vi "DéfiGentecEO.vi"() -> ()   [LabVIEW 2017]
uses:
  PC-Beamage Labview Distribution/BeamageNP.dll
panel:
  in  "File Type 2":enum16{"JPG", "PNG", "BMP"}(ring)=enum."BMP"
  in  "File Type":enum16{"JPG", "PNG", "BMP"}(ring)=enum."BMP"
  in  "Panneau de Fin":string caption="Tous les vaisseaux\n  ont été détruits!"
  out "Loop":dbl
  out "Saturation Power":dbl
  out "Yposition":dbl
  out "Xposition":dbl
  in  "Boolean":bool
  in  "error in  2":errorcluster
  out "DLL is Present":bool
  out "path":path
  out "error out 3":errorcluster
  in  "error in":errorcluster
  out "Connected":bool
  out "error out":errorcluster
  out "Pause En Cours 1":bool
  out "Temps Pause 1":timestamp
  out "Barre Bleue 1":dbl(slide) scale=0.0..100.0
  out "Pointage 1":dbl
  out "Barre Verte 1":dbl(slide) max=50.0 scale=0.0..100.0
  out "Chrono 1":dbl format="%.2g"
  in  "Cancel Button":bool
  out "Nombre total de vaisseaux":dbl
  out "Barre Rouge 1":dbl(slide) scale=0.0..100.0
  out "XY Graph 1":cluster{dbl[], dbl[]}[](graph)
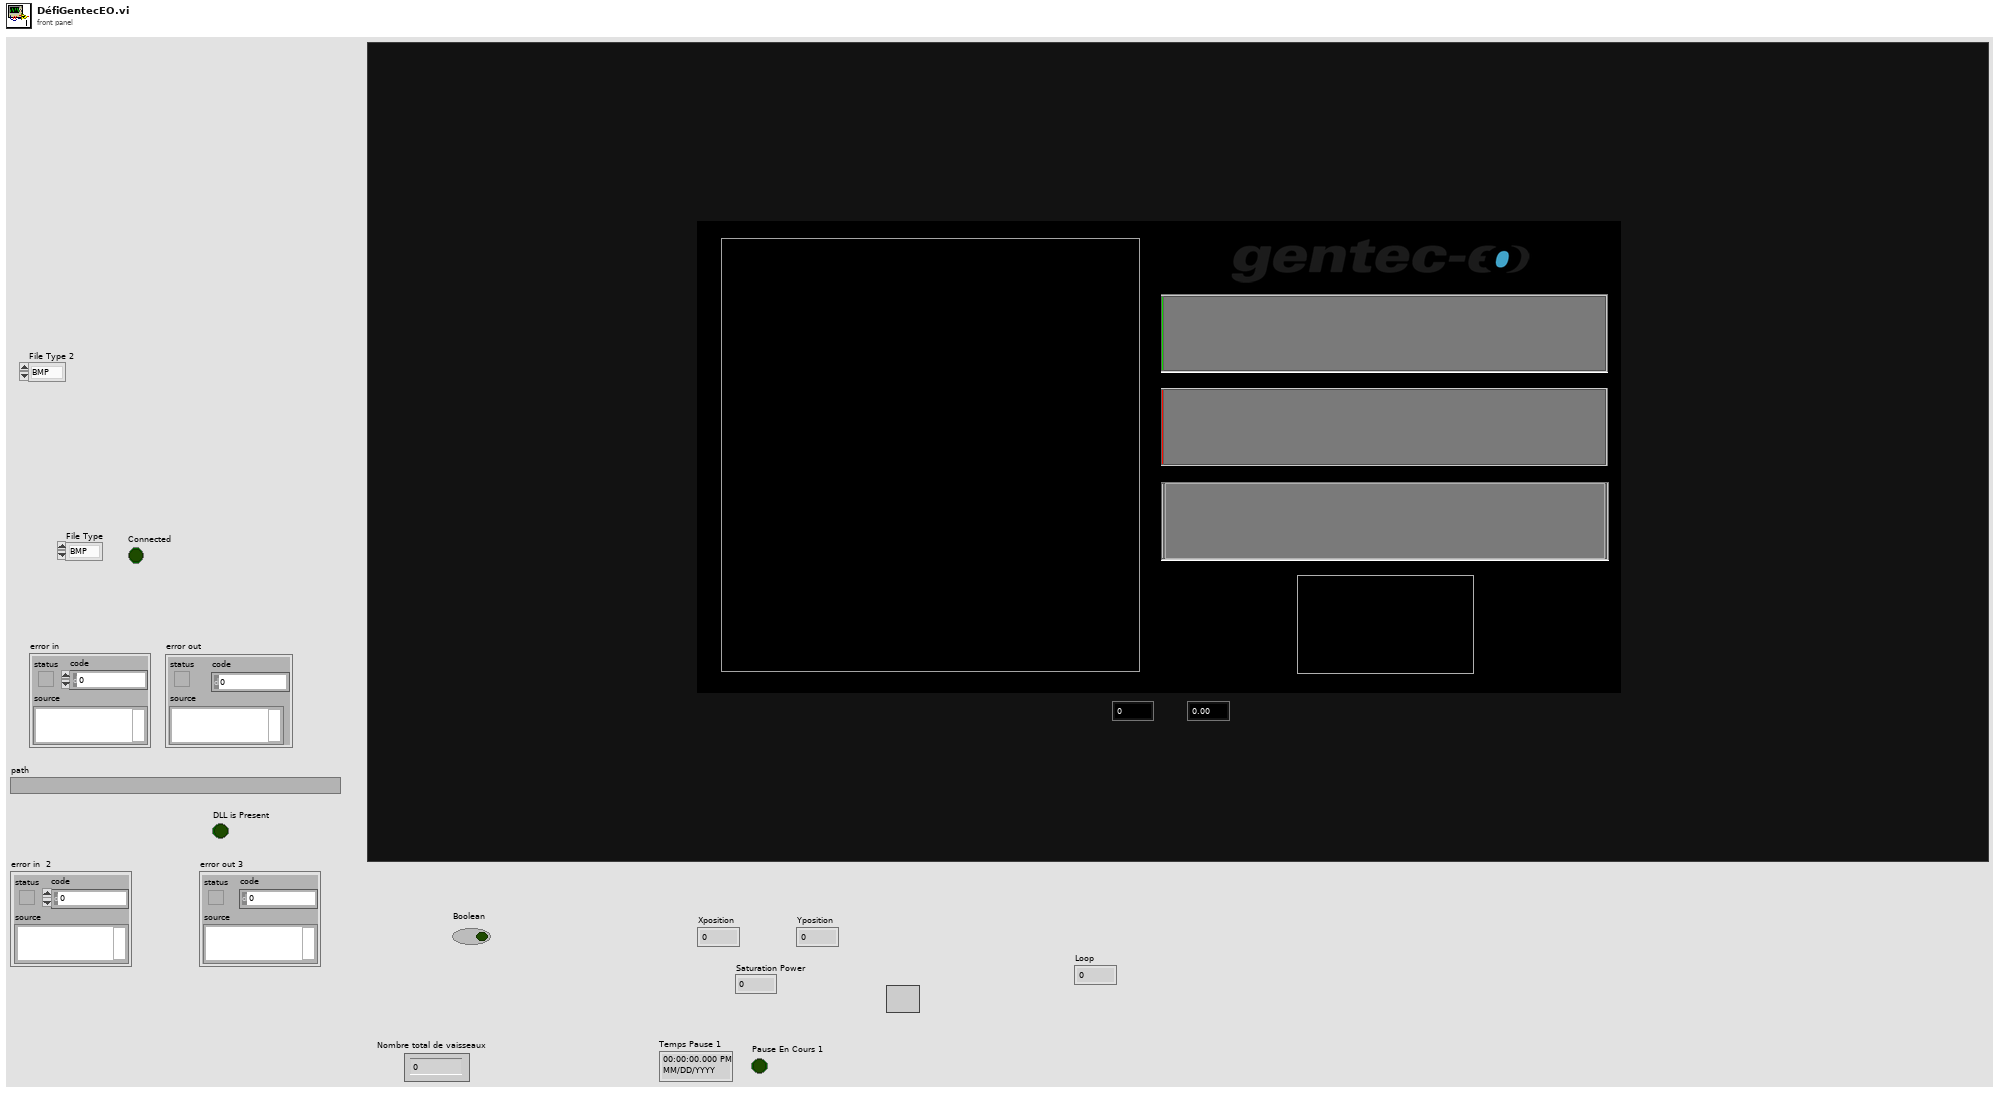
[diagram p1: front panel]
types:
  T1 = typedef "imagedata.ctl" = cluster{"image type":i32, "image depth":i32, "image":u8[], "mask":u8[], "colors":u32[], "Rectangle":cluster{"left":i16, "top":i16, "right":i16, "bottom":i16}}
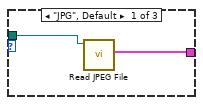
[diagram p2: hidden frame]
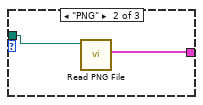
[diagram p3: hidden frame]
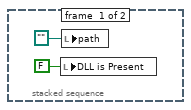
[diagram p4: hidden frame]
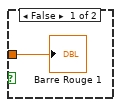
[diagram p11: hidden frame]
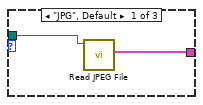
[diagram p13: hidden frame]
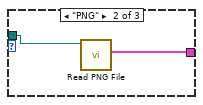
[diagram p14: hidden frame]
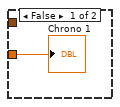
[diagram p15: hidden frame]
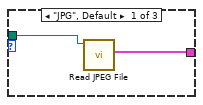
[diagram p17: hidden frame]
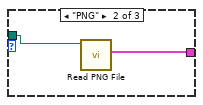
[diagram p18: hidden frame]
diagram:
  n1 = flat-sequence {
    tunnel: [w25] -> w2
    tunnel: [w13] -> w1
    tunnel: w2 -> [w56]
    tunnel: w1 -> [w55]
    frame #0 {
      w10 = u32 16777215
      w22 = 0
      # "Code LabVIEW écrit par Charles Matte-Breton dans le cadre de la 10e édition des Jeux Photoniques (23 octobre 2017)"
      n2 = Current VI's Path() -> (path=w5:path)
      n3 = case shown="No Error" "error in" {
        selector: "error in" -> [w50 w54]
        tunnel: [w49 w54] -> w17
        frame No Error {
          # "Verify that PC Beamage is running and the Labview data  pipe is open."
          n4 = dll-call lib="PTH2Šabs CUsersCharles\tDocumentsÃ‰coleImplicationJeux PhotoniquesDÃ©fi Gentec-EOPC-Beamage Labview Distribution\nBeamageNP.dll" fn="OpenNP"(error in=w50) -> (error out=w49:errorcluster, "return type"=w53:i32)  [unwired: 2 in, 1 out]
          n5 = Equal?(x=w53, y=1) -> (x = y?=→"Connected":bool)
        }
        frame Error {
        }
      }
      "error out" <- w17
      n6 = local write "Barre Rouge 1"(w22) -> ()
      n7 = local write "Barre Bleue 1"(w22) -> ()
      n8 = property on="XY Graph 1" class="XYGraph (strict)"("BG Color"=u32 0) -> ()  [unwired: 2 in, 2 out]
      n9 = case shown="No Error" "error in  2" {
        selector: "error in  2" -> [w33 w48]
        tunnel: [w32 w48] -> w15
        frame No Error {
          # "Verify the DLL Labview needs to communicate with PC-Beamage is present on the PC.\n\nFile should be in the same directory as this VI."
          n10 = stacked-sequence {
            tunnel: w33 -> [_ w43]
            tunnel: [_ w41] -> w32
            frame #0 {
              n11 = local write "DLL is Present"(FALSE ("file exists?")) -> ()
              n12 = local write "path"(path "") -> ()
            }
            frame #1 {
              n13 = property class="VI"(error in=w43) -> (error out=w42:errorcluster, "Path"=w47:path, "Name"=w37:string)  [unwired: 1 in, 1 out]
              n14 = Path To String(path=w47) -> (string=w38:string)
              n15 = Match Pattern(string=w38, regular expression=w37) -> (before substring=w36:string)  [unwired: 1 in, 3 out]
              n16 = Concatenate Strings(w36, "BeamageNP.dll" ("string")) -> (w45:string)
              n17 = String To Path(string=w45) -> (path=w44:path)
              n18 = call <vilib>:"Check if File or Folder Exists.vi"("error in (no error)"=w42, "path"=w44) -> ("error out"=w41:errorcluster, "file or folder exists?"=→"DLL is Present":bool, "dup path"=→"path":path)  [unwired: 7 in]
            }
          }
        }
        frame Error {
        }
      }
      "error out 3" <- w15
      n19 = property on="Chrono 1" class="DigNum (strict)"("NumText.BGColor"=u32 0) -> ()  [unwired: 2 in, 2 out]
      n20 = Build Path(base path=w5, name or relative path=path "../Espace.bmp") -> (appended path=w3:path)
      n21 = case shown="\"BMP\"" "File Type" {
        tunnel: [w27 w29 w31] -> w8
        tunnel: w3 -> [w26 w28 w30]
        frame "JPG", Default {
          n22 = call <vilib>:"Read JPEG File.vi"("path to JPEG file"=w26) -> ("image data"=w27:T1)  [unwired: 8 in, 2 out]
        }
        frame "PNG" {
          n23 = call <vilib>:"Read PNG File.vi"("path to PNG file"=w28) -> ("image data"=w29:T1)  [unwired: 8 in, 2 out]
        }
        frame "BMP" {
          n24 = call <vilib>:"Read BMP File.vi"("path to BMP file"=w30) -> ("image data"=w31:T1)  [unwired: 8 in, 2 out]
        }
      }
      n25 = Wait (ms)(milliseconds to wait=5) -> ()  [unwired: 1 out]
      n26 = local write "Pause En Cours 1"(FALSE) -> ()
      n27 = property on="Chrono 1" class="DigNum (strict)"("NumText.TextColor"=w10) -> ()  [unwired: 2 in, 2 out]
      n28 = property on="Panneau de Fin" class="Str"("Visible"=FALSE) -> ()  [unwired: 2 in, 2 out]
      n29 = call <vilib>:"Draw Flattened Pixmap.vi"("image data"=w8) -> ("new picture"=w6:picture)  [unwired: 8 in]
      n30 = local write "Pointage 1"(0) -> ()
      n31 = property on="Pointage 1" class="DigNum (strict)"("NumText.TextColor"=w10) -> ()  [unwired: 2 in, 2 out]
      n32 = property on="XY Graph 1" class="XYGraph (strict)"("PlotImages.Back"=w6) -> ()  [unwired: 2 in, 2 out]
      n33 = Spreadsheet String To Array(format string="%f", spreadsheet string="0\t0\n0\t0\n0\t0\n0\t0\n0\t0\n0\t0\n0\t0\n0\t0\n0\t0\n0\t0\n0\t0\n0\t0\n0\t0\n0\t0\n0\t0\n0\t0\n0\t0\n0\t0\n0\t0\n0\t0\n0\t0\n0\t0\n0\t0\n0\t0\n0\t0\n0\t0\n0\t0\n0\t0\n0\t0\n0\t0\n0\t0\n0\t0\n0\t0\n0\t0\n0\t0\n0\t0\n0\t0\n0\t0\n0\t0\n0\t0\n0\t0\n0\t0\n0\t0\n0\t0\n0\t0\n0\t0\n0\t0\n0\t0\n0\t0\n0\t0\n0\t0\n0\t0\n0\t0\n0\t0\n0\t0\n0\t0\n0\t0\n0\t0\n0\t0\n0\t0\n0\t0\n0\t0\n0\t0\n0\t0\n0\t0\n0\t0\n0\t0\n0\t0\n0\t0\n0\t0\n0\t0\n0\t0\n0\t0\n0\t0\n0\t0\n0\t0\n0\t0\n0\t0\n0\t0\n0\t0\n0\t0\n0\t0\n0\t0\n0\t0\n0\t0\n0\t0\n0\t0\n0\t0\n0\t0\n0\t0\n0\t0\n0\t0\n0\t0\n0\t0\n0\t0\n0\t0\n0\t0\n0\t0\n0\t0\n0\t0\n0\t0\n0\t0\n0\t0\n0\t0\n0\t0\n0\t0\n0\t0\n0\t0\n0\t0\n0\t0\n0\t0\n0\t0\n0\t0\n0\t0\n0\t0\n0\t0\n0\t0\n0\t0\n0\t0\n0\t0\n0\t0\n0\t0\n0\t0\n0\t0\n0\t0\n0\t0\n0\t0\n0\t0\n0\t0\n0\t0\n0\t0\n0\t0\n0\t0\n0\t0\n0\t0\n0\t0\n0\t0\n0\t0\n0\t0\n0\t0\n0\t0\n0\t0\n0\t0\n0\t0\n0\t0\n0\t0\n0\t0\n0\t0\n0\t0\n0\t0\n0.1\t0\n0.2\t0\n0.3\t0\n0.4\t0\n0.5\t0\n0.6\t0\n0.7\t0\n0.8\t0\n0.9\t0\n1\t0\n1.1\t0\n1.2\t0\n1.3\t0\n1.4\t0\n1.5\t0\n1.6\t0\n1.7\t0\n1.8\t0\n1.9\t0\n2\t0\n2.1\t0\n2.2\t0\n2.3\t0\n2.4\t0\n2.5\t0\n2.6\t0\n2.7\t0\n2.8\t0\n2.9\t0\n3\t0\n3.1\t0\n3.2\t0\n3.3\t0\n3.4\t0\n3.5\t0\n3.6\t0\n3.7\t0\n3.8\t0\n3.9\t0\n4\t0\n4.1\t0\n4.2\t0\n4.3\t0\n4.4\t0\n4.5\t0\n4.6\t0\n4.7\t0\n4.8\t0\n4.9\t0\n5\t0\n5.1\t0\n5.2\t0\n5.3\t0\n5.4\t0\n5.5\t0\n5.6\t0\n5.7\t0\n5.8\t0\n5.9\t0\n6\t0\n6.1\t0\n6.2\t0\n6.3\t0\n6.4\t0\n6.5\t0\n6.6\t0\n6.7\t0\n6.8\t0\n6.9\t0\n7\t0\n7.1\t0\n7.2\t0\n7.3\t0\n7.4\t0\n7.5\t0\n7.6\t0\n7.7\t0\n7.8\t0\n7.9\t0\n8\t0\n8.1\t0\n8.2\t0\n8.3\t0\n8.4\t0\n8.5\t0\n8.6\t0\n8.7\t0\n8.8\t0\n8.9\t0\n9\t0\n9.1\t0\n9.2\t0\n9.3\t0\n9.4\t0\n9.5\t0\n9.6\t0\n9.7\t0\n9.8\t0\n9.9\t0\n10\t0\n10.1\t0\n10.2\t0\n10.3\t0\n10.4\t0\n10.5\t0\n10.6\t0\n10.7\t0\n10.8\t0\n10.9\t0\n11\t0\n11.1\t0\n11.2\t0\n11.3\t0\n11.4\t0\n11.5\t0\n11.6\t0\n11.7\t0\n11.8\t0\n11.9\t0\n12\t0\n12.1\t0\n12.2\t0\n12.3\t0\n12.4\t0\n12.5\t0\n12.6\t0\n12.7\t0\n12.8\t0\n12.9\t0\n13\t0\n13.1\t0\n13.2\t0\n13.3\t0\n13.4\t0\n13.5\t0\n13.6\t0\n13.7\t0\n13.8\t0\n13.9\t0\n14\t0\n14.1\t0\n14.2\t0\n14.3\t0\n14.4\t0\n14.5\t0\n14.6\t0\n14.7\t0\n14.8\t0\n14.9\t0\n15\t0\n15.1\t0\n15.2\t0\n15.3\t0\n15.4\t0\n15.5\t0\n15.6\t0\n15.7\t0\n15.8\t0\n15.9\t0\n16\t0\n16.1\t0\n16.2\t0\n16.3\t0\n16.4\t0\n16.5\t0\n16.6\t0\n16.7\t0\n16.8\t0\n16.9\t0\n17\t0\n17.1\t0\n17.2\t0\n17.3\t0\n17.4\t0\n17.5\t0\n17.6\t0\n17.7\t0\n17.8\t0\n17.9\t0\n18\t0\n18.1\t0\n18.2\t0\n18.3\t0\n18.4\t0\n18.5\t0\n18.6\t0\n18.7\t0\n18.8\t0\n18.9\t0\n19\t0\n19.1\t0\n19.2\t0\n19.3\t0\n19.4\t0\n19.5\t0\n19.6\t0\n19.7\t0\n19.8\t0\n19.9\t0\n20\t0\n20.1\t0\n20.2\t0\n20.3\t0\n20.4\t0\n20.5\t0\n20.6\t0\n20.7\t0\n20.8\t0\n20.9\t0\n21\t0\n21.1\t0\n21.2\t0\n21.3\t0\n21.4\t0\n21.5\t0\n21.6\t0\n21.7\t0\n21.8\t0\n21.9\t0\n22\t0\n22.1\t0\n22.2\t0\n22.3\t0\n22.4\t0\n22.5\t0\n22.6\t0\n22.7\t0\n22.8\t0\n22.9\t0\n23\t0\n23.1\t0\n23.2\t0\n23.3\t0\n23.4\t0\n23.5\t0\n23.6\t0\n23.7\t0\n23.8\t0\n23.9\t0\n24\t0\n24.1\t0\n24.2\t0\n24.3\t0\n24.4\t0\n24.5\t0\n24.6\t0\n24.7\t0\n24.8\t0\n24.9\t0\n25\t0\n25.1\t0\n25.2\t0\n25.3\t0\n25.4\t0\n25.5\t0\n25.6\t0\n25.7\t0\n25.8\t0\n25.9\t0\n26\t0\n26.1\t0\n26.2\t0\n26.3\t0\n26.4\t0\n26.5\t0\n26.6\t0\n26.7\t0\n26.8\t0\n26.9\t0\n27\t0\n27.1\t0\n27.2\t0\n27.3\t0\n27.4\t0\n27.5\t0\n27.6\t0\n27.7\t0\n27.8\t0\n27.9\t0\n28\t0\n28.1\t0\n28.2\t0\n28.3\t0\n28.4\t0\n28.5\t0\n28.6\t0\n28.7\t0\n28.8\t0\n28.9\t0\n29\t0\n29.1\t0\n29.2\t0\n29.3\t0\n29.4\t0\n29.5\t0\n29.6\t0\n29.7\t0\n29.8\t0\n29.9\t0\n30\t0\n30.1\t0\n30.2\t0\n30.3\t0\n30.4\t0\n30.5\t0\n30.6\t0\n30.7\t0\n30.8\t0\n30.9\t0\n31\t0\n31.1\t0\n31.2\t0\n31.3\t0\n31.4\t0\n31.5\t0\n31.6\t0\n31.7\t0\n31.8\t0\n31.9\t0\n32\t0\n32.1\t0\n32.2\t0\n32.3\t0\n32.4\t0\n32.5\t0\n32.6\t0\n32.7\t0\n32.8\t0\n32.9\t0\n33\t0\n33.1\t0\n33.2\t0\n33.3\t0\n33.4\t0\n33.5\t0\n33.6\t0\n33.7\t0\n33.8\t0\n33.9\t0\n34\t0\n34.1\t0\n34.2\t0\n34.3\t0\n34.4\t0\n34.5\t0\n34.6\t0\n34.7\t0\n34.8\t0\n34.9\t0\n35\t0\n35.1\t0\n35.2\t0\n35.3\t0\n35.4\t0\n35.5\t0\n35.6\t0\n35.7\t0\n35.8\t0\n35.9\t0\n36\t0\n36.1\t0\n36.2\t0\n36.3\t0\n36.4\t0\n36.5\t0\n36.6\t0\n36.7\t0\n36.8\t0\n36.9\t0\n37\t0\n37.1\t0\n37.2\t0\n37.3\t0\n37.4\t0\n37.5\t0\n37.6\t0\n37.7\t0\n37.8\t0\n37.9\t0\n38\t0\n38.1\t0\n38.2\t0\n38.3\t0\n38.4\t0\n38.5\t0\n38.6\t0\n38.7\t0\n38.8\t0\n38.9\t0\n39\t0\n39.1\t0\n39.2\t0\n39.3\t0\n39.4\t0\n39.5\t0\n39.6\t0\n39.7\t0\n39.8\t0\n39.9\t0\n40\t0\n40.1\t0\n40.2\t0\n40.3\t0\n40.4\t0\n40.5\t0\n40.6\t0\n40.7\t0\n40.8\t0\n40.9\t0\n41\t0\n41.1\t0\n41.2\t0\n41.3\t0\n41.4\t0\n41.5\t0\n41.6\t0\n41.7\t0\n41.8\t0\n41.9\t0\n42\t0\n42.1\t0\n42.2\t0\n42.3\t0\n42.4\t0\n42.5\t0\n42.6\t0\n42.7\t0\n42.8\t0\n42.9\t0\n43\t0\n43.1\t0\n43.2\t0\n43.3\t0\n43.4\t0\n43.5\t0\n43.6\t0\n43.7\t0\n43.8\t0\n43.9\t0\n44\t0\n44.1\t0\n44.2\t0\n44.3\t0\n44.4\t0\n44.5\t0\n44.6\t0\n44.7\t0\n44.8\t0\n44.9\t0\n45\t0\n45.1\t0\n45.2\t0\n45.3\t0\n45.4\t0\n45.5\t0\n45.6\t0\n45.7\t0\n45.8\t0\n45.9\t0\n46\t0\n46.1\t0\n46.2\t0\n46.3\t0\n46.4\t0\n46.5\t0\n46.6\t0\n46.7\t0\n46.8\t0\n46.9\t0\n47\t0\n47.1\t0\n47.2\t0\n47.3\t0\n47.4\t0\n47.5\t0\n47.6\t0\n47.7\t0\n47.8\t0\n47.9\t0\n48\t0.3\n48.1\t0.6\n48.2\t0.9\n48.3\t1.2\n48.4\t1.5\n48.5\t1.8\n48.6\t2.1\n48.7\t2.4\n48.8\t2.7\n48.9\t3\n49\t3.3\n49.1\t3.6\n49.2\t3.9\n49.3\t4.2\n49.4\t4.5\n49.5\t4.8\n49.6\t5.1\n49.7\t5.4\n49.8\t5.7\n49.9\t6\n50\t6.3\n50.1\t6.6\n50.2\t6.9\n50.3\t7.2\n50.4\t7.5\n50.5\t7.8\n50.6\t8.1\n50.7\t8.4\n50.8\t8.7\n50.9\t9\n51\t9.3\n51.1\t9.6\n51.2\t9.9\n51.3\t10.2\n51.4\t10.5\n51.5\t10.8\n51.6\t11.1\n51.7\t11.4\n51.8\t11.7\n51.9\t12\n52\t12.3\n52.1\t12.6\n52.2\t12.9\n52.3\t13.2\n52.4\t13.5\n52.5\t13.8\n52.6\t14.1\n52.7\t14.4\n52.8\t14.7\n52.9\t15\n53\t15.3\n53.1\t15.6\n53.2\t15.9\n53.3\t16.2\n53.4\t16.5\n53.5\t16.8\n53.6\t17.1\n53.7\t17.4\n53.8\t17.7\n53.9\t18\n54\t18.3\n54.1\t18.6\n54.2\t18.9\n54.3\t19.2\n54.4\t19.5\n54.5\t19.8\n54.6\t20.1\n54.7\t20.4\n54.8\t20.7\n54.9\t21\n55\t21.3\n55.1\t21.6\n55.2\t21.9\n55.3\t22.2\n55.4\t22.5\n55.5\t22.8\n55.6\t23.1\n55.7\t23.4\n55.8\t23.7\n55.9\t24\n56\t24.3\n56.1\t24.6\n56.2\t24.9\n56.3\t25.2\n56.4\t25.5\n56.5\t25.8\n56.6\t26.1\n56.7\t26.4\n56.8\t26.7\n56.9\t27\n57\t27.3\n57.1\t27.6\n57.2\t27.9\n57.3\t28.2\n57.4\t28.5\n57.5\t28.8\n57.6\t29.1\n57.7\t29.4\n57.8\t29.7\n57.9\t30\n58\t30.3\n58.1\t30.6\n58.2\t30.9\n58.3\t31.2\n58.4\t31.5\n58.5\t31.8\n58.6\t32.1\n58.7\t32.4\n58.8\t32.7\n58.9\t33\n59\t33.3\n59.1\t33.6\n59.2\t33.9\n59.3\t34.2\n59.4\t34.5\n59.5\t34.8\n59.6\t35.1\n59.7\t35.4\n59.8\t35.7\n59.9\t36\n60\t36.3\n60.1\t36.6\n60.2\t36.9\n60.3\t37.2\n60.4\t37.5\n60.5\t37.8\n60.6\t38.1\n60.7\t38.4\n60.8\t38.7\n60.9\t39\n61\t39.3\n61.1\t39.6\n61.2\t39.9\n61.3\t40.2\n61.4\t40.5\n61.5\t40.8\n61.6\t41.1\n61.7\t41.4\n61.8\t41.7\n61.9\t42\n62\t42.3\n62.1\t42.6\n62.2\t42.9\n62.3\t43.2\n62.4\t43.5\n62.5\t43.8\n62.6\t44.1\n62.7\t44.4\n62.8\t44.7\n62.9\t45\n63\t45.3\n63.1\t45.6\n63.2\t45.9\n63.3\t46.2\n63.4\t46.5\n63.5\t46.8\n63.6\t47.1\n63.7\t47.4\n63.8\t47.7\n63.9\t48\n64\t48.3\n64.1\t48.6\n64.2\t48.9\n64.3\t49.2\n64.4\t49.5\n64.5\t49.8\n64.6\t50.1\n64.7\t50.4\n64.8\t50.7\n64.9\t51\n65\t51.3\n65.1\t51.6\n65.2\t51.9\n65.3\t52.2\n65.4\t52.5\n65.5\t52.8\n65.6\t53.1\n65.7\t53.4\n65.8\t53.7\n65.9\t54\n66\t54.3\n66.1\t54.6\n66.2\t54.9\n66.3\t55.2\n66.4\t55.5\n66.5\t55.8\n66.6\t56.1\n66.7\t56.4\n66.8\t56.7\n66.9\t57\n67\t57.3\n67.1\t57.6\n67.2\t57.9\n67.3\t58.2\n67.4\t58.5\n67.5\t58.8\n67.6\t59.1\n67.7\t59.4\n67.8\t59.7\n67.9\t60\n68\t60.3\n68.1\t60.6\n68.2\t60.9\n68.3\t61.2\n68.4\t61.5\n68.5\t61.8\n68.6\t62.1\n68.7\t62.4\n68.8\t62.7\n68.9\t63\n69\t63.3\n69.1\t63.6\n69.2\t63.9\n69.3\t64.2\n69.4\t64.5\n69.5\t64.8\n69.6\t65.1\n69.7\t65.4\n69.8\t65.7\n69.9\t66\n70\t66.3\n70.1\t66.6\n70.2\t66.9\n70.3\t67.2\n70.4\t67.5\n70.5\t67.8\n70.6\t68.1\n70.7\t68.4\n70.8\t68.7\n70.9\t69\n71\t69.3\n71.1\t69.6\n71.2\t69.9\n71.3\t70.2\n71.4\t70.5\n71.5\t70.8\n71.6\t71.1\n71.7\t71.4\n71.8\t71.7\n71.9\t72\n72\t72.3\n72.1\t72.6\n72.2\t72.9\n72.3\t73.2\n72.4\t73.5\n72.5\t73.8\n72.6\t74.1\n72.7\t74.4\n72.8\t74.7\n72.9\t75\n73\t75.3\n73.1\t75.6\n73.2\t75.9\n73.3\t76.2\n73.4\t76.5\n73.5\t76.8\n73.6\t77.1\n73.7\t77.4\n73.8\t77.7\n73.9\t78\n74\t78.3\n74.1\t78.6\n74.2\t78.9\n74.3\t79.2\n74.4\t79.5\n74.5\t79.8\n74.6\t80.1\n74.7\t80.4\n74.8\t80.7\n74.9\t81\n74.7\t81.3\n74.5\t81.6\n74.3\t81.9\n74.1\t82.2\n73.9\t82.5\n73.7\t82.8\n73.5\t83.1\n73.3\t83.4\n73.1\t83.7\n72.9\t84\n72.7\t84.3\n72.5\t84.6\n72.3\t84.9\n72.1\t85.2\n71.9\t85.5\n71.7\t85.8\n71.5\t86.1\n71.3\t86.4\n71.1\t86.7\n70.9\t87\n70.7\t87.3\n70.5\t87.6\n70.3\t87.9\n70.1\t88.2\n69.9\t88.5\n69.7\t88.8\n69.5\t89.1\n69.3\t89.4\n69.1\t89.7\n68.9\t90\n68.7\t90.3\n68.5\t90.6\n68.3\t90.9\n68.1\t91.2\n67.9\t91.5\n67.7\t91.8\n67.5\t92.1\n67.3\t92.4\n67.1\t92.7\n66.9\t93\n66.7\t93.3\n66.5\t93.6\n66.3\t93.9\n66.1\t94.2\n65.9\t94.5\n65.7\t94.8\n65.5\t95.1\n65.3\t95.4\n65.1\t95.7\n64.9\t96\n64.7\t96.3\n64.5\t96.6\n64.3\t96.9\n64.1\t97.2\n63.9\t97.5\n63.7\t97.3\n63.5\t97.1\n63.3\t96.9\n63.1\t96.7\n62.9\t96.5\n62.7\t96.3\n62.5\t96.1\n62.3\t95.9\n62.1\t95.7\n61.9\t95.5\n61.7\t95.3\n61.5\t95.1\n61.3\t94.9\n61.1\t94.7\n60.9\t94.5\n60.7\t94.3\n60.5\t94.1\n60.3\t93.9\n60.1\t93.7\n59.9\t93.5\n59.7\t93.3\n59.5\t93.1\n59.3\t92.9\n59.1\t92.7\n58.9\t92.5\n58.7\t92.3\n58.5\t92.1\n58.3\t91.9\n58.1\t91.7\n57.9\t91.5\n57.7\t91.3\n57.5\t91.1\n57.3\t90.9\n57.1\t90.7\n56.9\t90.5\n56.7\t90.3\n56.5\t90.1\n56.3\t89.9\n56.1\t89.7\n55.9\t89.5\n55.7\t89.3\n55.5\t89.1\n55.3\t88.9\n55.1\t88.7\n54.9\t88.5\n54.7\t88.3\n54.5\t88.1\n54.3\t87.9\n54.1\t87.7\n53.9\t87.5\n53.7\t87.3\n53.5\t87.1\n53.3\t86.9\n53.1\t86.7\n52.9\t86.5\n52.7\t86.3\n52.5\t86.1\n52.3\t85.9\n52.1\t85.7\n51.9\t85.5\n51.7\t85.3\n51.5\t85.1\n51.3\t84.9\n51.1\t84.7\n50.9\t84.5\n50.7\t84.3\n50.5\t84.1\n50.3\t83.9\n50.1\t83.7\n49.9\t83.5\n49.7\t83.3\n49.5\t83.1\n49.3\t82.9\n49.1\t82.7\n48.9\t82.5\n48.7\t82.3\n48.5\t82.1\n48.3\t81.9\n48.1\t81.7\n47.9\t81.5\n47.7\t81.3\n47.5\t81.1\n47.3\t80.9\n47.1\t80.7\n46.9\t80.5\n46.7\t80.3\n46.5\t80.1\n46.3\t79.9\n46.1\t79.7\n45.9\t79.5\n45.7\t79.3\n45.5\t79.1\n45.3\t78.9\n45.1\t78.7\n44.9\t78.5\n44.7\t78.3\n44.5\t78.1\n44.3\t77.9\n44.1\t77.7\n43.9\t77.5\n43.7\t77.3\n43.5\t77.1\n43.3\t76.9\n43.1\t76.7\n42.9\t76.5\n42.7\t76.3\n42.5\t76.1\n42.3\t75.9\n42.1\t75.7\n41.9\t75.5\n41.7\t75.3\n41.5\t75.1\n41.3\t74.9\n41.1\t74.7\n40.9\t74.5\n40.7\t74.3\n40.5\t74.1\n40.3\t73.9\n40.1\t73.7\n39.9\t73.5\n39.7\t73.3\n39.5\t73.1\n39.3\t72.9\n39.1\t72.7\n38.9\t72.5\n38.7\t72.3\n38.5\t72.1\n38.3\t71.9\n38.1\t71.7\n37.9\t71.5\n37.7\t71.3\n37.5\t71.1\n37.3\t70.9\n37.1\t70.7\n36.9\t70.5\n36.7\t70.3\n36.5\t70.1\n36.3\t69.9\n36.1\t69.7\n35.9\t69.5\n35.7\t69.3\n35.5\t69.1\n35.3\t68.9\n35.1\t68.7\n34.9\t68.5\n34.7\t68.3\n34.5\t68.1\n34.3\t67.9\n34.1\t67.7\n33.9\t67.5\n33.7\t67.3\n33.5\t67.1\n33.3\t66.9\n33.1\t66.7\n32.9\t66.5\n32.7\t66.3\n32.5\t66.1\n32.3\t65.9\n32.1\t65.7\n31.9\t65.5\n31.7\t65.3\n31.5\t65.1\n31.3\t64.9\n31.1\t64.7\n30.9\t64.5\n30.7\t64.3\n30.5\t64.1\n30.3\t63.9\n30.1\t63.7\n29.9\t63.5\n29.7\t63.3\n29.5\t63.1\n29.3\t62.9\n29.1\t62.7\n28.9\t62.5\n28.7\t62.3\n28.5\t62.1\n28.3\t61.9\n28.1\t61.7\n27.9\t61.5\n27.7\t61.3\n27.5\t61.1\n27.3\t60.9\n27.1\t60.7\n26.9\t60.5\n26.7\t60.3\n26.5\t60.1\n26.3\t59.9\n26.1\t59.7\n25.9\t59.5\n25.7\t59.3\n25.5\t59.1\n25.3\t58.9\n25.1\t58.7\n24.9\t58.5\n24.7\t58.3\n24.5\t58.1\n24.3\t57.9\n24.1\t57.7\n23.9\t57.5\n23.7\t57.3\n23.5\t57.1\n23.3\t56.9\n23.1\t56.7\n22.9\t56.5\n22.7\t56.3\n22.5\t56.1\n22.3\t55.9\n22.1\t55.7\n21.9\t55.5\n21.7\t55.3\n21.5\t55.1\n21.3\t54.9\n21.1\t54.7\n20.9\t54.5\n20.7\t54.3\n20.5\t54.1\n20.3\t53.9\n20.1\t53.7\n19.9\t53.5\n19.7\t53.3\n19.5\t53.1\n19.3\t52.9\n19.1\t52.7\n18.9\t52.5\n18.7\t52.3\n18.5\t52.1\n18.3\t51.9\n18.1\t51.7\n17.9\t51.5\n17.7\t51.3\n17.5\t51.1\n17.3\t50.9\n17.1\t50.7\n16.9\t50.5\n16.7\t50.3\n16.5\t50.1\n16.3\t49.9\n16.1\t49.7\n15.9\t49.5\n15.7\t49.3\n15.5\t49.1\n15.3\t48.9\n15.1\t48.7\n14.9\t48.5\n14.7\t48.3\n14.5\t48.1\n14.3\t47.9\n14.1\t47.7\n13.9\t47.5\n13.7\t47.3\n13.5\t47.1\n13.3\t46.9\n13.1\t46.7\n12.9\t46.5\n12.7\t46.3\n12.5\t46.1\n12.3\t45.9\n12.1\t45.7\n11.9\t45.5\n11.7\t45.3\n11.5\t45.1\n11.3\t44.9\n11.1\t44.7\n10.9\t44.5\n10.7\t44.3\n10.5\t44.1\n10.3\t43.9\n10.1\t43.7\n9.9\t43.5\n9.7\t43.3\n9.5\t43.1\n9.3\t42.9\n9.1\t42.7\n8.9\t42.5\n8.7\t42.3\n8.5\t42.1\n8.3\t41.9\n8.1\t41.7\n7.9\t41.5\n7.7\t41.3\n7.5\t41.1\n7.3\t40.9\n7.1\t40.7\n6.9\t40.5\n6.7\t40.3\n6.5\t40.1\n6.3\t39.9\n6.1\t39.7\n5.9\t39.5\n5.7\t39.3\n5.5\t39.1\n5.3\t38.9\n5.1\t38.7\n4.9\t38.5\n4.7\t38.3\n4.5\t38.1\n4.3\t37.9\n4.1\t37.7\n3.9\t37.5\n3.7\t37.3\n3.5\t37.1\n3.3\t36.9\n3.1\t36.7\n2.9\t36.5\n2.7\t36.3\n2.5\t36.1\n2.3\t35.9\n2.1\t35.7\n1.9\t35.5\n1.7\t35.3\n1.5\t35.1\n1.3\t34.9\n1.1\t34.7\n0.9\t34.5\n0.7\t34.3\n0.5\t34.1\n0.3\t33.9\n0.1\t33.7\n-0.1\t33.5\n-0.3\t33.3\n-0.5\t33.1\n-0.7\t32.9\n-0.9\t32.7\n-1.1\t32.5\n-1.3\t32.3\n-1.5\t32.1\n-1.7\t31.9\n-1.9\t31.7\n-2.1\t31.5\n-2.3\t31.3\n-2.5\t31.1\n-2.7\t30.9\n-2.9\t30.7\n-3.1\t30.5\n-3.3\t30.3\n-3.5\t30.1\n-3.7\t29.9\n-3.9\t29.7\n-4.1\t29.5\n-4.3\t29.3\n-4.5\t29.1\n-4.7\t28.9\n-4.9\t28.7\n-5.1\t28.5\n-5.3\t28.3\n-5.5\t28.1\n-5.7\t27.9\n-5.9\t27.7\n-6.1\t27.5\n-6.3\t27.3\n-6.5\t27.1\n-6.7\t26.9\n-6.9\t26.7\n-7.1\t26.5\n-7.3\t26.3\n-7.5\t26.1\n-7.7\t25.9\n-7.9\t25.7\n-8.1\t25.5\n-8.3\t25.3\n-8.5\t25.1\n-8.7\t24.9\n-8.9\t24.7\n-9.1\t24.5\n-9.3\t24.3\n-9.5\t24.1\n-9.7\t23.9\n-9.9\t23.7\n-10.1\t23.5\n-10.3\t23.3\n-10.5\t23.1\n-10.7\t22.9\n-10.9\t22.7\n-11.1\t22.5\n-11.3\t22.3\n-11.5\t22.1\n-11.7\t21.9\n-11.9\t21.7\n-12.1\t21.5\n-12.3\t21.3\n-12.5\t21.1\n-12.7\t20.9\n-12.9\t20.7\n-13.1\t20.5\n-13.3\t20.3\n-13.5\t20.1\n-13.7\t19.9\n-13.9\t19.7\n-14.1\t19.5\n-14.3\t19.3\n-14.5\t19.1\n-14.7\t18.9\n-14.9\t18.7\n-15.1\t18.5\n-15.3\t18.3\n-15.5\t18.1\n-15.7\t17.9\n-15.9\t17.7\n-16.1\t17.5\n-16.3\t17.3\n-16.5\t17.1\n-16.7\t16.9\n-16.9\t16.7\n-17.1\t16.5\n-17.3\t16.3\n-17.5\t16.1\n-17.7\t15.9\n-17.9\t15.7\n-18.1\t15.5\n-18.3\t15.3\n-18.5\t15.1\n-18.7\t14.9\n-18.9\t14.7\n-19.1\t14.5\n-19.3\t14.3\n-19.5\t14.1\n-19.7\t13.9\n-19.9\t13.7\n-20.1\t13.5\n-20.3\t13.3\n-20.5\t13.1\n-20.7\t12.9\n-20.9\t12.7\n-21.1\t12.5\n-21.3\t12.3\n-21.5\t12.1\n-21.7\t11.9\n-21.9\t11.7\n-22.1\t11.5\n-22.3\t11.3\n-22.5\t11.1\n-22.7\t10.9\n-22.9\t10.7\n-23.1\t11.3\n-23.3\t11.9\n-23.5\t12.5\n-23.7\t13.1\n-23.9\t13.7\n-24.1\t14.3\n-24.3\t14.9\n-24.5\t15.5\n-24.7\t16.1\n-24.9\t16.7\n-25.1\t17.3\n-25.3\t17.9\n-25.5\t18.5\n-25.7\t19.1\n-25.9\t19.7\n-26.1\t20.3\n-26.3\t20.9\n-26.5\t21.5\n-26.7\t22.1\n-26.9\t22.7\n-27.1\t23.3\n-27.3\t23.9\n-27.5\t24.5\n-27.7\t25.1\n-27.9\t25.7\n-28.1\t26.3\n-28.3\t26.9\n-28.5\t27.5\n-28.7\t28.1\n-28.9\t28.7\n-29.1\t29.3\n-29.3\t29.9\n-29.5\t30.5\n-29.7\t31.1\n-29.9\t31.7\n-30.1\t32.3\n-30.3\t32.9\n-30.5\t33.5\n-30.7\t34.1\n-30.9\t34.7\n-31.1\t35.3\n-31.3\t35.9\n-31.5\t36.5\n-31.7\t37.1\n-31.9\t37.7\n-32.1\t38.3\n-32.3\t38.9\n-32.5\t39.5\n-32.7\t40.1\n-32.9\t40.7\n-33.1\t41.3\n-33.3\t41.9\n-33.5\t42.5\n-33.7\t43.1\n-33.9\t43.7\n-34.1\t44.3\n-34.3\t44.9\n-34.5\t45.5\n-34.7\t46.1\n-34.9\t46.7\n-35.1\t47.3\n-35.3\t47.9\n-35.5\t48.5\n-35.7\t49.1\n-35.9\t49.7\n-36.1\t50.3\n-36.3\t50.9\n-36.5\t51.5\n-36.7\t52.1\n-36.9\t52.7\n-37.1\t53.3\n-37.3\t53.9\n-37.5\t54.5\n-37.7\t55.1\n-37.9\t55.7\n-38.1\t56.3\n-38.3\t56.9\n-38.5\t57.5\n-38.7\t58.1\n-38.9\t58.7\n-39.1\t59.3\n-39.3\t59.9\n-39.5\t60.5\n-39.7\t61.1\n-39.9\t61.7\n-40.1\t62.3\n-40.3\t62.9\n-40.5\t63.5\n-40.7\t64.1\n-40.9\t64.7\n-41.1\t65.3\n-41.3\t65.9\n-41.5\t66.5\n-41.7\t67.1\n-41.9\t67.7\n-42.1\t68.3\n-42.3\t68.9\n-42.5\t69.5\n-42.7\t70.1\n-42.9\t70.7\n-43.1\t71.3\n-43.3\t71.9\n-43.5\t72.5\n-43.7\t73.1\n-43.9\t73.7\n-44.1\t74.3\n-44.3\t74.9\n-44.5\t75.5\n-44.7\t76.1\n-44.9\t76.7\n-45.1\t77.3\n-45.3\t77.9\n-45.5\t78.5\n-45.7\t79.1\n-45.9\t79.7\n-46.1\t80.3\n-46.3\t80.9\n-46.5\t81.5\n-46.7\t82.1\n-46.9\t82.7\n-47.1\t83.3\n-47.3\t83.9\n-47.5\t84.5\n-47.7\t85.1\n-47.9\t85.7\n-48.1\t86.3\n-48.3\t86.9\n-48.5\t87.5\n-48.7\t88.1\n-48.9\t88.7\n-49.1\t89.3\n-49.3\t89.9\n-49.5\t90.5\n-49.7\t91.1\n-49.9\t91.7\n-50.1\t92.3\n-50.3\t92.9\n-50.5\t93.5\n-50.7\t94.1\n-50.9\t93.8\n-51.1\t93.5\n-51.3\t93.2\n-51.5\t92.9\n-51.7\t92.6\n-51.9\t92.3\n-52.1\t92\n-52.3\t91.7\n-52.5\t91.4\n-52.7\t91.1\n-52.9\t90.8\n-53.1\t90.5\n-53.3\t90.2\n-53.5\t89.9\n-53.7\t89.6\n-53.9\t89.3\n-54.1\t89\n-54.3\t88.7\n-54.5\t88.4\n-54.7\t88.1\n-54.9\t87.8\n-55.1\t87.5\n-55.3\t87.2\n-55.5\t86.9\n-55.7\t86.6\n-55.9\t86.3\n-56.1\t86\n-56.3\t85.7\n-56.5\t85.4\n-56.7\t85.1\n-56.9\t84.8\n-57.1\t84.5\n-57.3\t84.2\n-57.5\t83.9\n-57.7\t83.6\n-57.9\t83.3\n-58.1\t83\n-58.3\t82.7\n-58.5\t82.4\n-58.7\t82.1\n-58.9\t81.8\n-59.1\t81.5\n-59.3\t81.2\n-59.5\t80.9\n-59.7\t80.6\n-59.9\t80.3\n-60.1\t80\n-60.3\t79.7\n-60.5\t79.4\n-60.7\t79.1\n-60.9\t78.8\n-61.1\t78.5\n-61.3\t78.2\n-61.5\t77.9\n-61.7\t77.6\n-61.9\t77.3\n-62.1\t77\n-62.3\t76.7\n-62.5\t76.4\n-62.7\t76.1\n-62.9\t75.8\n-63.1\t75.5\n-63.3\t75.2\n-63.5\t74.9\n-63.7\t74.6\n-63.9\t74.3\n-64.1\t74\n-64.3\t73.7\n-64.5\t73.4\n-64.7\t73.1\n-64.9\t72.8\n-65.1\t72.5\n-65.3\t72.2\n-65.5\t71.9\n-65.7\t71.6\n-65.9\t71.3\n-66.1\t71\n-66.3\t70.7\n-66.5\t70.4\n-66.7\t70.1\n-66.9\t69.8\n-67.1\t69.5\n-67.3\t69.2\n-67.5\t68.9\n-67.2\t68.6\n-66.9\t68.3\n-66.6\t68\n-66.3\t67.7\n-66\t67.4\n-65.7\t67.1\n-65.4\t66.8\n-65.1\t66.5\n-64.8\t66.2\n-64.5\t65.9\n-64.2\t65.6\n-63.9\t65.3\n-63.6\t65\n-63.3\t64.7\n-63\t64.4\n-62.7\t64.1\n-62.4\t63.8\n-62.1\t63.5\n-61.8\t63.2\n-61.5\t62.9\n-61.2\t62.6\n-60.9\t62.3\n-60.6\t62\n-60.3\t61.7\n-60\t61.4\n-59.7\t61.1\n-59.4\t60.8\n-59.1\t60.5\n-58.8\t60.2\n-58.5\t59.9\n-58.2\t59.6\n-57.9\t59.3\n-57.6\t59\n-57.3\t58.7\n-57\t58.4\n-56.7\t58.1\n-56.4\t57.8\n-56.1\t57.5\n-55.8\t57.2\n-55.5\t56.9\n-55.2\t56.6\n-54.9\t56.3\n-54.6\t56\n-54.3\t55.7\n-54\t55.4\n-53.7\t55.1\n-53.4\t54.8\n-53.1\t54.5\n-52.8\t54.2\n-52.5\t53.9\n-52.2\t53.6\n-51.9\t53.3\n-51.6\t53\n-51.3\t52.7\n-51\t52.4\n-50.7\t52.1\n-50.4\t51.8\n-50.1\t51.5\n-49.8\t51.2\n-49.5\t50.9\n-49.2\t50.6\n-48.9\t50.3\n-48.6\t50\n-48.3\t49.7\n-48\t49.4\n-47.7\t49.1\n-47.4\t48.8\n-47.1\t48.5\n-46.8\t48.2\n-46.5\t47.9\n-46.2\t47.6\n-45.9\t47.3\n-45.6\t47\n-45.3\t46.7\n-45\t46.4\n-44.7\t46.1\n-44.4\t45.8\n-44.1\t45.5\n-43.8\t45.2\n-43.5\t44.9\n-43.2\t44.6\n-42.9\t44.3\n-42.6\t44\n-42.3\t43.7\n-42\t43.4\n-41.7\t43.1\n-41.4\t42.8\n-41.1\t42.5\n-40.8\t42.2\n-40.5\t41.9\n-40.2\t41.6\n-39.9\t41.3\n-39.6\t41\n-39.3\t40.7\n-39\t40.4\n-38.7\t40.1\n-38.4\t39.8\n-38.1\t39.5\n-37.8\t39.2\n-37.5\t38.9\n-37.2\t38.6\n-36.9\t38.3\n-36.6\t38\n-36.3\t37.7\n-36\t37.4\n-35.7\t37.1\n-35.4\t36.8\n-35.1\t36.5\n-34.8\t36.2\n-34.5\t35.9\n-34.2\t35.6\n-33.9\t35.3\n-33.6\t35\n-33.3\t34.7\n-33\t34.4\n-32.7\t34.1\n-32.4\t33.8\n-32.1\t33.5\n-31.8\t33.2\n-31.5\t32.9\n-31.2\t32.6\n-30.9\t32.3\n-30.6\t32\n-30.3\t31.7\n-30\t31.4\n-29.7\t31.1\n-29.4\t30.8\n-29.1\t30.5\n-28.8\t30.2\n-28.5\t29.9\n-28.2\t29.6\n-27.9\t29.3\n-27.6\t29\n-27.3\t28.7\n-27\t28.4\n-26.7\t28.1\n-26.4\t27.8\n-26.1\t27.5\n-25.8\t27.2\n-25.5\t26.9\n-25.2\t26.6\n-24.9\t26.3\n-24.6\t26\n-24.3\t25.7\n-24\t25.4\n-23.7\t25.1\n-23.4\t24.8\n-23.1\t24.5\n-22.8\t24.2\n-22.5\t23.9\n-22.2\t23.6\n-21.9\t23.3\n-21.6\t23\n-21.3\t22.7\n-21\t22.4\n-20.7\t22.1\n-20.4\t21.8\n-20.1\t21.5\n-19.8\t21.2\n-19.5\t20.9\n-19.2\t20.6\n-18.9\t20.3\n-18.6\t20\n-18.3\t19.7\n-18\t19.4\n-17.7\t19.1\n-17.4\t18.8\n-17.1\t18.5\n-16.8\t18.2\n-16.5\t17.9\n-16.2\t17.6\n-15.9\t17.3\n-15.6\t17\n-15.3\t16.7\n-15\t16.4\n-14.7\t16.1\n-14.4\t15.8\n-14.1\t15.5\n-13.8\t15.2\n-13.5\t14.9\n-13.2\t14.6\n-12.9\t14.3\n-12.6\t14\n-12.3\t13.7\n-12\t13.4\n-11.7\t13.1\n-11.4\t12.8\n-11.1\t12.5\n-10.8\t12.2\n-10.5\t11.9\n-10.2\t11.6\n-9.9\t11.3\n-9.6\t11\n-9.3\t10.7\n-9\t10.4\n-8.7\t10.1\n-8.4\t9.8\n-8.1\t9.5\n-7.8\t9.2\n-7.5\t8.9\n-7.2\t8.6\n-6.9\t8.3\n-6.6\t8\n-6.3\t7.7\n-6\t7.4\n-5.7\t7.1\n-5.4\t6.8\n-5.1\t6.5\n-4.8\t6.2\n-4.5\t5.9\n-4.2\t5.6\n-3.9\t5.3\n-3.6\t5\n-3.3\t4.7\n-3\t4.4\n-2.7\t4.1\n-2.4\t3.8\n-2.1\t3.5\n-1.8\t3.2\n-1.5\t2.9\n-1.2\t2.6\n-0.9\t2.3\n-0.6\t2\n-0.3\t1.7\n-1.20559E-12\t1.4\n0.3\t1.1\n0.6\t0.8\n0.9\t0.5\n1.2\t0.2\n1.5\t-0.1\n1.8\t-0.4\n2.1\t-0.7\n2.4\t-1\n2.7\t-1.3\n3\t-1.6\n3.3\t-1.9\n3.6\t-2.2\n3.9\t-2.5\n4.2\t-2.8\n4.5\t-3.1\n4.8\t-3.4\n5.1\t-3.7\n5.4\t-4\n5.7\t-4.3\n6\t-4.6\n6.3\t-4.9\n6.6\t-5.2\n6.9\t-5.5\n7.2\t-5.8\n7.5\t-6.1\n7.8\t-6.4\n8.1\t-6.7\n8.4\t-7\n8.7\t-7.3\n9\t-7.6\n9.3\t-7.9\n9.6\t-8.2\n9.9\t-8.5\n10.2\t-8.8\n10.5\t-9.1\n10.8\t-9.4\n11.1\t-9.7\n11.4\t-10\n11.7\t-10.3\n12\t-10.6\n12.3\t-10.9\n12.6\t-11.2\n12.9\t-11.5\n13.2\t-11.8\n13.5\t-12.1\n13.8\t-12.4\n14.1\t-12.7\n14.4\t-13\n14.7\t-13.3\n15\t-13.6\n15.3\t-13.9\n15.6\t-14.2\n15.9\t-14.5\n16.2\t-14.8\n16.5\t-15.1\n16.8\t-15.4\n17.1\t-15.7\n17.4\t-16\n17.7\t-16.3\n18\t-16.6\n18.3\t-16.9\n18.6\t-17.2\n18.9\t-17.5\n19.2\t-17.8\n19.5\t-18.1\n19.8\t-18.4\n20.1\t-18.7\n20.4\t-19\n20.7\t-19.3\n21\t-19.6\n21.3\t-19.9\n21.6\t-20.2\n21.9\t-20.5\n22.2\t-20.8\n22.1\t-21.1\n22\t-21.4\n21.9\t-21.7\n21.8\t-22\n21.7\t-22.3\n21.6\t-22.6\n21.5\t-22.9\n21.4\t-23.2\n21.3\t-23.5\n21.2\t-23.8\n21.1\t-24.1\n21\t-24.4\n20.9\t-24.7\n20.8\t-25\n20.7\t-25.3\n20.6\t-25.6\n20.5\t-25.9\n20.4\t-26.2\n20.3\t-26.5\n20.2\t-26.8\n20.1\t-27.1\n20\t-27.4\n19.9\t-27.7\n19.8\t-28\n19.7\t-28.3\n19.6\t-28.6\n19.5\t-28.9\n19.4\t-29.2\n19.3\t-29.5\n19.2\t-29.8\n19.1\t-30.1\n19\t-30.4\n18.9\t-30.7\n18.8\t-31\n18.7\t-31.3\n18.6\t-31.6\n18.5\t-31.9\n18.4\t-32.2\n18.3\t-32.5\n18.2\t-32.8\n18.1\t-33.1\n18\t-33.4\n17.9\t-33.7\n17.8\t-34\n17.7\t-34.3\n17.6\t-34.6\n17.5\t-34.9\n17.4\t-35.2\n17.3\t-35.5\n17.2\t-35.8\n17.1\t-36.1\n17\t-36.4\n16.9\t-36.7\n16.8\t-37\n16.7\t-37.3\n16.6\t-37.6\n16.5\t-37.9\n16.4\t-38.2\n16.3\t-38.5\n16.2\t-38.8\n16.1\t-39.1\n16\t-39.4\n15.9\t-39.7\n15.8\t-40\n15.7\t-40.3\n15.6\t-40.6\n15.5\t-40.9\n15.4\t-41.2\n15.3\t-41.5\n15.2\t-41.8\n15.1\t-42.1\n15\t-42.4\n14.9\t-42.7\n14.8\t-43\n14.7\t-43.3\n14.6\t-43.6\n14.5\t-43.9\n14.4\t-44.2\n14.3\t-44.5\n14.2\t-44.8\n14.1\t-45.1\n14\t-45.4\n13.9\t-45.7\n13.8\t-46\n13.7\t-46.3\n13.6\t-46.6\n13.5\t-46.9\n13.4\t-47.2\n13.3\t-47.5\n13.2\t-47.8\n13.1\t-48.1\n13\t-48.4\n12.9\t-48.7\n12.8\t-49\n12.7\t-49.3\n12.6\t-49.6\n12.5\t-49.9\n12.4\t-50.2\n12.3\t-50.5\n12.2\t-50.8\n12.1\t-51.1\n12\t-51.4\n11.9\t-51.7\n11.8\t-52\n11.7\t-52.3\n11.6\t-52.6\n11.5\t-52.9\n11.4\t-53.2\n11.3\t-53.5\n11.2\t-53.8\n11.1\t-54.1\n11\t-54.4\n10.9\t-54.7\n10.8\t-55\n10.7\t-55.3\n10.6\t-55.6\n10.5\t-55.9\n10.4\t-56.2\n10.3\t-56.5\n10.2\t-56.8\n10.1\t-57.1\n10\t-57.4\n9.9\t-57.7\n9.8\t-58\n9.7\t-58.3\n9.6\t-58.6\n9.5\t-58.9\n9.4\t-59.2\n9.3\t-59.5\n9.2\t-59.8\n9.1\t-60.1\n9\t-60.4\n8.9\t-60.7\n8.8\t-61\n8.7\t-61.3\n8.6\t-61.6\n8.5\t-61.9\n8.4\t-62.2\n8.3\t-62.5\n8.2\t-62.8\n8.1\t-63.1\n8\t-63.4\n7.9\t-63.7\n7.8\t-64\n7.7\t-64.3\n7.6\t-64.6\n7.5\t-64.9\n7.4\t-65.2\n7.3\t-65.5\n7.2\t-65.8\n7.1\t-66.1\n7\t-66.4\n6.9\t-65.8\n6.8\t-65.2\n6.7\t-64.6\n6.6\t-64\n6.5\t-63.4\n6.4\t-62.8\n6.3\t-62.2\n6.2\t-61.6\n6.1\t-61\n6\t-60.4\n5.9\t-59.8\n5.8\t-59.2\n5.7\t-58.6\n5.6\t-58\n5.5\t-57.4\n5.4\t-56.8\n5.3\t-56.2\n5.2\t-55.6\n5.1\t-55\n5\t-54.4\n4.9\t-53.8\n4.8\t-53.2\n4.7\t-52.6\n4.6\t-52\n4.5\t-51.4\n4.4\t-50.8\n4.3\t-50.2\n4.2\t-49.6\n4.1\t-49\n4\t-48.4\n3.9\t-47.8\n3.8\t-47.2\n3.7\t-46.6\n3.6\t-46\n3.5\t-45.4\n3.4\t-44.8\n3.3\t-44.2\n3.2\t-43.6\n3.1\t-43\n3\t-42.4\n2.9\t-41.8\n2.8\t-41.2\n2.7\t-40.6\n2.6\t-40\n2.5\t-39.4\n2.4\t-38.8\n2.3\t-38.2\n2.2\t-37.6\n2.1\t-37\n2\t-36.4\n1.9\t-35.8\n1.8\t-35.2\n1.7\t-34.6\n1.6\t-34\n1.5\t-33.4\n1.4\t-32.8\n1.3\t-32.2\n1.2\t-31.6\n1.1\t-31\n1\t-30.4\n0.9\t-29.8\n0.8\t-29.2\n0.7\t-28.6\n0.6\t-28\n0.5\t-27.4\n0.4\t-26.8\n0.3\t-26.2\n0.2\t-25.6\n0.1\t-25\n0\t-24.4\n-0.1\t-23.8\n-0.2\t-23.2\n-0.3\t-22.6\n-0.4\t-22\n-0.5\t-21.4\n-0.6\t-20.8\n-0.7\t-20.2\n-0.8\t-19.6\n-0.9\t-19\n-1\t-18.4\n-1.1\t-17.8\n-1.2\t-17.2\n-1.3\t-16.6\n-1.4\t-16\n-1.5\t-15.4\n-1.6\t-14.8\n-1.7\t-14.2\n-1.8\t-13.6\n-1.9\t-13\n-2\t-12.4\n-2.1\t-11.8\n-2.2\t-11.2\n-2.3\t-10.6\n-2.4\t-10\n-2.5\t-9.4\n-2.6\t-8.8\n-2.7\t-8.2\n-2.8\t-7.6\n-2.9\t-7\n-3\t-6.4\n-3.1\t-5.8\n-3.2\t-5.2\n-3.3\t-4.6\n-3.4\t-4\n-3.5\t-3.4\n-3.6\t-2.8\n-3.7\t-2.2\n-3.8\t-1.6\n-3.9\t-1\n-4\t-0.4\n-4.1\t0.2\n-4.2\t0.8\n-4.3\t1.4\n-4.4\t2\n-4.5\t2.6\n-4.6\t3.2\n-4.7\t3.8\n-4.8\t4.4\n-4.9\t5\n-5\t5.6\n-5.1\t6.2\n-5.2\t6.8\n-5.3\t7.4\n-5.4\t8\n-5.5\t8.6\n-5.6\t9.2\n-5.7\t9.8\n-5.8\t10.4\n-5.9\t11\n-6\t11.6\n-6.1\t12.2\n-6.2\t12.8\n-6.3\t13.4\n-6.4\t14\n-6.5\t14.6\n-6.6\t15.2\n-6.7\t15.8\n-6.8\t16.4\n-6.9\t17\n-7\t17.6\n-7.1\t18.2\n-7.2\t18.8\n-7.3\t19.4\n-7.4\t20\n-7.5\t20.6\n-7.6\t21.2\n-7.7\t21.8\n-7.8\t22.4\n-7.9\t23\n-8\t23.6\n-8.1\t24.2\n-8.2\t24.8\n-8.3\t25.4\n-8.4\t26\n-8.5\t26.6\n-8.6\t27.2\n-8.7\t27.8\n-8.8\t28.4\n-8.9\t29\n-9\t29.6\n-9.1\t30.2\n-9.2\t30.8\n-9.3\t31.4\n-9.4\t32\n-9.5\t32.6\n-9.6\t33.2\n-9.7\t33.8\n-9.8\t34.4\n-9.9\t35\n-10\t35.6\n-10.1\t36.2\n-10.2\t36.8\n-10.3\t37.4\n-10.4\t38\n-10.5\t38.6\n-10.6\t39.2\n-10.7\t39.8\n-10.8\t40.4\n-10.9\t40.1\n-11\t39.8\n-11.1\t39.5\n-11.2\t39.2\n-11.3\t38.9\n-11.4\t38.6\n-11.5\t38.3\n-11.6\t38\n-11.7\t37.7\n-11.8\t37.4\n-11.9\t37.1\n-12\t36.8\n-12.1\t36.5\n-12.2\t36.2\n-12.3\t35.9\n-12.4\t35.6\n-12.5\t35.3\n-12.8\t35\n-13.1\t34.7\n-13.4\t34.4\n-13.7\t34.1\n-14\t33.8\n-14.3\t33.5\n-14.6\t33.2\n-14.9\t32.9\n-15.2\t32.6\n-15.5\t32.3\n-15.8\t32\n-16.1\t31.7\n-16.4\t31.4\n-16.7\t31.1\n-17\t30.8\n-17.3\t30.5\n-17.6\t30.2\n-17.9\t29.9\n-18.2\t29.6\n-18.5\t29.3\n-18.8\t29\n-19.1\t28.7\n-19.4\t28.4\n-19.7\t28.1\n-20\t27.8\n-20.3\t27.5\n-20.6\t27.2\n-20.9\t26.9\n-21.2\t26.6\n-21.5\t26.3\n-21.8\t26\n-22.1\t25.7\n-22.4\t25.4\n-22.7\t25.1\n-23\t24.8\n-23.3\t24.5\n-23.6\t24.2\n-23.9\t23.9\n-24.2\t23.6\n-24.5\t23.3\n-24.8\t23\n-25.1\t22.7\n-25.4\t22.4\n-25.7\t22.1\n-26\t21.8\n-26.3\t21.5\n-26.6\t21.2\n-26.9\t20.9\n-27.2\t20.6\n-27.5\t20.3\n-27.8\t20\n-28.1\t19.7\n-28.4\t19.4\n-28.7\t19.1\n-29\t18.8\n-29.3\t18.5\n-29.6\t18.2\n-29.9\t17.9\n-30.2\t17.6\n-30.5\t17.3\n-30.8\t17\n-31.1\t16.7\n-31.4\t16.4\n-31.7\t16.1\n-32\t15.8\n-32.3\t15.5\n-32.6\t15.2\n-32.9\t14.9\n-33.2\t14.6\n-33.5\t14.3\n-33.8\t14\n-34.1\t13.7\n-34.4\t13.4\n-34.7\t13.1\n-35\t12.8\n-35.3\t12.5\n-35.6\t12.2\n-35.9\t11.9\n-36.2\t11.6\n-36.5\t11.3\n-36.8\t11\n-37.1\t10.7\n-37.4\t10.4\n-37.7\t10.1\n-38\t9.8\n-38.3\t9.5\n-38.6\t9.2\n-38.9\t8.9\n-39.2\t8.6\n-39.5\t8.3\n-39.8\t8\n-40.1\t7.7\n-40.4\t7.4\n-40.7\t7.1\n-41\t6.8\n-41.3\t6.5\n-41.6\t6.2\n-41.9\t5.9\n-42.2\t5.6\n-42.5\t5.3\n-42.8\t5\n-43.1\t4.7\n-43.4\t4.4\n-43.7\t4.1\n-44\t3.8\n-44.3\t3.5\n-44.6\t3.2\n-44.9\t2.9\n-45.2\t2.6\n-45.5\t2.3\n-45.8\t2\n-46.1\t1.7\n-46.4\t1.4\n-46.7\t1.1\n-47\t0.8\n-47.3\t0.5\n-47.6\t0.2\n-47.9\t-0.1\n-48.2\t-0.4\n-48.5\t-0.7\n-48.8\t-1\n-49.1\t-1.3\n-49.4\t-1.6\n-49.7\t-1.9\n-50\t-2.2\n-50.3\t-2.5\n-50.6\t-2.8\n-50.9\t-3.1\n-51.2\t-3.4\n-51.5\t-3.7\n-51.8\t-4\n-52.1\t-4.3\n-52.4\t-4.6\n-52.7\t-4.9\n-53\t-5.2\n-53.3\t-5.5\n-53.6\t-5.8\n-53.9\t-6.1\n-54.2\t-6.4\n-54.5\t-6.7\n-54.8\t-7\n-55.1\t-7.3\n-55.4\t-7.6\n-55.7\t-7.9\n-56\t-8.2\n-56.3\t-8.5\n-56.6\t-8.8\n-56.9\t-9.1\n-57.2\t-9.4\n-57.5\t-9.7\n-57.8\t-10\n-58.1\t-10.3\n-58.4\t-10.6\n-58.7\t-10.9\n-59\t-11.2\n-59.3\t-11.5\n-59.6\t-11.8\n-59.9\t-12.1\n-60.2\t-12.4\n-60.5\t-12.7\n-60.8\t-13\n-61.1\t-13.3\n-61.4\t-13.6\n-61.7\t-13.9\n-62\t-14.2\n-62.3\t-14.5\n-62.6\t-14.8\n-62.9\t-15.1\n-63.2\t-15.4\n-63.5\t-15.7\n-63.8\t-16\n-64.1\t-16.3\n-64.4\t-16.6\n-64.7\t-16.9\n-65\t-17.2\n-65.3\t-17.5\n-65.6\t-17.8\n-65.9\t-18.1\n-66.2\t-18.4\n-66.5\t-18.7\n-66.8\t-19\n-67.1\t-19.3\n-67.4\t-19.6\n-67.7\t-19.9\n-68\t-20.2\n-68.3\t-20.5\n-68.6\t-20.8\n-68.9\t-21.1\n-69.2\t-21.4\n-69.5\t-21.7\n-69.8\t-22\n-70.1\t-22.3\n-70.4\t-22.6\n-70.7\t-22.9\n-71\t-23.2\n-71.3\t-23.5\n-71.6\t-23.8\n-71.9\t-24.1\n-72.2\t-24.4\n-72.5\t-24.7\n-72.8\t-25\n-73.1\t-25.3\n-73.4\t-25.6\n-73.7\t-25.9\n-74\t-26.2\n-74.3\t-26.5\n-74.6\t-26.8\n-74.9\t-27.1\n-75.2\t-27.4\n-75.5\t-27.7\n-75.8\t-28\n-76.1\t-28.3\n-76.4\t-28.6\n-76.7\t-28.9\n-77\t-29.2\n-77.3\t-29.5\n-77.6\t-29.8\n-77.9\t-30.1\n-78.2\t-30.4\n-78.5\t-30.7\n-78.8\t-31\n-79.1\t-31.3\n-79.4\t-31.6\n-79.7\t-31.9\n-80\t-32.2\n-80.3\t-32.5\n-80.6\t-32.8\n-80.9\t-33.1\n-81.2\t-33.4\n-81.5\t-33.7\n-81.8\t-34\n-82.1\t-34.3\n-82.4\t-34.6\n-82.7\t-34.9\n-83\t-35.2\n-83.3\t-35.5\n-83.6\t-35.8\n-83.9\t-36.1\n-84.2\t-36.4\n-84.5\t-36.7\n-84.8\t-37\n-85.1\t-37.3\n-85.4\t-37.6\n-85.7\t-37.9\n-86\t-38.2\n-86.3\t-38.5\n-86.6\t-38.8\n-86.9\t-39.1\n-87.2\t-39.4\n-87.5\t-39.7\n-87.8\t-40\n-88.1\t-40.3\n-88.4\t-40.6\n-88.7\t-40.9\n-89\t-41.2\n-88.4\t-41.5\n-87.8\t-41.8\n-87.2\t-42.1\n-86.6\t-42.4\n-86\t-42.7\n-85.4\t-43\n-84.8\t-43.3\n-84.2\t-43.6\n-83.6\t-43.9\n-83\t-44.2\n-82.4\t-44.5\n-81.8\t-44.8\n-81.2\t-45.1\n-80.6\t-45.4\n-80\t-45.7\n-79.4\t-46\n-78.8\t-46.3\n-78.2\t-46.6\n-77.6\t-46.9\n-77\t-47.2\n-76.4\t-47.5\n-75.8\t-47.8\n-75.2\t-48.1\n-74.6\t-48.4\n-74\t-48.7\n-73.4\t-49\n-72.8\t-49.3\n-72.2\t-49.6\n-71.6\t-49.9\n-71\t-50.2\n-70.4\t-50.5\n-69.8\t-50.8\n-69.2\t-51.1\n-68.6\t-51.4\n-68\t-51.7\n-67.4\t-52\n-66.8\t-52.3\n-66.2\t-52.6\n-65.6\t-52.9\n-65\t-53.2\n-64.4\t-53.5\n-63.8\t-53.8\n-63.2\t-54.1\n-62.6\t-54.4\n-62\t-54.7\n-61.4\t-55\n-60.8\t-55.3\n-60.2\t-55.6\n-59.6\t-55.9\n-59\t-56.2\n-58.4\t-56.5\n-57.8\t-56.8\n-57.2\t-57.1\n-56.6\t-57.4\n-56\t-57.7\n-55.4\t-58\n-54.8\t-58.3\n-54.2\t-58.6\n-53.6\t-58.9\n-53\t-59.2\n-52.4\t-59.5\n-51.8\t-59.8\n-51.2\t-60.1\n-50.6\t-60.4\n-50\t-60.7\n-49.4\t-61\n-48.8\t-61.3\n-48.2\t-61.6\n-47.6\t-61.9\n-47\t-62.2\n-46.4\t-62.5\n-45.8\t-62.8\n-45.2\t-63.1\n-44.6\t-63.4\n-44\t-63.7\n-43.4\t-64\n-42.8\t-64.3\n-42.2\t-64.6\n-41.6\t-64.9\n-41\t-65.2\n-40.4\t-65.5\n-39.8\t-65.8\n-39.2\t-66.1\n-38.6\t-66.4\n-38\t-66.7\n-37.4\t-67\n-36.8\t-67.3\n-36.2\t-67.6\n-35.6\t-67.9\n-35\t-68.2\n-34.4\t-68.5\n-33.8\t-68.8\n-33.2\t-69.1\n-32.6\t-69.4\n-32\t-69.7\n-31.4\t-70\n-30.8\t-70.3\n-30.2\t-70.6\n-29.6\t-70.9\n-29\t-71.2\n-28.4\t-71.5\n-27.8\t-71.8\n-27.2\t-72.1\n-26.6\t-72.4\n-26\t-72.7\n-25.4\t-73\n-24.8\t-73.3\n-24.2\t-73.6\n-23.6\t-73.9\n-23\t-74.2\n-22.4\t-74.5\n-21.8\t-74.8\n-21.2\t-75.1\n-20.6\t-75.4\n-20\t-75.7\n-19.4\t-76\n-18.8\t-76.3\n-18.2\t-76.6\n-17.6\t-76.9\n-17\t-77.2\n-16.4\t-77.5\n-15.8\t-77.8\n-15.2\t-78.1\n-14.6\t-78.4\n-14\t-78.7\n-13.4\t-79\n-12.8\t-79.3\n-12.2\t-79.6\n-11.6\t-79.9\n-11\t-80.2\n-10.4\t-80.5\n-9.8\t-80.8\n-9.2\t-81.1\n-8.6\t-81.4\n-8\t-81.7\n-7.4\t-82\n-6.8\t-82.3\n-6.2\t-82.6\n-5.6\t-82.9\n-5\t-83.2\n-4.4\t-83.5\n-3.8\t-83.8\n-3.2\t-84.1\n-2.6\t-84.4\n-2\t-84.7\n-1.4\t-85\n-0.8\t-85.3\n-0.2\t-85.6\n0.4\t-85.9\n1\t-86.2\n1.6\t-86.5\n2.2\t-86.8\n2.8\t-87.1\n3.4\t-87.4\n4\t-87.7\n4.6\t-88\n5.2\t-88.3\n5.8\t-88.6\n6.4\t-88.9\n7\t-89.2\n7.6\t-89.5\n8.2\t-89.8\n8.8\t-90.1\n9.4\t-90.4\n10\t-90.3\n10.6\t-90.2\n11.2\t-90.1\n11.8\t-90\n12.4\t-89.9\n13\t-89.8\n13.6\t-89.7\n14.2\t-89.6\n14.8\t-89.5\n15.4\t-89.4\n16\t-89.3\n16.6\t-89.2\n17.2\t-89.1\n17.8\t-89\n18.4\t-88.9\n19\t-88.8\n19.6\t-88.7\n20.2\t-88.6\n20.8\t-88.5\n21.4\t-88.4\n22\t-88.3\n22.6\t-88.2\n23.2\t-88.1\n23.8\t-88\n24.4\t-87.9\n25\t-87.8\n25.6\t-87.7\n26.2\t-87.6\n26.8\t-87.5\n27.4\t-87.4\n28\t-87.3\n28.6\t-87.2\n29.2\t-87.1\n29.8\t-87\n30.4\t-86.9\n31\t-86.8\n31.6\t-86.7\n32.2\t-86.6\n32.8\t-86.5\n33.4\t-86.4\n34\t-86.3\n34.6\t-86.2\n35.2\t-86.1\n35.8\t-86\n36.4\t-85.9\n37\t-85.8\n37.6\t-85.7\n38.2\t-85.6\n38.8\t-85.5\n39.4\t-85.4\n40\t-85.3\n40.6\t-85.2\n41.2\t-85.1\n41.8\t-85\n42.4\t-84.9\n43\t-84.8\n43.6\t-84.7\n44.2\t-84.6\n44.8\t-84.5\n45.4\t-84.4\n46\t-84.3\n46.6\t-84.2\n47.2\t-84.1\n47.8\t-84\n48.4\t-83.9\n49\t-83.8\n49.6\t-83.7\n50.2\t-83.6\n50.8\t-83.5\n51.4\t-83.4\n52\t-83.3\n52.6\t-83.2\n53.2\t-83.1\n53.8\t-83\n54.4\t-82.9\n55\t-82.8\n55.6\t-82.7\n56.2\t-82.6\n56.8\t-82.5\n57.4\t-82.4\n58\t-82.3\n58.6\t-82.2\n59.2\t-82.1\n59.8\t-82\n60.4\t-81.9\n61\t-81.8\n61.6\t-81.7\n62.2\t-81.6\n62.8\t-81.5\n63.4\t-81.4\n64\t-81.3\n64.6\t-81.2\n65.2\t-81.1\n65.8\t-81\n66.4\t-80.9\n67\t-80.8\n67.6\t-80.7\n68.2\t-80.6\n68.8\t-80.5\n69.4\t-80.4\n70\t-80.3\n70.6\t-80.2\n71.2\t-80.1\n71.8\t-80\n72.4\t-79.9\n73\t-79.8\n73.6\t-79.7\n74.2\t-79.6\n74.8\t-79.5\n75.4\t-79.4\n76\t-79.3\n76.6\t-79.2\n77.2\t-79.1\n77.8\t-79\n78.4\t-78.9\n79\t-78.8\n79.6\t-78.7\n80.2\t-78.6\n80.8\t-78.5\n81.4\t-78.4\n82\t-78.3\n82.6\t-78.2\n83.2\t-78.1\n83.8\t-78\n84.4\t-77.9\n84\t-77.8\n83.6\t-77.7\n83.2\t-77.6\n82.8\t-77.5\n82.4\t-77.4\n82\t-77.3\n81.6\t-77.2\n81.2\t-77.1\n80.8\t-77\n80.4\t-76.9\n80\t-76.8\n79.6\t-76.7\n79.2\t-76.6\n78.8\t-76.5\n78.4\t-76.4\n78\t-76.3\n77.6\t-76.2\n77.2\t-76.1\n76.8\t-76\n76.4\t-75.9\n76\t-75.8\n75.6\t-75.7\n75.2\t-75.6\n74.8\t-75.5\n74.4\t-75.4\n74\t-75.3\n73.6\t-75.2\n73.2\t-75.1\n72.8\t-75\n72.4\t-74.9\n72\t-74.8\n71.6\t-74.7\n71.2\t-74.6\n70.8\t-74.5\n70.4\t-74.4\n70\t-74.3\n69.6\t-74.2\n69.2\t-74.1\n68.8\t-74\n68.4\t-73.9\n68\t-73.8\n67.6\t-73.7\n67.2\t-73.6\n66.8\t-73.5\n66.4\t-73.4\n66\t-73.3\n65.6\t-73.2\n65.2\t-73.1\n64.8\t-73\n64.4\t-72.9\n64\t-72.8\n63.6\t-72.7\n63.2\t-72.6\n62.8\t-72.5\n62.4\t-72.4\n62\t-72.3\n61.6\t-72.2\n61.2\t-72.1\n60.8\t-72\n60.4\t-71.9\n60\t-71.8\n59.6\t-71.7\n59.2\t-71.6\n58.8\t-71.5\n58.4\t-71.4\n58\t-71.3\n57.6\t-71.2\n57.2\t-71.1\n56.8\t-71\n56.4\t-70.9\n56\t-70.8\n55.6\t-70.7\n55.2\t-70.6\n54.8\t-70.5\n54.4\t-70.4\n54\t-70.3\n53.6\t-70.2\n53.2\t-70.1\n52.8\t-70\n52.4\t-69.9\n52\t-69.8\n51.6\t-69.7\n51.2\t-69.6\n50.8\t-69.5\n50.4\t-69.4\n50\t-69.3\n49.6\t-69.2\n49.2\t-69.1\n48.8\t-69\n48.4\t-68.9\n48\t-68.8\n47.6\t-68.7\n47.2\t-68.6\n46.8\t-68.5\n46.4\t-68.4\n46\t-68.3\n45.6\t-68.2\n45.2\t-68.1\n44.8\t-68\n44.4\t-67.9\n44\t-67.8\n43.6\t-67.7\n43.2\t-67.6\n42.8\t-67.5\n42.4\t-67.4\n42\t-67.3\n41.6\t-67.2\n41.2\t-67.1\n40.8\t-67\n40.4\t-66.9\n40\t-66.8\n39.6\t-66.7\n39.2\t-66.6\n38.8\t-66.5\n38.4\t-66.4\n38\t-66.3\n37.6\t-66.2\n37.2\t-66.1\n36.8\t-66\n36.4\t-65.9\n36\t-65.8\n35.6\t-65.7\n35.2\t-65.6\n34.8\t-65.5\n34.4\t-65.4\n34\t-65.1\n33.6\t-64.8\n33.2\t-64.5\n32.8\t-64.2\n32.4\t-63.9\n32\t-63.6\n31.6\t-63.3\n31.2\t-63\n30.8\t-62.7\n30.4\t-62.4\n30\t-62.1\n29.6\t-61.8\n29.2\t-61.5\n28.8\t-61.2\n28.4\t-60.9\n28\t-60.6\n27.6\t-60.3\n27.2\t-60\n26.8\t-59.7\n26.4\t-59.4\n26\t-59.1\n25.6\t-58.8\n25.2\t-58.5\n24.8\t-58.2\n24.4\t-57.9\n24\t-57.6\n23.6\t-57.3\n23.2\t-57\n22.8\t-56.7\n22.4\t-56.4\n22\t-56.1\n21.6\t-55.8\n21.2\t-55.5\n20.8\t-55.2\n20.4\t-54.9\n20\t-54.6\n19.6\t-54.3\n19.2\t-54\n18.8\t-53.7\n18.4\t-53.4\n18\t-53.1\n17.6\t-52.8\n17.2\t-52.5\n16.8\t-52.2\n16.4\t-51.9\n16\t-51.6\n15.6\t-51.3\n15.2\t-51\n14.8\t-50.7\n14.4\t-50.4\n14\t-50.1\n13.6\t-49.8\n13.2\t-49.5\n12.8\t-49.2\n12.4\t-48.9\n12\t-48.6\n11.6\t-48.3\n11.2\t-48\n10.8\t-47.7\n10.4\t-47.4\n10\t-47.1\n9.6\t-46.8\n9.2\t-46.5\n8.8\t-46.2\n8.4\t-45.9\n8\t-45.6\n7.6\t-45.3\n7.2\t-45\n6.8\t-44.7\n6.4\t-44.4\n6\t-44.1\n5.6\t-43.8\n5.2\t-43.5\n4.8\t-43.2\n4.4\t-42.9\n4\t-42.6\n3.6\t-42.3\n3.2\t-42\n2.8\t-41.7\n2.4\t-41.4\n2\t-41.1\n1.6\t-40.8\n1.2\t-40.5\n0.8\t-40.2\n0.4\t-39.9\n1.74638E-13\t-39.6\n-0.4\t-39.3\n-0.8\t-39\n-1.2\t-38.7\n-1.6\t-38.4\n-2\t-38.1\n-2.4\t-37.8\n-2.8\t-37.5\n-3.2\t-37.2\n-3.6\t-36.9\n-4\t-36.6\n-4.4\t-36.3\n-4.8\t-36\n-5.2\t-35.7\n-5.6\t-35.4\n-6\t-35.1\n-6.4\t-34.8\n-6.8\t-34.5\n-7.2\t-34.2\n-7.6\t-33.9\n-8\t-33.6\n-8.4\t-33.3\n-8.8\t-33\n-9.2\t-32.7\n-9.6\t-32.4\n-10\t-32.1\n-10.4\t-31.8\n-10.8\t-31.5\n-11.2\t-31.2\n-11.6\t-30.9\n-12\t-30.6\n-12.4\t-30.3\n-12.8\t-30\n-13.2\t-29.7\n-13.6\t-29.4\n-14\t-29.1\n-14.4\t-28.8\n-14.8\t-28.5\n-15.2\t-28.2\n-15.6\t-27.9\n-16\t-27.6\n-16.4\t-27.3\n-16.8\t-27\n-17.2\t-26.7\n-17.6\t-26.4\n-18\t-26.1\n-18.4\t-25.8\n-18.8\t-25.5\n-19.2\t-25.2\n-19.6\t-24.9\n-20\t-24.6\n-20.4\t-24.3\n-20.8\t-24\n-21.2\t-23.7\n-21.6\t-23.4\n-22\t-23.1\n-22.4\t-22.8\n-22.8\t-22.5\n-23.2\t-22.2\n-23.6\t-21.9\n-24\t-21.6\n-24.4\t-21.3\n-24.8\t-21\n-25.2\t-20.7\n-25.6\t-20.4\n-26\t-20.1\n-26.4\t-19.8\n-26.8\t-19.5\n-27.2\t-19.2\n-27.6\t-18.9\n-28\t-18.6\n-28.4\t-18.3\n-28.8\t-18\n-29.2\t-17.7\n-29.6\t-17.4\n-30\t-17.1\n-30.4\t-16.8\n-30.8\t-16.5\n-31.2\t-16.2\n-31.6\t-15.9\n-32\t-15.6\n-32.4\t-15.3\n-32.8\t-15\n-33.2\t-14.7\n-33.6\t-14.4\n-34\t-14.1\n-34.4\t-13.8\n-34.8\t-13.5\n-35.2\t-13.2\n-35.6\t-12.9\n-36\t-12.6\n-36.4\t-12.3\n-36.8\t-12\n-37.2\t-11.7\n-37.6\t-11.4\n-38\t-11.1\n-38.4\t-10.8\n-38.8\t-10.5\n-39.2\t-10.2\n-39.6\t-9.9\n-40\t-9.6\n-40.4\t-9.3\n-40.8\t-9\n-41.2\t-8.7\n-41.6\t-8.4\n-42\t-8.1\n-42.4\t-7.8\n-42.8\t-7.5\n-43.2\t-7.2\n-43.6\t-6.9\n-44\t-6.6\n-44.4\t-6.3\n-44.8\t-6\n-45.2\t-5.7\n-45.6\t-5.4\n-46\t-5.1\n-46.4\t-4.8\n-46.8\t-4.5\n-47.2\t-4.2\n-47.6\t-3.9\n-48\t-3.6\n-48.4\t-3.3\n-48.8\t-3\n-49.2\t-2.7\n-49.6\t-2.4\n-50\t-2.1\n-50.4\t-1.8\n-50.8\t-1.5\n-51.2\t-1.2\n-51.6\t-0.9\n-52\t-0.6\n-52.4\t-0.3\n-52.8\t-1.83087E-12\n-53.2\t0.3\n-53.6\t0.6\n-54\t0.9\n-54.4\t1.2\n-54.8\t1.5\n-55.2\t1.8\n-55.6\t2.1\n-56\t2.4\n-56.4\t2.7\n-56.8\t3\n-57.2\t3.3\n-57.6\t3.6\n-58\t3.9\n-58.4\t4.2\n-58.8\t4.5\n-59.2\t4.8\n-59.6\t5.1\n-60\t5.4\n-60.4\t5.7\n-60.8\t6\n-61.2\t6.3\n-61.6\t6.6\n-62\t6.9\n-62.4\t7.2\n-62.8\t7.5\n-63.2\t7.8\n-63.6\t8.1\n-64\t8.4\n-64.4\t8.7\n-64.8\t9\n-65.2\t9.3\n-65.6\t9.6\n-66\t9.9\n-66.4\t10.2\n-66.8\t10.5\n-67.2\t10.8\n-67.6\t11.1\n-68\t11.4\n-68.4\t11.7\n-68.8\t12\n-69.2\t12.3\n-69.6\t12.6\n-70\t12.9\n-70.4\t13.2\n-70.8\t13.5\n-71.2\t13.8\n-71.6\t14.1\n-72\t14.4\n-72.4\t14.7\n-72.8\t15\n-73.2\t15.3\n-73.6\t15.6\n-74\t15.9\n-74.4\t16.2\n-74.8\t16.5\n-75.2\t16.8\n-75.6\t17.1\n-76\t17.4\n-76.4\t17.7\n-76.8\t18\n-77.2\t18.3\n-77.6\t18.6\n-78\t18.9\n-78.4\t19.2\n-78.8\t19.5\n-79.2\t19.8\n-79.6\t20.1\n-80\t20.4\n-80.4\t20.7\n-80.8\t21\n-81.2\t21.3\n-81.6\t21.6\n-82\t21.9\n-82.4\t22.2\n-82.8\t22.5\n-83.2\t22.8\n-83.6\t23.1\n-84\t23.4\n-84.4\t23.7\n-84.8\t24\n-85.2\t24.3\n-85.6\t24.6\n-86\t24.9\n-86.4\t25.2\n-86.8\t25.5\n-87.2\t25.8\n-87.6\t26.1\n-88\t26.4\n-88.4\t26.7\n-88.8\t27\n-89.2\t27.3\n-89.6\t27.6\n-90\t27.9\n-90.4\t28.2\n-90.8\t28.5\n-91.2\t28.8\n-91.6\t29.1\n-92\t29.4\n-92.4\t29.7\n-92.3\t30\n-92.2\t30.3\n-92.1\t30.6\n-92\t30.9\n-91.9\t31.2\n-91.8\t31.5\n-91.7\t31.8\n-91.6\t32.1\n-91.5\t32.4\n-91.4\t32.7\n-91.3\t33\n-91.2\t33.3\n-91.1\t33.6\n-91\t33.9\n-90.9\t34.2\n-90.8\t34.5\n-90.7\t34.8\n-90.6\t35.1\n-90.5\t35.4\n-90.4\t35.7\n-90.3\t36\n-90.2\t36.3\n-90.1\t36.6\n-90\t36.9\n-89.9\t37.2\n-89.8\t37.5\n-89.7\t37.8\n-89.6\t38.1\n-89.5\t38.4\n-89.4\t38.7\n-89.3\t39\n-89.2\t39.3\n-89.1\t39.6\n-89\t39.9\n-88.9\t40.2\n-88.8\t40.5\n-88.7\t40.8\n-88.6\t41.1\n-88.5\t41.4\n-88.4\t41.7\n-88.3\t42\n-88.2\t42.3\n-88.1\t42.6\n-88\t42.9\n-87.9\t43.2\n-87.8\t43.5\n-87.7\t43.8\n-87.6\t44.1\n-87.5\t44.4\n-87.4\t44.7\n-87.3\t45\n-87.2\t45.3\n-87.1\t45.6\n-87\t45.9\n-86.9\t46.2\n-86.8\t46.5\n-86.7\t46.8\n-86.6\t47.1\n-86.5\t47.4\n-86.4\t47.7\n-86.3\t48\n-86.2\t48.3\n-86.1\t48.6\n-86\t48.9\n-85.9\t49.2\n-85.8\t49.5\n-85.7\t49.8\n-85.6\t50.1\n-85.5\t50.4\n-85.4\t50.7\n-85.3\t51\n-85.2\t51.3\n-85.1\t51.6\n-85\t51.9\n-84.9\t52.2\n-84.8\t52.5\n-84.7\t52.8\n-84.6\t53.1\n-84.5\t53.4\n-84.4\t53.7\n-84.3\t54\n-84.2\t54.3\n-84.1\t54.6\n-84\t54.9\n-83.9\t55.2\n-83.8\t55.5\n-83.7\t55.8\n-83.6\t56.1\n-83.5\t56.4\n-83.4\t56.7\n-83.3\t57\n-83.2\t57.3\n-83.1\t57.6\n-83\t57.9\n-82.9\t58.2\n-82.8\t58.5\n-82.7\t58.8\n-82.6\t59.1\n-82.5\t59.4\n-82.4\t59.7\n-82.3\t60\n-82.2\t60.3\n-82.1\t60.6\n-82\t60.9\n-81.9\t61.2\n-81.8\t61.5\n-81.7\t61.8\n-81.6\t62.1\n-81.5\t62.4\n-81.4\t62.7\n-81.3\t63\n-81.2\t63.3\n-81.1\t63.6\n-81\t63.9\n-80.9\t64.2\n-80.8\t64.5\n-80.7\t64.8\n-80.6\t65.1\n-80.5\t65.4\n-80.4\t65.7\n-80.3\t66\n-80.2\t66.3\n-80.1\t66.6\n-80\t66.9\n-79.9\t67.2\n-79.8\t67.5\n-79.7\t67.8\n-79.6\t68.1\n-79.5\t68.4\n-79.4\t68.7\n-79.3\t69\n-79.2\t69.3\n-79.1\t69.6\n-79\t69.9\n-78.9\t70.2\n-78.8\t70.5\n-78.7\t70.8\n-78.6\t71.1\n-78.5\t71.4\n-78.4\t71.7\n-78.3\t72\n-78.2\t72.3\n-78.1\t72.6\n-78\t72.9\n-77.9\t73.2\n-77.8\t73.5\n-77.7\t73.8\n-77.6\t74.1\n-77.5\t74.4\n-77.4\t74.7\n-77.3\t75\n-77.2\t75.3\n-77.1\t75.6\n-77\t75.9\n-76.9\t76.2\n-76.8\t76.5\n-76.7\t76.8\n-76.6\t77.1\n-76.5\t77.4\n-76.4\t77.7\n-76.3\t78\n-76.2\t78.3\n-76.1\t78.6\n-76\t78.9\n-75.9\t79.2\n-75.8\t79.5\n-75.7\t79.8\n-75.6\t80.1\n-75.5\t80.4\n-75.4\t80.7\n-75.3\t81\n-75.2\t81.3\n-75.1\t81.6\n-75\t81.9\n-74.9\t82.2\n-74.8\t82.5\n-74.7\t82.8\n-74.6\t83.1\n-74.5\t83.4\n-74.4\t83.7\n-74.3\t84\n-74.2\t84.3\n-74.1\t84.6\n-74\t84.9\n-73.9\t85.2\n-73.8\t85.5\n-73.7\t85.8\n-73.6\t86.1\n-73.5\t86.4\n-73.4\t86.7\n-73.3\t87\n-73.2\t87.3\n-73.1\t87.6\n-73\t87.9\n-72.9\t88.2\n-72.8\t88.5\n-72.7\t88.8\n-72.6\t89.1\n-72.5\t89.4\n-72.4\t89.7\n-72.3\t90\n-72.2\t90.3\n-72.1\t90.6\n-72\t90.9\n-71.9\t91.2\n-71.8\t91.5\n-71.7\t91.8\n-71.6\t92.1\n-71.5\t92.4\n-71.4\t92.7\n-71.3\t93\n-71.2\t93.3\n-71.1\t93.6\n-71\t93.9\n-70.9\t93.2\n-70.8\t92.5\n-70.7\t91.8\n-70.6\t91.1\n-70.5\t90.4\n-70.4\t89.7\n-70.3\t89\n-70.2\t88.3\n-70.1\t87.6\n-70\t86.9\n-69.9\t86.2\n-69.8\t85.5\n-69.7\t84.8\n-69.6\t84.1\n-69.5\t83.4\n-69.4\t82.7\n-69.3\t82\n-69.2\t81.3\n-69.1\t80.6\n-69\t79.9\n-68.9\t79.2\n-68.8\t78.5\n-68.7\t77.8\n-68.6\t77.1\n-68.5\t76.4\n-68.4\t75.7\n-68.3\t75\n-68.2\t74.3\n-68.1\t73.6\n-68\t72.9\n-67.9\t72.2\n-67.8\t71.5\n-67.7\t70.8\n-67.6\t70.1\n-67.5\t69.4\n-67.4\t68.7\n-67.3\t68\n-67.2\t67.3\n-67.1\t66.6\n-67\t65.9\n-66.9\t65.2\n-66.8\t64.5\n-66.7\t63.8\n-66.6\t63.1\n-66.5\t62.4\n-66.4\t61.7\n-66.3\t61\n-66.2\t60.3\n-66.1\t59.6\n-66\t58.9\n-65.9\t58.2\n-65.8\t57.5\n-65.7\t56.8\n-65.6\t56.1\n-65.5\t55.4\n-65.4\t54.7\n-65.3\t54\n-65.2\t53.3\n-65.1\t52.6\n-65\t51.9\n-64.9\t51.2\n-64.8\t50.5\n-64.7\t49.8\n-64.6\t49.1\n-64.5\t48.4\n-64.4\t47.7\n-64.3\t47\n-64.2\t46.3\n-64.1\t45.6\n-64\t44.9\n-63.9\t44.2\n-63.8\t43.5\n-63.7\t42.8\n-63.6\t42.1\n-63.5\t41.4\n-63.4\t40.7\n-63.3\t40\n-63.2\t39.3\n-63.1\t38.6\n-63\t37.9\n-62.9\t37.2\n-62.8\t36.5\n-62.7\t35.8\n-62.6\t35.1\n-62.5\t34.4\n-62.4\t33.7\n-62.3\t33\n-62.2\t32.3\n-62.1\t31.6\n-62\t30.9\n-61.9\t30.2\n-61.8\t29.5\n-61.7\t28.8\n-61\t28.1\n-60.3\t27.4\n-59.6\t26.7\n-58.9\t26\n-58.2\t25.3\n-57.5\t24.6\n-56.8\t23.9\n-56.1\t23.2\n-55.4\t22.5\n-54.7\t21.8\n-54\t21.1\n-53.3\t20.4\n-52.6\t19.7\n-51.9\t19\n-51.2\t18.3\n-50.5\t17.6\n-49.8\t16.9\n-49.1\t16.2\n-48.4\t15.5\n-47.7\t14.8\n-47\t14.1\n-46.3\t13.4\n-45.6\t12.7\n-44.9\t12\n-44.2\t11.3\n-43.5\t10.6\n-42.8\t9.9\n-42.1\t9.2\n-41.4\t8.5\n-40.7\t7.8\n-40\t7.1\n-39.3\t6.4\n-38.6\t5.7\n-37.9\t5\n-37.2\t4.3\n-36.5\t3.6\n-35.8\t2.9\n-35.1\t2.2\n-34.4\t1.5\n-33.7\t0.8\n-33\t0.1\n-32.3\t-0.6\n-31.6\t-1.3\n-30.9\t-2\n-30.2\t-2.7\n-29.5\t-3.4\n-28.8\t-4.1\n-28.1\t-4.8\n-27.4\t-5.5\n-26.7\t-6.2\n-26\t-6.9\n-25.3\t-7.6\n-24.6\t-8.3\n-23.9\t-9\n-23.2\t-9.7\n-22.5\t-10.4\n-21.8\t-11.1\n-21.1\t-11.8\n-20.4\t-12.5\n-19.7\t-13.2\n-19\t-13.9\n-18.3\t-14.6\n-17.6\t-15.3\n-16.9\t-16\n-16.2\t-16.7\n-15.5\t-17.4\n-14.8\t-18.1\n-14.1\t-18.8\n-13.4\t-19.5\n-12.7\t-20.2\n-12\t-20.9\n-11.3\t-21.6\n-10.6\t-22.3\n-9.9\t-23\n-9.2\t-23.7\n-8.5\t-24.4\n-7.8\t-25.1\n-7.1\t-25.8\n-6.4\t-26.5\n-5.7\t-27.2\n-5\t-27.9\n-4.3\t-28.6\n-3.6\t-29.3\n-2.9\t-30\n-2.2\t-30.7\n-1.5\t-31.4\n-0.8\t-32.1\n-0.1\t-32.8\n0.6\t-33.5\n1.3\t-34.2\n2\t-34.9\n2.7\t-35.6\n3.4\t-36.3\n4.1\t-37\n4.8\t-37.7\n5.5\t-38.4\n6.2\t-39.1\n6.9\t-39.8\n7.6\t-40.5\n8.3\t-41.2\n9\t-41.9\n9.7\t-42.6\n10.4\t-43.3\n11.1\t-44\n11.8\t-44.7\n12.5\t-45.4\n13.2\t-46.1\n13.9\t-46.8\n14.6\t-47.5\n15.3\t-48.2\n16\t-48.9\n16.7\t-49.6\n17.4\t-50.3\n18.1\t-51\n18.8\t-51.7\n19.5\t-52.4\n20.2\t-53.1\n20.9\t-53.8\n21.6\t-54.5\n22.3\t-55.2\n23\t-55.9\n23.7\t-56.6\n24.4\t-57.3\n25.1\t-58\n25.8\t-58.7\n26.5\t-59.4\n27.2\t-60.1\n27.9\t-60.8\n28.6\t-61.5\n29.3\t-62.2\n30\t-62.9\n30.7\t-63.6\n31.4\t-64.3\n32.1\t-65\n32.8\t-65.7\n33.5\t-66.4\n34.2\t-67.1\n34.9\t-67.8\n35.6\t-68.5\n36.3\t-69.2\n37\t-69.9\n37.7\t-70.6\n38.4\t-71.3\n39.1\t-72\n39.8\t-72.7\n40.5\t-73.4\n41.2\t-74.1\n41.9\t-74.8\n42.6\t-75.5\n43.3\t-75\n44\t-74.5\n44.7\t-74\n45.4\t-73.5\n46.1\t-73\n46.8\t-72.5\n47.5\t-72\n48.2\t-71.5\n48.9\t-71\n49.6\t-70.5\n50.3\t-70\n51\t-69.5\n51.7\t-69\n52.4\t-68.5\n53.1\t-68\n53.8\t-67.5\n54.5\t-67\n55.2\t-66.5\n55.9\t-66\n56.6\t-65.5\n57.3\t-65\n58\t-64.5\n58.7\t-64\n59.4\t-63.5\n60.1\t-63\n60.8\t-62.5\n61.5\t-62\n62.2\t-61.5\n62.9\t-61\n63.6\t-60.5\n64.3\t-60\n65\t-59.5\n65.7\t-59\n66.4\t-58.5\n67.1\t-58\n67.8\t-57.5\n68.5\t-57\n69.2\t-56.5\n69.9\t-56\n70.6\t-55.5\n71.3\t-55\n71.1\t-54.5\n70.9\t-54\n70.7\t-53.5\n70.5\t-53\n70.3\t-52.5\n70.1\t-52\n69.9\t-51.5\n69.7\t-51\n69.5\t-50.5\n69.3\t-50\n69.1\t-49.5\n68.9\t-49\n68.7\t-48.5\n68.5\t-48\n68.3\t-47.5\n68.1\t-47\n67.9\t-46.5\n67.7\t-46\n67.5\t-45.5\n67.3\t-45\n67.1\t-44.5\n66.9\t-44\n66.7\t-43.5\n66.5\t-43\n66.3\t-42.5\n66.1\t-42\n65.9\t-41.5\n65.7\t-41\n65.5\t-40.5\n65.3\t-40\n65.1\t-39.5\n64.9\t-39\n64.7\t-38.5\n64.5\t-38\n64.3\t-37.5\n64.1\t-37\n63.9\t-36.5\n63.7\t-36\n63.5\t-35.5\n63.3\t-35\n63.1\t-34.5\n62.9\t-34\n62.7\t-33.5\n62.5\t-33\n62.3\t-32.5\n62.1\t-32\n61.9\t-31.5\n61.7\t-31\n61.5\t-30.5\n61.3\t-30\n61.1\t-29.5\n60.9\t-29\n60.7\t-28.5\n60.5\t-28\n60.3\t-27.5\n60.1\t-27\n59.9\t-26.5\n59.7\t-26\n59.5\t-25.5\n59.3\t-25\n59.1\t-24.5\n58.9\t-24\n58.7\t-23.5\n58.5\t-23\n58.3\t-22.5\n58.1\t-22\n57.9\t-21.5\n57.7\t-21\n57.5\t-20.5\n57.3\t-20\n57.1\t-19.5\n56.9\t-19\n56.7\t-18.5\n56.5\t-18\n56.3\t-17.5\n56.1\t-17\n55.9\t-16.5\n55.7\t-16\n55.5\t-15.5\n55.3\t-15\n55.1\t-14.5\n54.9\t-14\n54.7\t-13.5\n54.5\t-13\n54.3\t-12.5\n54.1\t-12\n53.9\t-11.5\n53.7\t-11\n53.5\t-10.5\n53.3\t-10\n53.1\t-9.5\n52.9\t-9\n52.7\t-8.5\n52.5\t-8\n52.3\t-7.5\n52.1\t-7\n51.9\t-6.5\n51.7\t-6\n51.5\t-5.5\n51.3\t-5\n51.1\t-4.5\n50.9\t-4\n50.7\t-3.5\n50.5\t-3\n50.3\t-2.5\n50.1\t-2\n49.9\t-1.5\n49.7\t-1\n49.5\t-0.5\n49.3\t-2.74269E-12\n49.1\t0.5\n48.9\t1\n48.7\t1.5\n48.5\t2\n48.3\t2.5\n48.1\t3\n47.9\t3.5\n47.7\t4\n47.5\t4.5\n47.3\t5\n47.1\t5.5\n46.9\t6\n46.7\t6.5\n46.5\t7\n46.3\t7.5\n46.1\t8\n45.9\t8.5\n45.7\t9\n45.5\t9.5\n45.3\t10\n45.1\t10.5\n44.9\t11\n44.7\t11.5\n44.5\t12\n44.3\t12.5\n44.1\t13\n43.9\t13.5\n43.7\t14\n43.5\t14.5\n43.3\t15\n43.1\t15.5\n42.9\t16\n42.7\t16.5\n42.5\t17\n42.3\t17.5\n42.1\t18\n41.9\t18.5\n41.7\t19\n41.5\t19.5\n41.3\t20\n41.1\t20.5\n40.9\t21\n40.7\t21.5\n40.5\t22\n40.3\t22.5\n40.1\t23\n39.9\t23.5\n39.7\t24\n39.5\t24.5\n39.3\t25\n39.1\t25.5\n38.9\t26\n38.7\t26.5\n38.5\t27\n38.3\t27.5\n38.1\t28\n37.9\t28.5\n37.7\t29\n37.5\t29.5\n37.3\t30\n37.1\t30.5\n36.9\t31\n36.7\t31.5\n36.5\t32\n36.3\t32.5\n36.1\t33\n35.9\t33.5\n35.7\t34\n35.5\t34.5\n35.3\t35\n35.1\t35.5\n34.9\t36\n34.7\t35.8\n34.5\t35.6\n34.3\t35.4\n34.1\t35.2\n33.9\t35\n33.7\t34.8\n33.5\t34.6\n33.3\t34.4\n33.1\t34.2\n32.9\t34\n32.7\t33.8\n32.5\t33.6\n32.3\t33.4\n32.1\t33.2\n31.9\t33\n31.7\t32.8\n31.5\t32.6\n31.3\t32.4\n31.1\t32.2\n30.9\t32\n30.7\t31.8\n30.5\t31.6\n30.3\t31.4\n30.1\t31.2\n29.9\t31\n29.7\t30.8\n29.5\t30.6\n29.3\t30.4\n29.1\t30.2\n28.9\t30\n28.7\t29.8\n28.5\t29.6\n28.3\t29.4\n28.1\t29.2\n27.9\t29\n27.7\t28.8\n27.5\t28.6\n27.3\t28.4\n27.1\t28.2\n26.9\t28\n26.7\t27.8\n26.5\t27.6\n26.3\t27.4\n26.1\t27.2\n25.9\t27\n25.7\t26.8\n25.5\t26.6\n25.3\t26.4\n25.1\t26.2\n24.9\t26\n24.7\t25.8\n24.5\t25.6\n24.3\t25.4\n24.1\t25.2\n23.9\t25\n23.7\t24.8\n23.5\t24.6\n23.3\t24.4\n23.1\t24.2\n22.9\t24\n22.7\t23.8\n22.5\t23.6\n22.3\t23.4\n22.1\t23.2\n21.9\t23\n21.7\t22.8\n21.5\t22.6\n21.3\t22.4\n21.1\t22.2\n20.9\t22\n20.7\t21.8\n20.5\t21.6\n20.3\t21.4\n20.1\t21.2\n19.9\t21\n19.7\t20.8\n19.5\t20.6\n19.3\t20.4\n19.1\t20.2\n18.9\t20\n18.7\t19.8\n18.5\t19.6\n18.3\t19.4\n18.1\t19.2\n17.9\t19\n17.7\t18.8\n17.5\t18.6\n17.3\t18.4\n17.1\t18.2\n16.9\t18\n16.7\t17.8\n16.5\t17.6\n16.3\t17.4\n16.1\t17.2\n15.9\t17\n15.7\t16.8\n15.5\t16.6\n15.3\t16.4\n15.1\t16.2\n14.9\t16\n14.7\t15.8\n14.5\t15.6\n14.3\t15.4\n14.1\t15.2\n13.9\t15\n13.7\t14.8\n13.5\t14.6\n13.3\t14.4\n13.1\t14.2\n12.9\t14\n12.7\t13.8\n12.5\t13.6\n12.3\t13.4\n12.1\t13.2\n11.9\t13\n11.7\t12.8\n11.5\t12.6\n11.3\t12.4\n11.1\t12.2\n10.9\t12\n10.7\t11.8\n10.5\t11.6\n10.3\t11.4\n10.1\t11.2\n9.9\t11\n9.7\t10.8\n9.5\t10.6\n9.3\t10.4\n9.1\t10.2\n8.9\t10\n8.7\t9.8\n8.5\t9.6\n8.3\t9.4\n8.1\t9.2\n7.9\t9\n7.7\t8.8\n7.5\t8.6\n7.3\t8.4\n7.1\t8.2\n6.9\t8\n6.7\t7.8\n6.5\t7.6\n6.3\t7.4\n6.1\t7.2\n5.9\t7\n5.7\t6.8\n5.5\t6.6\n5.3\t6.4\n5.1\t6.2\n4.9\t6\n4.3\t5.8\n3.7\t5.6\n3.1\t5.4\n2.5\t5.2\n1.9\t5\n1.3\t4.8\n0.7\t4.6\n0.1\t4.4\n-0.5\t4.2\n-1.1\t4\n-1.7\t3.8\n-2.3\t3.6\n-2.9\t3.4\n-3.5\t3.2\n-4.1\t3\n-4.7\t2.8\n-5.3\t2.6\n-5.9\t2.4\n-6.5\t2.2\n-7.1\t2\n-7.7\t1.8\n-8.3\t1.6\n-8.9\t1.4\n-9.5\t1.2\n-10.1\t1\n-10.7\t0.8\n-11.3\t0.6\n-11.9\t0.4\n-12.5\t0.2\n-13.1\t-2.71644E-12\n-13.7\t-0.2\n-14.3\t-0.4\n-14.9\t-0.6\n-15.5\t-0.8\n-16.1\t-1\n-16.7\t-1.2\n-17.3\t-1.4\n-17.9\t-1.6\n-18.5\t-1.8\n-19.1\t-2\n-19.7\t-2.2\n-20.3\t-2.4\n-20.9\t-2.6\n-21.5\t-2.8\n-22.1\t-3\n-22.7\t-3.2\n-23.3\t-3.4\n-23.9\t-3.6\n-24.5\t-3.8\n-25.1\t-4\n-25.7\t-4.2\n-26.3\t-4.4\n-26.9\t-4.6\n-27.5\t-4.8\n-28.1\t-5\n-28.7\t-5.2\n-29.3\t-5.4\n-29.9\t-5.6\n-30.5\t-5.8\n-31.1\t-6\n-31.7\t-6.2\n-32.3\t-6.4\n-32.9\t-6.6\n-33.5\t-6.8\n-34.1\t-7\n-34.7\t-7.2\n-35.3\t-7.4\n-35.9\t-7.6\n-36.5\t-7.8\n-37.1\t-8\n-37.7\t-8.2\n-38.3\t-8.4\n-38.9\t-8.6\n-39.5\t-8.8\n-40.1\t-9\n-40.7\t-9.2\n-41.3\t-9.4\n-41.9\t-9.6\n-42.5\t-9.8\n-43.1\t-10\n-43.7\t-10.2\n-44.3\t-10.4\n-44.9\t-10.6\n-45.5\t-10.8\n-46.1\t-11\n-46.7\t-11.2\n-47.3\t-11.4\n-47.9\t-11.6\n-48.5\t-11.8\n-49.1\t-12\n-49.7\t-12.2\n-50.3\t-12.4\n-50.9\t-12.6\n-51.5\t-12.8\n-52.1\t-13\n-52.7\t-13.2\n-53.3\t-13.4\n-53.9\t-13.6\n-54.5\t-13.8\n-55.1\t-14\n-55.7\t-14.2\n-55.4\t-14.4\n-55.1\t-14.6\n-54.8\t-14.8\n-54.5\t-15\n-54.2\t-15.2\n-53.9\t-15.4\n-53.6\t-15.6\n-53.3\t-15.8\n-53\t-16\n-52.7\t-16.2\n-52.4\t-16.4\n-52.1\t-16.6\n-51.8\t-16.8\n-51.5\t-17\n-51.2\t-17.2\n-50.9\t-17.4\n-50.6\t-17.6\n-50.3\t-17.8\n-50\t-18\n-49.7\t-18.2\n-49.4\t-18.4\n-49.1\t-18.6\n-48.8\t-18.8\n-48.5\t-19\n-48.2\t-19.2\n-47.9\t-19.4\n-47.6\t-19.6\n-47.3\t-19.8\n-47\t-20\n-46.7\t-20.2\n-46.4\t-20.4\n-46.1\t-20.6\n-45.8\t-20.8\n-45.5\t-21\n-45.2\t-21.2\n-44.9\t-21.4\n-44.6\t-21.6\n-44.3\t-21.8\n-44\t-22\n-43.7\t-22.2\n-43.4\t-22.4\n-43.1\t-22.6\n-42.8\t-22.8\n-42.5\t-23\n-42.2\t-23.2\n-41.9\t-23.4\n-41.6\t-23.6\n-41.3\t-23.8\n-41\t-24\n-40.7\t-24.2\n-40.4\t-24.4\n-40.1\t-24.6\n-39.8\t-24.8\n-39.5\t-25\n-39.2\t-25.2\n-38.9\t-25.4\n-38.6\t-25.6\n-38.3\t-25.8\n-38\t-26\n-37.7\t-26.2\n-37.4\t-26.4\n-37.1\t-26.6\n-36.8\t-26.8\n-36.5\t-27\n-36.2\t-27.2\n-35.9\t-27.4\n-35.6\t-27.6\n-35.3\t-27.8\n-35\t-28\n-34.7\t-28.2\n-34.4\t-28.4\n-34.1\t-28.6\n-33.8\t-28.8\n-33.5\t-29\n-33.2\t-29.2\n-32.9\t-29.4\n-32.6\t-29.6\n-32.3\t-29.8\n-32\t-30\n-31.7\t-30.2\n-31.4\t-30.4\n-31.1\t-30.6\n-30.8\t-30.8\n-30.5\t-31\n-30.2\t-31.2\n-29.9\t-31.4\n-29.6\t-31.6\n-29.3\t-31.8\n-29\t-32\n-28.7\t-32.2\n-28.4\t-32.4\n-28.1\t-32.6\n-27.8\t-32.8\n-27.5\t-33\n-27.2\t-33.2\n-26.9\t-33.4\n-26.6\t-33.6\n-26.3\t-33.8\n-26\t-34\n-25.7\t-34.2\n-25.4\t-34.4\n-25.1\t-34.6\n-24.8\t-34.8\n-24.5\t-35\n-24.2\t-35.2\n-23.9\t-35.4\n-23.6\t-35.6\n-23.3\t-35.8\n-23\t-36\n-22.7\t-36.2\n-22.4\t-36.4\n-22.1\t-36.6\n-21.8\t-36.8\n-21.5\t-37\n-21.2\t-37.2\n-20.9\t-37.4\n-20.6\t-37.6\n-20.3\t-37.8\n-20\t-38\n-19.7\t-38.2\n-19.4\t-38.4\n-19.1\t-38.6\n-18.8\t-38.8\n-18.5\t-39\n-18.2\t-39.2\n-17.9\t-39.4\n-17.6\t-39.6\n-17.3\t-39.8\n-17\t-40\n-16.7\t-40.2\n-16.4\t-40.4\n-16.1\t-40.6\n-15.8\t-40.8\n-15.5\t-41\n-15.2\t-41.2\n-14.9\t-41.4\n-14.6\t-41.6\n-14.3\t-41.8\n-14\t-42\n-13.7\t-42.2\n-13.4\t-42.4\n-13.1\t-42.6\n-12.8\t-42.8\n-12.5\t-43\n-12.2\t-43.2\n-11.9\t-43.4\n-11.6\t-43.6\n-11.3\t-43.8\n-11\t-44\n-10.7\t-44.2\n-10.4\t-44.4\n-10.1\t-44.6\n-9.8\t-44.8\n-9.5\t-45\n-9.2\t-45.2\n-8.9\t-45.4\n-8.6\t-45.6\n-8.3\t-45.8\n-8\t-46\n-7.7\t-46.2\n-7.4\t-46.4\n-7.1\t-46.6\n-6.8\t-46.8\n-6.5\t-47\n-6.2\t-47.2\n-5.9\t-47.4\n-5.6\t-47.6\n-5.3\t-47.8\n-5\t-48\n-4.7\t-48.2\n-4.4\t-48.4\n-4.1\t-48.6\n-3.8\t-48.8\n-3.5\t-49\n-3.2\t-49.2\n-2.9\t-49.4\n-2.6\t-49.6\n-2.3\t-49.8\n-2\t-50\n-1.7\t-50.2\n-1.4\t-50.4\n-1.1\t-50.6\n-0.8\t-50.8\n-0.5\t-51\n-0.2\t-51.2\n0.1\t-51.4\n0.4\t-51.6\n0.7\t-51.8\n1\t-52\n1.3\t-52.2\n1.6\t-52.4\n1.9\t-52.6\n2.2\t-52.8\n2.5\t-53\n2.8\t-53.2\n3.1\t-53.4\n3.4\t-53.6\n3.7\t-53.8\n4\t-54\n4.3\t-54.2\n4.6\t-54.4\n4.9\t-54.6\n5.2\t-54.8\n5.5\t-55\n5.8\t-55.2\n6.1\t-55.4\n6.4\t-55.6\n6.7\t-55.8\n7\t-56\n7.3\t-56.2\n7.6\t-56.4\n7.9\t-56.6\n8.2\t-56.8\n8.5\t-57\n8.8\t-57.2\n9.1\t-57.4\n9.4\t-57.6\n9.7\t-57.8\n10\t-58\n10.3\t-58.2\n10.6\t-58.4\n10.9\t-58.6\n11.2\t-58.8\n11.5\t-59\n11.8\t-59.2\n12.1\t-59.4\n12.4\t-59.6\n12.7\t-59.8\n13\t-60\n13.3\t-60.2\n13.6\t-60.4\n13.9\t-60.6\n14.2\t-60.8\n14.5\t-61\n14.8\t-61.2\n15.1\t-61.4\n15.4\t-61.6\n15.7\t-61.8\n16\t-62\n16.3\t-62.2\n16.6\t-62.4\n16.9\t-62.6\n17.2\t-62.8\n17.5\t-63\n17.8\t-63.2\n18.1\t-63.4\n18.4\t-63.6\n18.7\t-63.8\n19\t-64\n19.3\t-64.2\n19.6\t-64.4\n19.9\t-64.6\n20.2\t-64.8\n20.5\t-65\n20.8\t-65.2\n21.1\t-65.4\n21.4\t-65.6\n21.7\t-65.8\n22\t-66\n22.3\t-66.2\n22.6\t-66.4\n22.9\t-66.6\n23.2\t-66.8\n23.5\t-67\n23.8\t-67.2\n24.1\t-67.4\n24.4\t-67.6\n24.7\t-67.8\n25\t-68\n25.3\t-68.2\n25.6\t-68.4\n25.9\t-68.6\n26.2\t-68.8\n26.5\t-69\n26.8\t-69.2\n27.1\t-69.4\n27.4\t-69.6\n27.7\t-69.8\n28\t-70\n28.3\t-70.2\n28.6\t-70.4\n28.9\t-70.6\n29.2\t-70.8\n29.5\t-71\n29.8\t-71.2\n30.1\t-71.4\n30.4\t-71.6\n30.7\t-71.8\n31\t-72\n31.3\t-72.2\n31.6\t-72.4\n31.9\t-72.6\n32.2\t-72.8\n32.5\t-73\n32.8\t-73.2\n33.1\t-73.4\n33.4\t-73.6\n33.7\t-73.8\n34\t-74\n34.3\t-74.2\n34.6\t-74.4\n34.9\t-74.6\n35.2\t-74.8\n35.5\t-75\n35.8\t-75.2\n36.1\t-75.4\n36.4\t-75.6\n36.7\t-75.8\n37\t-76\n37.3\t-76.2\n37.6\t-76.4\n37.9\t-76.6\n38.2\t-76.8\n38.5\t-77\n38.8\t-77.2\n39.1\t-77.4\n39.4\t-77.6\n39.7\t-77.8\n40\t-78\n40.3\t-78.2\n40.6\t-78.4\n40.9\t-78.6\n41.2\t-78.8\n41.5\t-79\n41.8\t-79.2\n42.1\t-79.4\n42.4\t-79.6\n42.7\t-79.8\n43\t-80\n43.3\t-80.2\n43.6\t-80.4\n43.9\t-80.6\n44.2\t-80.8\n44.5\t-81\n44.8\t-81.2\n45.1\t-81.4\n45.4\t-81.6\n45.7\t-81.8\n46\t-82\n46.3\t-82.2\n46.6\t-82.4\n46.9\t-82.6\n47.2\t-82.8\n47.5\t-83\n47.8\t-83.2\n48.1\t-83.4\n48.4\t-83.6\n48.7\t-83.8\n49\t-84\n49.3\t-84.2\n49.6\t-84.4\n49.9\t-84.6\n50.2\t-84.8\n50.5\t-85\n50.8\t-85.2\n51.1\t-85.4\n51.4\t-85.6\n51.7\t-85.8\n52\t-86\n52.3\t-86.2\n52.6\t-86.4\n52.9\t-86.6\n53.2\t-86.8\n53.5\t-87\n53.8\t-87.2\n54.1\t-87.4\n54.4\t-87.6\n54.7\t-87.8\n55\t-88\n55.3\t-88.2\n55.6\t-88.4\n55.9\t-88.6\n56.2\t-88.8\n56.5\t-89\n56.8\t-89.2\n57.1\t-89.4\n57.4\t-89.6\n57.7\t-89.8\n58\t-90\n58.3\t-90.2\n58.6\t-90.4\n58.9\t-90.6\n59.2\t-90.8\n59.5\t-91\n59.8\t-91.2\n60.1\t-91.4\n60.4\t-91.6\n60.7\t-91.8\n61\t-92\n61.3\t-92.2\n61.6\t-92.4\n61.9\t-92.6\n62.2\t-92.8\n62.5\t-93\n62.8\t-93.2\n63.1\t-93.4\n63.4\t-93.6\n63.7\t-93.8\n64\t-94\n64.3\t-93.6\n64.6\t-93.2\n64.9\t-92.8\n65.2\t-92.4\n65.5\t-92\n65.8\t-91.6\n66.1\t-91.2\n66.4\t-90.8\n66.7\t-90.4\n67\t-90\n67.3\t-89.6\n67.6\t-89.2\n67.9\t-88.8\n68.2\t-88.4\n68.5\t-88\n68.8\t-87.6\n69.1\t-87.2\n69.4\t-86.8\n69.7\t-86.4\n70\t-86\n70.3\t-85.6\n70.6\t-85.2\n70.9\t-84.8\n71.2\t-84.4\n71.5\t-84\n71.8\t-83.6\n72.1\t-83.2\n72.4\t-82.8\n72.7\t-82.4\n73\t-82\n73.3\t-81.6\n73.6\t-81.2\n73.9\t-80.8\n74.2\t-80.4\n74.5\t-80\n74.8\t-79.6\n75.1\t-79.2\n75.4\t-78.8\n75.7\t-78.4\n76\t-78\n76.3\t-77.6\n76.6\t-77.2\n76.9\t-76.8\n77.2\t-76.4\n77.5\t-76\n77.8\t-75.6\n78.1\t-75.2\n78.4\t-74.8\n78.7\t-74.4\n79\t-74\n79.3\t-73.6\n79.6\t-73.2\n79.9\t-72.8\n80.2\t-72.4\n80.5\t-72\n80.8\t-71.6\n81.1\t-71.2\n81.4\t-70.8\n81.7\t-70.4\n82\t-70\n82.3\t-69.6\n82.6\t-69.2\n82.9\t-68.8\n83.2\t-68.4\n83.5\t-68\n83.8\t-67.6\n84.1\t-67.2\n84.4\t-66.8\n84.7\t-66.4\n83.8\t-66\n82.9\t-65.6\n82\t-65.2\n81.1\t-64.8\n80.2\t-64.4\n79.3\t-64\n78.4\t-63.6\n77.5\t-63.2\n76.6\t-62.8\n75.7\t-62.4\n74.8\t-62\n73.9\t-61.6\n73\t-61.2\n72.1\t-60.8\n71.2\t-60.4\n70.3\t-60\n69.4\t-59.6\n68.5\t-59.2\n67.6\t-58.8\n66.7\t-58.4\n65.8\t-58\n64.9\t-57.6\n64\t-57.2\n63.1\t-56.8\n62.2\t-56.4\n61.3\t-56\n60.4\t-55.6\n59.5\t-55.2\n58.6\t-54.8\n57.7\t-54.4\n56.8\t-54\n55.9\t-53.6\n55\t-53.2\n54.1\t-52.8\n53.2\t-52.4\n52.3\t-52\n51.4\t-51.6\n50.5\t-51.2\n49.6\t-50.8\n48.7\t-50.4\n47.8\t-50\n46.9\t-49.6\n46\t-49.2\n45.1\t-48.8\n44.2\t-48.4\n43.3\t-48\n42.4\t-47.6\n41.5\t-47.2\n40.6\t-46.8\n39.7\t-46.4\n38.8\t-46\n37.9\t-45.6\n37\t-45.2\n36.1\t-44.8\n35.2\t-44.4\n34.3\t-44\n33.4\t-43.6\n32.5\t-43.2\n31.6\t-42.8\n30.7\t-42.4\n29.8\t-42\n28.9\t-41.6\n28\t-41.2\n27.1\t-40.8\n26.2\t-40.4\n25.3\t-40\n24.4\t-39.6\n24.3\t-39.2\n24.2\t-38.8\n24.1\t-38.4\n24\t-38\n23.9\t-37.6\n23.8\t-37.2\n23.7\t-36.8\n23.6\t-36.4\n23.5\t-36\n23.4\t-35.6\n23.3\t-35.2\n23.2\t-34.8\n23.1\t-34.4\n23\t-34\n22.9\t-33.6\n22.8\t-33.2\n22.7\t-32.8\n22.6\t-32.4\n22.5\t-32\n22.4\t-31.6\n22.3\t-31.2\n22.2\t-30.8\n22.1\t-30.4\n22\t-30\n21.9\t-29.6\n21.8\t-29.2\n21.7\t-28.8\n21.6\t-28.4\n21.5\t-28\n21.4\t-27.6\n21.3\t-27.2\n21.2\t-26.8\n21.1\t-26.4\n21\t-26\n20.9\t-25.6\n20.8\t-25.2\n20.7\t-24.8\n20.6\t-24.4\n20.5\t-24\n20.4\t-23.6\n20.3\t-23.2\n20.2\t-22.8\n20.1\t-22.4\n20\t-22\n19.9\t-21.6\n19.8\t-21.2\n19.7\t-20.8\n19.6\t-20.4\n19.5\t-20\n19.4\t-19.6\n19.3\t-19.2\n19.2\t-18.8\n19.1\t-18.4\n19\t-18\n18.9\t-17.6\n18.8\t-17.2\n18.7\t-16.8\n18.6\t-16.4\n18.5\t-16\n18.4\t-15.6\n18.3\t-15.2\n18.2\t-14.8\n18.1\t-14.4\n18\t-14\n17.9\t-13.6\n17.8\t-13.2\n17.7\t-12.8\n17.6\t-12.4\n17.5\t-12\n17.4\t-11.6\n17.3\t-11.2\n17.2\t-10.8\n17.1\t-10.4\n17\t-10\n16.9\t-9.6\n16.8\t-9.2\n16.7\t-8.8\n16.6\t-8.4\n16.5\t-8\n16.4\t-7.6\n16.3\t-7.2\n16.2\t-6.8\n16.1\t-6.4\n16\t-6\n15.9\t-5.6\n15.8\t-5.2\n15.7\t-4.8\n15.6\t-4.4\n15.5\t-4\n15.4\t-3.6\n15.3\t-3.2\n15.2\t-2.8\n15.1\t-2.4\n15\t-2\n14.9\t-1.6\n14.8\t-1.2\n14.7\t-0.8\n14.6\t-0.4\n14.5\t0\n14.4\t0\n14.3\t0.3\n14.2\t0.6\n14.1\t0.9\n14\t1.2\n13.9\t1.5\n13.8\t1.8\n13.7\t2.1\n13.6\t2.4\n13.5\t2.7\n13.4\t3\n13.3\t3.3\n13.2\t3.6\n13.1\t3.9\n13\t4.2\n12.9\t4.5\n12.8\t4.8\n12.7\t5.1\n12.6\t5.4\n12.5\t5.7\n12.4\t6\n12.3\t6.3\n12.2\t6.6\n12.1\t6.9\n12\t7.2\n11.9\t7.5\n11.8\t7.8\n11.7\t8.1\n11.6\t8.4\n11.5\t8.7\n11.4\t9\n11.3\t9.3\n11.2\t9.6\n11.1\t9.9\n11\t10.2\n10.9\t10.5\n10.8\t10.8\n10.7\t11.1\n10.6\t11.4\n10.5\t11.7\n10.4\t12\n10.3\t12.3\n10.2\t12.6\n10.1\t12.9\n10\t13.2\n9.9\t13.5\n9.8\t13.8\n9.7\t14.1\n9.6\t14.4\n9.5\t14.7\n9.4\t15\n9.3\t15.3\n9.2\t15.6\n9.1\t15.9\n9\t16.2\n8.9\t16.5\n8.8\t16.8\n8.7\t17.1\n8.6\t17.4\n8.5\t17.7\n8.4\t18\n8.3\t18.3\n8.2\t18.6\n8.1\t18.9\n8\t19.2\n7.9\t19.5\n7.8\t19.8\n7.7\t20.1\n7.6\t20.4\n7.5\t20.7\n7.4\t21\n7.3\t21.3\n7.2\t21.6\n7.1\t21.9\n7\t22.2\n6.9\t22.5\n6.8\t22.8\n6.7\t23.1\n6.6\t23.4\n6.5\t23.7\n6.4\t24\n6.3\t24.3\n6.2\t24.6\n6.1\t24.9\n6\t25.2\n5.9\t25.5\n5.8\t25.8\n5.7\t26.1\n5.6\t26.4\n5.5\t26.7\n5.4\t27\n5.3\t27.3\n5.2\t27.6\n5.1\t27.9\n5\t28.2\n4.9\t28.5\n4.8\t28.8\n4.7\t29.1\n4.6\t29.4\n4.5\t29.7\n4.4\t30\n4.3\t30.3\n4.2\t30.6\n4.1\t30.9\n4\t31.2\n3.9\t31.5\n3.8\t31.8\n3.7\t32.1\n3.6\t32.4\n3.5\t32.7\n3.4\t33\n3.3\t33.3\n3.2\t33.6\n3.1\t33.9\n3\t34.2\n2.9\t34.5\n2.8\t34.8\n2.7\t35.1\n2.6\t35.4\n2.5\t35.7\n2.4\t36\n2.3\t36.3\n2.2\t36.6\n2.1\t36.9\n2\t37.2\n1.9\t37.5\n1.8\t37.8\n1.7\t38.1\n1.6\t38.4\n1.5\t38.7\n1.4\t39\n1.3\t39.3\n1.2\t39.6\n1.1\t39.9\n1\t40.2\n0.9\t40.5\n0.8\t40.8\n0.7\t41.1\n0.6\t41.4\n0.5\t41.7\n0.4\t42\n0.3\t42.3\n0.2\t42.6\n0.1\t42.9\n-2.72246E-12\t43.2\n-0.1\t43.5\n-0.2\t43.8\n-0.3\t44.1\n-0.4\t44.4\n-0.5\t44.7\n-0.6\t45\n-0.7\t45.3\n-0.8\t45.6\n-0.9\t45.9\n-1\t46.2\n-1.1\t46.5\n-1.2\t46.8\n-1.3\t47.1\n-1.4\t47.4\n-1.5\t47.7\n-1.6\t48\n-1.7\t48.3\n-1.8\t48.6\n-1.9\t48.9\n-2\t49.2\n-2.1\t49.5\n-2.2\t49.8\n-2.3\t50.1\n-2.4\t50.4\n-2.5\t50.7\n-2.6\t51\n-2.7\t51.3\n-2.8\t51.6\n-2.9\t51.9\n-3\t52.2\n-3.1\t52.5\n-3.2\t52.8\n-3.3\t53.1\n-3.4\t53.4\n-3.5\t53.7\n-3.6\t54\n-3.7\t54.3\n-3.8\t54.6\n-3.9\t54.9\n-4\t55.2\n-4.1\t55.5\n-4.2\t55.8\n-4.3\t56.1\n-4.4\t56.4\n-4.5\t56.7\n-4.6\t57\n-4.7\t57.3\n-4.8\t57.6\n-4.9\t57.9\n-5\t58.2\n-5.1\t58.5\n-5.2\t58.8\n-5.3\t59.1\n-5.4\t59.4\n-5.5\t59.7\n-5.6\t60\n-5.7\t60.3\n-5.8\t60.6\n-5.9\t60.9\n-6\t61.2\n-6.1\t61.5\n-6.2\t61.8\n-6.3\t62.1\n-6.4\t62.4\n-6.5\t62.7\n-6.6\t63\n-6.7\t63.3\n-6.8\t63.6\n-6.9\t63.9\n-7\t64.2\n-7.1\t64.5\n-7.2\t64.8\n-7.3\t65.1\n-7.4\t65.4\n-7.5\t65.7\n-7.6\t66\n-7.7\t66.3\n-7.8\t66.6\n-7.9\t66.9\n-8\t67.2\n-8.1\t67.5\n-8.2\t67.8\n-8.3\t68.1\n-8.4\t68.4\n-8.5\t68.7\n-8.6\t69\n-8.7\t69.3\n-8.8\t69.6\n-8.9\t69.9\n-9\t70.2\n-9.1\t70.5\n-9.2\t70.8\n-9.3\t71.1\n-9.4\t71.4\n-9.5\t71.7\n-9.6\t72\n-9.7\t72.3\n-9.8\t72.6\n-9.9\t72.9\n-10\t73.2\n-10.1\t73.5\n-10.2\t73.8\n-10.3\t74.1\n-10.4\t74.4\n-10.5\t74.7\n-10.6\t75\n-10.7\t75.3\n-10.8\t75.6\n-10.9\t75.9\n-11\t76.2\n-11.1\t76.5\n-11.2\t76.8\n-11.3\t77.1\n-11.4\t77.4\n-11.5\t77.7\n-11.6\t78\n-11.7\t78.3\n-11.8\t78.6\n-11.9\t78.9\n-12\t79.2\n-12.1\t79.5\n-12.2\t79.8\n-12.3\t80.1\n-12.4\t80.4\n-12.5\t80.7\n-12.6\t81\n-12.7\t81.3\n-12.8\t81.6\n-12.9\t81.9\n-13\t82.2\n-13.1\t82.5\n-13.2\t82.8\n-13.3\t83.1\n-13.4\t83.4\n-13.5\t83.7\n-13.6\t84\n-13.7\t84.3\n-13.8\t84.6\n-13.9\t84.9\n-14\t85.2\n-14.1\t85.5\n-14.2\t85.8\n-14.3\t86.1\n-14.4\t86.4\n-14.5\t86.7\n-14.6\t87\n-14.7\t87.3\n-14.8\t87.6\n-14.9\t87.9\n-15\t88.2\n-15.1\t88.5\n-15.2\t88.8\n-15.3\t89.1\n-15.4\t89.4\n-15.5\t89.7\n-15.6\t90\n-15.7\t90.3\n-15.8\t90.6\n-15.9\t90.9\n-16\t91.2\n-16.1\t91.5\n-16.2\t91.8\n-16.3\t92.1\n-16.4\t92.4\n-16.5\t92.7\n-16.6\t93\n-16.7\t93.3\n-16.8\t93.6\n-16.9\t93.9\n-17\t94.2\n-17.1\t94.5\n-17.2\t94.8\n-17.3\t95.1\n-17.4\t95.4\n-17.5\t95.7\n-17.6\t96\n-17.7\t96.3\n-17.8\t96.6\n-17.9\t96.9\n-18\t97.2\n-18.1\t97.5\n-18.2\t97.3\n-18.3\t97.1\n-18.4\t96.9\n-18.5\t96.7\n-18.6\t96.5\n-18.7\t96.3\n-18.8\t96.1\n-18.9\t95.9\n-19\t95.7\n-19.1\t95.5\n-19.2\t95.3\n-19.3\t95.1\n-19.4\t94.9\n-19.5\t94.7\n-19.6\t94.5\n-19.7\t94.3\n-19.8\t94.1\n-19.9\t93.9\n-20\t93.7\n-20.1\t93.5\n-20.2\t93.3\n-20.3\t93.1\n-20.4\t92.9\n-20.5\t92.7\n-20.6\t92.5\n-20.7\t92.3\n-20.8\t92.1\n-20.9\t91.9\n-21\t91.7\n-21.1\t91.5\n-21.2\t91.3\n-21.3\t91.1\n-21.4\t90.9\n-21.5\t90.7\n-21.6\t90.5\n-21.7\t90.3\n-21.8\t90.1\n-21.9\t89.9\n-22\t89.7\n-22.1\t89.5\n-22.2\t89.3\n-22.3\t89.1\n-22.4\t88.9\n-22.5\t88.7\n-22.6\t88.5\n-22.7\t88.3\n-22.8\t88.1\n-22.9\t87.9\n-23\t87.7\n-23.1\t87.5\n-23.2\t87.3\n-23.3\t87.1\n-23.4\t86.9\n-23.5\t86.7\n-23.6\t86.5\n-23.7\t86.3\n-23.8\t86.1\n-23.9\t85.9\n-24\t85.7\n-24.1\t85.5\n-24.2\t85.3\n-24.3\t85.1\n-24.4\t84.9\n-24.5\t84.7\n-24.6\t84.5\n-24.7\t84.3\n-24.8\t84.1\n-24.9\t83.9\n-25\t83.7\n-25.1\t83.5\n-25.2\t83.3\n-25.3\t83.1\n-25.4\t82.9\n-25.5\t82.7\n-25.6\t82.5\n-25.7\t82.3\n-25.8\t82.1\n-25.9\t81.9\n-26\t81.7\n-26.1\t81.5\n-26.2\t81.3\n-26.3\t81.1\n-26.4\t80.9\n-26.5\t80.7\n-26.6\t80.5\n-26.7\t80.3\n-26.8\t80.1\n-26.9\t79.9\n-27\t79.7\n-27.1\t79.5\n-27.2\t79.3\n-27.3\t79.1\n-27.4\t78.9\n-27.5\t78.7\n-27.6\t78.5\n-27.7\t78.3\n-27.8\t78.1\n-27.9\t77.9\n-28\t77.7\n-28.1\t77.5\n-28.2\t77.3\n-28.3\t77.1\n-28.4\t76.9\n-28.5\t76.7\n-28.6\t76.5\n-28.7\t76.3\n-28.8\t76.1\n-28.9\t75.9\n-29\t75.7\n-29.1\t75.5\n-29.2\t75.3\n-29.3\t75.1\n-29.4\t74.9\n-29.5\t74.7\n-29.6\t74.5\n-29.7\t74.3\n-29.8\t74.1\n-29.9\t73.9\n-30\t73.7\n-30.1\t73.5\n-30.2\t73.3\n-30.3\t73.1\n-30.4\t72.9\n-30.5\t72.7\n-30.6\t72.5\n-30.7\t72.3\n-30.8\t72.1\n-30.9\t71.9\n-31\t71.7\n-31.1\t71.5\n-31.2\t71.3\n-31.3\t71.1\n-31.4\t70.9\n-31.5\t70.7\n-31.6\t70.5\n-31.7\t70.3\n-31.8\t70.1\n-31.9\t69.9\n-32\t69.7\n-32.1\t69.5\n-32.2\t69.3\n-32.3\t69.1\n-32.4\t68.9\n-32.5\t68.7\n-32.6\t68.5\n-32.7\t68.3\n-32.8\t68.1\n-32.9\t67.9\n-33\t67.7\n-33.1\t67.5\n-33.2\t67.3\n-33.3\t67.1\n-33.4\t66.9\n-33.5\t66.7\n-33.6\t66.5\n-33.7\t66.3\n-33.8\t66.1\n-33.9\t65.9\n-34\t65.7\n-34.1\t65.5\n-34.2\t65.3\n-34.3\t65.1\n-34.4\t64.9\n-34.5\t64.7\n-34.6\t64.5\n-34.7\t64.3\n-34.8\t64.1\n-34.9\t63.9\n-35\t63.7\n-35.1\t63.5\n-35.2\t63.3\n-35.3\t63.1\n-35.4\t62.9\n-35.5\t62.7\n-35.6\t62.5\n-35.7\t62.3\n-35.8\t62.1\n-35.9\t61.9\n-36\t61.7\n-36.1\t61.5\n-36.2\t61.3\n-36.3\t61.1\n-36.4\t60.9\n-36.5\t60.7\n-36.6\t60.5\n-36.7\t60.3\n-36.8\t60.1\n-36.9\t59.9\n-37\t59.7\n-37.1\t59.5\n-37.2\t59.3\n-37.3\t59.1\n-37.4\t58.9\n-37.5\t58.7\n-37.6\t58.5\n-37.7\t58.3\n-37.8\t58.1\n-37.9\t57.9\n-38\t57.7\n-38.1\t57.5\n-38.2\t57.3\n-38.3\t57.1\n-38.4\t56.9\n-38.5\t56.7\n-38.6\t56.5\n-38.7\t56.3\n-38.8\t56.1\n-38.9\t55.9\n-39\t55.7\n-39.1\t55.5\n-39.2\t55.3\n-39.3\t55.1\n-39.4\t54.9\n-39.5\t54.7\n-39.6\t54.5\n-39.7\t54.3\n-39.8\t54.1\n-39.9\t53.9\n-40\t53.7\n-40.1\t53.5\n-40.2\t53.3\n-40.3\t53.1\n-40.4\t52.9\n-40.5\t52.7\n-40.6\t52.5\n-40.7\t52.3\n-40.8\t52.1\n-40.9\t51.9\n-41\t51.7\n-41.1\t51.5\n-41.2\t51.3\n-41.3\t51.1\n-41.4\t50.9\n-41.5\t50.7\n-41.6\t50.5\n-41.7\t50.3\n-41.8\t50.1\n-41.9\t49.9\n-42\t49.7\n-42.1\t49.5\n-42.2\t49.3\n-42.3\t49.1\n-42.4\t48.9\n-42.5\t48.7\n-42.6\t48.5\n-42.7\t48.3\n-42.8\t48.1\n-42.9\t47.9\n-43\t47.7\n-43.1\t47.5\n-43.2\t47.3\n-43.3\t47.1\n-43.4\t46.9\n-43.5\t46.7\n-43.6\t46.5\n-43.7\t46.3\n-43.8\t46.1\n-43.9\t45.9\n-44\t45.7\n-44.1\t45.5\n-44.2\t45.3\n-44.3\t45.1\n-44.4\t44.9\n-44.5\t44.7\n-44.6\t44.5\n-44.7\t44.3\n-44.8\t44.1\n-44.9\t43.9\n-45\t43.7\n-45.1\t43.5\n-45.2\t43.3\n-45.3\t43.1\n-45.4\t42.9\n-45.5\t42.7\n-45.6\t42.5\n-45.7\t42.3\n-45.8\t42.1\n-45.9\t41.9\n-46\t41.7\n-46.1\t41.5\n-46.2\t41.3\n-46.3\t41.1\n-46.4\t40.9\n-46.5\t40.7\n-46.6\t40.5\n-46.7\t40.3\n-46.8\t40.1\n-46.9\t39.9\n-47\t39.7\n-47.1\t39.5\n-47.2\t39.3\n-47.3\t39.1\n-47.4\t38.9\n-47.5\t38.7\n-47.6\t38.5\n-47.7\t38.3\n-47.8\t38.1\n-47.9\t37.9\n-48\t37.7\n-48.1\t37.5\n-48.2\t37.3\n-48.3\t37.1\n-48.4\t36.9\n-48.5\t36.7\n-48.6\t36.5\n-48.7\t36.3\n-48.8\t36.1\n-48.9\t35.9\n-49\t35.7\n-49.1\t35.5\n-49.2\t35.3\n-49.3\t35.1\n-49.4\t34.9\n-49.5\t34.7\n-49.6\t34.5\n-49.7\t34.3\n-49.8\t34.1\n-49.9\t33.9\n-50\t33.7\n-50.1\t33.5\n-50.2\t33.3\n-50.3\t33.1\n-50.4\t32.9\n-50.5\t32.7\n-50.6\t32.5\n-50.7\t32.3\n-50.8\t32.1\n-50.9\t31.9\n-51\t31.7\n-51.1\t31.5\n-51.2\t31.3\n-51.3\t31.1\n-51.4\t30.9\n-51.5\t30.7\n-51.6\t30.5\n-51.7\t30.3\n-51.8\t30.1\n-51.9\t29.9\n-52\t29.7\n-52.1\t29.5\n-52.2\t29.3\n-52.3\t29.1\n-52.4\t28.9\n-52.5\t28.7\n-52.6\t28.5\n-52.7\t28.3\n-52.8\t28.1\n-52.9\t27.9\n-53\t27.7\n-53.1\t27.5\n-53.2\t27.3\n-53.3\t27.1\n-53.4\t26.9\n-53.5\t26.7\n-53.6\t26.5\n-53.7\t26.3\n-53.8\t26.1\n-53.9\t25.9\n-54\t25.7\n-54.1\t25.5\n-54.2\t25.3\n-54.3\t25.1\n-54.4\t24.9\n-54.5\t24.7\n-54.6\t24.5\n-54.7\t24.3\n-54.8\t24.1\n-54.9\t23.9\n-55\t23.7\n-55.1\t23.5\n-55.2\t23.3\n-55.3\t23.1\n-55.4\t22.9\n-55.5\t22.7\n-55.6\t22.5\n-55.7\t22.3\n-55.8\t22.1\n-55.9\t21.9\n-56\t21.7\n-56.1\t21.5\n-56.2\t21.3\n-56.3\t21.1\n-56.4\t20.9\n-56.5\t20.7\n-56.6\t20.5\n-56.7\t20.3\n-56.8\t20.1\n-56.9\t19.9\n-57\t19.7\n-57.1\t19.5\n-57.2\t19.3\n-57.3\t19.1\n-57.4\t18.9\n-57.5\t18.7\n-57.6\t18.5\n-57.7\t18.3\n-57.8\t18.1\n-57.9\t17.9\n-58\t17.7\n-58.1\t17.5\n-58.2\t17.3\n-58.3\t17.1\n-58.4\t16.9\n-58.5\t16.7\n-58.6\t16.5\n-58.7\t16.3\n-58.8\t16.1\n-58.9\t15.9\n-59\t15.7\n-59.1\t15.5\n-59.2\t15.3\n-59.3\t15.1\n-59.4\t14.9\n-59.5\t14.7\n-59.6\t14.5\n-59.7\t14.3\n-59.8\t14.1\n-59.9\t13.9\n-60\t13.7\n-60.1\t13.5\n-60.2\t13.3\n-60.3\t13.1\n-60.4\t12.9\n-60.5\t12.7\n-60.6\t12.5\n-60.7\t12.3\n-60.8\t12.1\n-60.9\t11.9\n-61\t11.7\n-61.1\t11.5\n-61.2\t11.3\n-61.3\t11.1\n-61.4\t10.9\n-61.5\t10.7\n-61.6\t11.3\n-61.7\t11.9\n-61.8\t12.5\n-61.9\t13.1\n-62\t13.7\n-62.1\t14.3\n-62.2\t14.9\n-62.3\t15.5\n-62.4\t16.1\n-62.5\t16.7\n-62.6\t17.3\n-62.7\t17.9\n-62.8\t18.5\n-62.9\t19.1\n-63\t19.7\n-63.1\t20.3\n-63.2\t20.9\n-63.3\t21.5\n-63.4\t22.1\n-63.5\t22.7\n-63.6\t23.3\n-63.7\t23.9\n-63.8\t24.5\n-63.9\t25.1\n-64\t25.7\n-64.1\t26.3\n-64.2\t26.9\n-64.3\t27.5\n-64.4\t28.1\n-64.5\t28.7\n-64.6\t29.3\n-64.7\t29.9\n-64.8\t30.5\n-63.8\t31.1\n-62.8\t31.7\n-61.8\t32.3\n-60.8\t32.9\n-59.8\t33.5\n-58.8\t34.1\n-57.8\t34.7\n-56.8\t35.3\n-55.8\t35.9\n-54.8\t36.5\n-53.8\t37.1\n-52.8\t37.7\n-51.8\t38.3\n-50.8\t38.9\n-49.8\t39.5\n-48.8\t40.1\n-47.8\t40.7\n-46.8\t41.3\n-45.8\t41.9\n-44.8\t42.5\n-43.8\t43.1\n-42.8\t43.7\n-41.8\t44.3\n-40.8\t44.9\n-39.8\t45.5\n-38.8\t46.1\n-37.8\t46.7\n-36.8\t47.3\n-35.8\t47.9\n-34.8\t48.5\n-33.8\t49.1\n-32.8\t49.7\n-31.8\t50.3\n-30.8\t50.9\n-29.8\t51.5\n-28.8\t52.1\n-27.8\t52.7\n-26.8\t53.3\n-25.8\t53.9\n-24.8\t54.5\n-23.8\t55.1\n-22.8\t55.7\n-21.8\t56.3\n-20.8\t56.9\n-19.8\t57.5\n-18.8\t58.1\n-17.8\t58.7\n-16.8\t59.3\n-15.8\t59.9\n-14.8\t60.5\n-13.8\t61.1\n-12.8\t61.7\n-11.8\t62.3\n-10.8\t62.9\n-9.8\t63.5\n-8.8\t64.1\n-7.8\t64.7\n-6.8\t65.3\n-5.8\t65.9\n-4.8\t66.5\n-3.8\t67.1\n-2.8\t67.7\n-1.8\t68.3\n-0.8\t68.9\n0.2\t69.5\n1.2\t70.1\n2.2\t70.7\n3.2\t71.3\n4.2\t71.9\n5.2\t72.5\n6.2\t73.1\n7.2\t73.7\n8.2\t74.3\n9.2\t74.9\n10.2\t75.5\n11.2\t76.1\n12.2\t76.7\n13.2\t77.3\n14.2\t77.9\n15.2\t78.5\n16.2\t79.1\n17.2\t79.7\n18.2\t80.3\n19.2\t80.9\n20.2\t81.5\n21.2\t82.1\n22.2\t82.7\n23.2\t83.3\n24.2\t83.9\n25.2\t84.5\n26.2\t85.1\n27.2\t85.7\n28.2\t86.3\n29.2\t86.9\n30.2\t87.5\n31.2\t88.1\n32.2\t88.7\n33.2\t89.3\n34.2\t89.9\n35.2\t90.5\n36.2\t91.1\n37.2\t91.7\n38.2\t92.3\n39.2\t92.9\n40.2\t93.5\n41.2\t94.1\n42.2\t93.8\n43.2\t93.5\n44.2\t93.2\n45.2\t92.9\n46.2\t92.6\n47.2\t92.3\n48.2\t92\n49.2\t91.7\n50.2\t91.4\n51.2\t91.1\n52.2\t90.8\n53.2\t90.5\n54.2\t90.2\n55.2\t89.9\n56.2\t89.6\n57.2\t89.3\n58.2\t89\n59.2\t88.7\n60.2\t88.4\n61.2\t88.1\n62.2\t87.8\n63.2\t87.5\n64.2\t87.2\n65.2\t86.9\n66.2\t86.6\n67.2\t86.3\n68.2\t86\n69.2\t85.7\n70.2\t85.4\n71.2\t85.1\n72.2\t84.8\n73.2\t84.5\n74.2\t84.2\n75.2\t83.9\n76.2\t83.6\n77.2\t83.3\n78.2\t83\n79.2\t82.7\n80.2\t82.4\n81.2\t82.1\n82.2\t81.8\n83.2\t81.5\n84.2\t81.2\n85.2\t80.9\n86.2\t80.6\n87.2\t80.3\n88.2\t80\n89.2\t79.7\n90.2\t79.4\n91.2\t79.1\n92.2\t78.8\n93.2\t78.5\n94.2\t78.2\n93.8\t77.9\n93.4\t77.6\n93\t77.3\n92.6\t77\n92.2\t76.7\n91.8\t76.4\n91.4\t76.1\n91\t75.8\n90.6\t75.5\n90.2\t75.2\n89.8\t74.9\n89.4\t74.6\n89\t74.3\n88.6\t74\n88.2\t73.7\n87.8\t73.4\n87.4\t73.1\n87\t72.8\n86.6\t72.5\n86.2\t72.2\n85.8\t71.9\n85.4\t71.6\n85\t71.3\n84.6\t71\n84.2\t70.7\n83.8\t70.4\n83.4\t70.1\n83\t69.8\n82.6\t69.5\n82.2\t69.2\n81.8\t68.9\n81.4\t68.6\n81\t68.3\n80.6\t68\n80.2\t67.7\n79.8\t67.4\n79.4\t67.1\n79\t66.8\n78.6\t66.5\n78.2\t66.2\n77.8\t65.9\n77.4\t65.6\n77\t65.3\n76.6\t65\n76.2\t64.7\n75.8\t64.4\n75.4\t64.1\n75\t63.8\n74.6\t63.5\n74.2\t63.2\n73.8\t62.9\n73.4\t62.6\n73\t62.3\n72.6\t62\n72.2\t61.7\n71.8\t61.4\n71.4\t61.1\n71\t60.8\n70.6\t60.5\n70.2\t60.2\n69.8\t59.9\n69.4\t59.6\n69\t59.3\n68.6\t59\n68.2\t58.7\n67.8\t58.4\n67.4\t58.1\n67\t57.8\n66.6\t57.5\n66.2\t57.2\n65.8\t56.9\n65.4\t56.6\n65\t56.3\n64.6\t56\n64.2\t55.7\n63.8\t55.4\n63.4\t55.1\n63\t54.8\n62.6\t54.5\n62.2\t54.2\n61.8\t53.9\n61.4\t53.6\n61\t53.3\n60.6\t53\n60.2\t52.7\n59.8\t52.4\n59.4\t52.1\n59\t51.8\n58.6\t51.5\n58.2\t51.2\n57.8\t50.9\n57.4\t50.6\n57\t50.3\n56.6\t50\n56.2\t49.7\n55.8\t49.4\n55.4\t49.1\n55\t48.8\n54.6\t48.5\n54.2\t48.2\n53.8\t47.9\n53.4\t47.6\n53\t47.3\n52.6\t47\n52.2\t46.7\n51.8\t46.4\n51.4\t46.1\n51\t45.8\n50.6\t45.5\n50.2\t45.2\n49.8\t44.9\n49.4\t44.6\n49\t44.3\n48.6\t44\n48.2\t43.7\n47.8\t43.4\n47.4\t43.1\n47\t42.8\n46.6\t42.5\n46.2\t42.2\n45.8\t41.9\n45.4\t41.6\n45\t41.3\n44.6\t41\n44.2\t40.7\n43.8\t40.4\n43.4\t40.1\n43\t39.8\n42.6\t39.5\n42.2\t39.2\n41.8\t38.9\n41.4\t38.6\n41\t38.3\n40.6\t38\n40.2\t37.7\n39.8\t37.4\n39.4\t37.1\n39\t36.8\n38.6\t36.5\n38.2\t36.2\n37.8\t35.9\n37.4\t35.6\n37\t35.3\n36.6\t35\n36.2\t34.7\n35.8\t34.4\n35.4\t34.1\n35\t33.8\n34.6\t33.5\n34.2\t33.2\n33.8\t32.9\n33.4\t32.6\n33\t32.3\n32.6\t32\n32.2\t31.7\n31.8\t31.4\n31.4\t31.1\n31\t30.8\n30.6\t30.5\n30.2\t30.2\n29.8\t29.9\n29.4\t29.6\n29\t29.3\n28.6\t29\n28.2\t28.7\n27.8\t28.4\n27.4\t28.1\n27\t27.8\n26.6\t27.5\n26.2\t27.2\n25.8\t26.9\n25.4\t26.6\n25\t26.3\n24.6\t26\n24.2\t25.7\n23.8\t25.4\n23.4\t25.1\n23\t24.8\n22.6\t24.5\n22.2\t24.2\n21.8\t23.9\n21.4\t23.6\n21\t23.3\n20.6\t23\n20.2\t22.7\n19.8\t22.4\n19.4\t22.1\n19\t21.8\n18.6\t21.5\n18.2\t21.2\n17.8\t20.9\n17.4\t20.6\n17\t20.3\n16.6\t20\n16.2\t19.7\n15.8\t19.4\n15.4\t19.1\n15\t18.8\n14.6\t18.5\n14.2\t18.2\n13.8\t17.9\n13.4\t17.6\n13\t17.3\n12.6\t17\n12.2\t16.7\n11.8\t16.4\n11.4\t16.1\n11\t15.8\n10.6\t15.5\n10.2\t15.2\n9.8\t14.9\n9.4\t14.6\n9\t14.3\n8.6\t14\n8.2\t13.7\n7.8\t13.4\n7.4\t13.1\n7\t12.8\n6.6\t12.5\n6.2\t12.2\n5.8\t11.9\n5.4\t11.6\n5\t11.3\n4.6\t11\n4.2\t10.7\n3.8\t10.4\n3.4\t10.1\n3\t9.8\n2.8\t9.5\n2.6\t9.2\n2.4\t8.9\n2.2\t8.6\n2\t8.3\n1.8\t8\n1.6\t7.7\n1.4\t7.4\n1.2\t7.1\n1\t6.8\n0.8\t6.5\n0.6\t6.2\n0.4\t5.9\n0.2\t5.6\n-3.57486E-12\t5.3\n-0.2\t5\n-0.4\t4.7\n-0.6\t4.4\n-0.8\t4.1\n-1\t3.8\n-1.2\t3.5\n-1.4\t3.2\n-1.6\t2.9\n-1.8\t2.6\n-2\t2.3\n-2.2\t2\n-2.4\t1.7\n-2.6\t1.4\n-2.8\t1.1\n-3\t0.8\n-3.2\t0.5\n-3.4\t0.2\n-3.6\t-0.1\n-3.8\t-0.4\n-4\t-0.7\n-4.2\t-1\n-4.4\t-1.3\n-4.6\t-1.6\n-4.8\t-1.9\n-5\t-2.2\n-5.2\t-2.5\n-5.4\t-2.8\n-5.6\t-3.1\n-5.8\t-3.4\n-6\t-3.7\n-6.2\t-4\n-6.4\t-4.3\n-6.6\t-4.6\n-6.8\t-4.9\n-7\t-5.2\n-7.2\t-5.5\n-7.4\t-5.8\n-7.6\t-6.1\n-7.8\t-6.4\n-8\t-6.7\n-8.2\t-7\n-8.4\t-7.3\n-8.6\t-7.6\n-8.8\t-7.9\n-9\t-8.2\n-9.2\t-8.5\n-9.4\t-8.8\n-9.6\t-9.1\n-9.8\t-9.4\n-10\t-9.7\n-10.2\t-10\n-10.4\t-10.3\n-10.6\t-10.6\n-10.8\t-10.9\n-11\t-11.2\n-11.2\t-11.5\n-11.4\t-11.8\n-11.6\t-12.1\n-11.8\t-12.4\n-12\t-12.7\n-12.2\t-13\n-12.4\t-13.3\n-12.6\t-13.6\n-12.8\t-13.9\n-13\t-14.2\n-13.2\t-14.5\n-13.4\t-14.8\n-13.6\t-15.1\n-13.8\t-15.4\n-14\t-15.7\n-14.2\t-16\n-14.4\t-16.3\n-14.6\t-16.6\n-14.8\t-16.9\n-15\t-17.2\n-15.2\t-17.5\n-15.4\t-17.8\n-15.6\t-18.1\n-15.8\t-18.4\n-16\t-18.7\n-16.2\t-19\n-16.4\t-19.3\n-16.6\t-19.6\n-16.8\t-19.9\n-17\t-20.2\n-17.2\t-20.5\n-17.4\t-20.8\n-17.6\t-21.1\n-17.8\t-21.4\n-18\t-21.7\n-18.2\t-22\n-18.4\t-22.3\n-18.6\t-22.6\n-18.8\t-22.9\n-19\t-23.2\n-19.2\t-23.5\n-19.4\t-23.8\n-19.6\t-24.1\n-19.8\t-24.4\n-20\t-24.7\n-20.2\t-25\n-20.4\t-25.3\n-20.6\t-25.6\n-20.8\t-25.9\n-21\t-26.2\n-21.2\t-26.5\n-21.4\t-26.8\n-21.6\t-27.1\n-21.8\t-27.4\n-22\t-27.7\n-22.2\t-28\n-22.4\t-28.3\n-22.6\t-28.6\n-22.8\t-28.9\n-23\t-29.2\n-23.2\t-29.5\n-23.4\t-29.8\n-23.6\t-30.1\n-23.8\t-30.4\n-24\t-30.7\n-24.2\t-31\n-24.4\t-31.3\n-24.6\t-31.6\n-24.8\t-31.9\n-25\t-32.2\n-25.2\t-32.5\n-25.4\t-32.8\n-25.6\t-33.1\n-25.8\t-33.4\n-26\t-33.7\n-26.2\t-34\n-26.4\t-34.3\n-26.6\t-34.6\n-26.8\t-34.9\n-27\t-35.2\n-27.2\t-35.5\n-27.4\t-35.8\n-27.6\t-36.1\n-27.8\t-36.4\n-28\t-36.7\n-28.2\t-37\n-28.4\t-37.3\n-28.6\t-37.6\n-28.8\t-37.9\n-29\t-38.2\n-29.2\t-38.5\n-29.4\t-38.8\n-29.6\t-39.1\n-29.8\t-39.4\n-30\t-39.7\n-30.2\t-40\n-30.4\t-40.3\n-30.6\t-40.6\n-30.8\t-40.9\n-31\t-41.2\n-31.2\t-41.5\n-31.4\t-41.8\n-31.6\t-42.1\n-31.8\t-42.4\n-32\t-42.7\n-32.2\t-43\n-32.4\t-43.3\n-32.6\t-43.6\n-32.8\t-43.9\n-33\t-44.2\n-33.2\t-44.5\n-33.4\t-44.8\n-33.6\t-45.1\n-33.8\t-45.4\n-34\t-45.7\n-34.2\t-46\n-34.4\t-46.3\n-34.6\t-46.6\n-34.8\t-46.9\n-35\t-47.2\n-35.2\t-47.5\n-35.4\t-47.8\n-35.6\t-48.1\n-35.8\t-48.4\n-36\t-48.7\n-36.2\t-49\n-36.4\t-49.3\n-36.6\t-49.6\n-36.8\t-49.9\n-37\t-50.2\n-37.2\t-50.5\n-37.4\t-50.8\n-37.6\t-51.1\n-37.8\t-51.4\n-38\t-51.7\n-38.2\t-52\n-38.4\t-52.3\n-38.6\t-52.6\n-38.8\t-52.9\n-39\t-53.2\n-39.2\t-53.5\n-39.4\t-53.8\n-39.6\t-54.1\n-39.8\t-54.4\n-40\t-54.7\n-40.2\t-55\n-40.4\t-55.3\n-40.6\t-55.6\n-40.8\t-55.9\n-41\t-56.2\n-41.2\t-56.5\n-41.4\t-56.8\n-41.6\t-57.1\n-41.8\t-57.4\n-42\t-57.7\n-42.2\t-58\n-42.4\t-58.3\n-42.6\t-58.6\n-42.8\t-58.9\n-43\t-59.2\n-43.2\t-59.5\n-43.4\t-59.8\n-43.6\t-60.1\n-43.8\t-60.4\n-44\t-60.7\n-44.2\t-61\n-44.4\t-61.3\n-44.6\t-61.6\n-44.8\t-61.9\n-45\t-62.2\n-45.2\t-62.5\n-45.4\t-62.8\n-45.6\t-63.1\n-45.8\t-63.4\n-46\t-63.7\n-46.2\t-64\n-46.4\t-64.3\n-46.6\t-64.6\n-46.8\t-64.9\n-47\t-65.2\n-47.2\t-65.5\n-47.4\t-65.8\n-47.6\t-66.1\n-47.8\t-66.4\n-48\t-65.8\n-48.2\t-65.2\n-48.4\t-64.6\n-48.6\t-64\n-48.8\t-63.4\n-49\t-62.8\n-49.2\t-62.2\n-49.4\t-61.6\n-49.6\t-61\n-49.8\t-60.4\n-50\t-59.8\n-50.2\t-59.2\n-50.4\t-58.6\n-50.6\t-58\n-50.8\t-57.4\n-51\t-56.8\n-51.2\t-56.2\n-51.4\t-55.6\n-51.6\t-55\n-51.8\t-54.4\n-52\t-53.8\n-52.2\t-53.2\n-52.4\t-52.6\n-52.6\t-52\n-52.8\t-51.4\n-53\t-50.8\n-53.2\t-50.2\n-53.4\t-49.6\n-53.6\t-49\n-53.8\t-48.4\n-54\t-47.8\n-54.2\t-47.2\n-54.4\t-46.6\n-54.6\t-46\n-54.8\t-45.4\n-55\t-44.8\n-55.2\t-44.2\n-55.4\t-43.6\n-55.6\t-43\n-55.8\t-42.4\n-56\t-41.8\n-56.2\t-41.2\n-56.4\t-40.6\n-56.6\t-40\n-56.8\t-39.4\n-57\t-38.8\n-57.2\t-38.2\n-57.4\t-37.6\n-57.6\t-37\n-57.8\t-36.4\n-58\t-35.8\n-58.2\t-35.2\n-58.4\t-34.6\n-58.6\t-34\n-58.8\t-33.4\n-59\t-32.8\n-59.2\t-32.2\n-59.4\t-31.6\n-59.6\t-31\n-59.8\t-30.4\n-60\t-29.8\n-60.2\t-29.2\n-60.4\t-28.6\n-60.6\t-28\n-60.8\t-27.4\n-61\t-26.8\n-61.2\t-26.2\n-61.4\t-25.6\n-61.6\t-25\n-61.8\t-24.4\n-61.1\t-23.8\n-60.4\t-23.2\n-59.7\t-22.6\n-59\t-22\n-58.3\t-21.4\n-57.6\t-20.8\n-56.9\t-20.2\n-56.2\t-19.6\n-55.5\t-19\n-54.8\t-18.4\n-54.1\t-17.8\n-53.4\t-17.2\n-52.7\t-16.6\n-52\t-16\n-51.3\t-15.4\n-50.6\t-14.8\n-49.9\t-14.2\n-49.2\t-13.6\n-48.5\t-13\n-47.8\t-12.4\n-47.1\t-11.8\n-46.4\t-11.2\n-45.7\t-10.6\n-45\t-10\n-44.3\t-9.4\n-43.6\t-8.8\n-42.9\t-8.2\n-42.2\t-7.6\n-41.5\t-7\n-40.8\t-6.4\n-40.1\t-5.8\n-39.4\t-5.2\n-38.7\t-4.6\n-38\t-4\n-37.3\t-3.4\n-36.6\t-2.8\n-35.9\t-2.2\n-35.2\t-1.6\n-34.5\t-1\n-33.8\t-0.4\n-33.1\t0.2\n-32.4\t0.8\n-31.7\t1.4\n-31\t2\n-30.3\t2.6\n-29.6\t3.2\n-28.9\t3.8\n-28.2\t4.4\n-27.5\t5\n-26.8\t5.6\n-26.1\t6.2\n-25.4\t6.8\n-24.7\t7.4\n-24\t8\n-23.3\t8.6\n-22.6\t9.2\n-21.9\t9.8\n-21.2\t10.4\n-20.5\t11\n-19.8\t11.6\n-19.1\t12.2\n-18.4\t12.8\n-17.7\t13.4\n-17\t14\n-16.3\t14.6\n-15.6\t15.2\n-14.9\t15.8\n-14.2\t16.4\n-13.5\t17\n-12.8\t17.6\n-12.1\t18.2\n-11.4\t18.8\n-10.7\t19.4\n-10\t20\n-9.3\t20.6\n-8.6\t21.2\n-7.9\t21.8\n-7.2\t22.4\n-6.5\t23\n-5.8\t23.6\n-5.1\t24.2\n-4.4\t24.8\n-3.7\t25.4\n-3\t26\n-2.3\t26.6\n-1.6\t27.2\n-0.9\t27.8\n-0.2\t28.4\n0.5\t29\n1.2\t29.6\n1.9\t30.2\n2.6\t30.8\n3.3\t31.4\n4\t32\n4.7\t32.6\n5.4\t33.2\n6.1\t33.8\n6.8\t34.4\n7.5\t35\n8.2\t35.6\n8.9\t36.2\n9.6\t36.8\n10.3\t37.4\n11\t38\n11.7\t38.6\n12.4\t39.2\n13.1\t39.8\n13.8\t40.4\n14.5\t40.1\n15.2\t39.8\n15.9\t39.5\n16.6\t39.2\n17.3\t38.9\n18\t38.6\n18.7\t38.3\n19.4\t38\n20.1\t37.7\n20.8\t37.4\n21.5\t37.1\n22.2\t36.8\n22.9\t36.5\n23.6\t36.2\n24.3\t35.9\n25\t35.6\n25.7\t35.3\n26.4\t35\n27.1\t34.7\n27.8\t34.4\n28.5\t34.1\n29.2\t33.8\n29.9\t33.5\n30.6\t33.2\n31.3\t32.9\n32\t32.6\n32.7\t32.3\n33.4\t32\n34.1\t31.7\n34.8\t31.4\n35.5\t31.1\n36.2\t30.8\n36.9\t30.5\n37.6\t30.2\n38.3\t29.9\n39\t29.6\n39.7\t29.3\n40.4\t29\n41.1\t28.7\n41.8\t28.4\n42.5\t28.1\n43.2\t27.8\n43.9\t27.5\n44.6\t27.2\n45.3\t26.9\n46\t26.6\n46.7\t26.3\n47.4\t26\n48.1\t25.7\n48.8\t25.4\n49.5\t25.1\n50.2\t24.8\n50.9\t24.5\n51.6\t24.2\n52.3\t23.9\n53\t23.6\n53.7\t23.3\n54.4\t23\n55.1\t22.7\n55.8\t22.4\n56.5\t22.1\n57.2\t21.8\n57.9\t21.5\n58.6\t21.2\n59.3\t20.9\n60\t20.6\n60.7\t20.3\n61.4\t20\n62.1\t19.7\n62.8\t19.4\n63.5\t19.1\n64.2\t18.8\n64.9\t18.5\n65.6\t18.2\n66.3\t17.9\n67\t17.6\n67.7\t17.3\n68.4\t17\n69.1\t16.7\n69.8\t16.4\n70.5\t16.1\n71.2\t15.8\n71.9\t15.5\n72.6\t15.2\n73.3\t14.9\n74\t14.6\n74.7\t14.3\n75.4\t14\n76.1\t13.7\n76.8\t13.4\n77.5\t13.1\n78.2\t12.8\n78.9\t12.5\n79.6\t12.2\n80.3\t11.9\n81\t11.6\n81.7\t11.3\n82.4\t11\n83.1\t10.7\n83.8\t10.4\n84.5\t10.1\n85.2\t9.8\n85.9\t9.5\n86.6\t9.2\n87.3\t8.9\n88\t8.6\n88.7\t8.3\n88.3\t8\n87.9\t7.7\n87.5\t7.4\n87.1\t7.1\n86.7\t6.8\n86.3\t6.5\n85.9\t6.2\n85.5\t5.9\n85.1\t5.6\n84.7\t5.3\n84.3\t5\n83.9\t4.7\n83.5\t4.4\n83.1\t4.1\n82.7\t3.8\n82.3\t3.5\n81.9\t3.2\n81.5\t2.9\n81.1\t2.6\n80.7\t2.3\n80.3\t2\n79.9\t1.7\n79.5\t1.4\n79.1\t1.1\n78.7\t0.8\n78.3\t0.5\n77.9\t0.2\n77.5\t-0.1\n77.1\t-0.4\n76.7\t-0.7\n76.3\t-1\n75.9\t-1.3\n75.5\t-1.6\n75.1\t-1.9\n74.7\t-2.2\n74.3\t-2.5\n73.9\t-2.8\n73.5\t-3.1\n73.1\t-3.4\n72.7\t-3.7\n72.3\t-4\n71.9\t-4.3\n71.5\t-4.6\n71.1\t-4.9\n70.7\t-5.2\n70.3\t-5.5\n69.9\t-5.8\n69.5\t-6.1\n69.1\t-6.4\n68.7\t-6.7\n68.3\t-7\n67.9\t-7.3\n67.5\t-7.6\n67.1\t-7.9\n66.7\t-8.2\n66.3\t-8.5\n65.9\t-8.8\n65.5\t-9.1\n65.1\t-9.4\n64.7\t-9.7\n64.3\t-10\n63.9\t-10.3\n63.5\t-10.6\n63.1\t-10.9\n62.7\t-11.2\n62.3\t-11.5\n61.9\t-11.8\n61.5\t-12.1\n61.1\t-12.4\n60.7\t-12.7\n60.3\t-13\n59.9\t-13.3\n59.5\t-13.6\n59.1\t-13.9\n58.7\t-14.2\n58.3\t-14.5\n57.9\t-14.8\n57.5\t-15.1\n57.1\t-15.4\n56.7\t-15.7\n56.3\t-16\n55.9\t-16.3\n55.5\t-16.6\n55.1\t-16.9\n54.7\t-17.2\n54.3\t-17.5\n53.9\t-17.8\n53.5\t-18.1\n53.1\t-18.4\n52.7\t-18.7\n52.3\t-19\n51.9\t-19.3\n51.5\t-19.6\n51.1\t-19.9\n50.7\t-20.2\n50.3\t-20.5\n49.9\t-20.8\n49.5\t-21.1\n49.1\t-21.4\n48.7\t-21.7\n48.3\t-22\n47.9\t-22.3\n47.5\t-22.6\n47.1\t-22.9\n46.7\t-23.2\n46.3\t-23.5\n45.9\t-23.8\n45.5\t-24.1\n45.1\t-24.4\n44.7\t-24.7\n44.3\t-25\n43.9\t-25.3\n43.5\t-25.6\n43.1\t-25.9\n42.7\t-26.2\n42.3\t-26.5\n41.9\t-26.8\n41.5\t-27.1\n41.1\t-27.4\n40.7\t-27.7\n40.3\t-28\n39.9\t-28.3\n39.5\t-28.6\n39.1\t-28.9\n38.7\t-29.2\n38.3\t-29.5\n37.9\t-29.8\n37.5\t-30.1\n37.1\t-30.4\n36.7\t-30.7\n36.3\t-31\n35.9\t-31.3\n35.5\t-31.6\n35.1\t-31.9\n34.7\t-32.2\n34.3\t-32.5\n33.9\t-32.8\n33.5\t-33.1\n33.1\t-33.4\n32.7\t-33.7\n32.3\t-34\n31.9\t-34.3\n31.5\t-34.6\n31.1\t-34.9\n30.7\t-35.2\n30.3\t-35.5\n29.9\t-35.8\n29.5\t-36.1\n29.1\t-36.4\n28.7\t-36.7\n28.3\t-37\n27.9\t-37.3\n27.5\t-37.6\n27.1\t-37.9\n26.7\t-38.2\n26.3\t-38.5\n25.9\t-38.8\n25.5\t-39.1\n25.1\t-39.4\n24.7\t-39.7\n24.3\t-40\n23.9\t-40.3\n23.5\t-40.6\n23.1\t-40.9\n22.7\t-41.2\n22.3\t-41.5\n21.9\t-41.8\n21.5\t-42.1\n21.1\t-42.4\n20.7\t-42.7\n20.3\t-43\n19.9\t-43.3\n19.5\t-43.6\n19.1\t-43.9\n18.7\t-44.2\n18.3\t-44.5\n17.9\t-44.8\n17.5\t-45.1\n17.1\t-45.4\n16.7\t-45.7\n16.3\t-46\n15.9\t-46.3\n15.5\t-46.6\n15.1\t-46.9\n14.7\t-47.2\n14.3\t-47.5\n13.9\t-47.8\n13.5\t-48.1\n13.1\t-48.4\n12.7\t-48.7\n12.3\t-49\n11.9\t-49.3\n11.5\t-49.6\n11.1\t-49.9\n10.7\t-50.2\n10.3\t-50.5\n9.9\t-50.8\n9.5\t-51.1\n9.1\t-51.4\n8.7\t-51.7\n8.3\t-52\n7.9\t-52.3\n7.5\t-52.6\n7.1\t-52.9\n6.7\t-53.2\n6.3\t-53.5\n5.9\t-53.8\n5.5\t-54.1\n5.1\t-54.4\n4.7\t-54.7\n4.3\t-55\n3.9\t-55.3\n3.5\t-55.6\n3.1\t-55.9\n2.7\t-56.2\n2.3\t-56.5\n1.9\t-56.8\n1.5\t-57.1\n1.1\t-57.4\n0.7\t-57.7\n0.3\t-58\n-0.1\t-58.3\n-0.5\t-58.6\n-0.9\t-58.9\n-1.3\t-59.2\n-1.7\t-59.5\n-2.1\t-59.8\n-2.5\t-60.1\n-2.9\t-60.4\n-3.3\t-60.7\n-3.7\t-61\n-4.1\t-61.3\n-4.5\t-61.6\n-4.9\t-61.9\n-5.3\t-62.2\n-5.7\t-62.5\n-6.1\t-62.8\n-6.5\t-63.1\n-6.9\t-63.4\n-7.3\t-63.7\n-7.7\t-64\n-8.1\t-64.3\n-8.5\t-64.6\n-8.9\t-64.9\n-9.3\t-65.2\n-9.7\t-65.5\n-10.1\t-65.8\n-10.5\t-66.1\n-10.9\t-66.4\n-11.3\t-66.7\n-11.7\t-67\n-12.1\t-67.3\n-12.5\t-67.6\n-12.9\t-67.9\n-13.3\t-68.2\n-13.7\t-68.5\n-14.1\t-68.8\n-14.5\t-69.1\n-14.9\t-69.4\n-15.3\t-69.7\n-15.7\t-70\n-16.1\t-70.3\n-16.5\t-70.6\n-16.9\t-70.9\n-17.3\t-71.2\n-17.7\t-71.5\n-18.1\t-71.8\n-18.5\t-72.1\n-18.9\t-72.4\n-19.3\t-72.7\n-19.7\t-73\n-20.1\t-73.3\n-20.5\t-73.6\n-20.9\t-73.9\n-21.3\t-74.2\n-21.7\t-74.5\n-22.1\t-74.8\n-22.5\t-75.1\n-22.9\t-75.4\n-23.3\t-75.7\n-23.7\t-76\n-24.1\t-76.3\n-24.5\t-76.6\n-24.9\t-76.9\n-25.3\t-77.2\n-25.7\t-77.5\n-26.1\t-77.8\n-26.5\t-78.1\n-26.9\t-78.4\n-27.3\t-78.7\n-27.7\t-79\n-28.1\t-79.3\n-28.5\t-79.6\n-28.9\t-79.9\n-29.3\t-80.2\n-29.7\t-80.5\n-30.1\t-80.8\n-30.5\t-81.1\n-30.9\t-81.4\n-31.3\t-81.7\n-31.7\t-82\n-32.1\t-82.3\n-32.5\t-82.6\n-32.9\t-82.9\n-33.3\t-83.2\n-33.7\t-83.5\n-34.1\t-83.8\n-34.5\t-84.1\n-34.9\t-84.4\n-35.3\t-84.7\n-35.7\t-85\n-36.1\t-85.3\n-36.5\t-85.6\n-36.9\t-85.9\n-37.3\t-86.2\n-37.7\t-86.5\n-38.1\t-86.8\n-38.5\t-87.1\n-38.9\t-87.4\n-39.3\t-87.7\n-39.7\t-88\n-40.1\t-88.3\n-40.5\t-88.6\n-40.9\t-88.9\n-41.3\t-89.2\n-41.7\t-89.5\n-42.1\t-89.8\n-42.5\t-90.1\n-42.9\t-90.4\n-43.3\t-90.3\n-43.7\t-90.2\n-44.1\t-90.1\n-44.5\t-90\n-44.9\t-89.9\n-45.3\t-89.8\n-45.7\t-89.7\n-46.1\t-89.6\n-46.5\t-89.5\n-46.9\t-89.4\n-47.3\t-89.3\n-47.7\t-89.2\n-48.1\t-89.1\n-48.5\t-89\n-48.9\t-88.9\n-49.3\t-88.8\n-49.7\t-88.7\n-50.1\t-88.6\n-50.5\t-88.5\n-50.9\t-88.4\n-51.3\t-88.3\n-51.7\t-88.2\n-52.1\t-88.1\n-52.5\t-88\n-52.9\t-87.9\n-53.3\t-87.8\n-53.7\t-87.7\n-54.1\t-87.6\n-54.5\t-87.5\n-54.9\t-87.4\n-55.3\t-87.3\n-55.7\t-87.2\n-56.1\t-87.1\n-56.5\t-87\n-56.9\t-86.9\n-57.3\t-86.8\n-57.7\t-86.7\n-58.1\t-86.6\n-58.5\t-86.5\n-58.9\t-86.4\n-59.3\t-86.3\n-59.7\t-86.2\n-60.1\t-86.1\n-60.5\t-86\n-60.9\t-85.9\n-61.3\t-85.8\n-61.7\t-85.7\n-62.1\t-85.6\n-62.5\t-85.5\n-62.9\t-85.4\n-63.3\t-85.3\n-63.7\t-85.2\n-64.1\t-85.1\n-64.5\t-85\n-64.9\t-84.9\n-65.3\t-84.8\n-65.7\t-84.7\n-66.1\t-84.6\n-66.5\t-84.5\n-66.9\t-84.4\n-67.3\t-84.3\n-67.7\t-84.2\n-68.1\t-84.1\n-68.5\t-84\n-68.9\t-83.9\n-69.3\t-83.8\n-69.7\t-83.7\n-70.1\t-83.6\n-70.5\t-83.5\n-70.9\t-83.4\n-71.3\t-83.3\n-71.7\t-83.2\n-72.1\t-83.1\n-72.5\t-83\n-72.9\t-82.9\n-73.3\t-82.8\n-73.7\t-82.7\n-74.1\t-82.6\n-74.5\t-82.5\n-74.9\t-82.4\n-75.3\t-82.3\n-75.7\t-82.2\n-76.1\t-82.1\n-76.5\t-82\n-76.9\t-81.9\n-77.3\t-81.8\n-77.7\t-81.7\n-78.1\t-81.6\n-78.5\t-81.5\n-78.9\t-81.4\n-79.3\t-81.3\n-79.7\t-81.2\n-80.1\t-81.1\n-80.5\t-81\n-80.9\t-80.9\n-81.3\t-80.8\n-81.7\t-80.7\n-82.1\t-80.6\n-82.5\t-80.5\n-82.9\t-80.4\n-83.3\t-80.3\n-83.7\t-80.2\n-84.1\t-80.1\n-84.5\t-80\n-84.9\t-79.9\n-85.3\t-79.8\n-85.7\t-79.7\n-86.1\t-79.6\n-86.5\t-79.5\n-86.9\t-79.4\n-87.3\t-79.3\n-87.7\t-79.2\n-88.1\t-79.1\n-88.5\t-79\n-88.9\t-78.9\n-89.3\t-78.8\n-89.7\t-78.7\n-90.1\t-78.6\n-90.5\t-78.5\n-90.9\t-78.4\n-91.3\t-78.3\n-91.7\t-78.2\n-92.1\t-78.1\n-92.5\t-78\n-92.9\t-77.9\n-93.3\t-77.8\n-93.7\t-77.7\n-94.1\t-77.6\n-94.5\t-77.5\n-94.9\t-77.4\n-95.3\t-77.3\n-95.7\t-77.2\n-96.1\t-77.1\n-96.5\t-77\n-95.8\t-76.9\n-95.1\t-76.8\n-94.4\t-76.7\n-93.7\t-76.6\n-93\t-76.5\n-92.3\t-76.4\n-91.6\t-76.3\n-90.9\t-76.2\n-90.2\t-76.1\n-89.5\t-76\n-88.8\t-75.9\n-88.1\t-75.8\n-87.4\t-75.7\n-86.7\t-75.6\n-86\t-75.5\n-85.3\t-75.4\n-84.6\t-75.3\n-83.9\t-75.2\n-83.2\t-75.1\n-82.5\t-75\n-81.8\t-74.9\n-81.1\t-74.8\n-80.4\t-74.7\n-79.7\t-74.6\n-79\t-74.5\n-78.3\t-74.4\n-77.6\t-74.3\n-76.9\t-74.2\n-76.2\t-74.1\n-75.5\t-74\n-74.8\t-73.9\n-74.1\t-73.8\n-73.4\t-73.7\n-72.7\t-73.6\n-72\t-73.5\n-71.3\t-73.4\n-70.6\t-73.3\n-69.9\t-73.2\n-69.2\t-73.1\n-68.5\t-73\n-67.8\t-72.9\n-67.1\t-72.8\n-66.4\t-72.7\n-65.7\t-72.6\n-65\t-72.5\n-64.3\t-72.4\n-63.6\t-72.3\n-62.9\t-72.2\n-62.2\t-72.1\n-61.5\t-72\n-60.8\t-71.9\n-60.1\t-71.8\n-59.4\t-71.7\n-58.7\t-71.6\n-58\t-71.5\n-57.3\t-71.4\n-56.6\t-71.3\n-55.9\t-71.2\n-55.2\t-71.1\n-54.5\t-71\n-53.8\t-70.9\n-53.1\t-70.8\n-52.4\t-70.7\n-51.7\t-70.6\n-51\t-70.5\n-50.3\t-70.4\n-49.6\t-70.3\n-48.9\t-70.2\n-48.2\t-70.1\n-47.5\t-70\n-46.8\t-69.9\n-46.1\t-69.8\n-45.4\t-69.7\n-44.7\t-69.6\n-44\t-69.5\n-43.3\t-69.4\n-42.6\t-69.3\n-41.9\t-69.2\n-41.2\t-69.1\n-40.5\t-69\n-39.8\t-68.9\n-39.1\t-68.8\n-38.4\t-68.7\n-37.7\t-68.6\n-37\t-68.5\n-36.3\t-68.4\n-35.6\t-68.3\n-34.9\t-68.2\n-34.2\t-68.1\n-33.5\t-68\n-32.8\t-67.9\n-32.1\t-67.8\n-31.4\t-67.7\n-30.7\t-67.6\n-30\t-67.5\n-29.3\t-67.4\n-28.6\t-67.3\n-27.9\t-67.2\n-27.2\t-67.1\n-26.5\t-67\n-25.8\t-66.9\n-25.1\t-66.8\n-24.4\t-66.7\n-23.7\t-66.6\n-23\t-66.5\n-22.3\t-66.4\n-21.6\t-66.3\n-20.9\t-66.2\n-20.2\t-66.1\n-19.5\t-66\n-18.8\t-65.9\n-18.1\t-65.8\n-17.4\t-65.7\n-16.7\t-65.6\n-16\t-65.5\n-15.3\t-65.4\n-14.6\t-65.1\n-13.9\t-64.8\n-13.2\t-64.5\n-12.5\t-64.2\n-11.8\t-63.9\n-11.1\t-63.6\n-10.4\t-63.3\n-9.7\t-63\n-9\t-62.7\n-8.3\t-62.4\n-7.6\t-62.1\n-6.9\t-61.8\n-6.2\t-61.5\n-5.5\t-61.2\n-4.8\t-60.9\n-4.1\t-60.6\n-3.4\t-60.3\n-2.7\t-60\n-2\t-59.7\n-1.3\t-59.4\n-0.6\t-59.1\n0.1\t-58.8\n0.8\t-58.5\n1.5\t-58.2\n2.2\t-57.9\n2.9\t-57.6\n3.6\t-57.3\n4.3\t-57\n5\t-56.7\n5.7\t-56.4\n6.4\t-56.1\n7.1\t-55.8\n7.8\t-55.5\n8.5\t-55.2\n9.2\t-54.9\n9.9\t-54.6\n10.6\t-54.3\n11.3\t-54\n12\t-53.7\n12.7\t-53.4\n13.4\t-53.1\n14.1\t-52.8\n14.8\t-52.5\n15.5\t-52.2\n16.2\t-51.9\n16.9\t-51.6\n17.6\t-51.3\n18.3\t-51\n19\t-50.7\n19.7\t-50.4\n20.4\t-50.1\n21.1\t-49.8\n21.8\t-49.5\n22.5\t-49.2\n23.2\t-48.9\n23.9\t-48.6\n24.6\t-48.3\n25.3\t-48\n26\t-47.7\n26.7\t-47.4\n27.4\t-47.1\n28.1\t-46.8\n28.8\t-46.5\n29.5\t-46.2\n30.2\t-45.9\n30.9\t-45.6\n31.6\t-45.3\n32.3\t-45\n33\t-44.7\n33.7\t-44.4\n34.4\t-44.1\n35.1\t-43.8\n35.8\t-43.5\n36.5\t-43.2\n37.2\t-42.9\n37.9\t-42.6\n38.6\t-42.3\n39.3\t-42\n40\t-41.7\n40.7\t-41.4\n41.4\t-41.1\n42.1\t-40.8\n42.8\t-40.5\n43.5\t-40.2\n44.2\t-39.9\n44.9\t-39.6\n45.6\t-39.3\n46.3\t-39\n47\t-38.7\n47.7\t-38.4\n48.4\t-38.1\n49.1\t-37.8\n49.8\t-37.5\n50.5\t-37.2\n51.2\t-36.9\n51.9\t-36.6\n52.6\t-36.3\n53.3\t-36\n54\t-35.7\n54.7\t-35.4\n55.4\t-35.1\n56.1\t-34.8\n56.8\t-34.5\n57.5\t-34.2\n58.2\t-33.9\n58.9\t-33.6\n59.6\t-33.3\n60.3\t-33\n61\t-32.7\n61.7\t-32.4\n62.4\t-32.1\n63.1\t-31.8\n63.8\t-31.5\n64.5\t-31.2\n65.2\t-30.9\n65.9\t-30.6\n66.6\t-30.3\n67.3\t-30\n68\t-29.7\n68.7\t-29.4\n69.4\t-29.1\n70.1\t-28.8\n70.8\t-28.5\n71.5\t-28.2\n72.2\t-27.9\n72.9\t-27.6\n73.6\t-27.3\n74.3\t-27\n75\t-26.7\n75.7\t-26.4\n76.4\t-26.1\n77.1\t-25.8\n77.8\t-25.5\n77.2\t-25.2\n76.6\t-24.9\n76\t-24.6\n75.4\t-24.3\n74.8\t-24\n74.2\t-23.7\n73.6\t-23.4\n73\t-23.1\n72.4\t-22.8\n71.8\t-22.5\n71.2\t-22.2\n70.6\t-21.9\n70\t-21.6\n69.4\t-21.3\n68.8\t-21\n68.2\t-20.7\n67.6\t-20.4\n67\t-20.1\n66.4\t-19.8\n65.8\t-19.5\n65.2\t-19.2\n64.6\t-18.9\n64\t-18.6\n63.4\t-18.3\n62.8\t-18\n62.2\t-17.7\n61.6\t-17.4\n61\t-17.1\n60.4\t-16.8\n59.8\t-16.5\n59.2\t-16.2\n58.6\t-15.9\n58\t-15.6\n57.4\t-15.3\n56.8\t-15\n56.2\t-14.7\n55.6\t-14.4\n55\t-14.1\n54.4\t-13.8\n53.8\t-13.5\n53.2\t-13.2\n52.6\t-12.9\n52\t-12.6\n51.4\t-12.3\n50.8\t-12\n50.2\t-11.7\n49.6\t-11.4\n49\t-11.1\n48.4\t-10.8\n47.8\t-10.5\n47.2\t-10.2\n46.6\t-9.9\n46\t-9.6\n45.4\t-9.3\n44.8\t-9\n44.2\t-8.7\n43.6\t-8.4\n43\t-8.1\n42.6\t-7.8\n42.2\t-7.5\n41.8\t-7.2\n41.4\t-6.9\n41\t-6.6\n40.6\t-6.3\n40.2\t-6\n39.8\t-5.7\n39.4\t-5.4\n39\t-5.1\n38.6\t-4.8\n38.2\t-4.5\n37.8\t-4.2\n37.4\t-3.9\n37\t-3.6\n36.6\t-3.3\n36.2\t-3\n35.8\t-2.7\n35.4\t-2.4\n35\t-2.1\n34.6\t-1.8\n34.2\t-1.5\n33.8\t-1.2\n33.4\t-0.9\n33\t-0.6\n32.6\t-0.3\n32.2\t-1.83087E-12\n31.8\t0.3\n31.4\t0.6\n31\t0.9\n30.6\t1.2\n30.2\t1.5\n29.8\t1.8\n29.4\t2.1\n29\t2.4\n28.6\t2.7\n28.2\t3\n27.8\t3.3\n27.4\t3.6\n27\t3.9\n26.6\t4.2\n26.2\t4.5\n25.8\t4.8\n25.4\t5.1\n25\t5.4\n24.6\t5.7\n24.2\t6\n23.8\t6.3\n23.4\t6.6\n23\t6.9\n22.6\t7.2\n22.2\t7.5\n21.8\t7.8\n21.4\t8.1\n21\t8.4\n20.6\t8.7\n20.2\t9\n19.8\t9.3\n19.4\t9.6\n19\t9.9\n18.6\t10.2\n18.2\t10.5\n17.8\t10.8\n17.4\t11.1\n17\t11.4\n16.6\t11.7\n16.2\t12\n15.8\t12.3\n15.4\t12.6\n15\t12.9\n14.6\t13.2\n14.2\t13.5\n13.8\t13.8\n13.4\t14.1\n13\t14.4\n12.6\t14.7\n12.2\t15\n11.8\t15.3\n11.4\t15.6\n11\t15.9\n10.6\t16.2\n10.2\t16.5\n9.8\t16.8\n9.4\t17.1\n9\t17.4\n8.6\t17.7\n8.2\t18\n7.8\t18.3\n7.4\t18.6\n7\t18.9\n6.6\t19.2\n6.2\t19.5\n5.8\t19.8\n5.4\t20.1\n5\t20.4\n4.6\t20.7\n4.2\t21\n3.8\t21.3\n3.4\t21.6\n3\t21.9\n2.6\t22.2\n2.2\t22.5\n1.8\t22.8\n1.4\t23.1\n1\t23.4\n0.6\t23.7\n0.2\t24\n-0.2\t24.3\n-0.6\t24.6\n-1\t24.9\n-1.4\t25.2\n-1.8\t25.5\n-2.2\t25.8\n-2.6\t26.1\n-3\t26.4\n-3.4\t26.7\n-3.8\t27\n-4.2\t27.3\n-4.6\t27.6\n-5\t27.9\n-5.4\t28.2\n-5.8\t28.5\n-6.2\t28.8\n-6.6\t29.1\n-7\t29.4\n-7.4\t29.7\n-7.8\t30\n-8.2\t30.3\n-8.6\t30.6\n-9\t30.9\n-9.4\t31.2\n-9.8\t31.5\n-10.2\t31.8\n-10.6\t32.1\n-11\t32.4\n-11.4\t32.7\n-11.8\t33\n-12.2\t33.3\n-12.6\t33.6\n-13\t33.9\n-13.4\t34.2\n-13.8\t34.5\n-14.2\t34.8\n-14.6\t35.1\n-15\t35.4\n-15.4\t35.7\n-15.8\t36\n-16.2\t36.3\n-16.6\t36.6\n-17\t36.9\n-17.4\t37.2\n-17.8\t37.5\n-18.2\t37.8\n-18.6\t38.1\n-19\t38.4\n-19.4\t38.7\n-19.8\t39\n-20.2\t39.3\n-20.6\t39.6\n-21\t39.9\n-21.4\t40.2\n-21.8\t40.5\n-22.2\t40.8\n-22.6\t41.1\n-23\t41.4\n-23.4\t41.7\n-23.8\t42\n-24.2\t42.3\n-24.6\t42.6\n-25\t42.9\n-25.4\t43.2\n-25.8\t43.5\n-26.2\t43.8\n-26.6\t44.1\n-27\t44.4\n-27.4\t44.7\n-27.8\t45\n-28.2\t45.3\n-28.6\t45.6\n-29\t45.9\n-29.4\t46.2\n-29.8\t46.5\n-30.2\t46.8\n-30.6\t47.1\n-31\t47.4\n-31.4\t47.7\n-31.8\t48\n-32.2\t48.3\n-32.6\t48.6\n-33\t48.9\n-33.4\t49.2\n-33.8\t49.5\n-34.2\t49.8\n-34.6\t50.1\n-35\t50.4\n-35.4\t50.7\n-35.8\t51\n-36.2\t51.3\n-36.6\t51.6\n-37\t51.9\n-37.4\t52.2\n-37.8\t52.5\n-38.2\t52.8\n-38.6\t53.1\n-39\t53.4\n-39.4\t53.7\n-39.8\t54\n-40.2\t54.3\n-40.6\t54.6\n-41\t54.9\n-41.4\t55.2\n-41.8\t55.5\n-42.2\t55.8\n-42.6\t56.1\n-43\t56.4\n-43.4\t56.7\n-43.8\t57\n-44.2\t57.3\n-44.6\t57.6\n-45\t57.9\n-45.4\t58.2\n-45.8\t58.5\n-46.2\t58.8\n-46.6\t59.1\n-47\t59.4\n-47.4\t59.7\n-47.8\t60\n-48.2\t60.3\n-48.6\t60.6\n-49\t60.9\n-49.4\t61.2\n-49.8\t61.5\n-50.2\t61.8\n-50.6\t62.1\n-51\t62.4\n-51.4\t62.7\n-51.8\t63\n-52.2\t63.3\n-52.6\t63.6\n-53\t63.9\n-53.4\t64.2\n-53.8\t64.5\n-54.2\t64.8\n-54.6\t65.1\n-55\t65.4\n-55.4\t65.7\n-55.8\t66\n-56.2\t66.3\n-56.6\t66.6\n-57\t66.9\n-57.4\t67.2\n-57.8\t67.5\n-58.2\t67.8\n-58.6\t68.1\n-59\t68.4\n-59.4\t68.7\n-59.8\t69\n-60.2\t69.3\n-60.6\t69.6\n-61\t69.9\n-60.7\t70.2\n-60.4\t70.5\n-60.1\t70.8\n-59.8\t71.1\n-59.5\t71.4\n-59.2\t71.7\n-58.9\t72\n-58.6\t72.3\n-58.3\t72.6\n-58\t72.9\n-57.7\t73.2\n-57.4\t73.5\n-57.1\t73.8\n-56.8\t74.1\n-56.5\t74.4\n-56.2\t74.7\n-55.9\t75\n-55.6\t75.3\n-55.3\t75.6\n-55\t75.9\n-54.7\t76.2\n-54.4\t76.5\n-54.1\t76.8\n-53.8\t77.1\n-53.5\t77.4\n-53.2\t77.7\n-52.9\t78\n-52.6\t78.3\n-52.3\t78.6\n-52\t78.9\n-51.7\t79.2\n-51.4\t79.5\n-51.1\t79.8\n-50.8\t80.1\n-50.5\t80.4\n-50.2\t80.7\n-49.9\t81\n-49.6\t81.3\n-49.3\t81.6\n-49\t81.9\n-48.7\t82.2\n-48.4\t82.5\n-48.1\t82.8\n-47.8\t83.1\n-47.5\t83.4\n-47.2\t83.7\n-46.9\t84\n-46.6\t84.3\n-46.3\t84.6\n-46\t84.9\n-45.7\t85.2\n-45.4\t85.5\n-45.1\t85.8\n-44.8\t86.1\n-44.5\t86.4\n-44.2\t86.7\n-43.9\t87\n-43.6\t87.3\n-43.3\t87.6\n-43\t87.9\n-42.7\t88.2\n-42.4\t88.5\n-42.1\t88.8\n-41.8\t89.1\n-41.5\t89.4\n-41.2\t89.7\n-40.9\t90\n-40.6\t90.3\n-40.3\t90.6\n-40\t90.9\n-39.7\t91.2\n-39.4\t91.5\n-39.1\t91.8\n-38.8\t92.1\n-38.5\t92.4\n-38.2\t92.7\n-37.9\t93\n-37.6\t93.3\n-37.3\t93.6\n-37\t93.9\n-36.7\t93.2\n-36.4\t92.5\n-36.1\t91.8\n-35.8\t91.1\n-35.5\t90.4\n-35.2\t89.7\n-34.9\t89\n-34.6\t88.3\n-34.3\t87.6\n-34\t86.9\n-33.7\t86.2\n-33.4\t85.5\n-33.1\t84.8\n-32.8\t84.1\n-32.5\t83.4\n-32.2\t82.7\n-31.9\t82\n-31.6\t81.3\n-31.3\t80.6\n-31\t79.9\n-30.7\t79.2\n-30.4\t78.5\n-30.1\t77.8\n-29.8\t77.1\n-29.5\t76.4\n-29.2\t75.7\n-28.9\t75\n-28.6\t74.3\n-28.3\t73.6\n-28\t72.9\n-27.7\t72.2\n-27.4\t71.5\n-27.1\t70.8\n-26.8\t70.1\n-26.5\t69.4\n-26.2\t68.7\n-25.9\t68\n-25.6\t67.3\n-25.3\t66.6\n-25\t65.9\n-24.7\t65.2\n-24.4\t64.5\n-24.1\t63.8\n-23.8\t63.1\n-23.5\t62.4\n-23.2\t61.7\n-22.9\t61\n-22.6\t60.3\n-22.3\t59.6\n-22\t58.9\n-21.7\t58.2\n-21.4\t57.5\n-21.1\t56.8\n-20.8\t56.1\n-20.5\t55.4\n-20.2\t54.7\n-19.9\t54\n-19.6\t53.3\n-19.3\t52.6\n-19\t51.9\n-18.7\t51.2\n-18.4\t50.5\n-18.1\t49.8\n-17.8\t49.1\n-17.5\t48.4\n-17.2\t47.7\n-16.9\t47\n-16.6\t46.3\n-16.3\t45.6\n-16\t44.9\n-15.7\t44.2\n-15.4\t43.5\n-15.1\t42.8\n-14.8\t42.1\n-14.5\t41.4\n-14.2\t40.7\n-13.9\t40\n-13.6\t39.3\n-13.3\t38.6\n-13\t37.9\n-12.7\t37.2\n-12.4\t36.5\n-12.1\t35.8\n-11.8\t35.1\n-11.5\t34.4\n-11.2\t33.7\n-10.9\t33\n-10.6\t32.3\n-10.3\t31.6\n-10\t30.9\n-9.7\t30.2\n-9.4\t29.5\n-9.1\t28.8\n-8.8\t28.1\n-8.5\t27.4\n-8.2\t26.7\n-7.9\t26\n-7.6\t25.3\n-7.3\t24.6\n-7\t23.9\n-6.7\t23.2\n-6.4\t22.5\n-6.1\t21.8\n-5.8\t21.1\n-5.5\t20.4\n-5.2\t19.7\n-4.9\t19\n-4.6\t18.3\n-4.3\t17.6\n-4\t16.9\n-3.7\t16.2\n-3.4\t15.5\n-3.1\t14.8\n-2.8\t14.1\n-2.5\t13.4\n-2.2\t12.7\n-1.9\t12\n-1.6\t11.3\n-1.3\t10.6\n-1\t9.9\n-0.7\t9.2\n-0.4\t8.5\n-0.1\t7.8\n0.2\t7.1\n0.5\t6.4\n0.8\t5.7\n1.1\t5\n1.4\t4.3\n1.7\t3.6\n2\t2.9\n2.3\t2.2\n2.6\t1.5\n2.9\t0.8\n3.2\t0.1\n3.5\t-0.6\n3.8\t-1.3\n4.1\t-2\n4.4\t-2.7\n4.7\t-3.4\n5\t-4.1\n5.3\t-4.8\n5.6\t-5.5\n5.9\t-6.2\n6.2\t-6.9\n6.5\t-7.6\n6.8\t-8.3\n7.1\t-9\n7.4\t-9.7\n7.7\t-10.4\n8\t-11.1\n8.3\t-11.8\n8.6\t-12.5\n8.9\t-13.2\n9.2\t-13.9\n9.5\t-14.6\n9.8\t-15.3\n10.1\t-16\n10.4\t-16.7\n10.7\t-17.4\n11\t-18.1\n11.3\t-18.8\n11.6\t-19.5\n11.9\t-20.2\n12.2\t-20.9\n12.5\t-21.6\n12.8\t-22.3\n13.1\t-23\n13.4\t-23.7\n13.7\t-24.4\n14\t-25.1\n14.3\t-25.8\n14.6\t-26.5\n14.9\t-27.2\n15.2\t-27.9\n15.5\t-28.6\n15.8\t-29.3\n16.1\t-30\n16.4\t-30.7\n16.7\t-31.4\n17\t-32.1\n17.3\t-32.8\n17.6\t-33.5\n17.9\t-34.2\n18.2\t-34.9\n18.5\t-35.6\n18.8\t-36.3\n19.1\t-37\n19.4\t-37.7\n19.7\t-38.4\n20\t-39.1\n20.3\t-39.8\n20.6\t-40.5\n20.9\t-41.2\n21.2\t-41.9\n21.5\t-42.6\n21.8\t-43.3\n22.1\t-44\n22.4\t-44.7\n22.7\t-45.4\n23\t-46.1\n23.3\t-46.8\n23.6\t-47.5\n23.9\t-48.2\n24.2\t-48.9\n24.5\t-49.6\n24.8\t-50.3\n25.1\t-51\n25.4\t-51.7\n25.7\t-52.4\n26\t-53.1\n26.3\t-53.8\n26.6\t-54.5\n26.9\t-55.2\n27.2\t-55.9\n27.5\t-56.6\n27.8\t-57.3\n28.1\t-58\n28.4\t-58.7\n28.7\t-59.4\n29\t-60.1\n29.3\t-60.8\n29.6\t-61.5\n29.9\t-62.2\n30.2\t-62.9\n30.5\t-63.6\n30.8\t-64.3\n31.1\t-65\n31.4\t-65.7\n31.7\t-66.4\n32\t-67.1\n32.3\t-67.8\n32.6\t-68.5\n32.9\t-69.2\n33.2\t-69.9\n33.5\t-70.6\n33.8\t-71.3\n34.1\t-72\n34.4\t-72.7\n34.7\t-73.4\n35\t-74.1\n35.3\t-74.8\n35.6\t-75.5\n35.9\t-75\n36.2\t-74.5\n36.5\t-74\n36.8\t-73.5\n37.1\t-73\n37.4\t-72.5\n37.7\t-72\n38\t-71.5\n38.3\t-71\n38.6\t-70.5\n38.9\t-70\n39.2\t-69.5\n39.5\t-69\n39.8\t-68.5\n40.1\t-68\n40.4\t-67.5\n40.7\t-67\n41\t-66.5\n41.3\t-66\n41.6\t-65.5\n41.9\t-65\n42.2\t-64.5\n42.5\t-64\n42.8\t-63.5\n43.1\t-63\n43.4\t-62.5\n43.7\t-62\n44\t-61.5\n44.3\t-61\n44.6\t-60.5\n44.9\t-60\n45.2\t-59.5\n45.5\t-59\n45.8\t-58.5\n46.1\t-58\n46.4\t-57.5\n46.7\t-57\n47\t-56.5\n47.3\t-56\n47.6\t-55.5\n47.9\t-55\n48.2\t-54.5\n48.5\t-54\n48.8\t-53.5\n49.1\t-53\n49.4\t-52.5\n49.7\t-52\n50\t-51.5\n50.3\t-51\n50.6\t-50.5\n50.9\t-50\n51.2\t-49.5\n51.5\t-49\n51.8\t-48.5\n52.1\t-48\n52.4\t-47.5\n52.7\t-47\n53\t-46.5\n53.3\t-46\n53.6\t-45.5\n53.9\t-45\n54.2\t-44.5\n54.5\t-44\n54.8\t-43.5\n55.1\t-43\n55.4\t-42.5\n54.6\t-42\n53.8\t-41.5\n53\t-41\n52.2\t-40.5\n51.4\t-40\n50.6\t-39.5\n49.8\t-39\n49\t-38.5\n48.2\t-38\n47.4\t-37.5\n46.6\t-37\n45.8\t-36.5\n45\t-36\n44.2\t-35.5\n43.4\t-35\n42.6\t-34.5\n41.8\t-34\n41\t-33.5\n40.2\t-33\n39.4\t-32.5\n38.6\t-32\n37.8\t-31.5\n37\t-31\n36.2\t-30.5\n35.4\t-30\n34.6\t-29.5\n33.8\t-29\n33\t-28.5\n32.2\t-28\n31.4\t-27.5\n30.6\t-27\n29.8\t-26.5\n29\t-26\n28.2\t-25.5\n27.4\t-25\n26.6\t-24.5\n25.8\t-24\n25\t-23.5\n24.2\t-23\n23.4\t-22.5\n22.6\t-22\n21.8\t-21.5\n21\t-21\n20.2\t-20.5\n19.4\t-20\n18.6\t-19.5\n17.8\t-19\n17\t-18.5\n16.2\t-18\n15.4\t-17.5\n14.6\t-17\n13.8\t-16.5\n13\t-16\n12.2\t-15.5\n11.4\t-15\n10.6\t-14.5\n9.8\t-14\n9\t-13.5\n8.2\t-13\n7.4\t-12.5\n6.6\t-12\n5.8\t-11.5\n5\t-11\n4.2\t-10.5\n3.4\t-10\n2.6\t-9.5\n1.8\t-9\n1\t-8.5\n0.2\t-8\n-0.6\t-7.5\n-1.4\t-7\n-2.2\t-6.5\n-3\t-6\n-3.8\t-5.5\n-4.6\t-5\n-5.4\t-4.5\n-6.2\t-4\n-7\t-3.5\n-7.8\t-3\n-8.6\t-2.5\n-9.4\t-2\n-10.2\t-1.5\n-11\t-1\n-11.8\t-0.5\n-12.6\t-2.74269E-12\n-13.4\t0.5\n-14.2\t1\n-15\t1.5\n-15.8\t2\n-16.6\t2.5\n-17.4\t3\n-18.2\t3.5\n-19\t4\n-19.8\t4.5\n-20.6\t5\n-21.4\t5.5\n-22.2\t6\n-23\t6.5\n-23.8\t7\n-24.6\t7.5\n-25.4\t8\n-26.2\t8.5\n-27\t9\n-27.8\t9.5\n-28.6\t10\n-29.4\t10.5\n-30.2\t11\n-31\t11.5\n-31.8\t12\n-32.6\t12.5\n-33.4\t13\n-34.2\t13.5\n-35\t14\n-35.8\t14.5\n-36.6\t15\n-37.4\t15.5\n-38.2\t16\n-39\t16.5\n-39.8\t17\n-40.6\t17.5\n-41.4\t18\n-42.2\t18.5\n-43\t19\n-43.8\t19.5\n-44.6\t20\n-45.4\t20.5\n-46.2\t21\n-47\t21.5\n-47.8\t22\n-48.6\t22.5\n-49.4\t23\n-50.2\t23.5\n-51\t24\n-51.8\t24.5\n-52.6\t25\n-53.4\t25.5\n-54.2\t26\n-55\t26.5\n-55.8\t27\n-56.6\t27.5\n-57.4\t28\n-58.2\t28.5\n-59\t29\n-59.8\t29.5\n-60.6\t30\n-61.4\t30.5\n-62.2\t31\n-63\t31.5\n-63.8\t32\n-64.6\t32.5\n-65.4\t33\n-66.2\t33.5\n-67\t34\n-67.8\t34.5\n-68.6\t35\n-69.4\t35.5\n-70.2\t36\n-71\t35.8\n-71.8\t35.6\n-72.6\t35.4\n-73.4\t35.2\n-74.2\t35\n-75\t34.8\n-75.8\t34.6\n-76.6\t34.4\n-77.4\t34.2\n-78.2\t34\n-79\t33.8\n-79.8\t33.6\n-80.6\t33.4\n-81.4\t33.2\n-82.2\t33\n-83\t32.8\n-83.8\t32.6\n-84.6\t32.4\n-85.4\t32.2\n-86.2\t32\n-87\t31.8\n-87.8\t31.6\n-88.6\t31.4\n-89.4\t31.2\n-90.2\t31\n-91\t30.8\n-91.8\t30.6\n-92.6\t30.4\n-93.4\t30.2\n-94.2\t30\n-95\t29.8\n-94.6\t29.6\n-94.2\t29.4\n-93.8\t29.2\n-93.4\t29\n-93\t28.8\n-92.6\t28.6\n-92.2\t28.4\n-91.8\t28.2\n-91.4\t28\n-91\t27.8\n-90.6\t27.6\n-90.2\t27.4\n-89.8\t27.2\n-89.4\t27\n-89\t26.8\n-88.6\t26.6\n-88.2\t26.4\n-87.8\t26.2\n-87.4\t26\n-87\t25.8\n-86.6\t25.6\n-86.2\t25.4\n-85.8\t25.2\n-85.4\t25\n-85\t24.8\n-84.6\t24.6\n-84.2\t24.4\n-83.8\t24.2\n-83.4\t24\n-83\t23.8\n-82.6\t23.6\n-82.2\t23.4\n-81.8\t23.2\n-81.4\t23\n-81\t22.8\n-80.6\t22.6\n-80.2\t22.4\n-79.8\t22.2\n-79.4\t22\n-79\t21.8\n-78.6\t21.6\n-78.2\t21.4\n-77.8\t21.2\n-77.4\t21\n-77\t20.8\n-76.6\t20.6\n-76.2\t20.4\n-75.8\t20.2\n-75.4\t20\n-75\t19.8\n-74.6\t19.6\n-74.2\t19.4\n-73.8\t19.2\n-73.4\t19\n-73\t18.8\n-72.6\t18.6\n-72.2\t18.4\n-71.8\t18.2\n-71.4\t18\n-71\t17.8\n-70.6\t17.6\n-70.2\t17.4\n-69.8\t17.2\n-69.4\t17\n-69\t16.8\n-68.6\t16.6\n-68.2\t16.4\n-67.8\t16.2\n-67.4\t16\n-67\t15.8\n-66.6\t15.6\n-66.2\t15.4\n-65.8\t15.2\n-65.4\t15\n-65\t14.8\n-64.6\t14.6\n-64.2\t14.4\n-63.8\t14.2\n-63.4\t14\n-63\t13.8\n-62.6\t13.6\n-62.2\t13.4\n-61.8\t13.2\n-61.4\t13\n-61\t12.8\n-60.6\t12.6\n-60.2\t12.4\n-59.8\t12.2\n-59.4\t12\n-59\t11.8\n-58.6\t11.6\n-58.2\t11.4\n-57.8\t11.2\n-57.4\t11\n-57\t10.8\n-56.6\t10.6\n-56.2\t10.4\n-55.8\t10.2\n-55.4\t10\n-55\t9.8\n-54.6\t9.6\n-54.2\t9.4\n-53.8\t9.2\n-53.4\t9\n-53\t8.8\n-52.6\t8.6\n-52.2\t8.4\n-51.8\t8.2\n-51.4\t8\n-51\t7.8\n-50.6\t7.6\n-50.2\t7.4\n-49.8\t7.2\n-49.4\t7\n-49\t6.8\n-48.6\t6.6\n-48.2\t6.4\n-47.8\t6.2\n-47.4\t6\n-47\t5.8\n-46.6\t5.6\n-46.2\t5.4\n-45.8\t5.2\n-45.4\t5\n-45\t4.8\n-44.6\t4.6\n-44.2\t4.4\n-43.8\t4.2\n-43.4\t4\n-43\t3.8\n-42.6\t3.6\n-42.2\t3.4\n-41.8\t3.2\n-41.4\t3\n-41\t2.8\n-40.6\t2.6\n-40.2\t2.4\n-39.8\t2.2\n-39.4\t2\n-39\t1.8\n-38.6\t1.6\n-38.2\t1.4\n-37.8\t1.2\n-37.4\t1\n-37\t0.8\n-36.6\t0.6\n-36.2\t0.4\n-35.8\t0.2\n-35.4\t-2.71644E-12\n-35\t-0.2\n-34.6\t-0.4\n-34.2\t-0.6\n-33.8\t-0.8\n-33.4\t-1\n-33\t-1.2\n-32.6\t-1.4\n-32.2\t-1.6\n-31.8\t-1.8\n-31.4\t-2\n-31\t-2.2\n-30.6\t-2.4\n-30.2\t-2.6\n-29.8\t-2.8\n-29.4\t-3\n-29\t-3.2\n-28.6\t-3.4\n-28.2\t-3.6\n-27.8\t-3.8\n-27.4\t-4\n-27\t-4.2\n-26.6\t-4.4\n-26.2\t-4.6\n-25.8\t-4.8\n-25.4\t-5\n-25\t-5.2\n-24.6\t-5.4\n-24.2\t-5.6\n-23.8\t-5.8\n-23.4\t-6\n-23\t-6.2\n-22.6\t-6.4\n-22.2\t-6.6\n-21.8\t-6.8\n-21.4\t-7\n-21\t-7.2\n-20.6\t-7.4\n-20.2\t-7.6\n-19.8\t-7.8\n-19.4\t-8\n-19\t-8.2\n-18.6\t-8.4\n-18.2\t-8.6\n-17.8\t-8.8\n-17.4\t-9\n-17\t-9.2\n-16.6\t-9.4\n-16.2\t-9.6\n-15.8\t-9.8\n-15.4\t-10\n-15\t-10.2\n-14.6\t-10.4\n-14.2\t-10.6\n-13.8\t-10.8\n-13.4\t-11\n-13\t-11.2\n-12.6\t-11.4\n-12.2\t-11.6\n-11.8\t-11.8\n-11.4\t-12\n-11\t-12.2\n-10.6\t-12.4\n-10.2\t-12.6\n-9.8\t-12.8\n-9.4\t-13\n-9\t-13.2\n-8.6\t-13.4\n-8.2\t-13.6\n-7.8\t-13.8\n-7.4\t-14\n-7\t-14.2\n-6.6\t-14.4\n-6.2\t-14.6\n-5.8\t-14.8\n-5.4\t-15\n-5\t-15.2\n-4.6\t-15.4\n-4.2\t-15.6\n-3.8\t-15.8\n-3.4\t-16\n-3\t-16.2\n-2.6\t-16.4\n-2.2\t-16.6\n-1.8\t-16.8\n-1.4\t-17\n-1\t-17.2\n-0.6\t-17.4\n-0.2\t-17.6\n0.2\t-17.8\n0.6\t-18\n1\t-18.2\n1.4\t-18.4\n1.8\t-18.6\n2.2\t-18.8\n2.6\t-19\n3\t-19.2\n3.4\t-19.4\n3.8\t-19.6\n4.2\t-19.8\n4.6\t-20\n5\t-20.2\n5.4\t-20.4\n5.8\t-20.6\n6.2\t-20.8\n6.6\t-21\n7\t-21.2\n7.4\t-21.4\n7.8\t-21.6\n8.2\t-21.8\n8.6\t-22\n9\t-22.2\n9.4\t-22.4\n9.8\t-22.6\n10.2\t-22.8\n10.6\t-23\n11\t-23.2\n11.4\t-23.4\n11.8\t-23.6\n12.2\t-23.8\n12.6\t-24\n13\t-24.2\n13.4\t-24.4\n13.8\t-24.6\n14.2\t-24.8\n14.6\t-25\n15\t-25.2\n15.4\t-25.4\n15.8\t-25.6\n16.2\t-25.8\n16.6\t-26\n17\t-26.2\n17.4\t-26.4\n17.8\t-26.6\n18.2\t-26.8\n18.6\t-27\n19\t-27.2\n19.4\t-27.4\n19.8\t-27.6\n20.2\t-27.8\n20.6\t-28\n21\t-28.2\n21.4\t-28.4\n21.8\t-28.6\n22.2\t-28.8\n22.6\t-29\n23\t-29.2\n23.4\t-29.4\n23.8\t-29.6\n24.2\t-29.8\n24.6\t-30\n25\t-30.2\n25.4\t-30.4\n25.8\t-30.6\n26.2\t-30.8\n26.6\t-31\n27\t-31.2\n27.4\t-31.4\n27.8\t-31.6\n28.2\t-31.8\n28.6\t-32\n29\t-32.2\n29.4\t-32.4\n29.8\t-32.6\n30.2\t-32.8\n30.6\t-33\n31\t-33.2\n31.4\t-33.4\n31.8\t-33.6\n32.2\t-33.8\n32.6\t-34\n33\t-34.2\n33.4\t-34.4\n33.8\t-34.6\n34.2\t-34.8\n34.6\t-35\n35\t-35.2\n35.4\t-35.4\n35.8\t-35.6\n36.6\t-35.8\n37.4\t-36\n38.2\t-36.2\n39\t-36.4\n39.8\t-36.6\n40.6\t-36.8\n41.4\t-37\n42.2\t-37.2\n43\t-37.4\n43.8\t-37.6\n44.6\t-37.8\n45.4\t-38\n46.2\t-38.2\n47\t-38.4\n47.8\t-38.6\n48.6\t-38.8\n49.4\t-39\n50.2\t-39.2\n51\t-39.4\n51.8\t-39.6\n52.6\t-39.8\n53.4\t-40\n54.2\t-40.2\n55\t-40.4\n55.8\t-40.6\n56.6\t-40.8\n57.4\t-41\n58.2\t-41.2\n59\t-41.4\n59.8\t-41.6\n60.6\t-41.8\n61.4\t-42\n62.2\t-42.2\n63\t-42.4\n63.8\t-42.6\n64.6\t-42.8\n65.4\t-43\n66.2\t-43.2\n67\t-43.4\n67.8\t-43.6\n68.6\t-43.8\n69.4\t-44\n70.2\t-44.2\n71\t-44.4\n71.8\t-44.6\n72.6\t-44.8\n73.4\t-45\n74.2\t-45.2\n75\t-45.4\n75.8\t-45.6\n76.6\t-45.8\n77.4\t-46\n78.2\t-46.2\n79\t-46.4\n79.8\t-46.6\n80.6\t-46.8\n81.4\t-47\n82.2\t-47.2\n83\t-47.4\n83.8\t-47.6\n84.6\t-47.8\n85.4\t-48\n86.2\t-48.2\n87\t-48.4\n87.8\t-48.6\n88.6\t-48.8\n89.4\t-49\n90.2\t-49.2\n91\t-49.4\n91.8\t-49.6\n92.6\t-49.8\n93.4\t-50\n94.2\t-50.2\n95\t-50.4\n95.8\t-50.6\n96.6\t-50.8\n97.4\t-51\n98.2\t-51.2\n97.6\t-51.4\n97\t-51.6\n96.4\t-51.8\n95.8\t-52\n95.2\t-52.2\n94.6\t-52.4\n94\t-52.6\n93.4\t-52.8\n92.8\t-53\n92.2\t-53.2\n91.6\t-53.4\n91\t-53.6\n90.4\t-53.8\n89.8\t-54\n89.2\t-54.2\n88.6\t-54.4\n88\t-54.6\n87.4\t-54.8\n86.8\t-55\n86.2\t-55.2\n85.6\t-55.4\n85\t-55.6\n84.4\t-55.8\n83.8\t-56\n83.2\t-56.2\n82.6\t-56.4\n82\t-56.6\n81.4\t-56.8\n80.8\t-57\n80.2\t-57.2\n79.6\t-57.4\n79\t-57.6\n78.4\t-57.8\n77.8\t-58\n77.2\t-58.2\n76.6\t-58.4\n76\t-58.6\n75.4\t-58.8\n74.8\t-59\n74.2\t-59.2\n73.6\t-59.4\n73\t-59.6\n72.4\t-59.8\n71.8\t-60\n71.2\t-60.2\n70.6\t-60.4\n70\t-60.6\n69.4\t-60.8\n68.8\t-61\n68.2\t-61.2\n67.6\t-61.4\n67\t-61.6\n66.4\t-61.8\n65.8\t-62\n65.2\t-62.2\n64.6\t-62.4\n64\t-62.6\n63.4\t-62.8\n62.8\t-63\n62.2\t-63.2\n61.6\t-63.4\n61\t-63.6\n60.4\t-63.8\n59.8\t-64\n59.2\t-64.2\n58.6\t-64.4\n58\t-64.6\n57.4\t-64.8\n56.8\t-65\n56.2\t-65.2\n55.6\t-65.4\n55\t-65.6\n54.4\t-65.8\n53.8\t-66\n53.2\t-66.2\n52.6\t-66.4\n52\t-66.6\n51.4\t-66.8\n50.8\t-67\n50.2\t-67.2\n49.6\t-67.4\n49\t-67.6\n48.4\t-67.8\n47.8\t-68\n47.2\t-68.2\n46.6\t-68.4\n46\t-68.6\n45.4\t-68.8\n44.8\t-69\n44.2\t-69.2\n43.6\t-69.4\n43\t-69.6\n42.4\t-69.8\n41.8\t-70\n41.2\t-70.2\n40.6\t-70.4\n40\t-70.6\n39.4\t-70.8\n38.8\t-71\n38.2\t-71.2\n37.6\t-71.4\n37\t-71.6\n36.4\t-71.8\n35.8\t-72\n35.2\t-72.2\n34.6\t-72.4\n34\t-72.6\n33.4\t-72.8\n32.8\t-73\n32.2\t-73.2\n31.6\t-73.4\n31\t-73.6\n30.4\t-73.8\n29.8\t-74\n29.2\t-74.2\n28.6\t-74.4\n28\t-74.6\n27.4\t-74.8\n26.8\t-75\n26.2\t-75.2\n25.6\t-75.4\n25\t-75.6\n24.4\t-75.8\n23.8\t-76\n23.2\t-76.2\n22.6\t-76.4\n22\t-76.6\n21.4\t-76.8\n20.8\t-77\n20.2\t-77.2\n19.6\t-77.4\n19\t-77.6\n18.4\t-77.8\n17.8\t-78\n17.2\t-78.2\n16.6\t-78.4\n16\t-78.6\n15.4\t-78.8\n14.8\t-79\n14.2\t-79.2\n13.6\t-79.4\n13\t-79.6\n12.4\t-79.8\n11.8\t-80\n11.2\t-80.2\n10.6\t-80.4\n10\t-80.6\n9.4\t-80.8\n8.8\t-81\n8.2\t-81.2\n7.6\t-81.4\n7\t-81.6\n6.4\t-81.8\n5.8\t-82\n5.2\t-82.2\n4.6\t-82.4\n4\t-82.6\n3.4\t-82.8\n2.8\t-83\n2.2\t-83.2\n1.6\t-83.4\n1\t-83.6\n0.4\t-83.8\n-0.2\t-84\n-0.8\t-84.2\n-1.4\t-84.4\n-2\t-84.6\n-2.6\t-84.8\n-3.2\t-85\n-3.8\t-85.2\n-4.4\t-85.4\n-5\t-85.6\n-5.6\t-85.8\n-6.2\t-86\n-6.8\t-86.2\n-7.4\t-86.4\n-8\t-86.6\n-8.6\t-86.8\n-9.2\t-87\n-9.8\t-87.2\n-10.4\t-87.4\n-11\t-87.6\n-11.6\t-87.8\n-12.2\t-88\n-12.8\t-88.2\n-13.4\t-88.4\n-14\t-88.6\n-14.6\t-88.8\n-15.2\t-89\n-15.8\t-89.2\n-16.4\t-89.4\n-17\t-89.6\n-17.6\t-89.8\n-18.2\t-90\n-18.8\t-90.2\n-19.4\t-90.4\n-20\t-90.6\n-20.6\t-90.8\n-21.2\t-91\n-21.8\t-91.2\n-22.4\t-91.4\n-23\t-91.6\n-23.6\t-91.8\n-24.2\t-92\n-24.8\t-92.2\n-25.4\t-92.4\n-26\t-92.6\n-26.6\t-92.8\n-27.2\t-93\n-27.8\t-93.2\n-28.4\t-93.4\n-29\t-93.6\n-29.6\t-93.8\n-30.2\t-94\n-30.8\t-93.6\n-31.4\t-93.2\n-32\t-92.8\n-32.6\t-92.4\n-33.2\t-92\n-33.8\t-91.6\n-34.4\t-91.2\n-35\t-90.8\n-35.6\t-90.4\n-36.2\t-90\n-36.8\t-89.6\n-37.4\t-89.2\n-38\t-88.8\n-38.6\t-88.4\n-39.2\t-88\n-39.8\t-87.6\n-40.4\t-87.2\n-41\t-86.8\n-41.6\t-86.4\n-42.2\t-86\n-42.8\t-85.6\n-43.4\t-85.2\n-44\t-84.8\n-44.6\t-84.4\n-45.2\t-84\n-45.8\t-83.6\n-46.4\t-83.2\n-47\t-82.8\n-47.6\t-82.4\n-48.2\t-82\n-48.8\t-81.6\n-49.4\t-81.2\n-50\t-80.8\n-50.6\t-80.4\n-51.2\t-80\n-51.8\t-79.6\n-52.4\t-79.2\n-53\t-78.8\n-53.6\t-78.4\n-54.2\t-78\n-54.8\t-77.6\n-55.4\t-77.2\n-56\t-76.8\n-56.6\t-76.4\n-57.2\t-76\n-57.8\t-75.6\n-58.4\t-75.2\n-59\t-74.8\n-59.6\t-74.4\n-60.2\t-74\n-60.8\t-73.6\n-61.4\t-73.2\n-62\t-72.8\n-62.6\t-72.4\n-63.2\t-72\n-63.8\t-71.6\n-64.4\t-71.2\n-65\t-70.8\n-65.6\t-70.4\n-66.2\t-70\n-66.8\t-69.6\n-67.4\t-69.2\n-68\t-68.8\n-68.6\t-68.4\n-69.2\t-68\n-69.8\t-67.6\n-70.4\t-67.2\n-71\t-66.8\n-71.6\t-66.4\n-72.2\t-66\n-72.8\t-65.6\n-73.4\t-65.2\n-74\t-64.8\n-74.6\t-64.4\n-75.2\t-64\n-75.8\t-63.6\n-76.4\t-63.2\n-77\t-62.8\n-77.6\t-62.4\n-78.2\t-62\n-78.8\t-61.6\n-79.4\t-61.2\n-80\t-60.8\n-80.6\t-60.4\n-81.2\t-60\n-81.8\t-59.6\n-82.4\t-59.2\n-83\t-58.8\n-83.6\t-58.4\n-84.2\t-58\n-84.8\t-57.6\n-85.4\t-57.2\n-86\t-56.8\n-86.6\t-56.4\n-87.2\t-56\n-87.8\t-55.6\n-88.4\t-55.2\n-89\t-54.8\n-89.6\t-54.4\n-89.4\t-54\n-89.2\t-53.6\n-89\t-53.2\n-88.8\t-52.8\n-88.6\t-52.4\n-88.4\t-52\n-88.2\t-51.6\n-88\t-51.2\n-87.8\t-50.8\n-87.6\t-50.4\n-87.4\t-50\n-87.2\t-49.6\n-87\t-49.2\n-86.8\t-48.8\n-86.6\t-48.4\n-86.4\t-48\n-86.2\t-47.6\n-86\t-47.2\n-85.8\t-46.8\n-85.6\t-46.4\n-85.4\t-46\n-85.2\t-45.6\n-85\t-45.2\n-84.8\t-44.8\n-84.6\t-44.4\n-84.4\t-44\n-84.2\t-43.6\n-84\t-43.2\n-83.8\t-42.8\n-83.6\t-42.4\n-83.4\t-42\n-83.2\t-41.6\n-83\t-41.2\n-82.8\t-40.8\n-82.6\t-40.4\n-82.4\t-40\n-82.2\t-39.6\n-82\t-39.2\n-81.8\t-38.8\n-81.6\t-38.4\n-81.4\t-38\n-81.2\t-37.6\n-81\t-37.2\n-80.8\t-36.8\n-80.6\t-36.4\n-80.4\t-36\n-80.2\t-35.6\n-80\t-35.2\n-79.8\t-34.8\n-79.6\t-34.4\n-79.4\t-34\n-79.2\t-33.6\n-79\t-33.2\n-78.8\t-32.8\n-78.6\t-32.4\n-78.4\t-32\n-78.2\t-31.6\n-78\t-31.2\n-77.8\t-30.8\n-77.6\t-30.4\n-77.4\t-30\n-77.2\t-29.6\n-77\t-29.2\n-76.8\t-28.8\n-76.6\t-28.4\n-76.4\t-28\n-76.2\t-27.6\n-76\t-27.2\n-75.8\t-26.8\n-75.6\t-26.4\n-75.4\t-26\n-75.2\t-25.6\n-75\t-25.2\n-74.8\t-24.8\n-74.6\t-24.4\n-74.4\t-24\n-74.2\t-23.6\n-74\t-23.2\n-73.8\t-22.8\n-73.6\t-22.4\n-73.4\t-22\n-73.2\t-21.6\n-73\t-21.2\n-72.8\t-20.8\n-72.6\t-20.4\n-72.4\t-20\n-72.2\t-19.6\n-72\t-19.2\n-71.8\t-18.8\n-71.6\t-18.4\n-71.4\t-18\n-71.2\t-17.6\n-71\t-17.2\n-70.8\t-16.8\n-70.6\t-16.4\n-70.4\t-16\n-70.2\t-15.6\n-70\t-15.2\n-69.8\t-14.8\n-69.6\t-14.4\n-69.4\t-14\n-69.2\t-13.6\n-69\t-13.2\n-68.8\t-12.8\n-68.6\t-12.4\n-68.4\t-12\n-68.2\t-11.6\n-68\t-11.2\n-67.8\t-10.8\n-67.6\t-10.4\n-67.4\t-10\n-67.2\t-9.6\n-67\t-9.2\n-66.8\t-8.8\n-66.6\t-8.4\n-66.4\t-8\n-66.2\t-7.6\n-66\t-7.2\n-65.8\t-6.8\n-65.6\t-6.4\n-65.4\t-6\n-65.2\t-5.6\n-65\t-5.2\n-64.8\t-4.8\n-64.6\t-4.4\n-64.4\t-4\n-64.2\t-3.6\n-64\t-3.2\n-63.8\t-2.8\n-63.6\t-2.4\n-63.4\t-2\n-63.2\t-1.6\n-63\t-1.2\n-62.8\t-0.8\n-62.6\t-0.4\n-62.4\t0\n-62.2\t0\n-62\t0.3\n-61.8\t0.6\n-61.6\t0.9\n-61.4\t1.2\n-61.2\t1.5\n-61\t1.8\n-60.8\t2.1\n-60.6\t2.4\n-60.4\t2.7\n-60.2\t3\n-60\t3.3\n-59.8\t3.6\n-59.6\t3.9\n-59.4\t4.2\n-59.2\t4.5\n-59\t4.8\n-58.8\t5.1\n-58.6\t5.4\n-58.4\t5.7\n-58.2\t6\n-58\t6.3\n-57.8\t6.6\n-57.6\t6.9\n-57.4\t7.2\n-57.2\t7.5\n-57\t7.8\n-56.8\t8.1\n-56.6\t8.4\n-56.4\t8.7\n-56.2\t9\n-56\t9.3\n-55.8\t9.6\n-55.6\t9.9\n-55.4\t10.2\n-55.2\t10.5\n-55\t10.8\n-54.8\t11.1\n-54.6\t11.4\n-54.4\t11.7\n-54.2\t12\n-54\t12.3\n-53.8\t12.6\n-53.6\t12.9\n-53.4\t13.2\n-53.2\t13.5\n-53\t13.8\n-52.8\t14.1\n-52.6\t14.4\n-52.4\t14.7\n-52.2\t15\n-52\t15.3\n-51.8\t15.6\n-51.6\t15.9\n-51.4\t16.2\n-51.2\t16.5\n-51\t16.8\n-50.8\t17.1\n-50.6\t17.4\n-50.4\t17.7\n-50.2\t18\n-50\t18.3\n-49.8\t18.6\n-49.6\t18.9\n-49.4\t19.2\n-49.2\t19.5\n-49\t19.8\n-48.8\t20.1\n-48.6\t20.4\n-48.4\t20.7\n-48.2\t21\n-48\t21.3\n-47.8\t21.6\n-47.6\t21.9\n-47.4\t22.2\n-47.2\t22.5\n-47\t22.8\n-46.8\t23.1\n-46.6\t23.4\n-46.4\t23.7\n-46.2\t24\n-46\t24.3\n-45.8\t24.6\n-45.6\t24.9\n-45.4\t25.2\n-45.2\t25.5\n-45\t25.8\n-44.8\t26.1\n-44.6\t26.4\n-44.4\t26.7\n-44.2\t27\n-44\t27.3\n-43.8\t27.6\n-43.6\t27.9\n-43.4\t28.2\n-43.2\t28.5\n-43\t28.8\n-42.8\t29.1\n-42.6\t29.4\n-42.4\t29.7\n-42.2\t30\n-42\t30.3\n-41.8\t30.6\n-41.6\t30.9\n-41.4\t31.2\n-41.2\t31.5\n-41\t31.8\n-40.8\t32.1\n-40.6\t32.4\n-40.4\t32.7\n-40.2\t33\n-40\t33.3\n-39.8\t33.6\n-39.6\t33.9\n-39.4\t34.2\n-39.2\t34.5\n-39\t34.8\n-38.8\t35.1\n-38.6\t35.4\n-38.4\t35.7\n-38.2\t36\n-38\t36.3\n-37.8\t36.6\n-37.6\t36.9\n-37.4\t37.2\n-37.2\t37.5\n-37\t37.8\n-36.8\t38.1\n-36.6\t38.4\n-36.4\t38.7\n-36.2\t39\n-36\t39.3\n-35.8\t39.6\n-35.6\t39.9\n-35.4\t40.2\n-35.2\t40.5\n-35\t40.8\n-34.8\t41.1\n-34.6\t41.4\n-34.4\t41.7\n-34.2\t42\n-34\t42.3\n-33.8\t42.6\n-33.6\t42.9\n-33.4\t43.2\n-33.2\t43.5\n-33\t43.8\n-32.8\t44.1\n-32.6\t44.4\n-32.4\t44.7\n-32.2\t45\n-32\t45.3\n-31.8\t45.6\n-31.6\t45.9\n-31.4\t46.2\n-31.2\t46.5\n-31\t46.8\n-30.8\t47.1\n-30.6\t47.4\n-30.4\t47.7\n-30.2\t48\n-30\t48.3\n-29.8\t48.6\n-29.6\t48.9\n-29.4\t49.2\n-29.2\t49.5\n-29\t49.8\n-28.8\t50.1\n-28.6\t50.4\n-28.4\t50.7\n-28.2\t51\n-28\t51.3\n-27.8\t51.6\n-27.6\t51.9\n-27.4\t52.2\n-27.2\t52.5\n-27\t52.8\n-26.8\t53.1\n-26.6\t53.4\n-26.4\t53.7\n-26.2\t54\n-26\t54.3\n-25.8\t54.6\n-25.6\t54.9\n-25.4\t55.2\n-25.2\t55.5\n-25\t55.8\n-24.8\t56.1\n-24.6\t56.4\n-24.4\t56.7\n-24.2\t57\n-24\t57.3\n-23.8\t57.6\n-23.6\t57.9\n-23.4\t58.2\n-23.2\t58.5\n-23\t58.8\n-22.8\t59.1\n-22.6\t59.4\n-22.4\t59.7\n-22.2\t60\n-22\t60.3\n-21.8\t60.6\n-21.6\t60.9\n-21.4\t61.2\n-21.2\t61.5\n-21\t61.8\n-20.8\t62.1\n-20.6\t62.4\n-20.4\t62.7\n-20.2\t63\n-20\t63.3\n-19.8\t63.6\n-19.6\t63.9\n-19.4\t64.2\n-19.2\t64.5\n-19\t64.8\n-18.8\t65.1\n-18.6\t65.4\n-18.4\t65.7\n-18.2\t66\n-18\t66.3\n-17.8\t66.6\n-17.6\t66.9\n-17.4\t67.2\n-17.2\t67.5\n-17\t67.8\n-16.8\t68.1\n-16.6\t68.4\n-16.4\t68.7\n-16.2\t69\n-16\t69.3\n-15.8\t69.6\n-15.6\t69.9\n-15.4\t70.2\n-15.2\t70.5\n-15\t70.8\n-14.8\t71.1\n-14.6\t71.4\n-14.4\t71.7\n-14.2\t72\n-14\t72.3\n-13.8\t72.6\n-13.6\t72.9\n-13.4\t73.2\n-13.2\t73.5\n-13\t73.8\n-12.8\t74.1\n-12.6\t74.4\n-12.4\t74.7\n-12.2\t75\n-12\t75.3\n-11.8\t75.6\n-11.6\t75.9\n-11.4\t76.2\n-11.2\t76.5\n-11\t76.8\n-10.8\t77.1\n-10.6\t77.4\n-10.4\t77.7\n-10.2\t78\n-10\t78.3\n-9.8\t78.6\n-9.6\t78.9\n-9.4\t79.2\n-9.2\t79.5\n-9\t79.8\n-8.8\t80.1\n-8.6\t80.4\n-8.4\t80.7\n-8.2\t81\n-8\t81.3\n-7.8\t81.6\n-7.6\t81.9\n-7.4\t82.2\n-7.2\t82.5\n-7\t82.8\n-6.8\t83.1\n-6.6\t83.4\n-6.4\t83.7\n-6.2\t84\n-6\t84.3\n-5.8\t84.6\n-5.6\t84.9\n-5.4\t85.2\n-5.2\t85.5\n-5\t85.8\n-4.8\t86.1\n-4.6\t86.4\n-4.4\t86.7\n-4.2\t87\n-4\t87.3\n-3.8\t87.6\n-3.6\t87.9\n-3.4\t88.2\n-3.2\t88.5\n-3\t88.8\n-2.8\t89.1\n-2.6\t89.4\n-2.4\t89.7\n-2.2\t90\n-2\t90.3\n-1.8\t90.6\n-1.6\t90.9\n-1.4\t91.2\n-1.2\t91.5\n-1\t91.8\n-0.8\t92.1\n-0.6\t92.4\n-0.4\t92.7\n-0.2\t93\n-2.43922E-12\t93.3\n0.2\t93.6\n0.4\t93.9\n0.6\t94.2\n0.8\t94.5\n1\t94.8\n1.2\t95.1\n1.4\t95.4\n1.6\t95.7\n1.8\t96\n2\t96.3\n2.2\t96.6\n2.4\t96.9\n2.6\t97.2\n2.8\t97.5\n3\t97.3\n3.2\t97.1\n3.4\t96.9\n3.6\t96.7\n3.8\t96.5\n4\t96.3\n4.2\t96.1\n4.4\t95.9\n4.6\t95.7\n4.8\t95.5\n5\t95.3\n5.2\t95.1\n5.4\t94.9\n5.6\t94.7\n5.8\t94.5\n6\t94.3\n6.2\t94.1\n6.4\t93.9\n6.6\t93.7\n6.8\t93.5\n7\t93.3\n7.2\t93.1\n7.4\t92.9\n7.6\t92.7\n7.8\t92.5\n8\t92.3\n8.2\t92.1\n8.4\t91.9\n8.6\t91.7\n8.8\t91.5\n9\t91.3\n9.2\t91.1\n9.4\t90.9\n9.6\t90.7\n9.8\t90.5\n10\t90.3\n10.2\t90.1\n10.4\t89.9\n10.6\t89.7\n10.8\t89.5\n11\t89.3\n11.2\t89.1\n11.4\t88.9\n11.6\t88.7\n11.8\t88.5\n12\t88.3\n12.2\t88.1\n12.4\t87.9\n12.6\t87.7\n12.8\t87.5\n13\t87.3\n13.2\t87.1\n13.4\t86.9\n13.6\t86.7\n13.8\t86.5\n14\t86.3\n14.2\t86.1\n14.4\t85.9\n14.6\t85.7\n14.8\t85.5\n15\t85.3\n15.2\t85.1\n15.4\t84.9\n15.6\t84.7\n15.8\t84.5\n16\t84.3\n16.2\t84.1\n16.4\t83.9\n16.6\t83.7\n16.8\t83.5\n17\t83.3\n17.2\t83.1\n17.4\t82.9\n17.6\t82.7\n17.8\t82.5\n18\t82.3\n18.2\t82.1\n18.4\t81.9\n18.6\t81.7\n18.8\t81.5\n19\t81.3\n19.2\t81.1\n19.4\t80.9\n19.6\t80.7\n19.8\t80.5\n20\t80.3\n20.2\t80.1\n20.4\t79.9\n20.6\t79.7\n20.8\t79.5\n21\t79.3\n21.2\t79.1\n21.4\t78.9\n21.6\t78.7\n21.8\t78.5\n22\t78.3\n22.2\t78.1\n22.4\t77.9\n22.6\t77.7\n22.8\t77.5\n23\t77.3\n23.2\t77.1\n23.4\t76.9\n23.6\t76.7\n23.8\t76.5\n24\t76.3\n24.2\t76.1\n24.4\t75.9\n24.6\t75.7\n24.8\t75.5\n25\t75.3\n25.2\t75.1\n25.4\t74.9\n25.6\t74.7\n25.8\t74.5\n26\t74.3\n26.2\t74.1\n26.4\t73.9\n26.6\t73.7\n26.8\t73.5\n27\t73.3\n27.2\t73.1\n27.4\t72.9\n27.6\t72.7\n27.8\t72.5\n28\t72.3\n28.2\t72.1\n28.4\t71.9\n28.6\t71.7\n28.8\t71.5\n29\t71.3\n29.2\t71.1\n29.4\t70.9\n29.6\t70.7\n29.8\t70.5\n30\t70.3\n30.2\t70.1\n30.4\t69.9\n30.6\t69.7\n30.8\t69.5\n31\t69.3\n31.2\t69.1\n31.4\t68.9\n31.6\t68.7\n31.8\t68.5\n32\t68.3\n32.2\t68.1\n32.4\t67.9\n32.6\t67.7\n32.8\t67.5\n33\t67.3\n33.2\t67.1\n33.4\t66.9\n33.6\t66.7\n33.8\t66.5\n34\t66.3\n34.2\t66.1\n34.4\t65.9\n34.6\t65.7\n34.8\t65.5\n35\t65.3\n35.2\t65.1\n35.4\t64.9\n35.6\t64.7\n35.8\t64.5\n36\t64.3\n36.2\t64.1\n36.4\t63.9\n36.6\t63.7\n36.8\t63.5\n37\t63.3\n37.2\t63.1\n37.4\t62.9\n37.6\t62.7\n37.8\t62.5\n38\t62.3\n38.2\t62.1\n38.4\t61.9\n38.6\t61.7\n38.8\t61.5\n39\t61.3\n39.2\t61.1\n39.4\t60.9\n39.6\t60.7\n39.8\t60.5\n40\t60.3\n40.2\t60.1\n40.4\t59.9\n40.6\t59.7\n40.8\t59.5\n41\t59.3\n41.2\t59.1\n41.4\t58.9\n41.6\t58.7\n41.8\t58.5\n42\t58.3\n42.2\t58.1\n42.4\t57.9\n42.6\t57.7\n42.8\t57.5\n43\t57.3\n43.2\t57.1\n43.4\t56.9\n43.6\t56.7\n43.8\t56.5\n44\t56.3\n44.2\t56.1\n44.4\t55.9\n44.6\t55.7\n44.8\t55.5\n45\t55.3\n45.2\t55.1\n45.4\t54.9\n45.6\t54.7\n45.8\t54.5\n46\t54.3\n46.2\t54.1\n46.4\t53.9\n46.6\t53.7\n46.8\t53.5\n47\t53.3\n47.2\t53.1\n47.4\t52.9\n47.6\t52.7\n47.8\t52.5\n48\t52.3\n48.2\t52.1\n48.4\t51.9\n48.6\t51.7\n48.8\t51.5\n49\t51.3\n49.2\t51.1\n49.4\t50.9\n49.6\t50.7\n49.8\t50.5\n50\t50.3\n50.2\t50.1\n50.4\t49.9\n50.6\t49.7\n50.8\t49.5\n51\t49.3\n51.2\t49.1\n51.4\t48.9\n51.6\t48.7\n51.8\t48.5\n52\t48.3\n52.2\t48.1\n52.4\t47.9\n52.6\t47.7\n52.8\t47.5\n53\t47.3\n53.2\t47.1\n53.4\t46.9\n53.6\t46.7\n53.8\t46.5\n54\t46.3\n54.2\t46.1\n54.4\t45.9\n54.6\t45.7\n54.8\t45.5\n55\t45.3\n55.2\t45.1\n55.4\t44.9\n55.6\t44.7\n55.8\t44.5\n56\t44.3\n56.2\t44.1\n56.4\t43.9\n56.6\t43.7\n56.8\t43.5\n57\t43.3\n57.2\t43.1\n57.4\t42.9\n57.6\t42.7\n57.8\t42.5\n58\t42.3\n58.2\t42.1\n58.4\t41.9\n58.6\t41.7\n58.8\t41.5\n59\t41.3\n59.2\t41.1\n59.4\t40.9\n59.6\t40.7\n59.8\t40.5\n60\t40.3\n60.2\t40.1\n60.4\t39.9\n60.6\t39.7\n60.8\t39.5\n61\t39.3\n61.2\t39.1\n61.4\t38.9\n61.6\t38.7\n61.8\t38.5\n62\t38.3\n62.2\t38.1\n62.4\t37.9\n62.6\t37.7\n62.8\t37.5\n63\t37.3\n63.2\t37.1\n63.4\t36.9\n63.6\t36.7\n63.8\t36.5\n64\t36.3\n64.2\t36.1\n64.4\t35.9\n64.6\t35.7\n64.8\t35.5\n65\t35.3\n65.2\t35.1\n65.4\t34.9\n65.6\t34.7\n65.8\t34.5\n66\t34.3\n66.2\t34.1\n66.4\t33.9\n66.6\t33.7\n66.8\t33.5\n67\t33.3\n67.2\t33.1\n67.4\t32.9\n67.6\t32.7\n67.8\t32.5\n67.4\t32.3\n67\t32.1\n66.6\t31.9\n66.2\t31.7\n65.8\t31.5\n65.4\t31.3\n65\t31.1\n64.6\t30.9\n64.2\t30.7\n63.8\t30.5\n63.4\t30.3\n63\t30.1\n62.6\t29.9\n62.2\t29.7\n61.8\t29.5\n61.4\t29.3\n61\t29.1\n60.6\t28.9\n60.2\t28.7\n59.8\t28.5\n59.4\t28.3\n59\t28.1\n58.6\t27.9\n58.2\t27.7\n57.8\t27.5\n57.4\t27.3\n57\t27.1\n56.6\t26.9\n56.2\t26.7\n55.8\t26.5\n55.4\t26.3\n55\t26.1\n54.6\t25.9\n54.2\t25.7\n53.8\t25.5\n53.4\t25.3\n53\t25.1\n52.6\t24.9\n52.2\t24.7\n51.8\t24.5\n51.4\t24.3\n51\t24.1\n50.6\t23.9\n50.2\t23.7\n49.8\t23.5\n49.4\t23.3\n49\t23.1\n48.6\t22.9\n48.2\t22.7\n47.8\t22.5\n47.4\t22.3\n47\t22.1\n46.6\t21.9\n46.2\t21.7\n45.8\t21.5\n45.4\t21.3\n45\t21.1\n44.6\t20.9\n44.2\t20.7\n43.8\t20.5\n43.4\t20.3\n43\t20.1\n42.6\t19.9\n42.2\t19.7\n41.8\t19.5\n41.4\t19.3\n41\t19.1\n40.6\t18.9\n40.2\t18.7\n39.8\t18.5\n39.4\t18.3\n39\t18.1\n38.6\t17.9\n38.2\t17.7\n37.8\t17.5\n37.4\t17.3\n37\t17.1\n36.6\t16.9\n36.2\t16.7\n35.8\t16.5\n35.4\t16.3\n35\t16.1\n34.6\t15.9\n34.2\t15.7\n33.8\t15.5\n33.4\t15.3\n33\t15.1\n32.6\t14.9\n32.2\t14.7\n31.8\t14.5\n31.4\t14.3\n31\t14.1\n30.6\t13.9\n30.2\t13.7\n29.8\t13.5\n29.4\t13.3\n29\t13.1\n28.6\t12.9\n28.2\t12.7\n27.8\t12.5\n27.4\t12.3\n27\t12.1\n26.6\t11.9\n26.2\t11.7\n25.8\t11.5\n25.4\t11.3\n25\t11.1\n24.6\t10.9\n24.2\t10.7\n23.8\t11.3\n23.4\t11.9\n23\t12.5\n22.6\t13.1\n22.2\t13.7\n21.8\t14.3\n21.4\t14.9\n21\t15.5\n20.6\t16.1\n20.2\t16.7\n19.8\t17.3\n19.4\t17.9\n19\t18.5\n18.6\t19.1\n18.2\t19.7\n17.8\t20.3\n17.4\t20.9\n17\t21.5\n16.6\t22.1\n16.2\t22.7\n15.8\t23.3\n15.4\t23.9\n15\t24.5\n14.6\t25.1\n14.2\t25.7\n13.8\t26.3\n13.4\t26.9\n13\t27.5\n12.6\t28.1\n12.2\t28.7\n11.8\t29.3\n11.4\t29.9\n11\t30.5\n10.6\t31.1\n10.2\t31.7\n9.8\t32.3\n9.4\t32.9\n9\t33.5\n8.6\t34.1\n8.2\t34.7\n7.8\t35.3\n7.4\t35.9\n7\t36.5\n6.6\t37.1\n6.2\t37.7\n5.8\t38.3\n5.4\t38.9\n5\t39.5\n4.6\t40.1\n4.2\t40.7\n3.8\t41.3\n3.4\t41.9\n3\t42.5\n2.6\t43.1\n2.2\t43.7\n1.8\t44.3\n1.4\t44.9\n1\t45.5\n0.6\t46.1\n0.2\t46.7\n-0.2\t47.3\n-0.6\t47.9\n-1\t48.5\n-1.4\t49.1\n-1.8\t49.7\n-2.2\t50.3\n-2.6\t50.9\n-3\t51.5\n-3.4\t52.1\n-3.8\t52.7\n-4.2\t53.3\n-4.6\t53.9\n-5\t54.5\n-5.4\t55.1\n-5.8\t55.7\n-6.2\t56.3\n-6.6\t56.9\n-7\t57.5\n-7.4\t58.1\n-7.8\t58.7\n-8.2\t59.3\n-8.6\t59.9\n-9\t60.5\n-9.4\t61.1\n-9.8\t61.7\n-10.2\t62.3\n-10.6\t62.9\n-11\t63.5\n-11.4\t64.1\n-11.8\t64.7\n-12.2\t65.3\n-12.6\t65.9\n-13\t66.5\n-13.4\t67.1\n-13.8\t67.7\n-14.2\t68.3\n-14.6\t68.9\n-15\t69.5\n-15.4\t70.1\n-15.8\t70.7\n-16.2\t71.3\n-16.6\t71.9\n-17\t72.5\n-17.4\t73.1\n-17.8\t73.7\n-18.2\t74.3\n-18.6\t74.9\n-19\t75.5\n-19.4\t76.1\n-19.8\t76.7\n-20.2\t77.3\n-20.6\t77.9\n-21\t78.5\n-21.4\t79.1\n-21.8\t79.7\n-22.2\t80.3\n-22.6\t80.9\n-23\t81.5\n-23.4\t82.1\n-23.8\t82.7\n-24.2\t83.3\n-24.6\t83.9\n-25\t84.5\n-25.4\t85.1\n-25.8\t85.7\n-26.2\t86.3\n-26.6\t86.9\n-27\t87.5\n-27.4\t88.1\n-27.8\t88.7\n-28.2\t89.3\n-28.6\t89.9\n-29\t90.5\n-29.4\t91.1\n-29.8\t91.7\n-30.2\t92.3\n-30.6\t92.9\n-31\t93.5\n-31.4\t94.1\n-31.8\t93.8\n-32.2\t93.5\n-32.6\t93.2\n-33\t92.9\n-33.4\t92.6\n-33.8\t92.3\n-34.2\t92\n-34.6\t91.7\n-35\t91.4\n-35.4\t91.1\n-35.8\t90.8\n-36.2\t90.5\n-36.6\t90.2\n-37\t89.9\n-37.4\t89.6\n-37.8\t89.3\n-38.2\t89\n-38.6\t88.7\n-39\t88.4\n-39.4\t88.1\n-39.8\t87.8\n-40.2\t87.5\n-40.6\t87.2\n-41\t86.9\n-41.4\t86.6\n-41.8\t86.3\n-42.2\t86\n-42.6\t85.7\n-43\t85.4\n-43.4\t85.1\n-43.8\t84.8\n-44.2\t84.5\n-44.6\t84.2\n-45\t83.9\n-45.4\t83.6\n-45.8\t83.3\n-46.2\t83\n-46.6\t82.7\n-47\t82.4\n-47.4\t82.1\n-47.8\t81.8\n-48.2\t81.5\n-48.6\t81.2\n-49\t80.9\n-49.4\t80.6\n-49.8\t80.3\n-50.2\t80\n-50.6\t79.7\n-51\t79.4\n-51.4\t79.1\n-51.8\t78.8\n-52.2\t78.5\n-52.6\t78.2\n-53\t77.9\n-53.4\t77.6\n-53.8\t77.3\n-53.2\t77\n-52.6\t76.7\n-52\t76.4\n-51.4\t76.1\n-50.8\t75.8\n-50.2\t75.5\n-49.6\t75.2\n-49\t74.9\n-48.4\t74.6\n-47.8\t74.3\n-47.2\t74\n-46.6\t73.7\n-46\t73.4\n-45.4\t73.1\n-44.8\t72.8\n-44.2\t72.5\n-43.6\t72.2\n-43\t71.9\n-42.4\t71.6\n-41.8\t71.3\n-41.2\t71\n-40.6\t70.7\n-40\t70.4\n-39.4\t70.1\n-38.8\t69.8\n-38.2\t69.5\n-37.6\t69.2\n-37\t68.9\n-36.4\t68.6\n-35.8\t68.3\n-35.2\t68\n-34.6\t67.7\n-34\t67.4\n-33.4\t67.1\n-32.8\t66.8\n-32.2\t66.5\n-31.6\t66.2\n-31\t65.9\n-30.4\t65.6\n-29.8\t65.3\n-29.2\t65\n-28.6\t64.7\n-28\t64.4\n-27.4\t64.1\n-26.8\t63.8\n-26.2\t63.5\n-25.6\t63.2\n-25\t62.9\n-24.4\t62.6\n-23.8\t62.3\n-23.2\t62\n-22.6\t61.7\n-22\t61.4\n-21.4\t61.1\n-20.8\t60.8\n-20.2\t60.5\n-19.6\t60.2\n-19\t59.9\n-18.4\t59.6\n-17.8\t59.3\n-17.2\t59\n-16.6\t58.7\n-16\t58.4\n-15.4\t58.1\n-14.8\t57.8\n-14.2\t57.5\n-13.6\t57.2\n-13\t56.9\n-12.4\t56.6\n-11.8\t56.3\n-11.2\t56\n-10.6\t55.7\n-10\t55.4\n-9.4\t55.1\n-8.8\t54.8\n-8.2\t54.5\n-7.6\t54.2\n-7\t53.9\n-6.4\t53.6\n-5.8\t53.3\n-5.2\t53\n-4.6\t52.7\n-4\t52.4\n-3.4\t52.1\n-2.8\t51.8\n-2.2\t51.5\n-1.6\t51.2\n-1\t50.9\n-0.4\t50.6\n0.2\t50.3\n0.8\t50\n1.4\t49.7\n2\t49.4\n2.6\t49.1\n3.2\t48.8\n3.8\t48.5\n4.4\t48.2\n5\t47.9\n5.6\t47.6\n6.2\t47.3\n6.8\t47\n7.4\t46.7\n8\t46.4\n8.6\t46.1\n9.2\t45.8\n9.8\t45.5\n10.4\t45.2\n11\t44.9\n11.6\t44.6\n12.2\t44.3\n12.8\t44\n13.4\t43.7\n14\t43.4\n14.6\t43.1\n15.2\t42.8\n15.8\t42.5\n16.4\t42.2\n17\t41.9\n17.6\t41.6\n18.2\t41.3\n18.8\t41\n19.4\t40.7\n20\t40.4\n20.6\t40.1\n21.2\t39.8\n21.8\t39.5\n22.4\t39.2\n23\t38.9\n23.6\t38.6\n24.2\t38.3\n24.8\t38\n25.4\t37.7\n26\t37.4\n26.6\t37.1\n27.2\t36.8\n27.8\t36.5\n28.4\t36.2\n29\t35.9\n29.6\t35.6\n30.2\t35.3\n30.8\t35\n31.4\t34.7\n32\t34.4\n32.6\t34.1\n33.2\t33.8\n33.8\t33.5\n34.4\t33.2\n35\t32.9\n35.6\t32.6\n36.2\t32.3\n36.8\t32\n37.4\t31.7\n38\t31.4\n38.6\t31.1\n39.2\t30.8\n39.8\t30.5\n40.4\t30.2\n41\t29.9\n41.6\t29.6\n42.2\t29.3\n42.8\t29\n43.4\t28.7\n44\t28.4\n44.6\t28.1\n45.2\t27.8\n45.8\t27.5\n46.4\t27.2\n47\t26.9\n47.6\t26.6\n48.2\t26.3\n48.8\t26\n49.4\t25.7\n50\t25.4\n50.6\t25.1\n51.2\t24.8\n51.8\t24.5\n52.4\t24.2\n53\t23.9\n53.6\t23.6\n54.2\t23.3\n54.8\t23\n55.4\t22.7\n56\t22.4\n56.6\t22.1\n57.2\t21.8\n57.8\t21.5\n58.4\t21.2\n59\t20.9\n59.6\t20.6\n60.2\t20.3\n60.8\t20\n61.4\t19.7\n62\t19.4\n62.6\t19.1\n63.2\t18.8\n63.8\t18.5\n64.4\t18.2\n65\t17.9\n65.6\t17.6\n66.2\t17.3\n66.8\t17\n67.4\t16.7\n68\t16.4\n68.6\t16.1\n69.2\t15.8\n69.8\t15.5\n70.4\t15.2\n71\t14.9\n71.6\t14.6\n72.2\t14.3\n72.8\t14\n73.4\t13.7\n74\t13.4\n74.6\t13.1\n75.2\t12.8\n75.8\t12.5\n76.4\t12.2\n77\t11.9\n77.6\t11.6\n78.2\t11.3\n78.8\t11\n79.4\t10.7\n80\t10.4\n80.6\t10.1\n81.2\t9.8\n81.8\t9.5\n82.4\t9.2\n83\t8.9\n83.6\t8.6\n84.2\t8.3\n84.8\t8\n85.4\t7.7\n86\t7.4\n86.6\t7.1\n87.2\t6.8\n87.8\t6.5\n88.4\t6.2\n89\t5.9\n89.6\t5.6\n90.2\t5.3\n90.8\t5\n91.4\t4.7\n92\t4.4\n92.6\t4.1\n93.2\t3.8\n93.8\t3.5\n94.4\t3.2\n95\t2.9\n95.6\t2.6\n95.4\t2.3\n95.2\t2\n95\t1.7\n94.8\t1.4\n94.6\t1.1\n94.4\t0.8\n94.2\t0.5\n94\t0.2\n93.8\t-0.1\n93.6\t-0.4\n93.4\t-0.7\n93.2\t-1\n93\t-1.3\n92.8\t-1.6\n92.6\t-1.9\n92.4\t-2.2\n92.2\t-2.5\n92\t-2.8\n91.8\t-3.1\n91.6\t-3.4\n91.4\t-3.7\n91.2\t-4\n91\t-4.3\n90.8\t-4.6\n90.6\t-4.9\n90.4\t-5.2\n90.2\t-5.5\n90\t-5.8\n89.8\t-6.1\n89.6\t-6.4\n89.4\t-6.7\n89.2\t-7\n89\t-7.3\n88.8\t-7.6\n88.6\t-7.9\n88.4\t-8.2\n88.2\t-8.5\n88\t-8.8\n87.8\t-9.1\n87.6\t-9.4\n87.4\t-9.7\n87.2\t-10\n87\t-10.3\n86.8\t-10.6\n86.6\t-10.9\n86.4\t-11.2\n86.2\t-11.5\n86\t-11.8\n85.8\t-12.1\n85.6\t-12.4\n85.4\t-12.7\n85.2\t-13\n85\t-13.3\n84.8\t-13.6\n84.6\t-13.9\n84.4\t-14.2\n84.2\t-14.5\n84\t-14.8\n83.8\t-15.1\n83.6\t-15.4\n83.4\t-15.7\n83.2\t-16\n83\t-16.3\n82.8\t-16.6\n82.6\t-16.9\n82.4\t-17.2\n82.2\t-17.5\n82\t-17.8\n81.8\t-18.1\n81.6\t-18.4\n81.4\t-18.7\n81.2\t-19\n81\t-19.3\n80.8\t-19.6\n80.6\t-19.9\n80.4\t-20.2\n80.2\t-20.5\n80\t-20.8\n79.8\t-21.1\n79.6\t-21.4\n79.4\t-21.7\n79.2\t-22\n79\t-22.3\n78.8\t-22.6\n78.6\t-22.9\n78.4\t-23.2\n78.2\t-23.5\n78\t-23.8\n77.8\t-24.1\n77.6\t-24.4\n77.4\t-24.7\n77.2\t-25\n77\t-25.3\n76.8\t-25.6\n76.6\t-25.9\n76.4\t-26.2\n76.2\t-26.5\n76\t-26.8\n75.8\t-27.1\n75.6\t-27.4\n75.4\t-27.7\n75.2\t-28\n75\t-28.3\n74.8\t-28.6\n74.6\t-28.9\n74.4\t-29.2\n74.2\t-29.5\n74\t-29.8\n73.8\t-30.1\n73.6\t-30.4\n73.4\t-30.7\n73.2\t-31\n73\t-31.3\n72.8\t-31.6\n72.6\t-31.9\n72.4\t-32.2\n72.2\t-32.5\n72\t-32.8\n71.8\t-33.1\n71.6\t-33.4\n71.4\t-33.7\n71.2\t-34\n71\t-34.3\n70.8\t-34.6\n70.6\t-34.9\n70.4\t-35.2\n70.2\t-35.5\n70\t-35.8\n69.8\t-36.1\n69.6\t-36.4\n69.4\t-36.7\n69.2\t-37\n69\t-37.3\n68.8\t-37.6\n68.6\t-37.9\n68.4\t-38.2\n68.2\t-38.5\n68\t-38.8\n67.8\t-39.1\n67.6\t-39.4\n67.4\t-39.7\n67.2\t-40\n67\t-40.3\n66.8\t-40.6\n66.6\t-40.9\n66.4\t-41.2\n66.2\t-41.5\n66\t-41.8\n65.8\t-42.1\n65.6\t-42.4\n65.4\t-42.7\n65.2\t-43\n65\t-43.3\n64.8\t-43.6\n64.6\t-43.9\n64.4\t-44.2\n64.2\t-44.5\n64\t-44.8\n63.8\t-45.1\n63.6\t-45.4\n63.4\t-45.7\n63.2\t-46\n63\t-46.3\n62.8\t-46.6\n62.6\t-46.9\n62.4\t-47.2\n62.2\t-47.5\n62\t-47.8\n61.8\t-48.1\n61.6\t-48.4\n61.4\t-48.7\n61.2\t-49\n61\t-49.3\n60.8\t-49.6\n60.6\t-49.9\n60.4\t-50.2\n60.2\t-50.5\n60\t-50.8\n59.8\t-51.1\n59.6\t-51.4\n59.4\t-51.7\n59.2\t-52\n59\t-52.3\n58.8\t-52.6\n58.6\t-52.9\n58.4\t-53.2\n58.2\t-53.5\n58\t-53.8\n57.8\t-54.1\n57.6\t-54.4\n57.4\t-54.7\n57.2\t-55\n57\t-55.3\n56.8\t-55.6\n56.6\t-55.9\n56.4\t-56.2\n56.2\t-56.5\n56\t-56.8\n55.8\t-57.1\n55.6\t-57.4\n55.4\t-57.7\n55.2\t-58\n55\t-58.3\n54.8\t-58.6\n54.6\t-58.9\n54.4\t-59.2\n54.2\t-59.5\n54\t-59.8\n53.8\t-60.1\n53.6\t-60.4\n53.4\t-60.7\n53.2\t-61\n53\t-61.3\n52.8\t-61.6\n52.6\t-61.9\n52.4\t-62.2\n52.2\t-62.5\n52\t-62.8\n51.8\t-63.1\n51.6\t-63.4\n51.4\t-63.7\n51.2\t-64\n51\t-64.3\n50.8\t-64.6\n50.6\t-64.9\n50.4\t-65.2\n50.2\t-65.5\n50\t-65.8\n49.8\t-66.1\n49.6\t-66.4\n49.4\t-65.8\n49.2\t-65.2\n49\t-64.6\n48.8\t-64\n48.6\t-63.4\n48.4\t-62.8\n48.2\t-62.2\n48\t-61.6\n47.8\t-61\n47.6\t-60.4\n47.4\t-59.8\n47.2\t-59.2\n47\t-58.6\n46.8\t-58\n46.6\t-57.4\n46.4\t-56.8\n46.2\t-56.2\n46\t-55.6\n45.8\t-55\n45.6\t-54.4\n45.4\t-53.8\n45.2\t-53.2\n45\t-52.6\n44.8\t-52\n44.6\t-51.4\n44.4\t-50.8\n44.2\t-50.2\n44\t-49.6\n43.8\t-49\n43.6\t-48.4\n43.4\t-47.8\n43.2\t-47.2\n43\t-46.6\n42.8\t-46\n42.6\t-45.4\n42.4\t-44.8\n42.2\t-44.2\n42\t-43.6\n41.8\t-43\n41.6\t-42.4\n41.4\t-41.8\n41.2\t-41.2\n41\t-40.6\n40.8\t-40\n40.6\t-39.4\n40.4\t-38.8\n40.2\t-38.2\n40\t-37.6\n39.8\t-37\n39.6\t-36.4\n39.4\t-35.8\n39.2\t-35.2\n39\t-34.6\n38.8\t-34\n38.6\t-33.4\n38.4\t-32.8\n38.2\t-32.2\n38\t-31.6\n37.8\t-31\n37.6\t-30.4\n37.4\t-29.8\n37.2\t-29.2\n37\t-28.6\n36.8\t-28\n36.6\t-27.4\n36.4\t-26.8\n36.2\t-26.2\n36\t-25.6\n35.8\t-25\n35.6\t-24.4\n35.4\t-23.8\n35.2\t-23.2\n35\t-22.6\n34.8\t-22\n34.6\t-21.4\n34.4\t-20.8\n34.2\t-20.2\n34\t-19.6\n33.8\t-19\n33.6\t-18.4\n33.4\t-17.8\n33.2\t-17.2\n33\t-16.6\n32.8\t-16\n32.6\t-15.4\n32.4\t-14.8\n32.2\t-14.2\n32\t-13.6\n31.8\t-13\n31.6\t-12.4\n31.4\t-11.8\n31.2\t-11.2\n31\t-10.6\n30.8\t-10\n30.6\t-9.4\n30.4\t-8.8\n30.2\t-8.2\n30\t-7.6\n29.8\t-7\n29.6\t-6.4\n29.4\t-5.8\n29.2\t-5.2\n29\t-4.6\n28.8\t-4\n28.6\t-3.4\n28.4\t-2.8\n28.2\t-2.2\n28\t-1.6\n27.8\t-1\n27.6\t-0.4\n27.4\t0.2\n27.2\t0.8\n27\t1.4\n26.8\t2\n26.6\t2.6\n26.4\t3.2\n26.2\t3.8\n26\t4.4\n25.8\t5\n25.6\t5.6\n25.4\t6.2\n25.2\t6.8\n25\t7.4\n24.8\t8\n24.6\t8.6\n24.4\t9.2\n24.2\t9.8\n24\t10.4\n23.8\t11\n23.6\t11.6\n23.4\t12.2\n23.2\t12.8\n23\t13.4\n22.8\t14\n22.6\t14.6\n22.4\t15.2\n22.2\t15.8\n22\t16.4\n21.8\t17\n21.6\t17.6\n21.4\t18.2\n21.2\t18.8\n21\t19.4\n20.8\t20\n20.6\t20.6\n20.4\t21.2\n20.2\t21.8\n20\t22.4\n19.8\t23\n19.6\t23.6\n19.4\t24.2\n19.2\t24.8\n19\t25.4\n18.8\t26\n18.6\t26.6\n18.4\t27.2\n18.2\t27.8\n18\t28.4\n17.8\t29\n17.6\t29.6\n17.4\t30.2\n17.2\t30.8\n17\t31.4\n16.8\t32\n16.6\t32.6\n16.4\t33.2\n16.2\t33.8\n16\t34.4\n15.8\t35\n15.6\t35.6\n15.4\t36.2\n15.2\t36.8\n15\t37.4\n14.8\t38\n14.6\t38.6\n14.4\t39.2\n14.2\t39.8\n14\t40.4\n13.8\t40.1\n13.6\t39.8\n13.4\t39.5\n13.2\t39.2\n13\t38.9\n12.8\t38.6\n12.6\t38.3\n12.4\t38\n12.2\t37.7\n12\t37.4\n11.8\t37.1\n11.6\t36.8\n11.4\t36.5\n11.2\t36.2\n11\t35.9\n10.8\t35.6\n10.6\t35.3\n10.4\t35\n10.2\t34.7\n10\t34.4\n9.8\t34.1\n9.6\t33.8\n9.4\t33.5\n9.2\t33.2\n9\t32.9\n8.8\t32.6\n8.6\t32.3\n8.4\t32\n8.2\t31.7\n8\t31.4\n7.8\t31.1\n7.6\t30.8\n7.4\t30.5\n7.2\t30.2\n7\t29.9\n6.8\t29.6\n6.6\t29.3\n6.4\t29\n6.2\t28.7\n6\t28.4\n5.8\t28.1\n5.6\t27.8\n5.4\t27.5\n5.2\t27.2\n5\t26.9\n4.8\t26.6\n4.6\t26.3\n4.4\t26\n4.2\t25.7\n4\t25.4\n3.8\t25.1\n3.6\t24.8\n3.4\t24.5\n3.2\t24.2\n3\t23.9\n2.8\t23.6\n2.6\t23.3\n2.4\t23\n2.2\t22.7\n2\t22.4\n1.8\t22.1\n1.6\t21.8\n1.4\t21.5\n1.2\t21.2\n1\t20.9\n0.8\t20.6\n0.6\t20.3\n0.4\t20\n0.2\t19.7\n-2.71644E-12\t19.4\n-0.2\t19.1\n-0.4\t18.8\n-0.6\t18.5\n-0.8\t18.2\n-1\t17.9\n-1.2\t17.6\n-1.4\t17.3\n-1.6\t17\n-1.8\t16.7\n-2\t16.4\n-2.2\t16.1\n-2.4\t15.8\n-2.6\t15.5\n-2.8\t15.2\n-3\t14.9\n-3.2\t14.6\n-3.4\t14.3\n-3.6\t14\n-3.8\t13.7\n-4\t13.4\n-4.2\t13.1\n-4.4\t12.8\n-4.6\t12.5\n-4.8\t12.2\n-5\t11.9\n-5.2\t11.6\n-5.4\t11.3\n-5.6\t11\n-5.8\t10.7\n-6\t10.4\n-6.2\t10.1\n-6.4\t9.8\n-6.6\t9.5\n-7.1\t9.2\n-7.6\t8.9\n-8.1\t8.6\n-8.6\t8.3\n-9.1\t8\n-9.6\t7.7\n-10.1\t7.4\n-10.6\t7.1\n-11.1\t6.8\n-11.6\t6.5\n-12.1\t6.2\n-12.6\t5.9\n-13.1\t5.6\n-13.6\t5.3\n-14.1\t5\n-14.6\t4.7\n-15.1\t4.4\n-15.6\t4.1\n-16.1\t3.8\n-16.6\t3.5\n-17.1\t3.2\n-17.6\t2.9\n-18.1\t2.6\n-18.6\t2.3\n-19.1\t2\n-19.6\t1.7\n-20.1\t1.4\n-20.6\t1.1\n-21.1\t0.8\n-21.6\t0.5\n-22.1\t0.2\n-22.6\t-0.1\n-23.1\t-0.4\n-23.6\t-0.7\n-24.1\t-1\n-24.6\t-1.3\n-25.1\t-1.6\n-25.6\t-1.9\n-26.1\t-2.2\n-26.6\t-2.5\n-27.1\t-2.8\n-27.6\t-3.1\n-28.1\t-3.4\n-28.6\t-3.7\n-29.1\t-4\n-29.6\t-4.3\n-30.1\t-4.6\n-30.6\t-4.9\n-31.1\t-5.2\n-31.6\t-5.5\n-32.1\t-5.8\n-32.6\t-6.1\n-33.1\t-6.4\n-33.6\t-6.7\n-34.1\t-7\n-34.6\t-7.3\n-35.1\t-7.6\n-35.6\t-7.9\n-36.1\t-8.2\n-36.6\t-8.5\n-37.1\t-8.8\n-37.6\t-9.1\n-38.1\t-9.4\n-38.6\t-9.7\n-39.1\t-10\n-39.6\t-10.3\n-40.1\t-10.6\n-40.6\t-10.9\n-41.1\t-11.2\n-41.6\t-11.5\n-42.1\t-11.8\n-42.6\t-12.1\n-43.1\t-12.4\n-43.6\t-12.7\n-44.1\t-13\n-44.6\t-13.3\n-45.1\t-13.6\n-45.6\t-13.9\n-46.1\t-14.2\n-46.6\t-14.5\n-47.1\t-14.8\n-47.6\t-15.1\n-48.1\t-15.4\n-48.6\t-15.7\n-49.1\t-16\n-49.6\t-16.3\n-50.1\t-16.6\n-50.6\t-16.9\n-51.1\t-17.2\n-51.6\t-17.5\n-52.1\t-17.8\n-52.6\t-18.1\n-53.1\t-18.4\n-53.6\t-18.7\n-54.1\t-19\n-54.6\t-19.3\n-55.1\t-19.6\n-55.6\t-19.9\n-56.1\t-20.2\n-56.6\t-20.5\n-57.1\t-20.8\n-57.6\t-21.1\n-58.1\t-21.4\n-58.6\t-21.7\n-59.1\t-22\n-59.6\t-22.3\n-60.1\t-22.6\n-60.6\t-22.9\n-61.1\t-23.2\n-61.6\t-23.5\n-62.1\t-23.8\n-62.6\t-24.1\n-63.1\t-24.4\n-63.6\t-24.7\n-64.1\t-25\n-64.6\t-25.3\n-65.1\t-25.6\n-65.6\t-25.9\n-66.1\t-26.2\n-66.6\t-26.5\n-67.1\t-26.8\n-67.6\t-27.1\n-68.1\t-27.4\n-68.6\t-27.7\n-69.1\t-28\n-69.6\t-28.3\n-70.1\t-28.6\n-70.6\t-28.9\n-71.1\t-29.2\n-71.6\t-29.5\n-72.1\t-29.8\n-72.6\t-30.1\n-73.1\t-30.4\n-73.6\t-30.7\n-74.1\t-31\n-74.6\t-31.3\n-75.1\t-31.6\n-75.6\t-31.9\n-76.1\t-32.2\n-76.6\t-32.5\n-77.1\t-32.8\n-77.6\t-33.1\n-78.1\t-33.4\n-78.6\t-33.7\n-79.1\t-34\n-79.6\t-34.3\n-80.1\t-34.6\n-80.6\t-34.9\n-81.1\t-35.2\n-81.6\t-35.5\n-82.1\t-35.8\n-82.6\t-36.1\n-83.1\t-36.4\n-83.6\t-36.7\n-84.1\t-37\n-84.6\t-37.3\n-85.1\t-37.6\n-85.6\t-37.9\n-86.1\t-38.2\n-86.6\t-38.5\n-87.1\t-38.8\n-87.6\t-39.1\n-88.1\t-39.4\n-88.6\t-39.7\n-89.1\t-40\n-89.6\t-40.3\n-90.1\t-40.6\n-90.6\t-40.9\n-91.1\t-41.2\n-91.6\t-41.5\n-92.1\t-41.8\n-92.6\t-42.1\n-93.1\t-42.4\n-93.6\t-42.7\n-94.1\t-43\n-94.6\t-43.3\n-95.1\t-43.6\n-95.6\t-43.9\n-96.1\t-44.2\n-96.6\t-44.5\n-97.1\t-44.8\n-97.6\t-45.1\n-98.1\t-45.4\n-97.7\t-45.7\n-97.3\t-46\n-96.9\t-46.3\n-96.5\t-46.6\n-96.1\t-46.9\n-95.7\t-47.2\n-95.3\t-47.5\n-94.9\t-47.8\n-94.5\t-48.1\n-94.1\t-48.4\n-93.7\t-48.7\n-93.3\t-49\n-92.9\t-49.3\n-92.5\t-49.6\n-92.1\t-49.9\n-91.7\t-50.2\n-91.3\t-50.5\n-90.9\t-50.8\n-90.5\t-51.1\n-90.1\t-51.4\n-89.7\t-51.7\n-89.3\t-52\n-88.9\t-52.3\n-88.5\t-52.6\n-88.1\t-52.9\n-87.7\t-53.2\n-87.3\t-53.5\n-86.9\t-53.8\n-86.5\t-54.1\n-86.1\t-54.4\n-85.7\t-54.7\n-85.3\t-55\n-84.9\t-55.3\n-84.5\t-55.6\n-84.1\t-55.9\n-83.7\t-56.2\n-83.3\t-56.5\n-82.9\t-56.8\n-82.5\t-57.1\n-82.1\t-57.4\n-81.7\t-57.7\n-81.3\t-58\n-80.9\t-58.3\n-80.5\t-58.6\n-80.1\t-58.9\n-79.7\t-59.2\n-79.3\t-59.5\n-78.9\t-59.8\n-78.5\t-60.1\n-78.1\t-60.4\n-77.7\t-60.7\n-77.3\t-61\n-76.9\t-61.3\n-76.5\t-61.6\n-76.1\t-61.9\n-75.7\t-62.2\n-75.3\t-62.5\n-74.9\t-62.8\n-74.5\t-63.1\n-74.1\t-63.4\n-73.7\t-63.7\n-73.3\t-64\n-72.9\t-64.3\n-72.5\t-64.6\n-72.1\t-64.9\n-71.7\t-65.2\n-71.3\t-65.5\n-70.9\t-65.8\n-70.5\t-66.1\n-70.1\t-66.4\n-69.7\t-66.7\n-69.3\t-67\n-68.9\t-67.3\n-68.5\t-67.6\n-68.1\t-67.9\n-67.7\t-68.2\n-67.3\t-68.5\n-66.9\t-68.8\n-66.5\t-69.1\n-66.1\t-69.4\n-65.7\t-69.7\n-65.3\t-70\n-64.9\t-70.3\n-64.5\t-70.6\n-64.1\t-70.9\n-63.7\t-71.2\n-63.3\t-71.5\n-62.9\t-71.8\n-62.5\t-72.1\n-62.1\t-72.4\n-61.7\t-72.7\n-61.3\t-73\n-60.9\t-73.3\n-60.5\t-73.6\n-60.1\t-73.9\n-59.7\t-74.2\n-59.3\t-74.5\n-58.9\t-74.8\n-58.5\t-75.1\n-58.1\t-75.4\n-57.7\t-75.7\n-57.3\t-76\n-56.9\t-76.3\n-56.5\t-76.6\n-56.1\t-76.9\n-55.7\t-77.2\n-55.3\t-77.5\n-54.9\t-77.8\n-54.5\t-78.1\n-54.1\t-78.4\n-53.7\t-78.7\n-53.3\t-79\n-52.9\t-79.3\n-52.5\t-79.6\n-52.1\t-79.9\n-51.7\t-80.2\n-51.3\t-80.5\n-50.9\t-80.8\n-50.5\t-81.1\n-50.1\t-81.4\n-49.7\t-81.7\n-49.3\t-82\n-48.9\t-82.3\n-48.5\t-82.6\n-48.1\t-82.9\n-47.7\t-83.2\n-47.3\t-83.5\n-46.9\t-83.8\n-46.5\t-84.1\n-46.1\t-84.4\n-45.7\t-84.7\n-45.3\t-85\n-44.9\t-85.3\n-44.5\t-85.6\n-44.1\t-85.9\n-43.7\t-86.2\n-43.3\t-86.5\n-42.9\t-86.8\n-42.5\t-87.1\n-42.1\t-87.4\n-41.7\t-87.7\n-41.3\t-88\n-40.9\t-88.3\n-40.5\t-88.6\n-40.1\t-88.9\n-39.7\t-89.2\n-39.3\t-89.5\n-38.9\t-89.8\n-38.5\t-90.1\n-38.1\t-90.4\n-37.7\t-90.3\n-37.3\t-90.2\n-36.9\t-90.1\n-36.5\t-90\n-36.1\t-89.9\n-35.7\t-89.8\n-35.3\t-89.7\n-34.9\t-89.6\n-34.5\t-89.5\n-34.1\t-89.4\n-33.7\t-89.3\n-33.3\t-89.2\n-32.9\t-89.1\n-32.5\t-89\n-32.1\t-88.9\n-31.7\t-88.8\n-31.3\t-88.7\n-30.9\t-88.6\n-30.5\t-88.5\n-30.1\t-88.4\n-29.7\t-88.3\n-29.3\t-88.2\n-28.9\t-88.1\n-28.5\t-88\n-28.1\t-87.9\n-27.7\t-87.8\n-27.3\t-87.7\n-26.9\t-87.6\n-26.5\t-87.5\n-26.1\t-87.4\n-25.7\t-87.3\n-25.3\t-87.2\n-24.9\t-87.1\n-24.5\t-87\n-24.1\t-86.9\n-23.7\t-86.8\n-23.3\t-86.7\n-22.9\t-86.6\n-22.5\t-86.5\n-22.1\t-86.4\n-21.7\t-86.3\n-21.3\t-86.2\n-20.9\t-86.1\n-20.5\t-86\n-20.1\t-85.9\n-19.7\t-85.8\n-19.3\t-85.7\n-18.9\t-85.6\n-18.5\t-85.5\n-18.1\t-85.4\n-17.7\t-85.3\n-17.3\t-85.2\n-16.9\t-85.1\n-16.5\t-85\n-16.1\t-84.9\n-15.7\t-84.8\n-15.3\t-84.7\n-14.9\t-84.6\n-14.5\t-84.5\n-14.1\t-84.4\n-13.7\t-84.3\n-13.3\t-84.2\n-12.9\t-84.1\n-12.5\t-84\n-12.1\t-83.9\n-11.7\t-83.8\n-11.3\t-83.7\n-10.9\t-83.6\n-10.5\t-83.5\n-10.1\t-83.4\n-9.7\t-83.3\n-9.3\t-83.2\n-8.9\t-83.1\n-8.5\t-83\n-8.1\t-82.9\n-7.7\t-82.8\n-7.3\t-82.7\n-6.9\t-82.6\n-6.5\t-82.5\n-6.1\t-82.4\n-5.7\t-82.3\n-5.3\t-82.2\n-4.9\t-82.1\n-4.5\t-82\n-4.1\t-81.9\n-3.7\t-81.8\n-3.3\t-81.7\n-2.9\t-81.6\n-2.5\t-81.5\n-2.1\t-81.4\n-1.7\t-81.3\n-1.3\t-81.2\n-0.9\t-81.1\n-0.5\t-81\n-0.1\t-80.9\n0.3\t-80.8\n0.7\t-80.7\n1.1\t-80.6\n1.5\t-80.5\n1.9\t-80.4\n2.3\t-80.3\n2.7\t-80.2\n3.1\t-80.1\n3.5\t-80\n3.9\t-79.9\n4.3\t-79.8\n4.7\t-79.7\n5.1\t-79.6\n5.5\t-79.5\n5.9\t-79.4\n6.3\t-79.3\n6.7\t-79.2\n7.1\t-79.1\n7.5\t-79\n7.9\t-78.9\n8.3\t-78.8\n8.7\t-78.7\n9.1\t-78.6\n9.5\t-78.5\n9.1\t-78.4\n8.7\t-78.3\n8.3\t-78.2\n7.9\t-78.1\n7.5\t-78\n7.1\t-77.9\n6.7\t-77.8\n6.3\t-77.7\n5.9\t-77.6\n5.5\t-77.5\n5.1\t-77.4\n4.7\t-77.3\n4.3\t-77.2\n3.9\t-77.1\n3.5\t-77\n3.1\t-76.9\n2.7\t-76.8\n2.3\t-76.7\n1.9\t-76.6\n1.5\t-76.5\n1.1\t-76.4\n0.7\t-76.3\n0.3\t-76.2\n-0.1\t-76.1\n-0.5\t-76\n-0.9\t-75.9\n-1.3\t-75.8\n-1.7\t-75.7\n-2.1\t-75.6\n-2.5\t-75.5\n-2.9\t-75.4\n-3.3\t-75.3\n-3.7\t-75.2\n-4.1\t-75.1\n-4.5\t-75\n-4.9\t-74.9\n-5.3\t-74.8\n-5.7\t-74.7\n-6.1\t-74.6\n-6.5\t-74.5\n-6.9\t-74.4\n-7.3\t-74.3\n-7.7\t-74.2\n-8.1\t-74.1\n-8.5\t-74\n-8.9\t-73.9\n-9.3\t-73.8\n-9.7\t-73.7\n-10.1\t-73.6\n-10.5\t-73.5\n-10.9\t-73.4\n-11.3\t-73.3\n-11.7\t-73.2\n-12.1\t-73.1\n-12.5\t-73\n-12.9\t-72.9\n-13.3\t-72.8\n-13.7\t-72.7\n-14.1\t-72.6\n-14.5\t-72.5\n-14.9\t-72.4\n-15.3\t-72.3\n-15.7\t-72.2\n-16.1\t-72.1\n-16.5\t-72\n-16.9\t-71.9\n-17.3\t-71.8\n-17.7\t-71.7\n-18.1\t-71.6\n-18.5\t-71.5\n-18.9\t-71.4\n-19.3\t-71.3\n-19.7\t-71.2\n-20.1\t-71.1\n-20.5\t-71\n-20.9\t-70.9\n-21.3\t-70.8\n-21.7\t-70.7\n-22.1\t-70.6\n-22.5\t-70.5\n-22.9\t-70.4\n-23.3\t-70.3\n-23.7\t-70.2\n-24.1\t-70.1\n-24.5\t-70\n-24.9\t-69.9\n-25.3\t-69.8\n-25.7\t-69.7\n-26.1\t-69.6\n-26.5\t-69.5\n-26.9\t-69.4\n-27.3\t-69.3\n-27.7\t-69.2\n-28.1\t-69.1\n-28.5\t-69\n-28.9\t-68.9\n-29.3\t-68.8\n-29.7\t-68.7\n-30.1\t-68.6\n-30.5\t-68.5\n-30.9\t-68.4\n-31.3\t-68.3\n-31.7\t-68.2\n-32.1\t-68.1\n-32.5\t-68\n-32.9\t-67.9\n-33.3\t-67.8\n-33.7\t-67.7\n-34.1\t-67.6\n-34.5\t-67.5\n-34.9\t-67.4\n-35.3\t-67.3\n-35.7\t-67.2\n-36.1\t-67.1\n-36.5\t-67\n-36.9\t-66.9\n-37.3\t-66.8\n-37.7\t-66.7\n-38.1\t-66.6\n-38.5\t-66.5\n-38.9\t-66.4\n-39.3\t-66.3\n-39.7\t-66.2\n-40.1\t-66.1\n-40.5\t-66\n-40.9\t-65.9\n-41.3\t-65.8\n-41.7\t-65.7\n-42.1\t-65.6\n-42.5\t-65.5\n-42.9\t-65.4\n-43.3\t-65.1\n-43.7\t-64.8\n-44.1\t-64.5\n-44.5\t-64.2\n-44.9\t-63.9\n-45.3\t-63.6\n-45.7\t-63.3\n-46.1\t-63\n-46.5\t-62.7\n-46.9\t-62.4\n-47.3\t-62.1\n-47.7\t-61.8\n-48.1\t-61.5\n-48.5\t-61.2\n-48.9\t-60.9\n-49.3\t-60.6\n-49.7\t-60.3\n-50.1\t-60\n-50.5\t-59.7\n-50.9\t-59.4\n-51.3\t-59.1\n-51.7\t-58.8\n-52.1\t-58.5\n-52.5\t-58.2\n-52.9\t-57.9\n-53.3\t-57.6\n-53.7\t-57.3\n-54.1\t-57\n-54.5\t-56.7\n-54.9\t-56.4\n-55.3\t-56.1\n-55.7\t-55.8\n-56.1\t-55.5\n-56.5\t-55.2\n-56.9\t-54.9\n-57.3\t-54.6\n-57.7\t-54.3\n-58.1\t-54\n-58.5\t-53.7\n-58.9\t-53.4\n-59.3\t-53.1\n-59.7\t-52.8\n-60.1\t-52.5\n-60.5\t-52.2\n-60.9\t-51.9\n-61.3\t-51.6\n-61.7\t-51.3\n-62.1\t-51\n-62.5\t-50.7\n-62.9\t-50.4\n-63.3\t-50.1\n-63.7\t-49.8\n-64.1\t-49.5\n-64.5\t-49.2\n-64.9\t-48.9\n-65.3\t-48.6\n-65.7\t-48.3\n-66.1\t-48\n-66.5\t-47.7\n-66.9\t-47.4\n-67.3\t-47.1\n-67.7\t-46.8\n-68.1\t-46.5\n-68.5\t-46.2\n-68.9\t-45.9\n-69.3\t-45.6\n-69.7\t-45.3\n-70.1\t-45\n-70.5\t-44.7\n-70.9\t-44.4\n-71.3\t-44.1\n-71.7\t-43.8\n-72.1\t-43.5\n-72.5\t-43.2\n-72.9\t-42.9\n-73.3\t-42.6\n-73.7\t-42.3\n-74.1\t-42\n-74.5\t-41.7\n-74.9\t-41.4\n-75.3\t-41.1\n-75.7\t-40.8\n-76.1\t-40.5\n-76.5\t-40.2\n-76.9\t-39.9\n-77.3\t-39.6\n-77.7\t-39.3\n-78.1\t-39\n-78.5\t-38.7\n-78.9\t-38.4\n-79.3\t-38.1\n-79.7\t-37.8\n-80.1\t-37.5\n-80.5\t-37.2\n-80.9\t-36.9\n-81.3\t-36.6\n-81.7\t-36.3\n-82.1\t-36\n-82.5\t-35.7\n-82.9\t-35.4\n-83.3\t-35.1\n-83.7\t-34.8\n-84.1\t-34.5\n-84.5\t-34.2\n-84.9\t-33.9\n-85.3\t-33.6\n-85.7\t-33.3\n-86.1\t-33\n-86.5\t-32.7\n-86.9\t-32.4\n-87.3\t-32.1\n-87.7\t-31.8\n-88.1\t-31.5\n-88.5\t-31.2\n-88.9\t-30.9\n-89.3\t-30.6\n-89.7\t-30.3\n-90.1\t-30\n-90.5\t-29.7\n-90\t-29.4\n-89.5\t-29.1\n-89\t-28.8\n-88.5\t-28.5\n-88\t-28.2\n-87.5\t-27.9\n-87\t-27.6\n-86.5\t-27.3\n-86\t-27\n-85.5\t-26.7\n-85\t-26.4\n-84.5\t-26.1\n-84\t-25.8\n-83.5\t-25.5\n-83\t-25.2\n-82.5\t-24.9\n-82\t-24.6\n-81.5\t-24.3\n-81\t-24\n-80.5\t-23.7\n-80\t-23.4\n-79.5\t-23.1\n-79\t-22.8\n-78.5\t-22.5\n-78\t-22.2\n-77.5\t-21.9\n-77\t-21.6\n-76.5\t-21.3\n-76\t-21\n-75.5\t-20.7\n-75\t-20.4\n-74.5\t-20.1\n-74\t-19.8\n-73.5\t-19.5\n-73\t-19.2\n-72.5\t-18.9\n-72\t-18.6\n-71.5\t-18.3\n-71\t-18\n-70.5\t-17.7\n-70\t-17.4\n-69.5\t-17.1\n-69\t-16.8\n-68.5\t-16.5\n-68\t-16.2\n-67.5\t-15.9\n-67\t-15.6\n-66.5\t-15.3\n-66\t-15\n-65.5\t-14.7\n-65\t-14.4\n-64.5\t-14.1\n-64\t-13.8\n-63.5\t-13.5\n-63\t-13.2\n-62.5\t-12.9\n-62\t-12.6\n-61.5\t-12.3\n-61\t-12\n-60.5\t-11.7\n-60\t-11.4\n-59.5\t-11.1\n-59\t-10.8\n-58.5\t-10.5\n-58\t-10.2\n-57.5\t-9.9\n-57\t-9.6\n-56.5\t-9.3\n-56\t-9\n-55.5\t-8.7\n-55\t-8.4\n-54.5\t-8.1\n-54\t-7.8\n-53.5\t-7.5\n-53\t-7.2\n-52.5\t-6.9\n-52\t-6.6\n-51.5\t-6.3\n-51\t-6\n-50.5\t-5.7\n-50\t-5.4\n-49.5\t-5.1\n-49\t-4.8\n-48.5\t-4.5\n-48\t-4.2\n-47.5\t-3.9\n-47\t-3.6\n-46.5\t-3.3\n-46\t-3\n-45.5\t-2.7\n-45\t-2.4\n-44.5\t-2.1\n-44\t-1.8\n-43.5\t-1.5\n-43\t-1.2\n-42.5\t-0.9\n-42\t-0.6\n-41.5\t-0.3\n-41\t-1.83087E-12\n-40.5\t0.3\n-40\t0.6\n-39.5\t0.9\n-39\t1.2\n-38.5\t1.5\n-38\t1.8\n-37.5\t2.1\n-37\t2.4\n-36.5\t2.7\n-36\t3\n-35.5\t3.3\n-35\t3.6\n-34.5\t3.9\n-34\t4.2\n-33.5\t4.5\n-33\t4.8\n-32.5\t5.1\n-32\t5.4\n-31.5\t5.7\n-31\t6\n-30.5\t6.3\n-30\t6.6\n-29.5\t6.9\n-29\t7.2\n-28.5\t7.5\n-28\t7.8\n-27.5\t8.1\n-27\t8.4\n-26.5\t8.7\n-26\t9\n-25.5\t9.3\n-25\t9.6\n-24.5\t9.9\n-24\t10.2\n-23.5\t10.5\n-23\t10.8\n-22.5\t11.1\n-22\t11.4\n-21.5\t11.7\n-21\t12\n-20.5\t12.3\n-20\t12.6\n-19.5\t12.9\n-19\t13.2\n-18.5\t13.5\n-18\t13.8\n-17.5\t14.1\n-17\t14.4\n-16.5\t14.7\n-16\t15\n-15.5\t15.3\n-15\t15.6\n-14.5\t15.9\n-14\t16.2\n-13.5\t16.5\n-13\t16.8\n-12.5\t17.1\n-12\t17.4\n-11.5\t17.7\n-11\t18\n-10.5\t18.3\n-10\t18.6\n-9.5\t18.9\n-9\t19.2\n-8.5\t19.5\n-8\t19.8\n-7.5\t20.1\n-7\t20.4\n-6.5\t20.7\n-6\t21\n-5.5\t21.3\n-5\t21.6\n-4.5\t21.9\n-4\t22.2\n-3.5\t22.5\n-3\t22.8\n-2.5\t23.1\n-2\t23.4\n-1.5\t23.7\n-1\t24\n-0.5\t24.3\n-2.6148E-12\t24.6\n0.5\t24.9\n1\t25.2\n1.5\t25.5\n2\t25.8\n2.5\t26.1\n3\t26.4\n3.5\t26.7\n4\t27\n4.5\t27.3\n5\t27.6\n5.5\t27.9\n6\t28.2\n6.5\t28.5\n7\t28.8\n7.5\t29.1\n8\t29.4\n8.5\t29.7\n9\t30\n9.5\t30.3\n10\t30.6\n10.5\t30.9\n11\t31.2\n11.5\t31.5\n12\t31.8\n12.5\t32.1\n13\t32.4\n13.5\t32.7\n14\t33\n14.5\t33.3\n15\t33.6\n15.5\t33.9\n16\t34.2\n16.5\t34.5\n17\t34.8\n17.5\t35.1\n18\t35.4\n18.5\t35.7\n19\t36\n19.5\t36.3\n20\t36.6\n20.5\t36.9\n20.2\t37.2\n19.9\t37.5\n19.6\t37.8\n19.3\t38.1\n19\t38.4\n18.7\t38.7\n18.4\t39\n18.1\t39.3\n17.8\t39.6\n17.5\t39.9\n17.2\t40.2\n16.9\t40.5\n16.6\t40.8\n16.3\t41.1\n16\t41.4\n15.7\t41.7\n15.4\t42\n15.1\t42.3\n14.8\t42.6\n14.5\t42.9\n14.2\t43.2\n13.9\t43.5\n13.6\t43.8\n13.3\t44.1\n13\t44.4\n12.7\t44.7\n12.4\t45\n12.1\t45.3\n11.8\t45.6\n11.5\t45.9\n11.2\t46.2\n10.9\t46.5\n10.6\t46.8\n10.3\t47.1\n10\t47.4\n9.7\t47.7\n9.4\t48\n9.1\t48.3\n8.8\t48.6\n8.5\t48.9\n8.2\t49.2\n7.9\t49.5\n7.6\t49.8\n7.3\t50.1\n7\t50.4\n6.7\t50.7\n6.4\t51\n6.1\t51.3\n5.8\t51.6\n5.5\t51.9\n5.2\t52.2\n4.9\t52.5\n4.6\t52.8\n4.3\t53.1\n4\t53.4\n3.7\t53.7\n3.4\t54\n3.1\t54.3\n2.8\t54.6\n2.5\t54.9\n2.2\t55.2\n1.9\t55.5\n1.6\t55.8\n1.3\t56.1\n1\t56.4\n0.7\t56.7\n0.4\t57\n0.1\t57.3\n-0.2\t57.6\n-0.5\t57.9\n-0.8\t58.2\n-1.1\t58.5\n-1.4\t58.8\n-1.7\t59.1\n-2\t59.4\n-2.3\t59.7\n-2.6\t60\n-2.9\t60.3\n-3.2\t60.6\n-3.5\t60.9\n-3.8\t61.2\n-4.1\t61.5\n-4.4\t61.8\n-4.7\t62.1\n-5\t62.4\n-5.3\t62.7\n-5.6\t63\n-5.9\t63.3\n-6.2\t63.6\n-6.5\t63.9\n-6.8\t64.2\n-7.1\t64.5\n-7.4\t64.8\n-7.7\t65.1\n-8\t65.4\n-8.3\t65.7\n-8.6\t66\n-8.9\t66.3\n-9.2\t66.6\n-9.5\t66.9\n-9.8\t67.2\n-10.1\t67.5\n-10.4\t67.8\n-10.7\t68.1\n-11\t68.4\n-11.3\t68.7\n-11.6\t69\n-11.9\t69.3\n-12.2\t69.6\n-12.5\t69.9\n-12.8\t70.2\n-13.1\t70.5\n-13.4\t70.8\n-13.7\t71.1\n-14\t71.4\n-14.3\t71.7\n-14.6\t72\n-14.9\t72.3\n-15.2\t72.6\n-15.5\t72.9\n-15.8\t73.2\n-16.1\t73.5\n-16.4\t73.8\n-16.7\t74.1\n-17\t74.4\n-17.3\t74.7\n-17.6\t75\n-17.9\t75.3\n-18.2\t75.6\n-18.5\t75.9\n-18.8\t76.2\n-19.1\t76.5\n-19.4\t76.8\n-19.7\t77.1\n-20\t77.4\n-20.3\t77.7\n-20.6\t78\n-20.9\t78.3\n-21.2\t78.6\n-21.5\t78.9\n-21.8\t79.2\n-22.1\t79.5\n-22.4\t79.8\n-22.7\t80.1\n-23\t80.4\n-23.3\t80.7\n-23.6\t81\n-23.9\t81.3\n-24.2\t81.6\n-24.5\t81.9\n-24.8\t82.2\n-25.1\t82.5\n-25.4\t82.8\n-25.7\t83.1\n-26\t83.4\n-26.3\t83.7\n-26.6\t84\n-26.9\t84.3\n-27.2\t84.6\n-27.5\t84.9\n-27.8\t85.2\n-28.1\t85.5\n-28.4\t85.8\n-28.7\t86.1\n-29\t86.4\n-29.3\t86.7\n-29.6\t87\n-29.9\t87.3\n-30.2\t87.6\n-30.5\t87.9\n-30.8\t88.2\n-31.1\t88.5\n-31.4\t88.8\n-31.7\t89.1\n-32\t89.4\n-32.3\t89.7\n-32.6\t90\n-32.9\t90.3\n-33.2\t90.6\n-33.5\t90.9\n-33.8\t91.2\n-34.1\t91.5\n-34.4\t91.8\n-34.7\t92.1\n-35\t92.4\n-35.3\t92.7\n-35.6\t93\n-35.9\t93.3\n-36.2\t93.6\n-36.5\t93.9\n-36.8\t93.2\n-37.1\t92.5\n-37.4\t91.8\n-37.7\t91.1\n-38\t90.4\n-38.3\t89.7\n-38.6\t89\n-38.9\t88.3\n-39.2\t87.6\n-39.5\t86.9\n-39.8\t86.2\n-40.1\t85.5\n-40.4\t84.8\n-40.7\t84.1\n-41\t83.4\n-41.3\t82.7\n-41.6\t82\n-41.9\t81.3\n-42.2\t80.6\n-42.5\t79.9\n-42.8\t79.2\n-43.1\t78.5\n-43.4\t77.8\n-43.7\t77.1\n-44\t76.4\n-44.3\t75.7\n-44.6\t75\n-44.9\t74.3\n-45.2\t73.6\n-45.5\t72.9\n-45.8\t72.2\n-46.1\t71.5\n-46.4\t70.8\n-46.7\t70.1\n-47\t69.4\n-47.3\t68.7\n-47.6\t68\n-47.9\t67.3\n-48.2\t66.6\n-48.5\t65.9\n-48.8\t65.2\n-49.1\t64.5\n-49.4\t63.8\n-49.7\t63.1\n-50\t62.4\n-50.3\t61.7\n-50.6\t61\n-50.9\t60.3\n-51.2\t59.6\n-51.5\t58.9\n-51.8\t58.2\n-52.1\t57.5\n-52.4\t56.8\n-52.7\t56.1\n-53\t55.4\n-53.3\t54.7\n-53.6\t54\n-53.9\t53.3\n-54.2\t52.6\n-54.5\t51.9\n-54.8\t51.2\n-55.1\t50.5\n-55.4\t49.8\n-55.7\t49.1\n-56\t48.4\n-56.3\t47.7\n-56.6\t47\n-56.9\t46.3\n-57.2\t45.6\n-57.5\t44.9\n-57.8\t44.2\n-58.1\t43.5\n-58.4\t42.8\n-58.7\t42.1\n-59\t41.4\n-59.3\t40.7\n-59.6\t40\n-59.9\t39.3\n-60.2\t38.6\n-60.5\t37.9\n-60.8\t37.2\n-61.1\t36.5\n-61.4\t35.8\n-61.7\t35.1\n-62\t34.4\n-62.3\t33.7\n-62.6\t33\n-62.9\t32.3\n-63.2\t31.6\n-63.5\t30.9\n-63.8\t30.2\n-64.1\t29.5\n-64.4\t28.8\n-64.7\t28.1\n-65\t27.4\n-65.3\t26.7\n-65.6\t26\n-65.9\t25.3\n-66.2\t24.6\n-66.5\t23.9\n-66.8\t23.2\n-67.1\t22.5\n-67.4\t21.8\n-67.7\t21.1\n-68\t20.4\n-68.3\t19.7\n-68.6\t19\n-68.9\t18.3\n-69.2\t17.6\n-69.5\t16.9\n-69.8\t16.2\n-70.1\t15.5\n-70.4\t14.8\n-70.7\t14.1\n-71\t13.4\n-71.3\t12.7\n-71.6\t12\n-71.9\t11.3\n-72.2\t10.6\n-71.4\t9.9\n-70.6\t9.2\n-69.8\t8.5\n-69\t7.8\n-68.2\t7.1\n-67.4\t6.4\n-66.6\t5.7\n-65.8\t5\n-65\t4.3\n-64.2\t3.6\n-63.4\t2.9\n-62.6\t2.2\n-61.8\t1.5\n-61\t0.8\n-60.2\t0.1\n-59.4\t-0.6\n-58.6\t-1.3\n-57.8\t-2\n-57\t-2.7\n-56.2\t-3.4\n-55.4\t-4.1\n-54.6\t-4.8\n-53.8\t-5.5\n-53\t-6.2\n-52.2\t-6.9\n-51.4\t-7.6\n-50.6\t-8.3\n-49.8\t-9\n-49\t-9.7\n-48.2\t-10.4\n-47.4\t-11.1\n-46.6\t-11.8\n-45.8\t-12.5\n-45\t-13.2\n-44.2\t-13.9\n-43.4\t-14.6\n-42.6\t-15.3\n-41.8\t-16\n-41\t-16.7\n-40.2\t-17.4\n-39.4\t-18.1\n-38.6\t-18.8\n-37.8\t-19.5\n-37\t-20.2\n-36.2\t-20.9\n-35.4\t-21.6\n-34.6\t-22.3\n-33.8\t-23\n-33\t-23.7\n-32.2\t-24.4\n-31.4\t-25.1\n-30.6\t-25.8\n-29.8\t-26.5\n-29\t-27.2\n-28.2\t-27.9\n-27.4\t-28.6\n-26.6\t-29.3\n-25.8\t-30\n-25\t-30.7\n-24.2\t-31.4\n-23.4\t-32.1\n-22.6\t-32.8\n-21.8\t-33.5\n-21\t-34.2\n-20.2\t-34.9\n-19.4\t-35.6\n-18.6\t-36.3\n-17.8\t-37\n-17\t-37.7\n-16.2\t-38.4\n-15.4\t-39.1\n-14.6\t-39.8\n-13.8\t-40.5\n-13\t-41.2\n-12.2\t-41.9\n-11.4\t-42.6\n-10.6\t-43.3\n-9.8\t-44\n-9\t-44.7\n-8.2\t-45.4\n-7.4\t-46.1\n-6.6\t-46.8\n-5.8\t-47.5\n-5\t-48.2\n-4.2\t-48.9\n-3.4\t-49.6\n-2.6\t-50.3\n-1.8\t-51\n-1\t-51.7\n-0.2\t-52.4\n0.6\t-53.1\n1.4\t-53.8\n2.2\t-54.5\n3\t-55.2\n3.8\t-55.9\n4.6\t-56.6\n5.4\t-57.3\n6.2\t-58\n7\t-58.7\n7.8\t-59.4\n8.6\t-60.1\n9.4\t-60.8\n10.2\t-61.5\n11\t-62.2\n11.8\t-62.9\n12.6\t-63.6\n13.4\t-64.3\n14.2\t-65\n15\t-65.7\n15.8\t-66.4\n16.6\t-67.1\n17.4\t-67.8\n18.2\t-68.5\n19\t-69.2\n19.8\t-69.9\n20.6\t-70.6\n21.4\t-71.3\n22.2\t-72\n23\t-72.7\n23.8\t-73.4\n24.6\t-74.1\n25.4\t-74.8\n26.2\t-75.5\n27\t-75\n27.8\t-74.5\n28.6\t-74\n29.4\t-73.5\n30.2\t-73\n31\t-72.5\n31.8\t-72\n32.6\t-71.5\n33.4\t-71\n34.2\t-70.5\n35\t-70\n35.8\t-69.5\n36.6\t-69\n37.4\t-68.5\n38.2\t-68\n39\t-67.5\n39.8\t-67\n40.6\t-66.5\n41.4\t-66\n42.2\t-65.5\n43\t-65\n43.8\t-64.5\n44.6\t-64\n45.4\t-63.5\n46.2\t-63\n47\t-62.5\n47.8\t-62\n48.6\t-61.5\n49.4\t-61\n50.2\t-60.5\n51\t-60\n51.8\t-59.5\n52.6\t-59\n53.4\t-58.5\n54.2\t-58\n55\t-57.5\n55.8\t-57\n56.6\t-56.5\n57.4\t-56\n58.2\t-55.5\n59\t-55\n59.8\t-54.5\n60.6\t-54\n61.4\t-53.5\n62.2\t-53\n63\t-52.5\n63.8\t-52\n64.6\t-51.5\n65.4\t-51\n66.2\t-50.5\n67\t-50\n67.8\t-49.5\n68.6\t-49\n69.4\t-48.5\n70.2\t-48\n71\t-47.5\n71.8\t-47\n72.6\t-46.5\n73.4\t-46\n74.2\t-45.5\n75\t-45\n75.8\t-44.5\n76.6\t-44\n77.4\t-43.5\n78.2\t-43\n79\t-42.5\n79.8\t-42\n80.6\t-41.5\n81.4\t-41\n82.2\t-40.5\n83\t-40\n83.8\t-39.5\n84.6\t-39\n85.4\t-38.5\n86.2\t-38\n87\t-37.5\n87.8\t-37\n88.6\t-36.5\n89.4\t-36\n90.2\t-35.5\n91\t-35\n91.8\t-34.5\n92.6\t-34\n93.4\t-33.5\n94.2\t-33\n95\t-32.5\n95.8\t-32\n96.6\t-31.5\n97.4\t-31\n98.2\t-30.5\n99\t-30\n98.7\t-29.5\n98.4\t-29\n98.1\t-28.5\n97.8\t-28\n97.5\t-27.5\n97.2\t-27\n96.9\t-26.5\n96.6\t-26\n96.3\t-25.5\n96\t-25\n95.7\t-24.5\n95.4\t-24\n95.1\t-23.5\n94.8\t-23\n94.5\t-22.5\n94.2\t-22\n93.9\t-21.5\n93.6\t-21\n93.3\t-20.5\n93\t-20\n92.7\t-19.5\n92.4\t-19\n92.1\t-18.5\n91.8\t-18\n91.5\t-17.5\n91.2\t-17\n90.9\t-16.5\n90.6\t-16\n90.3\t-15.5\n90\t-15\n89.7\t-14.5\n89.4\t-14\n89.1\t-13.5\n88.8\t-13\n88.5\t-12.5\n88.2\t-12\n87.9\t-11.5\n87.6\t-11\n87.3\t-10.5\n87\t-10\n86.7\t-9.5\n86.4\t-9\n86.1\t-8.5\n85.8\t-8\n85.5\t-7.5\n85.2\t-7\n84.9\t-6.5\n84.6\t-6\n84.3\t-5.5\n84\t-5\n83.7\t-4.5\n83.4\t-4\n83.1\t-3.5\n82.8\t-3\n82.5\t-2.5\n82.2\t-2\n81.9\t-1.5\n81.6\t-1\n81.3\t-0.5\n81\t-2.74269E-12\n80.7\t0.5\n80.4\t1\n80.1\t1.5\n79.8\t2\n79.5\t2.5\n79.2\t3\n78.9\t3.5\n78.6\t4\n78.3\t4.5\n78\t5\n77.7\t5.5\n77.4\t6\n77.1\t6.5\n76.8\t7\n76.5\t7.5\n76.2\t8\n75.9\t8.5\n75.6\t9\n75.3\t9.5\n75\t10\n74.7\t10.5\n74.4\t11\n74.1\t11.5\n73.8\t12\n73.5\t12.5\n73.2\t13\n72.9\t13.5\n72.6\t14\n72.3\t14.5\n72\t15\n71.7\t15.5\n71.4\t16\n71.1\t16.5\n70.8\t17\n70.5\t17.5\n70.2\t18\n69.9\t18.5\n69.6\t19\n69.3\t19.5\n69\t20\n68.7\t20.5\n68.4\t21\n68.1\t21.5\n67.8\t22\n67.5\t22.5\n67.2\t23\n66.9\t23.5\n66.6\t24\n66.3\t24.5\n66\t25\n65.7\t25.5\n65.4\t26\n65.1\t26.5\n64.8\t27\n64.5\t27.5\n64.2\t28\n63.9\t28.5\n63.6\t29\n63.3\t29.5\n63\t30\n62.7\t30.5\n62.4\t31\n62.1\t31.5\n61.8\t32\n61.5\t32.5\n61.2\t33\n60.9\t33.5\n60.6\t34\n60.3\t34.5\n60\t35\n59.7\t35.5\n59.4\t36\n59.1\t35.8\n58.8\t35.6\n58.5\t35.4\n58.2\t35.2\n57.9\t35\n57.6\t34.8\n57.3\t34.6\n57\t34.4\n56.7\t34.2\n56.4\t34\n56.1\t33.8\n55.8\t33.6\n55.5\t33.4\n55.2\t33.2\n54.9\t33\n54.6\t32.8\n54.3\t32.6\n54\t32.4\n53.7\t32.2\n53.4\t32\n53.1\t31.8\n52.8\t31.6\n52.5\t31.4\n52.2\t31.2\n51.9\t31\n51.6\t30.8\n51.3\t30.6\n51\t30.4\n50.7\t30.2\n50.4\t30\n50.1\t29.8\n49.8\t29.6\n49.5\t29.4\n49.2\t29.2\n48.9\t29\n48.6\t28.8\n48.3\t28.6\n48\t28.4\n47.7\t28.2\n47.4\t28\n47.1\t27.8\n46.8\t27.6\n46.5\t27.4\n46.2\t27.2\n45.9\t27\n45.6\t26.8\n45.3\t26.6\n45\t26.4\n44.7\t26.2\n44.4\t26\n44.1\t25.8\n43.8\t25.6\n43.5\t25.4\n43.2\t25.2\n42.9\t25\n42.6\t24.8\n42.3\t24.6\n42\t24.4\n41.7\t24.2\n41.4\t24\n41.1\t23.8\n40.8\t23.6\n40.5\t23.4\n40.2\t23.2\n39.9\t23\n39.6\t22.8\n39.3\t22.6\n39\t22.4\n38.7\t22.2\n38.4\t22\n38.1\t21.8\n37.8\t21.6\n37.5\t21.4\n37.2\t21.2\n36.9\t21\n36.6\t20.8\n36.3\t20.6\n36\t20.4\n35.7\t20.2\n35.4\t20\n35.1\t19.8\n34.8\t19.6\n34.5\t19.4\n34.2\t19.2\n33.9\t19\n33.6\t18.8\n33.3\t18.6\n33\t18.4\n32.7\t18.2\n32.4\t18\n32.1\t17.8\n31.8\t17.6\n31.5\t17.4\n31.2\t17.2\n30.9\t17\n30.6\t16.8\n30.3\t16.6\n30\t16.4\n29.7\t16.2\n29.4\t16\n29.1\t15.8\n28.8\t15.6\n28.5\t15.4\n28.2\t15.2\n27.9\t15\n27.6\t14.8\n27.3\t14.6\n27\t14.4\n26.7\t14.2\n26.4\t14\n26.1\t13.8\n25.8\t13.6\n25.5\t13.4\n25.2\t13.2\n24.9\t13\n24.6\t12.8\n24.3\t12.6\n24\t12.4\n23.7\t12.2\n23.4\t12\n23.1\t11.8\n22.8\t11.6\n22.5\t11.4\n22.2\t11.2\n21.9\t11\n21.6\t10.8\n21.3\t10.6\n21\t10.4\n20.7\t10.2\n20.4\t10\n20.1\t9.8\n19.8\t9.6\n19.5\t9.4\n19.2\t9.2\n18.9\t9\n18.6\t8.8\n18.3\t8.6\n18\t8.4\n17.7\t8.2\n17.4\t8\n17.1\t7.8\n16.8\t7.6\n16.5\t7.4\n16.2\t7.2\n15.3\t7\n14.4\t6.8\n13.5\t6.6\n12.6\t6.4\n11.7\t6.2\n10.8\t6\n9.9\t5.8\n9\t5.6\n8.1\t5.4\n7.2\t5.2\n6.3\t5\n5.4\t4.8\n4.5\t4.6\n3.6\t4.4\n2.7\t4.2\n1.8\t4\n0.9\t3.8\n-2.06568E-12\t3.6\n-0.9\t3.4\n-1.8\t3.2\n-2.7\t3\n-3.6\t2.8\n-4.5\t2.6\n-5.4\t2.4\n-6.3\t2.2\n-7.2\t2\n-8.1\t1.8\n-9\t1.6\n-9.9\t1.4\n-10.8\t1.2\n-11.7\t1\n-12.6\t0.8\n-13.5\t0.6\n-14.4\t0.4\n-15.3\t0.2\n-16.2\t-2.71644E-12\n-17.1\t-0.2\n-18\t-0.4\n-18.9\t-0.6\n-19.8\t-0.8\n-20.7\t-1\n-21.6\t-1.2\n-22.5\t-1.4\n-23.4\t-1.6\n-24.3\t-1.8\n-25.2\t-2\n-26.1\t-2.2\n-27\t-2.4\n-27.9\t-2.6\n-28.8\t-2.8\n-29.7\t-3\n-30.6\t-3.2\n-31.5\t-3.4\n-32.4\t-3.6\n-33.3\t-3.8\n-34.2\t-4\n-35.1\t-4.2\n-36\t-4.4\n-36.9\t-4.6\n-37.8\t-4.8\n-38.7\t-5\n-39.6\t-5.2\n-40.5\t-5.4\n-41.4\t-5.6\n-42.3\t-5.8\n-43.2\t-6\n-44.1\t-6.2\n-45\t-6.4\n-45.9\t-6.6\n-46.8\t-6.8\n-47.7\t-7\n-48.6\t-7.2\n-49.5\t-7.4\n-50.4\t-7.6\n-51.3\t-7.8\n-52.2\t-8\n-53.1\t-8.2\n-54\t-8.4\n-54.9\t-8.6\n-55.8\t-8.8\n-56.7\t-9\n-57.6\t-9.2\n-58.5\t-9.4\n-59.4\t-9.6\n-60.3\t-9.8\n-61.2\t-10\n-62.1\t-10.2\n-63\t-10.4\n-63.9\t-10.6\n-64.8\t-10.8\n-65.7\t-11\n-66.6\t-11.2\n-67.5\t-11.4\n-68.4\t-11.6\n-69.3\t-11.8\n-70.2\t-12\n-71.1\t-12.2\n-72\t-12.4\n-72.9\t-12.6\n-73.8\t-12.8\n-74.7\t-13\n-75.6\t-13.2\n-76.5\t-13.4\n-77.4\t-13.6\n-78.3\t-13.8\n-79.2\t-14\n-80.1\t-14.2\n-81\t-14.4\n-81.9\t-14.6\n-82.8\t-14.8\n-83.7\t-15\n-83.3\t-15.2\n-82.9\t-15.4\n-82.5\t-15.6\n-82.1\t-15.8\n-81.7\t-16\n-81.3\t-16.2\n-80.9\t-16.4\n-80.5\t-16.6\n-80.1\t-16.8\n-79.7\t-17\n-79.3\t-17.2\n-78.9\t-17.4\n-78.5\t-17.6\n-78.1\t-17.8\n-77.7\t-18\n-77.3\t-18.2\n-76.9\t-18.4\n-76.5\t-18.6\n-76.1\t-18.8\n-75.7\t-19\n-75.3\t-19.2\n-74.9\t-19.4\n-74.5\t-19.6\n-74.1\t-19.8\n-73.7\t-20\n-73.3\t-20.2\n-72.9\t-20.4\n-72.5\t-20.6\n-72.1\t-20.8\n-71.7\t-21\n-71.3\t-21.2\n-70.9\t-21.4\n-70.5\t-21.6\n-70.1\t-21.8\n-69.7\t-22\n-69.3\t-22.2\n-68.9\t-22.4\n-68.5\t-22.6\n-68.1\t-22.8\n-67.7\t-23\n-67.3\t-23.2\n-66.9\t-23.4\n-66.5\t-23.6\n-66.1\t-23.8\n-65.7\t-24\n-65.3\t-24.2\n-64.9\t-24.4\n-64.5\t-24.6\n-64.1\t-24.8\n-63.7\t-25\n-63.3\t-25.2\n-62.9\t-25.4\n-62.5\t-25.6\n-62.1\t-25.8\n-61.7\t-26\n-61.3\t-26.2\n-60.9\t-26.4\n-60.5\t-26.6\n-60.1\t-26.8\n-59.7\t-27\n-59.3\t-27.2\n-58.9\t-27.4\n-58.5\t-27.6\n-58.1\t-27.8\n-57.7\t-28\n-57.3\t-28.2\n-56.9\t-28.4\n-56.5\t-28.6\n-56.1\t-28.8\n-55.7\t-29\n-55.3\t-29.2\n-54.9\t-29.4\n-54.5\t-29.6\n-54.1\t-29.8\n-53.7\t-30\n-53.3\t-30.2\n-52.9\t-30.4\n-52.5\t-30.6\n-52.1\t-30.8\n-51.7\t-31\n-51.3\t-31.2\n-50.9\t-31.4\n-50.5\t-31.6\n-50.1\t-31.8\n-49.7\t-32\n-49.3\t-32.2\n-48.9\t-32.4\n-48.5\t-32.6\n-48.1\t-32.8\n-47.7\t-33\n-47.3\t-33.2\n-46.9\t-33.4\n-46.5\t-33.6\n-46.1\t-33.8\n-45.7\t-34\n-45.3\t-34.2\n-44.9\t-34.4\n-44.5\t-34.6\n-44.1\t-34.8\n-43.7\t-35\n-43.3\t-35.2\n-42.9\t-35.4\n-42.5\t-35.6\n-42.1\t-35.8\n-41.7\t-36\n-41.3\t-36.2\n-41\t-36.4\n-40.7\t-36.6\n-40.4\t-36.8\n-40.1\t-37\n-39.8\t-37.2\n-39.5\t-37.4\n-39.2\t-37.6\n-38.9\t-37.8\n-38.6\t-38\n-38.3\t-38.2\n-38\t-38.4\n-37.7\t-38.6\n-37.4\t-38.8\n-37.1\t-39\n-36.8\t-39.2\n-36.5\t-39.4\n-36.2\t-39.6\n-35.9\t-39.8\n-35.6\t-40\n-35.3\t-40.2\n-35\t-40.4\n-34.7\t-40.6\n-34.4\t-40.8\n-34.1\t-41\n-33.8\t-41.2\n-33.5\t-41.4\n-33.2\t-41.6\n-32.9\t-41.8\n-32.6\t-42\n-32.3\t-42.2\n-32\t-42.4\n-31.7\t-42.6\n-31.4\t-42.8\n-31.1\t-43\n-30.8\t-43.2\n-30.5\t-43.4\n-30.2\t-43.6\n-29.9\t-43.8\n-29.6\t-44\n-29.3\t-44.2\n-29\t-44.4\n-28.7\t-44.6\n-28.4\t-44.8\n-28.1\t-45\n-27.8\t-45.2\n-27.5\t-45.4\n-27.2\t-45.6\n-26.9\t-45.8\n-26.6\t-46\n-26.3\t-46.2\n-26\t-46.4\n-25.7\t-46.6\n-25.4\t-46.8\n-25.1\t-47\n-24.8\t-47.2\n-24.5\t-47.4\n-24.2\t-47.6\n-23.9\t-47.8\n-23.6\t-48\n-23.3\t-48.2\n-23\t-48.4\n-22.7\t-48.6\n-22.4\t-48.8\n-22.1\t-49\n-21.8\t-49.2\n-21.5\t-49.4\n-21.2\t-49.6\n-20.9\t-49.8\n-20.6\t-50\n-20.3\t-50.2\n-20\t-50.4\n-19.7\t-50.6\n-19.4\t-50.8\n-19.1\t-51\n-18.8\t-51.2\n-18.5\t-51.4\n-18.2\t-51.6\n-17.9\t-51.8\n-17.6\t-52\n-17.3\t-52.2\n-17\t-52.4\n-16.7\t-52.6\n-16.4\t-52.8\n-16.1\t-53\n-15.8\t-53.2\n-15.5\t-53.4\n-15.2\t-53.6\n-14.9\t-53.8\n-14.6\t-54\n-14.3\t-54.2\n-14\t-54.4\n-13.7\t-54.6\n-13.4\t-54.8\n-13.1\t-55\n-12.8\t-55.2\n-12.5\t-55.4\n-12.2\t-55.6\n-11.9\t-55.8\n-11.6\t-56\n-11.3\t-56.2\n-11\t-56.4\n-10.7\t-56.6\n-10.4\t-56.8\n-10.1\t-57\n-9.8\t-57.2\n-9.5\t-57.4\n-9.2\t-57.6\n-8.9\t-57.8\n-8.6\t-58\n-8.3\t-58.2\n-8\t-58.4\n-7.7\t-58.6\n-7.4\t-58.8\n-7.1\t-59\n-6.8\t-59.2\n-6.5\t-59.4\n-6.2\t-59.6\n-5.9\t-59.8\n-5.6\t-60\n-5.3\t-60.2\n-5\t-60.4\n-4.7\t-60.6\n-4.4\t-60.8\n-4.1\t-61\n-3.8\t-61.2\n-3.5\t-61.4\n-3.2\t-61.6\n-2.9\t-61.8\n-2.6\t-62\n-2.3\t-62.2\n-2\t-62.4\n-1.7\t-62.6\n-1.4\t-62.8\n-1.1\t-63\n-0.8\t-63.2\n-0.5\t-63.4\n-0.2\t-63.6\n0.1\t-63.8\n0.4\t-64\n0.7\t-64.2\n1\t-64.4\n1.3\t-64.6\n1.6\t-64.8\n1.9\t-65\n2.2\t-65.2\n2.5\t-65.4\n2.8\t-65.6\n3.1\t-65.8\n3.4\t-66\n3.7\t-66.2\n4\t-66.4\n4.3\t-66.6\n4.6\t-66.8\n4.9\t-67\n5.2\t-67.2\n5.5\t-67.4\n5.8\t-67.6\n6.1\t-67.8\n6.4\t-68\n6.7\t-68.2\n7\t-68.4\n7.3\t-68.6\n7.6\t-68.8\n7.9\t-69\n8.2\t-69.2\n8.5\t-69.4\n8.8\t-69.6\n9.1\t-69.8\n9.4\t-70\n9.7\t-70.2\n10\t-70.4\n10.3\t-70.6\n10.6\t-70.8\n10.9\t-71\n11.2\t-71.2\n11.5\t-71.4\n11\t-71.6\n10.5\t-71.8\n10\t-72\n9.5\t-72.2\n9\t-72.4\n8.5\t-72.6\n8\t-72.8\n7.5\t-73\n7\t-73.2\n6.5\t-73.4\n6\t-73.6\n5.5\t-73.8\n5\t-74\n4.5\t-74.2\n4\t-74.4\n3.5\t-74.6\n3\t-74.8\n2.5\t-75\n2\t-75.2\n1.5\t-75.4\n1\t-75.6\n0.5\t-75.8\n-1.95222E-12\t-76\n-0.5\t-76.2\n-1\t-76.4\n-1.5\t-76.6\n-2\t-76.8\n-2.5\t-77\n-3\t-77.2\n-3.5\t-77.4\n-4\t-77.6\n-4.5\t-77.8\n-5\t-78\n-5.5\t-78.2\n-6\t-78.4\n-6.5\t-78.6\n-7\t-78.8\n-7.5\t-79\n-8\t-79.2\n-8.5\t-79.4\n-9\t-79.6\n-9.5\t-79.8\n-10\t-80\n-10.5\t-80.2\n-11\t-80.4\n-11.5\t-80.6\n-12\t-80.8\n-12.5\t-81\n-13\t-81.2\n-13.5\t-81.4\n-14\t-81.6\n-14.5\t-81.8\n-15\t-82\n-15.5\t-82.2\n-16\t-82.4\n-16.5\t-82.6\n-17\t-82.8\n-17.5\t-83\n-18\t-83.2\n-18.5\t-83.4\n-19\t-83.6\n-19.5\t-83.8\n-20\t-84\n-20.5\t-84.2\n-21\t-84.4\n-21.5\t-84.6\n-22\t-84.8\n-22.5\t-85\n-23\t-85.2\n-23.5\t-85.4\n-24\t-85.6\n-24.5\t-85.8\n-25\t-86\n-25.5\t-86.2\n-26\t-86.4\n-26.5\t-86.6\n-27\t-86.8\n-27.5\t-87\n-28\t-87.2\n-28.5\t-87.4\n-29\t-87.6\n-29.5\t-87.8\n-30\t-88\n-30.5\t-88.2\n-31\t-88.4\n-31.5\t-88.6\n-32\t-88.8\n-32.5\t-89\n-33\t-89.2\n-33.5\t-89.4\n-34\t-89.6\n-34.5\t-89.8\n-35\t-90\n-35.5\t-90.2\n-36\t-90.4\n-36.5\t-90.6\n-37\t-90.8\n-37.5\t-91\n-38\t-91.2\n-38.5\t-91.4\n-39\t-91.6\n-39.5\t-91.8\n-40\t-92\n-40.5\t-92.2\n-41\t-92.4\n-41.5\t-92.6\n-42\t-92.8\n-42.5\t-93\n-43\t-93.2\n-43.5\t-93.4\n-44\t-93.6\n-44.5\t-93.8\n-44\t-94\n-43.5\t-93.6\n-43\t-93.2\n-42.5\t-92.8\n-42\t-92.4\n-41.5\t-92\n-41\t-91.6\n-40.5\t-91.2\n-40\t-90.8\n-39.5\t-90.4\n-39\t-90\n-38.5\t-89.6\n-38\t-89.2\n-37.5\t-88.8\n-37\t-88.4\n-36.5\t-88\n-36\t-87.6\n-35.5\t-87.2\n-35\t-86.8\n-34.5\t-86.4\n-34\t-86\n-33.5\t-85.6\n-33\t-85.2\n-32.5\t-84.8\n-32\t-84.4\n-31.5\t-84\n-31\t-83.6\n-30.5\t-83.2\n-30\t-82.8\n-29.5\t-82.4\n-29\t-82\n-28.5\t-81.6\n-28\t-81.2\n-27.5\t-80.8\n-27\t-80.4\n-26.5\t-80\n-26\t-79.6\n-25.5\t-79.2\n-25\t-78.8\n-24.5\t-78.4\n-24\t-78\n-23.5\t-77.6\n-23\t-77.2\n-22.5\t-76.8\n-22\t-76.4\n-21.5\t-76\n-21\t-75.6\n-20.5\t-75.2\n-20\t-74.8\n-19.5\t-74.4\n-19\t-74\n-18.5\t-73.6\n-18\t-73.2\n-17.5\t-72.8\n-17\t-72.4\n-16.5\t-72\n-16\t-71.6\n-15.5\t-71.2\n-15\t-70.8\n-14.5\t-70.4\n-14\t-70\n-13.5\t-69.6\n-13\t-69.2\n-12.5\t-68.8\n-12\t-68.4\n-11.5\t-68\n-11\t-67.6\n-10.5\t-67.2\n-10\t-66.8\n-9.5\t-66.4\n-9\t-66\n-8.5\t-65.6\n-8\t-65.2\n-7.5\t-64.8\n-7\t-64.4\n-6.5\t-64\n-6\t-63.6\n-5.5\t-63.2\n-5\t-62.8\n-4.5\t-62.4\n-4\t-62\n-3.5\t-61.6\n-3\t-61.2\n-2.5\t-60.8\n-2\t-60.4\n-1.5\t-60\n-1\t-59.6\n-0.5\t-59.2\n0\t-58.8\n0\t-58.4\n-0.1\t-58\n-0.2\t-57.6\n-0.3\t-57.2\n-0.4\t-56.8\n-0.5\t-56.4\n-0.6\t-56\n-0.7\t-55.6\n-0.8\t-55.2\n-0.9\t-54.8\n-1\t-54.4\n-1.1\t-54\n-1.2\t-53.6\n-1.3\t-53.2\n-1.4\t-52.8\n-1.5\t-52.4\n-1.6\t-52\n-1.7\t-51.6\n-1.8\t-51.2\n-1.9\t-50.8\n-2\t-50.4\n-2.1\t-50\n-2.2\t-49.6\n-2.3\t-49.2\n-2.4\t-48.8\n-2.5\t-48.4\n-2.6\t-48\n-2.7\t-47.6\n-2.8\t-47.2\n-2.9\t-46.8\n-3\t-46.4\n-3.1\t-46\n-3.2\t-45.6\n-3.3\t-45.2\n-3.4\t-44.8\n-3.5\t-44.4\n-3.6\t-44\n-3.7\t-43.6\n-3.8\t-43.2\n-3.9\t-42.8\n-4\t-42.4\n-4.1\t-42\n-4.2\t-41.6\n-4.3\t-41.2\n-4.4\t-40.8\n-4.5\t-40.4\n-4.6\t-40\n-4.7\t-39.6\n-4.8\t-39.2\n-4.9\t-38.8\n-5\t-38.4\n-5.1\t-38\n-5.2\t-37.6\n-5.3\t-37.2\n-5.4\t-36.8\n-5.5\t-36.4\n-5.6\t-36\n-5.7\t-35.6\n-5.8\t-35.2\n-5.9\t-34.8\n-6\t-34.4\n-6.1\t-34\n-6.2\t-33.6\n-6.3\t-33.2\n-6.4\t-32.8\n-6.5\t-32.4\n-6.6\t-32\n-6.7\t-31.6\n-6.8\t-31.2\n-6.9\t-30.8\n-7\t-30.4\n-7.1\t-30\n-7.2\t-29.6\n-7.3\t-29.2\n-7.4\t-28.8\n-7.5\t-28.4\n-7.6\t-28\n-7.7\t-27.6\n-7.8\t-27.2\n-7.9\t-26.8\n-8\t-26.4\n-8.1\t-26\n-8.2\t-25.6\n-8.3\t-25.2\n-8.4\t-24.8\n-8.5\t-24.4\n-8.6\t-24\n-8.7\t-23.6\n-8.8\t-23.2\n-8.9\t-22.8\n-9\t-22.4\n-9.1\t-22\n-9.2\t-21.6\n-9.3\t-21.2\n-9.4\t-20.8\n-9.5\t-20.4\n-9.6\t-20\n-9.7\t-19.6\n-9.8\t-19.2\n-9.9\t-18.8\n-10\t-18.4\n-10.1\t-18\n-10.2\t-17.6\n-10.3\t-17.2\n-10.4\t-16.8\n-10.5\t-16.4\n-10.6\t-16\n-10.7\t-15.6\n-10.8\t-15.2\n-10.9\t-14.8\n-11\t-14.4\n-11.1\t-14\n-11.2\t-13.6\n-11.3\t-13.2\n-11.4\t-12.8\n-11.5\t-12.4\n-11.6\t-12\n-11.7\t-11.6\n-11.8\t-11.2\n-11.9\t-10.8\n-12\t-10.4\n-12.1\t-10\n-12.2\t-9.6\n-12.3\t-9.2\n-12.4\t-8.8\n-12.5\t-8.4\n-12.8\t-8\n-13.1\t-7.6\n-13.4\t-7.2\n-13.7\t-6.8\n-14\t-6.4\n-14.3\t-6\n-14.6\t-5.6\n-14.9\t-5.2\n-15.2\t-4.8\n-15.5\t-4.4\n-15.8\t-4\n-16.1\t-3.6\n-16.4\t-3.2\n-16.7\t-2.8\n-17\t-2.4\n-17.3\t-2\n-17.6\t-1.6\n-17.9\t-1.2\n-18.2\t-0.8\n-18.5\t-0.4\n-18.8\t0\n-19.1\t0\n-19.4\t0.3\n-19.7\t0.6\n-20\t0.9\n-20.3\t1.2\n-20.6\t1.5\n-20.9\t1.8\n-21.2\t2.1\n-21.5\t2.4\n-21.8\t2.7\n-22.1\t3\n-22.4\t3.3\n-22.7\t3.6\n-23\t3.9\n-23.3\t4.2\n-23.6\t4.5\n-23.9\t4.8\n-24.2\t5.1\n-24.5\t5.4\n-24.8\t5.7\n-25.1\t6\n-25.4\t6.3\n-25.7\t6.6\n-26\t6.9\n-26.3\t7.2\n-26.6\t7.5\n-26.9\t7.8\n-27.2\t8.1\n-27.5\t8.4\n-27.8\t8.7\n-28.1\t9\n-28.4\t9.3\n-28.7\t9.6\n-29\t9.9\n-29.3\t10.2\n-29.6\t10.5\n-29.9\t10.8\n-30.2\t11.1\n-30.5\t11.4\n-30.8\t11.7\n-31.1\t12\n-31.4\t12.3\n-31.7\t12.6\n-32\t12.9\n-32.3\t13.2\n-32.6\t13.5\n-32.9\t13.8\n-33.2\t14.1\n-33.5\t14.4\n-33.8\t14.7\n-34.1\t15\n-34.4\t15.3\n-34.7\t15.6\n-35\t15.9\n-35.3\t16.2\n-35.6\t16.5\n-35.9\t16.8\n-36.2\t17.1\n-36.5\t17.4\n-36.8\t17.7\n-37.1\t18\n-37.4\t18.3\n-37.7\t18.6\n-38\t18.9\n-38.3\t19.2\n-38.6\t19.5\n-38.9\t19.8\n-39.2\t20.1\n-39.5\t20.4\n-39.8\t20.7\n-40.1\t21\n-40.4\t21.3\n-40.7\t21.6\n-41\t21.9\n-41.3\t22.2\n-41.6\t22.5\n-41.9\t22.8\n-42.2\t23.1\n-42.5\t23.4\n-42.8\t23.7\n-43.1\t24\n-43.4\t24.3\n-43.7\t24.6\n-44\t24.9\n-44.3\t25.2\n-44.6\t25.5\n-44.9\t25.8\n-45.2\t26.1\n-45.5\t26.4\n-45.8\t26.7\n-46.1\t27\n-46.4\t27.3\n-46.7\t27.6\n-47\t27.9\n-47.3\t28.2\n-47.6\t28.5\n-47.9\t28.8\n-48.2\t29.1\n-48.5\t29.4\n-48.8\t29.7\n-49.1\t30\n-49.4\t30.3\n-49.7\t30.6\n-50\t30.9\n-50.3\t31.2\n-50.6\t31.5\n-50.9\t31.8\n-51.2\t32.1\n-51.5\t32.4\n-51.8\t32.7\n-52.1\t33\n-52.4\t33.3\n-52.7\t33.6\n-53\t33.9\n-53.3\t34.2\n-53.6\t34.5\n-53.9\t34.8\n-54.2\t35.1\n-54.5\t35.4\n-54.8\t35.7\n-55.1\t36\n-55.4\t36.3\n-55.7\t36.6\n-56\t36.9\n-56.3\t37.2\n-56.6\t37.5\n-56.9\t37.8\n-57.2\t38.1\n-57.5\t38.4\n-57.8\t38.7\n-58.1\t39\n-58.4\t39.3\n-58.7\t39.6\n-59\t39.9\n-59.3\t40.2\n-59.6\t40.5\n-59.9\t40.8\n-60.2\t41.1\n-60.5\t41.4\n-60.8\t41.7\n-61.1\t42\n-61.4\t42.3\n-61.7\t42.6\n-62\t42.9\n-62.3\t43.2\n-62.6\t43.5\n-62.9\t43.8\n-63.2\t44.1\n-63.5\t44.4\n-63.8\t44.7\n-64.1\t45\n-64.4\t45.3\n-64.7\t45.6\n-65\t45.9\n-65.3\t46.2\n-65.6\t46.5\n-65.9\t46.8\n-66.2\t47.1\n-66.5\t47.4\n-66.8\t47.7\n-67.1\t48\n-67.4\t48.3\n-67.7\t48.6\n-68\t48.9\n-68.3\t49.2\n-68.6\t49.5\n-68.9\t49.8\n-69.2\t50.1\n-69.5\t50.4\n-69.8\t50.7\n-70.1\t51\n-70.4\t51.3\n-70.7\t51.6\n-71\t51.9\n-71.3\t52.2\n-71.6\t52.5\n-71.9\t52.8\n-72.2\t53.1\n-72.5\t53.4\n-72.8\t53.7\n-73.1\t54\n-73.4\t54.3\n-73.7\t54.6\n-74\t54.9\n-74.3\t55.2\n-74.6\t55.5\n-74.9\t55.8\n-75.2\t56.1\n-75.5\t56.4\n-75.8\t56.7\n-76.1\t57\n-76.4\t57.3\n-76.7\t57.6\n-77\t57.9\n-77.3\t58.2\n-77.6\t58.5\n-77.9\t58.8\n-78.2\t59.1\n-78.5\t59.4\n-78.8\t59.7\n-79.1\t60\n-79.4\t60.3\n-79.7\t60.6\n-80\t60.9\n-80.3\t61.2\n-80.6\t61.5\n-80.9\t61.8\n-81.2\t62.1\n-81.5\t62.4\n-81.8\t62.7\n-82.1\t63\n-82.4\t63.3\n-82.7\t63.6\n-83\t63.9\n-83.3\t64.2\n-83.6\t64.5\n-83.9\t64.8\n-84.2\t65.1\n-84.5\t65.4\n-84.8\t65.7\n-85.1\t66\n-85.4\t66.3\n-85.7\t66.6\n-86\t66.9\n-86.3\t67.2\n-86.6\t67.5\n-86.9\t67.8\n-87.2\t68.1\n-87.5\t68.4\n-87.8\t68.7\n-88.1\t69\n-88.4\t69.3\n-88.7\t69.6\n-89\t69.9\n-88.4\t70.2\n-87.8\t70.5\n-87.2\t70.8\n-86.6\t71.1\n-86\t71.4\n-85.4\t71.7\n-84.8\t72\n-84.2\t72.3\n-83.6\t72.6\n-83\t72.9\n-82.4\t73.2\n-81.8\t73.5\n-81.2\t73.8\n-80.6\t74.1\n-80\t74.4\n-79.4\t74.7\n-78.8\t75\n-78.2\t75.3\n-77.6\t75.6\n-77\t75.9\n-76.4\t76.2\n-75.8\t76.5\n-75.2\t76.8\n-74.6\t77.1\n-74\t77.4\n-73.4\t77.7\n-72.8\t78\n-72.2\t78.3\n-71.6\t78.6\n-71\t78.9\n-70.4\t79.2\n-69.8\t79.5\n-69.2\t79.8\n-68.6\t80.1\n-68\t80.4\n-67.4\t80.7\n-66.8\t81\n-66.2\t81.3\n-65.6\t81.6\n-65\t81.9\n-64.4\t82.2\n-63.8\t82.5\n-63.2\t82.8\n-62.6\t83.1\n-62\t83.4\n-61.4\t83.7\n-60.8\t84\n-60.2\t84.3\n-59.6\t84.6\n-59\t84.9\n-58.4\t85.2\n-57.8\t85.5\n-57.2\t85.8\n-56.6\t86.1\n-56\t86.4\n-55.4\t86.7\n-54.8\t87\n-54.2\t87.3\n-53.6\t87.6\n-53\t87.9\n-52.4\t88.2\n-51.8\t88.5\n-51.2\t88.8\n-50.6\t89.1\n-50\t89.4\n-49.4\t89.7\n-48.8\t90\n-48.2\t90.3\n-47.6\t90.6\n-47\t90.9\n-46.4\t91.2\n-45.8\t91.5\n-45.2\t91.8\n-44.6\t92.1\n-44\t92.4\n-43.4\t92.7\n-42.8\t93\n-42.2\t93.3\n-41.6\t93.6\n-41\t93.9\n-40.4\t94.2\n-39.8\t94.5\n-39.2\t94.8\n-38.6\t95.1\n-38\t95.4\n-37.4\t95.7\n-36.8\t96\n-36.2\t96.3\n-35.6\t96.6\n-35\t96.9\n-34.4\t97.2\n-33.8\t97.5\n-33.2\t97.3\n-32.6\t97.1\n-32\t96.9\n-31.4\t96.7\n-30.8\t96.5\n-30.2\t96.3\n-29.6\t96.1\n-29\t95.9\n-28.4\t95.7\n-27.8\t95.5\n-27.2\t95.3\n-26.6\t95.1\n-26\t94.9\n-25.4\t94.7\n-24.8\t94.5\n-24.2\t94.3\n-23.6\t94.1\n-23\t93.9\n-22.4\t93.7\n-21.8\t93.5\n-21.2\t93.3\n-20.6\t93.1\n-20\t92.9\n-19.4\t92.7\n-18.8\t92.5\n-18.2\t92.3\n-17.6\t92.1\n-17\t91.9\n-16.4\t91.7\n-15.8\t91.5\n-15.2\t91.3\n-14.6\t91.1\n-14\t90.9\n-13.4\t90.7\n-12.8\t90.5\n-12.2\t90.3\n-11.6\t90.1\n-11\t89.9\n-10.4\t89.7\n-9.8\t89.5\n-9.2\t89.3\n-8.6\t89.1\n-8\t88.9\n-7.4\t88.7\n-6.8\t88.5\n-6.2\t88.3\n-5.6\t88.1\n-5\t87.9\n-4.4\t87.7\n-3.8\t87.5\n-3.2\t87.3\n-2.6\t87.1\n-2\t86.9\n-1.4\t86.7\n-0.8\t86.5\n-0.2\t86.3\n0.4\t86.1\n1\t85.9\n1.6\t85.7\n2.2\t85.5\n2.8\t85.3\n3.4\t85.1\n4\t84.9\n4.6\t84.7\n5.2\t84.5\n5.8\t84.3\n6.4\t84.1\n7\t83.9\n7.6\t83.7\n8.2\t83.5\n8.8\t83.3\n9.4\t83.1\n10\t82.9\n10.6\t82.7\n11.2\t82.5\n11.8\t82.3\n12.4\t82.1\n13\t81.9\n13.6\t81.7\n14.2\t81.5\n14.8\t81.3\n15.4\t81.1\n16\t80.9\n16.6\t80.7\n17.2\t80.5\n17.8\t80.3\n18.4\t80.1\n19\t79.9\n19.6\t79.7\n20.2\t79.5\n20.8\t79.3\n21.4\t79.1\n22\t78.9\n22.6\t78.7\n23.2\t78.5\n23.8\t78.3\n24.4\t78.1\n25\t77.9\n25.6\t77.7\n26.2\t77.5\n26.8\t77.3\n27.4\t77.1\n28\t76.9\n28.6\t76.7\n29.2\t76.5\n29.8\t76.3\n30.4\t76.1\n31\t75.9\n31.6\t75.7\n32.2\t75.5\n32.8\t75.3\n33.4\t75.1\n34\t74.9\n34.6\t74.7\n35.2\t74.5\n35.8\t74.3\n36.4\t74.1\n37\t73.9\n37.6\t73.7\n38.2\t73.5\n38.8\t73.3\n39.4\t73.1\n40\t72.9\n40.6\t72.7\n41.2\t72.5\n41.8\t72.3\n42.4\t72.1\n43\t71.9\n43.6\t71.7\n44.2\t71.5\n44.8\t71.3\n45.4\t71.1\n46\t70.9\n46.6\t70.7\n47.2\t70.5\n47.8\t70.3\n48.4\t70.1\n49\t69.9\n49.6\t69.7\n50.2\t69.5\n50.8\t69.3\n51.4\t69.1\n52\t68.9\n52.6\t68.7\n53.2\t68.5\n53.8\t68.3\n54.4\t68.1\n55\t67.9\n55.6\t67.7\n56.2\t67.5\n56.8\t67.3\n57.4\t67.1\n58\t66.9\n58.6\t66.7\n59.2\t66.5\n59.8\t66.3\n60.4\t66.1\n61\t65.9\n61.6\t65.7\n62.2\t65.5\n62.8\t65.3\n63.4\t65.1\n64\t64.9\n64.6\t64.7\n65.2\t64.5\n65.8\t64.3\n66.4\t64.1\n67\t63.9\n67.6\t63.7\n68.2\t63.5\n68.8\t63.3\n69.4\t63.1\n70\t62.9\n70.6\t62.7\n71.2\t62.5\n71.8\t62.3\n72.4\t62.1\n73\t61.9\n73.6\t61.7\n74.2\t61.5\n74.8\t61.3\n75.4\t61.1\n76\t60.9\n76.6\t60.7\n77.2\t60.5\n77.8\t60.3\n78.4\t60.1\n79\t59.9\n79.6\t59.7\n80.2\t59.5\n80.8\t59.3\n81.4\t59.1\n82\t58.9\n82.6\t58.7\n83.2\t58.5\n83.8\t58.3\n84.4\t58.1\n84\t57.9\n83.6\t57.7\n83.2\t57.5\n82.8\t57.3\n82.4\t57.1\n82\t56.9\n81.6\t56.7\n81.2\t56.5\n80.8\t56.3\n80.4\t56.1\n80\t55.9\n79.6\t55.7\n79.2\t55.5\n78.8\t55.3\n78.4\t55.1\n78\t54.9\n77.6\t54.7\n77.2\t54.5\n76.8\t54.3\n76.4\t54.1\n76\t53.9\n75.6\t53.7\n75.2\t53.5\n74.8\t53.3\n74.4\t53.1\n74\t52.9\n73.6\t52.7\n73.2\t52.5\n72.8\t52.3\n72.4\t52.1\n72\t51.9\n71.6\t51.7\n71.2\t51.5\n70.8\t51.3\n70.4\t51.1\n70\t50.9\n69.6\t50.7\n69.2\t50.5\n68.8\t50.3\n68.4\t50.1\n68\t49.9\n67.6\t49.7\n67.2\t49.5\n66.8\t49.3\n66.4\t49.1\n66\t48.9\n65.6\t48.7\n65.2\t48.5\n64.8\t48.3\n64.4\t48.1\n64\t47.9\n63.6\t47.7\n63.2\t47.5\n62.8\t47.3\n62.4\t47.1\n62\t46.9\n61.6\t46.7\n61.2\t46.5\n60.8\t46.3\n60.4\t46.1\n60\t45.9\n59.6\t45.7\n59.2\t45.5\n58.8\t45.3\n58.4\t45.1\n58\t44.9\n57.6\t44.7\n57.2\t44.5\n56.8\t44.3\n56.4\t44.1\n56\t43.9\n55.6\t43.7\n55.2\t43.5\n54.8\t43.3\n54.4\t43.1\n54\t42.9\n53.6\t42.7\n53.2\t42.5\n52.8\t42.3\n52.4\t42.1\n52\t41.9\n51.6\t41.7\n51.2\t41.5\n50.8\t41.3\n50.4\t41.1\n50\t40.9\n49.6\t40.7\n49.2\t40.5\n48.8\t40.3\n48.4\t40.1\n48\t39.9\n47.6\t39.7\n47.2\t39.5\n46.8\t39.3\n46.4\t39.1\n46\t38.9\n45.6\t38.7\n45.2\t38.5\n44.8\t38.3\n44.4\t38.1\n44\t37.9\n43.6\t37.7\n43.2\t37.5\n42.8\t37.3\n42.4\t37.1\n42\t36.9\n41.6\t36.7\n41.2\t36.5\n40.8\t36.3\n40.4\t36.1\n40\t35.9\n39.6\t35.7\n39.2\t35.5\n38.8\t35.3\n38.4\t35.1\n38\t34.9\n37.6\t34.7\n37.2\t34.5\n36.8\t34.3\n36.4\t34.1\n36\t33.9\n35.6\t33.7\n35.2\t33.5\n34.8\t33.3\n34.4\t33.1\n34\t32.9\n33.6\t32.7\n33.2\t32.5\n32.8\t32.3\n32.4\t32.1\n32\t31.9\n31.6\t31.7\n31.2\t31.5\n30.8\t31.3\n30.4\t31.1\n30\t30.9\n29.6\t30.7\n29.2\t30.5\n28.8\t30.3\n28.4\t30.1\n28\t29.9\n27.6\t29.7\n27.2\t29.5\n26.8\t29.3\n26.4\t29.1\n26\t28.9\n25.6\t28.7\n25.2\t28.5\n24.8\t28.3\n24.4\t28.1\n24\t27.9\n23.6\t27.7\n23.2\t27.5\n22.8\t27.3\n22.4\t27.1\n22\t26.9\n21.6\t26.7\n21.2\t26.5\n20.8\t26.3\n20.4\t26.1\n20\t25.9\n19.6\t25.7\n19.2\t25.5\n18.8\t25.3\n18.4\t25.1\n18\t24.9\n17.6\t24.7\n17.2\t24.5\n16.8\t24.3\n16.4\t24.1\n16\t23.9\n15.6\t23.7\n15.2\t23.5\n14.8\t23.3\n14.4\t23.1\n14\t22.9\n13.6\t22.7\n13.2\t22.5\n12.8\t22.3\n12.4\t22.1\n12\t21.9\n11.6\t21.7\n11.2\t21.5\n10.8\t21.3\n10.4\t21.1\n10\t20.9\n9.6\t20.7\n9.2\t20.5\n8.8\t20.3\n8.4\t20.1\n8\t19.9\n7.6\t19.7\n7.2\t19.5\n6.8\t19.3\n6.4\t19.1\n6\t18.9\n5.6\t18.7\n5.2\t18.5\n4.8\t18.3\n4.4\t18.1\n4\t17.9\n3.6\t17.7\n3.2\t17.5\n2.8\t17.3\n2.4\t17.1\n2\t16.9\n1.6\t16.7\n1.2\t16.5\n0.8\t16.3\n0.4\t16.1\n1.74638E-13\t15.9\n-0.4\t15.7\n-0.8\t15.5\n-1.2\t15.3\n-1.6\t15.1\n-2\t14.9\n-2.4\t14.7\n-2.8\t14.5\n-3.2\t14.3\n-3.6\t14.1\n-4\t13.9\n-4.4\t13.7\n-4.8\t13.5\n-5.2\t13.3\n-5.6\t13.1\n-6\t12.9\n-6.4\t12.7\n-6.8\t12.5\n-7.2\t12.3\n-7.6\t12.1\n-8\t11.9\n-8.4\t11.7\n-8.8\t11.5\n-9.2\t11.3\n-9.6\t11.1\n-10\t10.9\n-10.4\t10.7\n-10.8\t11.3\n-11.2\t11.9\n-11.6\t12.5\n-12\t13.1\n-12.4\t13.7\n-12.8\t14.3\n-13.2\t14.9\n-13.6\t15.5\n-14\t16.1\n-14.4\t16.7\n-14.8\t17.3\n-15.2\t17.9\n-15.6\t18.5\n-16\t19.1\n-16.4\t19.7\n-16.8\t20.3\n-17.2\t20.9\n-17.6\t21.5\n-18\t22.1\n-18.4\t22.7\n-18.8\t23.3\n-19.2\t23.9\n-19.6\t24.5\n-20\t25.1\n-20.4\t25.7\n-20.8\t26.3\n-21.2\t26.9\n-21.6\t27.5\n-22\t28.1\n-22.4\t28.7\n-22.8\t29.3\n-23.2\t29.9\n-23.6\t30.5\n-24\t31.1\n-24.4\t31.7\n-24.8\t32.3\n-25.2\t32.9\n-25.6\t33.5\n-26\t34.1\n-26.4\t34.7\n-26.8\t35.3\n-27.2\t35.9\n-27.6\t36.5\n-28\t37.1\n-28.4\t37.7\n-28.8\t38.3\n-29.2\t38.9\n-29.6\t39.5\n-30\t40.1\n-30.4\t40.7\n-30.8\t41.3\n-31.2\t41.9\n-31.6\t42.5\n-32\t43.1\n-32.4\t43.7\n-32.8\t44.3\n-33.2\t44.9\n-33.6\t45.5\n-34\t46.1\n-34.4\t46.7\n-34.8\t47.3\n-35.2\t47.9\n-35.6\t48.5\n-36\t49.1\n-36.4\t49.7\n-36.8\t50.3\n-37.2\t50.9\n-37.6\t51.5\n-38\t52.1\n-38.4\t52.7\n-38.8\t53.3\n-39.2\t53.9\n-39.6\t54.5\n-40\t55.1\n-40.4\t55.7\n-40.8\t56.3\n-41.2\t56.9\n-41.6\t57.5\n-42\t58.1\n-42.4\t58.7\n-42.8\t59.3\n-43.2\t59.9\n-43.6\t60.5\n-44\t61.1\n-44.4\t61.7\n-44.8\t62.3\n-45.2\t62.9\n-45.6\t63.5\n-46\t64.1\n-46.4\t64.7\n-46.8\t65.3\n-47.2\t65.9\n-47.6\t66.5\n-48\t67.1\n-48.4\t67.7\n-48.8\t68.3\n-49.2\t68.9\n-49.6\t69.5\n-50\t70.1\n-50.4\t70.7\n-50.8\t71.3\n-51.2\t71.9\n-51.6\t72.5\n-52\t73.1\n-52.4\t73.7\n-52.8\t74.3\n-53.2\t74.9\n-53.6\t75.5\n-54\t76.1\n-54.4\t76.7\n-54.8\t77.3\n-55.2\t77.9\n-55.6\t78.5\n-56\t79.1\n-56.4\t79.7\n-56.8\t80.3\n-57.2\t80.9\n-57.6\t81.5\n-58\t82.1\n-58.4\t82.7\n-58.8\t83.3\n-59.2\t83.9\n-59.6\t84.5\n-60\t85.1\n-60.4\t85.7\n-60.8\t86.3\n-61.2\t86.9\n-61.6\t87.5\n-62\t88.1\n-62.4\t88.7\n-62.8\t89.3\n-63.2\t89.9\n-63.6\t90.5\n-64\t91.1\n-64.4\t91.7\n-64.8\t92.3\n-65.2\t92.9\n-65.6\t93.5\n-66\t94.1\n-66.4\t93.8\n-66.8\t93.5\n-67.2\t93.2\n-67.6\t92.9\n-68\t92.6\n-68.4\t92.3\n-68.8\t92\n-69.2\t91.7\n-69.6\t91.4\n-70\t91.1\n-70.4\t90.8\n-70.8\t90.5\n-71.2\t90.2\n-71.6\t89.9\n-72\t89.6\n-72.4\t89.3\n-72.8\t89\n-73.2\t88.7\n-73.6\t88.4\n-74\t88.1\n-74.4\t87.8\n-74.8\t87.5\n-75.2\t87.2\n-75.6\t86.9\n-76\t86.6\n-76.4\t86.3\n-76.8\t86\n-77.2\t85.7\n-77.6\t85.4\n-78\t85.1\n-78.4\t84.8\n-78.8\t84.5\n-79.2\t84.2\n-79.6\t83.9\n-80\t83.6\n-80.4\t83.3\n-80.8\t83\n-81.2\t82.7\n-81.6\t82.4\n-82\t82.1\n-82.4\t81.8\n-82.8\t81.5\n-83.2\t81.2\n-83.6\t80.9\n-84\t80.6\n-84.4\t80.3\n-84.8\t80\n-85.2\t79.7\n-85.6\t79.4\n-86\t79.1\n-86.4\t78.8\n-86.8\t78.5\n-87.2\t78.2\n-87.6\t77.9\n-88\t77.6\n-88.4\t77.3\n-88.8\t77\n-89.2\t76.7\n-89.6\t76.4\n-90\t76.1\n-90.4\t75.8\n-90.8\t75.5\n-91.2\t75.2\n-91.6\t74.9\n-92\t74.6\n-92.4\t74.3\n-92.3\t74\n-92.2\t73.7\n-92.1\t73.4\n-92\t73.1\n-91.9\t72.8\n-91.8\t72.5\n-91.7\t72.2\n-91.6\t71.9\n-91.5\t71.6\n-91.4\t71.3\n-91.3\t71\n-91.2\t70.7\n-91.1\t70.4\n-91\t70.1\n-90.9\t69.8\n-90.8\t69.5\n-90.7\t69.2\n-90.6\t68.9\n-90.5\t68.6\n-90.4\t68.3\n-90.3\t68\n-90.2\t67.7\n-90.1\t67.4\n-90\t67.1\n-89.9\t66.8\n-89.8\t66.5\n-89.7\t66.2\n-89.6\t65.9\n-89.5\t65.6\n-89.4\t65.3\n-89.3\t65\n-89.2\t64.7\n-89.1\t64.4\n-89\t64.1\n-88.9\t63.8\n-88.8\t63.5\n-88.7\t63.2\n-88.6\t62.9\n-88.5\t62.6\n-88.4\t62.3\n-88.3\t62\n-88.2\t61.7\n-88.1\t61.4\n-88\t61.1\n-87.9\t60.8\n-87.8\t60.5\n-87.7\t60.2\n-87.6\t59.9\n-87.5\t59.6\n-87.4\t59.3\n-87.3\t59\n-87.2\t58.7\n-87.1\t58.4\n-87\t58.1\n-86.9\t57.8\n-86.8\t57.5\n-86.7\t57.2\n-86.6\t56.9\n-86.5\t56.6\n-86.4\t56.3\n-86.3\t56\n-86.2\t55.7\n-86.1\t55.4\n-86\t55.1\n-85.9\t54.8\n-85.8\t54.5\n-85.7\t54.2\n-85.6\t53.9\n-85.5\t53.6\n-85.4\t53.3\n-85.3\t53\n-85.2\t52.7\n-85.1\t52.4\n-85\t52.1\n-84.9\t51.8\n-84.8\t51.5\n-84.7\t51.2\n-84.6\t50.9\n-84.5\t50.6\n-84.4\t50.3\n-84.3\t50\n-84.2\t49.7\n-84.1\t49.4\n-84\t49.1\n-83.9\t48.8\n-83.8\t48.5\n-83.7\t48.2\n-83.6\t47.9\n-83.5\t47.6\n-83.4\t47.3\n-83.3\t47\n-83.2\t46.7\n-83.1\t46.4\n-83\t46.1\n-82.9\t45.8\n-82.8\t45.5\n-82.7\t45.2\n-82.6\t44.9\n-82.5\t44.6\n-82.4\t44.3\n-82.3\t44\n-82.2\t43.7\n-82.1\t43.4\n-82\t43.1\n-81.9\t42.8\n-81.8\t42.5\n-81.7\t42.2\n-81.6\t41.9\n-81.5\t41.6\n-81.4\t41.3\n-81.3\t41\n-81.2\t40.7\n-81.1\t40.4\n-81\t40.1\n-80.9\t39.8\n-80.8\t39.5\n-80.7\t39.2\n-80.6\t38.9\n-80.5\t38.6\n-80.4\t38.3\n-80.3\t38\n-80.2\t37.7\n-80.1\t37.4\n-80\t37.1\n-79.9\t36.8\n-79.8\t36.5\n-79.7\t36.2\n-79.6\t35.9\n-79.5\t35.6\n-79.4\t35.3\n-79.3\t35\n-79.2\t34.7\n-79.1\t34.4\n-79\t34.1\n-78.9\t33.8\n-78.8\t33.5\n-78.7\t33.2\n-78.6\t32.9\n-78.5\t32.6\n-78.4\t32.3\n-78.3\t32\n-78.2\t31.7\n-78.1\t31.4\n-78\t31.1\n-77.9\t30.8\n-77.8\t30.5\n-77.7\t30.2\n-77.6\t29.9\n-77.5\t29.6\n-77.4\t29.3\n-77.3\t29\n-77.2\t28.7\n-77.1\t28.4\n-77\t28.1\n-76.9\t27.8\n-76.8\t27.5\n-76.7\t27.2\n-76.6\t26.9\n-76.5\t26.6\n-76.4\t26.3\n-76.3\t26\n-76.2\t25.7\n-76.1\t25.4\n-76\t25.1\n-75.9\t24.8\n-75.8\t24.5\n-75.7\t24.2\n-75.6\t23.9\n-75.5\t23.6\n-75.4\t23.3\n-75.3\t23\n-75.2\t22.7\n-75.1\t22.4\n-75\t22.1\n-74.9\t21.8\n-74.8\t21.5\n-74.7\t21.2\n-74.6\t20.9\n-74.5\t20.6\n-74.4\t20.3\n-74.3\t20\n-74.2\t19.7\n-74.1\t19.4\n-74\t19.1\n-73.9\t18.8\n-73.8\t18.5\n-73.7\t18.2\n-73.6\t17.9\n-73.5\t17.6\n-73.4\t17.3\n-73.3\t17\n-73.2\t16.7\n-73.1\t16.4\n-73\t16.1\n-72.9\t15.8\n-72.8\t15.5\n-72.7\t15.2\n-72.6\t14.9\n-72.5\t14.6\n-72.4\t14.3\n-72.3\t14\n-72.2\t13.7\n-72.1\t13.4\n-72\t13.1\n-71.9\t12.8\n-71.8\t12.5\n-71.7\t12.2\n-71.6\t11.9\n-71.5\t11.6\n-71.4\t11.3\n-71.3\t11\n-71.2\t10.7\n-71.1\t10.4\n-71\t10.1\n-70.9\t9.8\n-70.8\t9.5\n-70.7\t9.2\n-70.6\t8.9\n-70.5\t8.6\n-70.4\t8.3\n-70.3\t8\n-70.2\t7.7\n-70.1\t7.4\n-70\t7.1\n-69.9\t6.8\n-69.8\t6.5\n-69.7\t6.2\n-69.6\t5.9\n-69.5\t5.6\n-69.4\t5.3\n-69.3\t5\n-69.2\t4.7\n-69.1\t4.4\n-69\t4.1\n-68.9\t3.8\n-68.8\t3.5\n-68.7\t3.2\n-68.6\t2.9\n-68.5\t2.6\n-68.4\t2.3\n-68.3\t2\n-68.2\t1.7\n-68.1\t1.4\n-68\t1.1\n-67.9\t0.8\n-67.8\t0.5\n-67.7\t0.2\n-67.6\t-0.1\n-67.5\t-0.4\n-67.4\t-0.7\n-67.3\t-1\n-67.2\t-1.3\n-67.1\t-1.6\n-67\t-1.9\n-66.9\t-2.2\n-66.8\t-2.5\n-66.7\t-2.8\n-66.6\t-3.1\n-66.5\t-3.4\n-66.4\t-3.7\n-66.3\t-4\n-66.2\t-4.3\n-66.1\t-4.6\n-66\t-4.9\n-65.9\t-5.2\n-65.8\t-5.5\n-65.7\t-5.8\n-65.6\t-6.1\n-65.5\t-6.4\n-65.4\t-6.7\n-65.3\t-7\n-65.2\t-7.3\n-65.1\t-7.6\n-65\t-7.9\n-64.9\t-8.2\n-64.8\t-8.5\n-64.7\t-8.8\n-64.6\t-9.1\n-64.5\t-9.4\n-64.4\t-9.7\n-64.3\t-10\n-64.2\t-10.3\n-64.1\t-10.6\n-64\t-10.9\n-63.9\t-11.2\n-63.8\t-11.5\n-63.7\t-11.8\n-63.6\t-12.1\n-63.5\t-12.4\n-63.4\t-12.7\n-63.3\t-13\n-63.2\t-13.3\n-63.1\t-13.6\n-63\t-13.9\n-62.9\t-14.2\n-62.8\t-14.5\n-62.7\t-14.8\n-62.6\t-15.1\n-62.5\t-15.4\n-62.4\t-15.7\n-62.3\t-16\n-62.2\t-16.3\n-62.1\t-16.6\n-62\t-16.9\n-61.9\t-17.2\n-61.8\t-17.5\n-61.7\t-17.8\n-61\t-18.1\n-60.3\t-18.4\n-59.6\t-18.7\n-58.9\t-19\n-58.2\t-19.3\n-57.5\t-19.6\n-56.8\t-19.9\n-56.1\t-20.2\n-55.4\t-20.5\n-54.7\t-20.8\n-54\t-21.1\n-53.3\t-21.4\n-52.6\t-21.7\n-51.9\t-22\n-51.2\t-22.3\n-50.5\t-22.6\n-49.8\t-22.9\n-49.1\t-23.2\n-48.4\t-23.5\n-47.7\t-23.8\n-47\t-24.1\n-46.3\t-24.4\n-45.6\t-24.7\n-44.9\t-25\n-44.2\t-25.3\n-43.5\t-25.6\n-42.8\t-25.9\n-42.1\t-26.2\n-41.4\t-26.5\n-40.7\t-26.8\n-40\t-27.1\n-39.3\t-27.4\n-38.6\t-27.7\n-37.9\t-28\n-37.2\t-28.3\n-36.5\t-28.6\n-35.8\t-28.9\n-35.1\t-29.2\n-34.4\t-29.5\n-33.7\t-29.8\n-33\t-30.1\n-32.3\t-30.4\n-31.6\t-30.7\n-30.9\t-31\n-30.2\t-31.3\n-29.5\t-31.6\n-28.8\t-31.9\n-28.1\t-32.2\n-27.4\t-32.5\n-26.7\t-32.8\n-26\t-33.1\n-25.3\t-33.4\n-24.6\t-33.7\n-23.9\t-34\n-23.2\t-34.3\n-22.5\t-34.6\n-21.8\t-34.9\n-21.1\t-35.2\n-20.4\t-35.5\n-19.7\t-35.8\n-19\t-36.1\n-18.3\t-36.4\n-17.6\t-36.7\n-16.9\t-37\n-16.2\t-37.3\n-15.5\t-37.6\n-14.8\t-37.9\n-14.1\t-38.2\n-13.4\t-38.5\n-12.7\t-38.8\n-12\t-39.1\n-11.3\t-39.4\n-10.6\t-39.7\n-9.9\t-40\n-9.2\t-40.3\n-8.5\t-40.6\n-7.8\t-40.9\n-7.1\t-41.2\n-6.4\t-41.5\n-5.7\t-41.8\n-5\t-42.1\n-4.3\t-42.4\n-3.6\t-42.7\n-2.9\t-43\n-2.2\t-43.3\n-1.5\t-43.6\n-0.8\t-43.9\n-0.1\t-44.2\n0.6\t-44.5\n1.3\t-44.8\n2\t-45.1\n2.7\t-45.4\n3.4\t-45.7\n4.1\t-46\n4.8\t-46.3\n5.5\t-46.6\n6.2\t-46.9\n6.9\t-47.2\n7.6\t-47.5\n8.3\t-47.8\n9\t-48.1\n9.7\t-48.4\n10.4\t-48.7\n11.1\t-49\n11.8\t-49.3\n12.5\t-49.6\n13.2\t-49.9\n13.9\t-50.2\n14.6\t-50.5\n15.3\t-50.8\n16\t-51.1\n16.7\t-51.4\n17.4\t-51.7\n18.1\t-52\n18.8\t-52.3\n19.5\t-52.6\n20.2\t-52.9\n20.9\t-53.2\n21.6\t-53.5\n22.3\t-53.8\n23\t-54.1\n23.7\t-54.4\n24.4\t-54.7\n25.1\t-55\n25.8\t-55.3\n26.5\t-55.6\n27.2\t-55.9\n27.9\t-56.2\n28.6\t-56.5\n29.3\t-56.8\n30\t-57.1\n30.7\t-57.4\n31.4\t-57.7\n32.1\t-58\n32.8\t-58.3\n33.5\t-58.6\n34.2\t-58.9\n34.9\t-59.2\n35.6\t-59.5\n36.3\t-59.8\n37\t-60.1\n37.7\t-60.4\n38.4\t-60.7\n39.1\t-61\n39.8\t-61.3\n40.5\t-61.6\n41.2\t-61.9\n41.9\t-62.2\n42.6\t-62.5\n43.3\t-62.8\n44\t-63.1\n44.7\t-63.4\n45.4\t-63.7\n46.1\t-64\n46.8\t-64.3\n47.5\t-64.6\n48.2\t-64.9\n48.9\t-65.2\n49.6\t-65.5\n50.3\t-65.8\n51\t-66.1\n51.7\t-66.4\n52.4\t-65.8\n53.1\t-65.2\n53.8\t-64.6\n54.5\t-64\n55.2\t-63.4\n55.9\t-62.8\n56.6\t-62.2\n57.3\t-61.6\n58\t-61\n58.7\t-60.4\n59.4\t-59.8\n60.1\t-59.2\n60.8\t-58.6\n61.5\t-58\n62.2\t-57.4\n62.9\t-56.8\n63.6\t-56.2\n64.3\t-55.6\n65\t-55\n65.7\t-54.4\n66.4\t-53.8\n67.1\t-53.2\n67.8\t-52.6\n68.5\t-52\n69.2\t-51.4\n69.9\t-50.8\n70.6\t-50.2\n71.3\t-49.6\n71.1\t-49\n70.9\t-48.4\n70.7\t-47.8\n70.5\t-47.2\n70.3\t-46.6\n70.1\t-46\n69.9\t-45.4\n69.7\t-44.8\n69.5\t-44.2\n69.3\t-43.6\n69.1\t-43\n68.9\t-42.4\n68.7\t-41.8\n68.5\t-41.2\n68.3\t-40.6\n68.1\t-40\n67.9\t-39.4\n67.7\t-38.8\n67.5\t-38.2\n67.3\t-37.6\n67.1\t-37\n66.9\t-36.4\n66.7\t-35.8\n66.5\t-35.2\n66.3\t-34.6\n66.1\t-34\n65.9\t-33.4\n65.7\t-32.8\n65.5\t-32.2\n65.3\t-31.6\n65.1\t-31\n64.9\t-30.4\n64.7\t-29.8\n64.5\t-29.2\n64.3\t-28.6\n64.1\t-28\n63.9\t-27.4\n63.7\t-26.8\n63.5\t-26.2\n63.3\t-25.6\n63.1\t-25\n62.9\t-24.4\n62.7\t-23.8\n62.5\t-23.2\n62.3\t-22.6\n62.1\t-22\n61.9\t-21.4\n61.7\t-20.8\n61.5\t-20.2\n61.3\t-19.6\n61.1\t-19\n60.9\t-18.4\n60.7\t-17.8\n60.5\t-17.2\n60.3\t-16.6\n60.1\t-16\n59.9\t-15.4\n59.7\t-14.8\n59.5\t-14.2\n59.3\t-13.6\n59.1\t-13\n58.9\t-12.4\n58.7\t-11.8\n58.5\t-11.2\n58.3\t-10.6\n58.1\t-10\n57.9\t-9.4\n57.7\t-8.8\n57.5\t-8.2\n57.3\t-7.6\n57.1\t-7\n56.9\t-6.4\n56.7\t-5.8\n56.5\t-5.2\n56.3\t-4.6\n56.1\t-4\n55.9\t-3.4\n55.7\t-2.8\n55.5\t-2.2\n55.3\t-1.6\n55.1\t-1\n54.9\t-0.4\n54.7\t0.2\n54.5\t0.8\n54.3\t1.4\n54.1\t2\n53.9\t2.6\n53.7\t3.2\n53.5\t3.8\n53.3\t4.4\n53.1\t5\n52.9\t5.6\n52.7\t6.2\n52.5\t6.8\n52.3\t7.4\n52.1\t8\n51.9\t8.6\n51.7\t9.2\n51.5\t9.8\n51.3\t10.4\n51.1\t11\n50.9\t11.6\n50.7\t12.2\n50.5\t12.8\n50.3\t13.4\n50.1\t14\n49.9\t14.6\n49.7\t15.2\n49.5\t15.8\n49.3\t16.4\n49.1\t17\n48.9\t17.6\n48.7\t18.2\n48.5\t18.8\n48.3\t19.4\n48.1\t20\n47.9\t20.6\n47.7\t21.2\n47.5\t21.8\n47.3\t22.4\n47.1\t23\n46.9\t23.6\n46.7\t24.2\n46.5\t24.8\n46.3\t25.4\n46.1\t26\n45.9\t26.6\n45.7\t27.2\n45.5\t27.8\n45.3\t28.4\n45.1\t29\n44.9\t29.6\n44.7\t30.2\n44.5\t30.8\n44.3\t31.4\n44.1\t32\n43.9\t32.6\n43.7\t33.2\n43.5\t33.8\n43.3\t34.4\n43.1\t35\n42.9\t35.6\n42.7\t36.2\n42.5\t36.8\n42.3\t37.4\n42.1\t38\n41.9\t38.6\n41.7\t39.2\n41.5\t39.8\n41.3\t40.4\n41.1\t40.1\n40.9\t39.8\n40.7\t39.5\n40.5\t39.2\n40.3\t38.9\n40.1\t38.6\n39.9\t38.3\n39.7\t38\n39.5\t37.7\n39.3\t37.4\n39.1\t37.1\n38.9\t36.8\n38.7\t36.5\n38.5\t36.2\n38.3\t35.9\n38.1\t35.6\n37.9\t35.3\n37.7\t35\n37.5\t34.7\n37.3\t34.4\n37.1\t34.1\n36.9\t33.8\n36.7\t33.5\n36.5\t33.2\n36.3\t32.9\n36.1\t32.6\n35.9\t32.3\n35.7\t32\n35.5\t31.7\n35.3\t31.4\n35.1\t31.1\n34.9\t30.8\n34.7\t30.5\n34.5\t30.2\n34.3\t29.9\n34.1\t29.6\n33.9\t29.3\n33.7\t29\n33.5\t28.7\n33.3\t28.4\n33.1\t28.1\n32.9\t27.8\n32.7\t27.5\n32.5\t27.2\n32.3\t26.9\n32.1\t26.6\n31.9\t26.3\n31.7\t26\n31.5\t25.7\n31.3\t25.4\n31.1\t25.1\n30.9\t24.8\n30.7\t24.5\n30.5\t24.2\n30.3\t23.9\n30.1\t23.6\n29.9\t23.3\n29.7\t23\n29.5\t22.7\n29.3\t22.4\n29.1\t22.1\n28.9\t21.8\n28.7\t21.5\n28.5\t21.2\n28.3\t20.9\n28.1\t20.6\n27.9\t20.3\n27.7\t20\n27.5\t19.7\n27.3\t19.4\n27.1\t19.1\n26.9\t18.8\n26.7\t18.5\n26.5\t18.2\n26.3\t17.9\n26.1\t17.6\n25.9\t17.3\n25.7\t17\n25.5\t16.7\n25.3\t16.4\n25.1\t16.1\n24.9\t15.8\n24.7\t15.5\n24.5\t15.2\n24.3\t14.9\n24.1\t14.6\n23.9\t14.3\n23.7\t14\n23.5\t13.7\n23.3\t13.4\n23.1\t13.1\n22.9\t12.8\n22.7\t12.5\n22.5\t12.2\n22.3\t11.9\n22.1\t11.6\n21.9\t11.3\n21.7\t11\n21.5\t10.7\n21.3\t10.4\n21.1\t10.1\n20.9\t9.8\n20.7\t9.5\n20.5\t9.2\n20.3\t8.9\n20.1\t8.6\n19.9\t8.3\n19.7\t8\n19.5\t7.7\n19.3\t7.4\n19.1\t7.1\n18.9\t6.8\n18.7\t6.5\n18.5\t6.2\n18.3\t5.9\n18.1\t5.6\n17.9\t5.3\n17.7\t5\n17.5\t4.7\n17.3\t4.4\n17.1\t4.1\n16.9\t3.8\n16.7\t3.5\n16.5\t3.2\n16.3\t2.9\n16.1\t2.6\n15.9\t2.3\n15.7\t2\n15.5\t1.7\n15.3\t1.4\n15.1\t1.1\n14.9\t0.8\n14.7\t0.5\n14.5\t0.2\n14.3\t-0.1\n14.1\t-0.4\n13.9\t-0.7\n13.7\t-1\n13.5\t-1.3\n13.3\t-1.6\n13.1\t-1.9\n12.9\t-2.2\n12.7\t-2.5\n12.5\t-2.8\n12.3\t-3.1\n12.1\t-3.4\n11.9\t-3.7\n11.7\t-4\n11.5\t-4.3\n11.3\t-4.6\n11.1\t-4.9\n10.9\t-5.2\n10.7\t-5.5\n10.5\t-5.8\n10.3\t-6.1\n10.1\t-6.4\n9.9\t-6.7\n9.7\t-7\n9.5\t-7.3\n9.3\t-7.6\n9.1\t-7.9\n8.9\t-8.2\n8.7\t-8.5\n8.5\t-8.8\n8.3\t-9.1\n8.1\t-9.4\n7.9\t-9.7\n7.7\t-10\n7.5\t-10.3\n7.3\t-10.6\n7.1\t-10.9\n6.9\t-11.2\n6.7\t-11.5\n6.5\t-11.8\n6.3\t-12.1\n6.1\t-12.4\n5.9\t-12.7\n5.7\t-13\n5.5\t-13.3\n5.3\t-13.6\n5.1\t-13.9\n4.9\t-14.2\n4.3\t-14.5\n3.7\t-14.8\n3.1\t-15.1\n2.5\t-15.4\n1.9\t-15.7\n1.3\t-16\n0.7\t-16.3\n0.1\t-16.6\n-0.5\t-16.9\n-1.1\t-17.2\n-1.7\t-17.5\n-2.3\t-17.8\n-2.9\t-18.1\n-3.5\t-18.4\n-4.1\t-18.7\n-4.7\t-19\n-5.3\t-19.3\n-5.9\t-19.6\n-6.5\t-19.9\n-7.1\t-20.2\n-7.7\t-20.5\n-8.3\t-20.8\n-8.9\t-21.1\n-9.5\t-21.4\n-10.1\t-21.7\n-10.7\t-22\n-11.3\t-22.3\n-11.9\t-22.6\n-12.5\t-22.9\n-13.1\t-23.2\n-13.7\t-23.5\n-14.3\t-23.8\n-14.9\t-24.1\n-15.5\t-24.4\n-16.1\t-24.7\n-16.7\t-25\n-17.3\t-25.3\n-17.9\t-25.6\n-18.5\t-25.9\n-19.1\t-26.2\n-19.7\t-26.5\n-20.3\t-26.8\n-20.9\t-27.1\n-21.5\t-27.4\n-22.1\t-27.7\n-22.7\t-28\n-23.3\t-28.3\n-23.9\t-28.6\n-24.5\t-28.9\n-25.1\t-29.2\n-25.7\t-29.5\n-26.3\t-29.8\n-26.9\t-30.1\n-27.5\t-30.4\n-28.1\t-30.7\n-28.7\t-31\n-29.3\t-31.3\n-29.9\t-31.6\n-30.5\t-31.9\n-31.1\t-32.2\n-31.7\t-32.5\n-32.3\t-32.8\n-32.9\t-33.1\n-33.5\t-33.4\n-34.1\t-33.7\n-34.7\t-34\n-35.3\t-34.3\n-35.9\t-34.6\n-36.5\t-34.9\n-37.1\t-35.2\n-37.7\t-35.5\n-38.3\t-35.8\n-38.9\t-36.1\n-39.5\t-36.4\n-40.1\t-36.7\n-40.7\t-37\n-41.3\t-37.3\n-41.9\t-37.6\n-42.5\t-37.9\n-43.1\t-38.2\n-43.7\t-38.5\n-44.3\t-38.8\n-44.9\t-39.1\n-45.5\t-39.4\n-46.1\t-39.7\n-46.7\t-40\n-47.3\t-40.3\n-47.9\t-40.6\n-48.5\t-40.9\n-49.1\t-41.2\n-49.7\t-41.5\n-50.3\t-41.8\n-50.9\t-42.1\n-51.5\t-42.4\n-52.1\t-42.7\n-52.7\t-43\n-53.3\t-43.3\n-53.9\t-43.6\n-54.5\t-43.9\n-55.1\t-44.2\n-55.7\t-44.5\n-55.4\t-44.8\n-55.1\t-45.1\n-54.8\t-45.4\n-54.5\t-45.7\n-54.2\t-46\n-53.9\t-46.3\n-53.6\t-46.6\n-53.3\t-46.9\n-53\t-47.2\n-52.7\t-47.5\n-52.4\t-47.8\n-52.1\t-48.1\n-51.8\t-48.4\n-51.5\t-48.7\n-51.2\t-49\n-50.9\t-49.3\n-50.6\t-49.6\n-50.3\t-49.9\n-50\t-50.2\n-49.7\t-50.5\n-49.4\t-50.8\n-49.1\t-51.1\n-48.8\t-51.4\n-48.5\t-51.7\n-48.2\t-52\n-47.9\t-52.3\n-47.6\t-52.6\n-47.3\t-52.9\n-47\t-53.2\n-46.7\t-53.5\n-46.4\t-53.8\n-46.1\t-54.1\n-45.8\t-54.4\n-45.5\t-54.7\n-45.2\t-55\n-44.9\t-55.3\n-44.6\t-55.6\n-44.3\t-55.9\n-44\t-56.2\n-43.7\t-56.5\n-43.4\t-56.8\n-43.1\t-57.1\n-42.8\t-57.4\n-42.5\t-57.7\n-42.2\t-58\n-41.9\t-58.3\n-41.6\t-58.6\n-41.3\t-58.9\n-41\t-59.2\n-40.7\t-59.5\n-40.4\t-59.8\n-40.1\t-60.1\n-39.8\t-60.4\n-39.5\t-60.7\n-39.2\t-61\n-38.9\t-61.3\n-38.6\t-61.6\n-38.3\t-61.9\n-38\t-62.2\n-37.7\t-62.5\n-37.4\t-62.8\n-37.1\t-63.1\n-36.8\t-63.4\n-36.5\t-63.7\n-36.2\t-64\n-35.9\t-64.3\n-35.6\t-64.6\n-35.3\t-64.9\n-35\t-65.2\n-34.7\t-65.5\n-34.4\t-65.8\n-34.1\t-66.1\n-33.8\t-66.4\n-33.5\t-66.7\n-33.2\t-67\n-32.9\t-67.3\n-32.6\t-67.6\n-32.3\t-67.9\n-32\t-68.2\n-31.7\t-68.5\n-31.4\t-68.8\n-31.1\t-69.1\n-30.8\t-69.4\n-30.5\t-69.7\n-30.2\t-70\n-29.9\t-70.3\n-29.6\t-70.6\n-29.3\t-70.9\n-29\t-71.2\n-28.7\t-71.5\n-28.4\t-71.8\n-28.1\t-72.1\n-27.8\t-72.4\n-27.5\t-72.7\n-27.2\t-73\n-26.9\t-73.3\n-26.6\t-73.6\n-26.3\t-73.9\n-26\t-74.2\n-25.7\t-74.5\n-25.4\t-74.8\n-25.1\t-75.1\n-24.8\t-75.4\n-24.5\t-75.7\n-24.2\t-76\n-23.9\t-76.3\n-23.6\t-76.6\n-23.3\t-76.9\n-23\t-77.2\n-22.7\t-77.5\n-22.4\t-77.8\n-22.1\t-78.1\n-21.8\t-78.4\n-21.5\t-78.7\n-21.2\t-79\n-20.9\t-79.3\n-20.6\t-79.6\n-20.3\t-79.9\n-20\t-80.2\n-19.7\t-80.5\n-19.4\t-80.8\n-19.1\t-81.1\n-18.8\t-81.4\n-18.5\t-81.7\n-18.2\t-82\n-17.9\t-82.3\n-17.6\t-82.6\n-17.3\t-82.9\n-17\t-83.2\n-16.7\t-83.5\n-16.4\t-83.8\n-16.1\t-84.1\n-15.8\t-84.4\n-15.5\t-84.7\n-15.2\t-85\n-14.9\t-85.3\n-14.6\t-85.6\n-14.3\t-85.9\n-14\t-86.2\n-13.7\t-86.5\n-13.4\t-86.8\n-13.1\t-87.1\n-12.8\t-87.4\n-12.5\t-87.7\n-12.2\t-88\n-11.9\t-88.3\n-11.6\t-88.6\n-11.3\t-88.9\n-11\t-89.2\n-10.7\t-89.5\n-10.4\t-89.8\n-10.1\t-90.1\n-9.8\t-90.4\n-9.5\t-90.3\n-9.2\t-90.2\n-8.9\t-90.1\n-8.6\t-90\n-8.3\t-89.9\n-8\t-89.8\n-7.7\t-89.7\n-7.4\t-89.6\n-7.1\t-89.5\n-6.8\t-89.4\n-6.5\t-89.3\n-6.2\t-89.2\n-5.9\t-89.1\n-5.6\t-89\n-5.3\t-88.9\n-5\t-88.8\n-4.7\t-88.7\n-4.4\t-88.6\n-4.1\t-88.5\n-3.8\t-88.4\n-3.5\t-88.3\n-3.2\t-88.2\n-2.9\t-88.1\n-2.6\t-88\n-2.3\t-87.9\n-2\t-87.8\n-1.7\t-87.7\n-1.4\t-87.6\n-1.1\t-87.5\n-0.8\t-87.4\n-0.5\t-87.3\n-0.2\t-87.2\n0.1\t-87.1\n0.4\t-87\n0.7\t-86.9\n1\t-86.8\n1.3\t-86.7\n1.6\t-86.6\n1.9\t-86.5\n2.2\t-86.4\n2.5\t-86.3\n2.8\t-86.2\n3.1\t-86.1\n3.4\t-86\n3.7\t-85.9\n4\t-85.8\n4.3\t-85.7\n4.6\t-85.6\n4.9\t-85.5\n5.2\t-85.4\n5.5\t-85.3\n5.8\t-85.2\n6.1\t-85.1\n6.4\t-85\n6.7\t-84.9\n7\t-84.8\n7.3\t-84.7\n7.6\t-84.6\n7.9\t-84.5\n8.2\t-84.4\n8.5\t-84.3\n8.8\t-84.2\n9.1\t-84.1\n9.4\t-84\n9.7\t-83.9\n10\t-83.8\n10.3\t-83.7\n10.6\t-83.6\n10.9\t-83.5\n11.2\t-83.4\n11.5\t-83.3\n11.8\t-83.2\n12.1\t-83.1\n12.4\t-83\n12.7\t-82.9\n13\t-82.8\n13.3\t-82.7\n13.6\t-82.6\n13.9\t-82.5\n14.2\t-82.4\n14.5\t-82.3\n14.8\t-82.2\n15.1\t-82.1\n15.4\t-82\n15.7\t-81.9\n16\t-81.8\n16.3\t-81.7\n16.6\t-81.6\n16.9\t-81.5\n17.2\t-81.4\n17.5\t-81.3\n17.8\t-81.2\n18.1\t-81.1\n18.4\t-81\n18.7\t-80.9\n19\t-80.8\n19.3\t-80.7\n19.6\t-80.6\n19.9\t-80.5\n20.2\t-80.4\n20.5\t-80.3\n20.8\t-80.2\n21.1\t-80.1\n21.4\t-80\n21.7\t-79.9\n22\t-79.8\n22.3\t-79.7\n22.6\t-79.6\n22.9\t-79.5\n23.2\t-79.4\n23.5\t-79.3\n23.8\t-79.2\n24.1\t-79.1\n24.4\t-79\n24.7\t-78.9\n25\t-78.8\n25.3\t-78.7\n25.6\t-78.6\n25.2\t-78.5\n24.8\t-78.4\n24.4\t-78.3\n24\t-78.2\n23.6\t-78.1\n23.2\t-78\n22.8\t-77.9\n22.4\t-77.8\n22\t-77.7\n21.6\t-77.6\n21.2\t-77.5\n20.8\t-77.4\n20.4\t-77.3\n20\t-77.2\n19.6\t-77.1\n19.2\t-77\n18.8\t-76.9\n18.4\t-76.8\n18\t-76.7\n17.6\t-76.6\n17.2\t-76.5\n16.8\t-76.4\n16.4\t-76.3\n16\t-76.2\n15.6\t-76.1\n15.2\t-76\n14.8\t-75.9\n14.4\t-75.8\n14\t-75.7\n13.6\t-75.6\n13.2\t-75.5\n12.8\t-75.4\n12.4\t-75.3\n12\t-75.2\n11.6\t-75.1\n11.2\t-75\n10.8\t-74.9\n10.4\t-74.8\n10\t-74.7\n9.6\t-74.6\n9.2\t-74.5\n8.8\t-74.4\n8.4\t-74.3\n8\t-74.2\n7.6\t-74.1\n7.2\t-74\n6.8\t-73.9\n6.4\t-73.8\n6\t-73.7\n5.6\t-73.6\n5.2\t-73.5\n4.8\t-73.4\n4.4\t-73.3\n4\t-73.2\n3.6\t-73.1\n3.2\t-73\n2.8\t-72.9\n2.4\t-72.8\n2\t-72.7\n1.6\t-72.6\n1.2\t-72.5\n0.8\t-72.4\n0.4\t-72.3\n-2.08267E-12\t-72.2\n-0.4\t-72.1\n-0.8\t-72\n-1.2\t-71.9\n-1.6\t-71.8\n-2\t-71.7\n-2.4\t-71.6\n-2.8\t-71.5\n-3.2\t-71.4\n-3.6\t-71.3\n-4\t-71.2\n-4.4\t-71.1\n-4.8\t-71\n-5.2\t-70.9\n-5.6\t-70.8\n-6\t-70.7\n-6.4\t-70.6\n-6.8\t-70.5\n-7.2\t-70.4\n-7.6\t-70.3\n-8\t-70.2\n-8.4\t-70.1\n-8.8\t-70\n-9.2\t-69.9\n-9.6\t-69.8\n-10\t-69.7\n-10.4\t-69.6\n-10.8\t-69.5\n-11.2\t-69.4\n-11.6\t-69.3\n-12\t-69.2\n-12.4\t-69.1\n-12.8\t-69\n-13.2\t-68.9\n-13.6\t-68.8\n-14\t-68.7\n-14.4\t-68.6\n-14.8\t-68.5\n-15.2\t-68.4\n-15.6\t-68.3\n-16\t-68.2\n-16.4\t-68.1\n-16.8\t-68\n-17.2\t-67.9\n-17.6\t-67.8\n-18\t-67.7\n-18.4\t-67.6\n-18.8\t-67.5\n-19.2\t-67.4\n-19.6\t-67.3\n-20\t-67.2\n-20.4\t-67.1\n-20.8\t-67\n-21.2\t-66.9\n-21.6\t-66.8\n-22\t-66.7\n-22.4\t-66.6\n-22.8\t-66.5\n-23.2\t-66.4\n-23.6\t-66.3\n-24\t-66.2\n-24.4\t-66.1\n-24.8\t-66\n-25.2\t-65.9\n-25.6\t-65.8\n-26\t-65.7\n-26.4\t-65.6\n-26.8\t-65.5\n-27.2\t-65.4\n-27.6\t-65.1\n-28\t-64.8\n-28.4\t-64.5\n-28.8\t-64.2\n-29.2\t-63.9\n-29.6\t-63.6\n-30\t-63.3\n-30.4\t-63\n-30.8\t-62.7\n-31.2\t-62.4\n-31.6\t-62.1\n-32\t-61.8\n-32.4\t-61.5\n-32.8\t-61.2\n-33.2\t-60.9\n-33.6\t-60.6\n-34\t-60.3\n-34.4\t-60\n-34.8\t-59.7\n-35.2\t-59.4\n-35.6\t-59.1\n-36\t-58.8\n-36.4\t-58.5\n-36.8\t-58.2\n-37.2\t-57.9\n-37.6\t-57.6\n-38\t-57.3\n-38.4\t-57\n-38.8\t-56.7\n-39.2\t-56.4\n-39.6\t-56.1\n-40\t-55.8\n-40.4\t-55.5\n-40.8\t-55.2\n-41.2\t-54.9\n-41.6\t-54.6\n-42\t-54.3\n-42.4\t-54\n-42.8\t-53.7\n-43.2\t-53.4\n-43.6\t-53.1\n-44\t-52.8\n-44.4\t-52.5\n-44.8\t-52.2\n-45.2\t-51.9\n-45.6\t-51.6\n-46\t-51.3\n-46.4\t-51\n-46.8\t-50.7\n-47.2\t-50.4\n-47.6\t-50.1\n-48\t-49.8\n-48.4\t-49.5\n-48.8\t-49.2\n-49.2\t-48.9\n-49.6\t-48.6\n-50\t-48.3\n-50.4\t-48\n-50.8\t-47.7\n-51.2\t-47.4\n-51.6\t-47.1\n-52\t-46.8\n-52.4\t-46.5\n-52.8\t-46.2\n-53.2\t-45.9\n-53.6\t-45.6\n-54\t-45.3\n-54.4\t-45\n-54.8\t-44.7\n-55.2\t-44.4\n-55.6\t-44.1\n-56\t-43.8\n-56.4\t-43.5\n-56.8\t-43.2\n-57.2\t-42.9\n-57.6\t-42.6\n-58\t-42.3\n-58.4\t-42\n-58.8\t-41.7\n-59.2\t-41.4\n-59.6\t-41.1\n-60\t-40.8\n-60.4\t-40.5\n-60.8\t-40.2\n-61.2\t-39.9\n-61.6\t-39.6\n-62\t-39.3\n-62.4\t-39\n-62.8\t-38.7\n-63.2\t-38.4\n-63.6\t-38.1\n-64\t-37.8\n-64.4\t-37.5\n-64.8\t-37.2\n-65.2\t-36.9\n-65.6\t-36.6\n-66\t-36.3\n-66.4\t-36\n-66.8\t-35.7\n-67.2\t-35.4\n-67.6\t-35.1\n-68\t-34.8\n-68.4\t-34.5\n-68.8\t-34.2\n-69.2\t-33.9\n-69.6\t-33.6\n-70\t-33.3\n-70.4\t-33\n-70.8\t-32.7\n-71.2\t-32.4\n-71.6\t-32.1\n-72\t-31.8\n-72.4\t-31.5\n-72.8\t-31.2\n-73.2\t-30.9\n-73.6\t-30.6\n-74\t-30.3\n-74.4\t-30\n-74.8\t-29.7\n-75.2\t-29.4\n-75.6\t-29.1\n-76\t-28.8\n-76.4\t-28.5\n-76.8\t-28.2\n-77.2\t-27.9\n-77.6\t-27.6\n-78\t-27.3\n-78.4\t-27\n-78.8\t-26.7\n-79.2\t-26.4\n-79.6\t-26.1\n-80\t-25.8\n-80.4\t-25.5\n-80.8\t-25.2\n-81.2\t-24.9\n-81.6\t-24.6\n-82\t-24.3\n-82.4\t-24\n-82.8\t-23.7\n-83.2\t-23.4\n-83.6\t-23.1\n-84\t-22.8\n-84.4\t-22.5\n-84.8\t-22.2\n-85.2\t-21.9\n-85.6\t-21.6\n-86\t-21.3\n-86.4\t-21\n-86.8\t-20.7\n-87.2\t-20.4\n-87.6\t-20.1\n-88\t-19.8\n-88.4\t-19.5\n-88.8\t-19.2\n-89.2\t-18.9\n-89.6\t-18.6\n-90\t-18.3\n-90.4\t-18\n-90.8\t-17.7\n-91.2\t-17.4\n-91.6\t-17.1\n-92\t-16.8\n-92.4\t-16.5\n-92.8\t-16.2\n-93.2\t-15.9\n-92.5\t-15.6\n-91.8\t-15.3\n-91.1\t-15\n-90.4\t-14.7\n-89.7\t-14.4\n-89\t-14.1\n-88.3\t-13.8\n-87.6\t-13.5\n-86.9\t-13.2\n-86.2\t-12.9\n-85.5\t-12.6\n-84.8\t-12.3\n-84.1\t-12\n-83.4\t-11.7\n-82.7\t-11.4\n-82\t-11.1\n-81.3\t-10.8\n-80.6\t-10.5\n-79.9\t-10.2\n-79.2\t-9.9\n-78.5\t-9.6\n-77.8\t-9.3\n-77.1\t-9\n-76.4\t-8.7\n-75.7\t-8.4\n-75\t-8.1\n-74.3\t-7.8\n-73.6\t-7.5\n-72.9\t-7.2\n-72.2\t-6.9\n-71.5\t-6.6\n-70.8\t-6.3\n-70.1\t-6\n-69.4\t-5.7\n-68.7\t-5.4\n-68\t-5.1\n-67.3\t-4.8\n-66.6\t-4.5\n-65.9\t-4.2\n-65.2\t-3.9\n-64.5\t-3.6\n-63.8\t-3.3\n-63.1\t-3\n-62.4\t-2.7\n-61.7\t-2.4\n-61\t-2.1\n-60.3\t-1.8\n-59.6\t-1.5\n-58.9\t-1.2\n-58.2\t-0.9\n-57.5\t-0.6\n-56.8\t-0.3\n-56.1\t-1.83087E-12\n-55.4\t0.3\n-54.7\t0.6\n-54\t0.9\n-53.3\t1.2\n-52.6\t1.5\n-51.9\t1.8\n-51.2\t2.1\n-50.5\t2.4\n-49.8\t2.7\n-49.1\t3\n-48.4\t3.3\n-47.7\t3.6\n-47\t3.9\n-46.3\t4.2\n-45.6\t4.5\n-44.9\t4.8\n-44.2\t5.1\n-43.5\t5.4\n-42.8\t5.7\n-42.1\t6\n-41.4\t6.3\n-40.7\t6.6\n-40\t6.9\n-39.3\t7.2\n-38.6\t7.5\n-37.9\t7.8\n-37.2\t8.1\n-36.5\t8.4\n-35.8\t8.7\n-35.1\t9\n-34.4\t9.3\n-33.7\t9.6\n-33\t9.9\n-32.3\t10.2\n-31.6\t10.5\n-30.9\t10.8\n-30.2\t11.1\n-29.5\t11.4\n-28.8\t11.7\n-28.1\t12\n-27.4\t12.3\n-26.7\t12.6\n-26\t12.9\n-25.3\t13.2\n-24.6\t13.5\n-23.9\t13.8\n-23.2\t14.1\n-22.5\t14.4\n-21.8\t14.7\n-21.1\t15\n-20.4\t15.3\n-19.7\t15.6\n-19\t15.9\n-18.3\t16.2\n-17.6\t16.5\n-16.9\t16.8\n-16.2\t17.1\n-15.5\t17.4\n-14.8\t17.7\n-14.1\t18\n-13.4\t18.3\n-12.7\t18.6\n-12\t18.9\n-11.3\t19.2\n-10.6\t19.5\n-9.9\t19.8\n-9.2\t20.1\n-8.5\t20.4\n-7.8\t20.7\n-7.1\t21\n-6.4\t21.3\n-5.7\t21.6\n-5\t21.9\n-4.3\t22.2\n-3.6\t22.5\n-2.9\t22.8\n-2.2\t23.1\n-1.5\t23.4\n-0.8\t23.7\n-0.1\t24\n0.6\t24.3\n1.3\t24.6\n2\t24.9\n2.7\t25.2\n3.4\t25.5\n4.1\t25.8\n4.8\t26.1\n5.5\t26.4\n6.2\t26.7\n6.9\t27\n7.6\t27.3\n8.3\t27.6\n9\t27.9\n9.7\t28.2\n10.4\t28.5\n11.1\t28.8\n11.8\t29.1\n12.5\t29.4\n13.2\t29.7\n13.9\t30\n14.6\t30.3\n15.3\t30.6\n16\t30.9\n16.7\t31.2\n17.4\t31.5\n18.1\t31.8\n18.8\t32.1\n19.5\t32.4\n20.2\t32.7\n20.9\t33\n21.6\t33.3\n22.3\t33.6\n23\t33.9\n23.7\t34.2\n24.4\t34.5\n25.1\t34.8\n25.8\t35.1\n26.5\t35.4\n27.2\t35.7\n27.9\t36\n28.6\t36.3\n29.3\t36.6\n30\t36.9\n30.7\t37.2\n31.4\t37.5\n32.1\t37.8\n32.8\t38.1\n33.5\t38.4\n34.2\t38.7\n34.9\t39\n35.6\t39.3\n36.3\t39.6\n37\t39.9\n37.7\t40.2\n38.4\t40.5\n39.1\t40.8\n39.8\t41.1\n40.5\t41.4\n41.2\t41.7\n41.9\t42\n42.6\t42.3\n43.3\t42.6\n44\t42.9\n44.7\t43.2\n45.4\t43.5\n46.1\t43.8\n46.8\t44.1\n47.5\t44.4\n48.2\t44.7\n48.9\t45\n49.6\t45.3\n50.3\t45.6\n51\t45.9\n51.7\t46.2\n52.4\t46.5\n53.1\t46.8\n53.8\t47.1\n54.5\t47.4\n55.2\t47.7\n55.9\t48\n56.6\t48.3\n57.3\t48.6\n58\t48.9\n58.7\t49.2\n59.4\t49.5\n60.1\t49.8\n60.8\t50.1\n61.5\t50.4\n62.2\t50.7\n62.9\t51\n63.6\t51.3\n64.3\t51.6\n65\t51.9\n65.7\t52.2\n66.4\t52.5\n67.1\t52.8\n67.8\t53.1\n68.5\t53.4\n69.2\t53.7\n69.9\t54\n70.6\t54.3\n71.3\t54.6\n72\t54.9\n72.7\t55.2\n73.4\t55.5\n74.1\t55.8\n74.8\t56.1\n75.5\t56.4\n76.2\t56.7\n76.9\t57\n77.6\t57.3\n78.3\t57.6\n79\t57.9\n79.7\t58.2\n80.4\t58.5\n81.1\t58.8\n81.8\t59.1\n82.5\t59.4\n83.2\t59.7\n83.9\t60\n84.6\t60.3\n85.3\t60.6\n86\t60.9\n86.7\t61.2\n87.4\t61.5\n88.1\t61.8\n88.8\t62.1\n89.5\t62.4\n90.2\t62.7\n90.9\t63\n91.6\t63.3\n92.3\t63.6\n93\t63.9\n93.7\t64.2\n94.4\t64.5\n95.1\t64.8\n94.7\t65.1\n94.3\t65.4\n93.9\t65.7\n93.5\t66\n93.1\t66.3\n92.7\t66.6\n92.3\t66.9\n91.9\t67.2\n91.5\t67.5\n91.1\t67.8\n90.7\t68.1\n90.3\t68.4\n89.9\t68.7\n89.5\t69\n89.1\t69.3\n88.7\t69.6\n88.3\t69.9\n87.9\t70.2\n87.5\t70.5\n87.1\t70.8\n86.7\t71.1\n86.3\t71.4\n85.9\t71.7\n85.5\t72\n85.1\t72.3\n84.7\t72.6\n84.3\t72.9\n83.9\t73.2\n83.5\t73.5\n83.1\t73.8\n82.7\t74.1\n82.3\t74.4\n81.9\t74.7\n81.5\t75\n81.1\t75.3\n80.7\t75.6\n80.3\t75.9\n79.9\t76.2\n79.5\t76.5\n79.1\t76.8\n78.7\t77.1\n78.3\t77.4\n77.9\t77.7\n77.5\t78\n77.1\t78.3\n76.7\t78.6\n76.3\t78.9\n75.9\t79.2\n75.5\t79.5\n75.1\t79.8\n74.7\t80.1\n74.3\t80.4\n73.9\t80.7\n73.5\t81\n73.1\t81.3\n72.7\t81.6\n72.3\t81.9\n71.9\t82.2\n71.5\t82.5\n71.1\t82.8\n70.7\t83.1\n70.3\t83.4\n69.9\t83.7\n69.5\t84\n69.1\t84.3\n68.7\t84.6\n68.3\t84.9\n67.9\t85.2\n67.5\t85.5\n67.1\t85.8\n66.7\t86.1\n66.3\t86.4\n65.9\t86.7\n65.5\t87\n65.1\t87.3\n64.7\t87.6\n64.3\t87.9\n63.9\t88.2\n63.5\t88.5\n63.1\t88.8\n62.7\t89.1\n62.3\t89.4\n61.9\t89.7\n61.5\t90\n61.1\t90.3\n60.7\t90.6\n60.3\t90.9\n59.9\t91.2\n59.5\t91.5\n59.1\t91.8\n58.7\t92.1\n58.3\t92.4\n57.9\t92.7\n57.5\t93\n57.1\t93.3\n56.7\t93.6\n56.3\t93.9\n55.9\t93.2\n55.5\t92.5\n55.1\t91.8\n54.7\t91.1\n54.3\t90.4\n53.9\t89.7\n53.5\t89\n53.1\t88.3\n52.7\t87.6\n52.3\t86.9\n51.9\t86.2\n51.5\t85.5\n51.1\t84.8\n50.7\t84.1\n50.3\t83.4\n49.9\t82.7\n49.5\t82\n49.1\t81.3\n48.7\t80.6\n48.3\t79.9\n47.9\t79.2\n47.5\t78.5\n47.1\t77.8\n46.7\t77.1\n46.3\t76.4\n45.9\t75.7\n45.5\t75\n45.1\t74.3\n44.7\t73.6\n44.3\t72.9\n43.9\t72.2\n43.5\t71.5\n43.1\t70.8\n42.7\t70.1\n42.3\t69.4\n41.9\t68.7\n41.5\t68\n41.1\t67.3\n40.7\t66.6\n40.3\t65.9\n39.9\t65.2\n39.5\t64.5\n39.1\t63.8\n38.7\t63.1\n38.3\t62.4\n37.9\t61.7\n37.5\t61\n37.1\t60.3\n36.7\t59.6\n36.3\t58.9\n35.9\t58.2\n35.5\t57.5\n35.1\t56.8\n34.7\t56.1\n34.3\t55.4\n33.9\t54.7\n33.5\t54\n33.1\t53.3\n32.7\t52.6\n32.3\t51.9\n31.9\t51.2\n31.5\t50.5\n31.1\t49.8\n30.7\t49.1\n30.3\t48.4\n29.9\t47.7\n29.5\t47\n29.1\t46.3\n28.7\t45.6\n28.3\t44.9\n27.9\t44.2\n27.5\t43.5\n27.1\t42.8\n26.7\t42.1\n26.3\t41.4\n25.9\t40.7\n25.5\t40\n25.1\t39.3\n24.7\t38.6\n24.3\t37.9\n23.9\t37.2\n23.5\t36.5\n23.1\t35.8\n22.7\t35.1\n22.3\t34.4\n21.9\t33.7\n21.5\t33\n21.1\t32.3\n20.7\t31.6\n20.3\t30.9\n19.9\t30.2\n19.5\t29.5\n19.1\t28.8\n18.7\t28.1\n18.3\t27.4\n17.9\t26.7\n17.5\t26\n17.1\t25.3\n16.7\t24.6\n16.3\t23.9\n15.9\t23.2\n15.5\t22.5\n15.1\t21.8\n14.7\t21.1\n14.3\t20.4\n13.9\t19.7\n13.5\t19\n13.1\t18.3\n12.7\t17.6\n12.3\t16.9\n11.9\t16.2\n11.5\t15.5\n11.1\t14.8\n10.7\t14.1\n10.3\t13.4\n9.9\t12.7\n9.5\t12\n9.1\t11.3\n8.7\t10.6\n8.3\t9.9\n7.9\t9.2\n7.5\t8.5\n7.1\t7.8\n6.7\t7.1\n6.3\t6.4\n5.9\t5.7\n5.5\t5\n5.1\t4.3\n4.7\t3.6\n4.3\t2.9\n3.9\t2.2\n3.5\t1.5\n3.1\t0.8\n2.7\t0.1\n2.3\t-0.6\n1.9\t-1.3\n1.5\t-2\n1.1\t-2.7\n0.7\t-3.4\n0.3\t-4.1\n-0.1\t-4.8\n-0.5\t-5.5\n-0.9\t-6.2\n-1.3\t-6.9\n-1.7\t-7.6\n-2.1\t-8.3\n-2.5\t-9\n-2.9\t-9.7\n-3.3\t-10.4\n-3.7\t-11.1\n-4.1\t-11.8\n-4.5\t-12.5\n-4.9\t-13.2\n-5.3\t-13.9\n-5.7\t-14.6\n-6.1\t-15.3\n-6.5\t-16\n-6.9\t-16.7\n-7.3\t-17.4\n-7.7\t-18.1\n-8.1\t-18.8\n-8.5\t-19.5\n-8.9\t-20.2\n-9.3\t-20.9\n-9.7\t-21.6\n-10.1\t-22.3\n-10.5\t-23\n-10.9\t-23.7\n-11.3\t-24.4\n-11.7\t-25.1\n-12.1\t-25.8\n-12.5\t-26.5\n-12.9\t-27.2\n-13.3\t-27.9\n-13.7\t-28.6\n-14.1\t-29.3\n-14.5\t-30\n-14.9\t-30.7\n-15.3\t-31.4\n-15.7\t-32.1\n-16.1\t-32.8\n-16.5\t-33.5\n-16.9\t-34.2\n-17.3\t-34.9\n-17.7\t-35.6\n-18.1\t-36.3\n-18.5\t-37\n-18.9\t-37.7\n-19.3\t-38.4\n-19.7\t-39.1\n-20.1\t-39.8\n-20.5\t-40.5\n-20.9\t-41.2\n-21.3\t-41.9\n-21.7\t-42.6\n-22.1\t-43.3\n-22.5\t-44\n-22.9\t-44.7\n-23.3\t-45.4\n-23.7\t-46.1\n-24.1\t-46.8\n-24.5\t-47.5\n-24.9\t-48.2\n-25.3\t-48.9\n-25.7\t-49.6\n-26.1\t-50.3\n-26.5\t-51\n-26.9\t-51.7\n-27.3\t-52.4\n-27.7\t-53.1\n-28.1\t-53.8\n-28.5\t-54.5\n-28.9\t-55.2\n-29.3\t-55.9\n-29.7\t-56.6\n-30.1\t-57.3\n-30.5\t-58\n-30.9\t-58.7\n-31.3\t-59.4\n-31.7\t-60.1\n-32.1\t-60.8\n-32.5\t-61.5\n-32.9\t-62.2\n-33.3\t-62.9\n-33.7\t-63.6\n-34.1\t-64.3\n-34.5\t-65\n-34.9\t-65.7\n-35.3\t-66.4\n-35.7\t-67.1\n-36.1\t-67.8\n-36.5\t-68.5\n-36.9\t-69.2\n-37.3\t-69.9\n-37.7\t-70.6\n-38.1\t-71.3\n-38.5\t-72\n-38.9\t-72.7\n-39.3\t-73.4\n-39.7\t-74.1\n-40.1\t-74.8\n-40.5\t-75.5\n-40.9\t-75\n-41.3\t-74.5\n-41.7\t-74\n-42.1\t-73.5\n-42.5\t-73\n-42.9\t-72.5\n-43.3\t-72\n-43.7\t-71.5\n-44.1\t-71\n-44.5\t-70.5\n-44.9\t-70\n-45.3\t-69.5\n-45.7\t-69\n-46.1\t-68.5\n-46.5\t-68\n-46.9\t-67.5\n-47.3\t-67\n-47.7\t-66.5\n-48.1\t-66\n-48.5\t-65.5\n-48.9\t-65\n-49.3\t-64.5\n-49.7\t-64\n-50.1\t-63.5\n-50.5\t-63\n-50.9\t-62.5\n-51.3\t-62\n-51.7\t-61.5\n-52.1\t-61\n-52.5\t-60.5\n-52.9\t-60\n-53.3\t-59.5\n-53.7\t-59\n-54.1\t-58.5\n-54.5\t-58\n-54.9\t-57.5\n-55.3\t-57\n-55.7\t-56.5\n-56.1\t-56\n-56.5\t-55.5\n-56.9\t-55\n-57.3\t-54.5\n-57.7\t-54\n-58.1\t-53.5\n-58.5\t-53\n-58.9\t-52.5\n-59.3\t-52\n-59.7\t-51.5\n-60.1\t-51\n-60.5\t-50.5\n-60.9\t-50\n-61.3\t-49.5\n-61.7\t-49\n-62.1\t-48.5\n-62.5\t-48\n-62.9\t-47.5\n-63.3\t-47\n-63.7\t-46.5\n-64.1\t-46\n-64.5\t-45.5\n-64.9\t-45\n-65.3\t-44.5\n-65.7\t-44\n-66.1\t-43.5\n-66.5\t-43\n-66.9\t-42.5\n-67.3\t-42\n-67.7\t-41.5\n-68.1\t-41\n-68.5\t-40.5\n-68.9\t-40\n-69.3\t-39.5\n-69.7\t-39\n-70.1\t-38.5\n-70.5\t-38\n-70.9\t-37.5\n-71.3\t-37\n-71.7\t-36.5\n-72.1\t-36\n-72.5\t-35.5\n-72.9\t-35\n-73.3\t-34.5\n-73.7\t-34\n-74.1\t-33.5\n-74.5\t-33\n-74.9\t-32.5\n-75.3\t-32\n-75.7\t-31.5\n-76.1\t-31\n-76.5\t-30.5\n-76.9\t-30\n-77.3\t-29.5\n-77.7\t-29\n-78.1\t-28.5\n-78.5\t-28\n-78.9\t-27.5\n-79.3\t-27\n-79.7\t-26.5\n-80.1\t-26\n-80.5\t-25.5\n-80.9\t-25\n-81.3\t-24.5\n-81.7\t-24\n-82.1\t-23.5\n-82.5\t-23\n-82.9\t-22.5\n-83.3\t-22\n-83.7\t-21.5\n-84.1\t-21\n-84.5\t-20.5\n-84.9\t-20\n-85.3\t-19.5\n-85.7\t-19\n-86.1\t-18.5\n-86.5\t-18\n-86.9\t-17.5\n-87.3\t-17\n-87.7\t-16.5\n-88.1\t-16\n-88.5\t-15.5\n-88.9\t-15\n-89.3\t-14.5\n-89.7\t-14\n-90.1\t-13.5\n-90.5\t-13\n-90.9\t-12.5\n-91.3\t-12\n-91.7\t-11.5\n-92.1\t-11\n-92.5\t-10.5\n-92.9\t-10\n-93.3\t-9.5\n-93.7\t-9\n-93.1\t-8.5\n-92.5\t-8\n-91.9\t-7.5\n-91.3\t-7\n-90.7\t-6.5\n-90.1\t-6\n-89.5\t-5.5\n-88.9\t-5\n-88.3\t-4.5\n-87.7\t-4\n-87.1\t-3.5\n-86.5\t-3\n-85.9\t-2.5\n-85.3\t-2\n-84.7\t-1.5\n-84.1\t-1\n-83.5\t-0.5\n-82.9\t-2.74269E-12\n-82.3\t0.5\n-81.7\t1\n-81.1\t1.5\n-80.5\t2\n-79.9\t2.5\n-79.3\t3\n-78.7\t3.5\n-78.1\t4\n-77.5\t4.5\n-76.9\t5\n-76.3\t5.5\n-75.7\t6\n-75.1\t6.5\n-74.5\t7\n-73.9\t7.5\n-73.3\t8\n-72.7\t8.5\n-72.1\t9\n-71.5\t9.5\n-70.9\t10\n-70.3\t10.5\n-69.7\t11\n-69.1\t11.5\n-68.5\t12\n-67.9\t12.5\n-67.3\t13\n-66.7\t13.5\n-66.1\t14\n-65.5\t14.5\n-64.9\t15\n-64.3\t15.5\n-63.7\t16\n-63.1\t16.5\n-62.5\t17\n-61.9\t17.5\n-61.3\t18\n-60.7\t18.5\n-60.1\t19\n-59.5\t19.5\n-58.9\t20\n-58.3\t20.5\n-57.7\t21\n-57.1\t21.5\n-56.5\t22\n-55.9\t22.5\n-55.3\t23\n-54.7\t23.5\n-54.1\t24\n-53.5\t24.5\n-52.9\t25\n-52.3\t25.5\n-51.7\t26\n-51.1\t26.5\n-50.5\t27\n-49.9\t27.5\n-49.3\t28\n-48.7\t28.5\n-48.1\t29\n-47.5\t29.5\n-46.9\t30\n-46.3\t30.5\n-45.7\t31\n-45.1\t31.5\n-44.5\t32\n-43.9\t32.5\n-43.3\t33\n-42.7\t33.5\n-42.1\t34\n-41.5\t34.5\n-40.9\t35\n-40.3\t35.5\n-39.7\t36\n-39.1\t35.8\n-38.5\t35.6\n-37.9\t35.4\n-37.3\t35.2\n-36.7\t35\n-36.1\t34.8\n-35.5\t34.6\n-34.9\t34.4\n-34.3\t34.2\n-33.7\t34\n-33.1\t33.8\n-32.5\t33.6\n-31.9\t33.4\n-31.3\t33.2\n-30.7\t33\n-30.1\t32.8\n-29.5\t32.6\n-28.9\t32.4\n-28.3\t32.2\n-27.7\t32\n-27.1\t31.8\n-26.5\t31.6\n-25.9\t31.4\n-25.3\t31.2\n-24.7\t31\n-24.1\t30.8\n-23.5\t30.6\n-22.9\t30.4\n-22.3\t30.2\n-21.7\t30\n-21.1\t29.8\n-20.5\t29.6\n-19.9\t29.4\n-19.3\t29.2\n-18.7\t29\n-18.1\t28.8\n-17.5\t28.6\n-16.9\t28.4\n-16.3\t28.2\n-15.7\t28\n-15.1\t27.8\n-14.5\t27.6\n-13.9\t27.4\n-13.3\t27.2\n-12.7\t27\n-12.1\t26.8\n-11.5\t26.6\n-10.9\t26.4\n-10.3\t26.2\n-9.7\t26\n-9.1\t25.8\n-8.5\t25.6\n-7.9\t25.4\n-7.3\t25.2\n-6.7\t25\n-6.1\t24.8\n-5.5\t24.6\n-4.9\t24.4\n-4.3\t24.2\n-3.7\t24\n-3.1\t23.8\n-2.5\t23.6\n-1.9\t23.4\n-1.3\t23.2\n-0.7\t23\n-0.1\t22.8\n0.5\t22.6\n1.1\t22.4\n1.7\t22.2\n2.3\t22\n2.9\t21.8\n3.5\t21.6\n4.1\t21.4\n4.7\t21.2\n5.3\t21\n5.9\t20.8\n6.5\t20.6\n7.1\t20.4\n7.7\t20.2\n8.3\t20\n8.9\t19.8\n9.5\t19.6\n10.1\t19.4\n10.7\t19.2\n11.3\t19\n11.9\t18.8\n12.5\t18.6\n13.1\t18.4\n13.7\t18.2\n14.3\t18\n14.9\t17.8\n15.5\t17.6\n16.1\t17.4\n16.7\t17.2\n17.3\t17\n17.9\t16.8\n18.5\t16.6\n19.1\t16.4\n19.7\t16.2\n20.3\t16\n20.9\t15.8\n21.5\t15.6\n22.1\t15.4\n22.7\t15.2\n23.3\t15\n23.9\t14.8\n24.5\t14.6\n25.1\t14.4\n25.7\t14.2\n26.3\t14\n26.9\t13.8\n27.5\t13.6\n28.1\t13.4\n28.7\t13.2\n29.3\t13\n29.9\t12.8\n30.5\t12.6\n31.1\t12.4\n31.7\t12.2\n32.3\t12\n32.9\t11.8\n33.5\t11.6\n34.1\t11.4\n34.7\t11.2\n35.3\t11\n35.9\t10.8\n36.5\t10.6\n37.1\t10.4\n37.7\t10.2\n38.3\t10\n38.9\t9.8\n39.5\t9.6\n40.1\t9.4\n40.7\t9.2\n41.3\t9\n41.9\t8.8\n42.5\t8.6\n43.1\t8.4\n43.7\t8.2\n44.3\t8\n44.9\t7.8\n45.5\t7.6\n46.1\t7.4\n46.7\t7.2\n47.3\t7\n47.9\t6.8\n48.5\t6.6\n49.1\t6.4\n49.7\t6.2\n50.3\t6\n50.9\t5.8\n51.5\t5.6\n52.1\t5.4\n52.7\t5.2\n53.3\t5\n53.9\t4.8\n54.5\t4.6\n55.1\t4.4\n55.7\t4.2\n56.3\t4\n56.9\t3.8\n57.5\t3.6\n58.1\t3.4\n58.7\t3.2\n59.3\t3\n59.9\t2.8\n60.5\t2.6\n61.1\t2.4\n61.7\t2.2\n62.3\t2\n62.9\t1.8\n63.5\t1.6\n64.1\t1.4\n64.7\t1.2\n65.3\t1\n65.9\t0.8\n66.5\t0.6\n67.1\t0.4\n67.7\t0.2\n68.3\t-2.71644E-12\n68.9\t-0.2\n69.5\t-0.4\n70.1\t-0.6\n70.7\t-0.8\n71.3\t-1\n71.9\t-1.2\n72.5\t-1.4\n73.1\t-1.6\n73.7\t-1.8\n74.3\t-2\n74.9\t-2.2\n75.5\t-2.4\n76.1\t-2.6\n76.7\t-2.8\n77.3\t-3\n77.9\t-3.2\n78.5\t-3.4\n79.1\t-3.6\n79.7\t-3.8\n80.3\t-4\n80.9\t-4.2\n81.5\t-4.4\n82.1\t-4.6\n82.7\t-4.8\n83.3\t-5\n83.9\t-5.2\n83.7\t-5.4\n83.5\t-5.6\n83.3\t-5.8\n83.1\t-6\n82.9\t-6.2\n82.7\t-6.4\n82.5\t-6.6\n82.3\t-6.8\n82.1\t-7\n81.9\t-7.2\n81.7\t-7.4\n81.5\t-7.6\n81.3\t-7.8\n81.1\t-8\n80.9\t-8.2\n80.7\t-8.4\n80.5\t-8.6\n80.3\t-8.8\n80.1\t-9\n79.9\t-9.2\n79.7\t-9.4\n79.5\t-9.6\n79.3\t-9.8\n79.1\t-10\n78.9\t-10.2\n78.7\t-10.4\n78.5\t-10.6\n78.3\t-10.8\n78.1\t-11\n77.9\t-11.2\n77.7\t-11.4\n77.5\t-11.6\n77.3\t-11.8\n77.1\t-12\n76.9\t-12.2\n76.7\t-12.4\n76.5\t-12.6\n76.3\t-12.8\n76.1\t-13\n75.9\t-13.2\n75.7\t-13.4\n75.5\t-13.6\n75.3\t-13.8\n75.1\t-14\n74.9\t-14.2\n74.7\t-14.4\n74.5\t-14.6\n74.3\t-14.8\n74.1\t-15\n73.9\t-15.2\n73.7\t-15.4\n73.5\t-15.6\n73.3\t-15.8\n73.1\t-16\n72.9\t-16.2\n72.7\t-16.4\n72.5\t-16.6\n72.3\t-16.8\n72.1\t-17\n71.9\t-17.2\n71.7\t-17.4\n71.5\t-17.6\n71.3\t-17.8\n71.1\t-18\n70.9\t-18.2\n70.7\t-18.4\n70.5\t-18.6\n70.3\t-18.8\n70.1\t-19\n69.9\t-19.2\n69.7\t-19.4\n69.5\t-19.6\n69.3\t-19.8\n69.1\t-20\n68.9\t-20.2\n68.7\t-20.4\n68.5\t-20.6\n68.3\t-20.8\n68.1\t-21\n67.9\t-21.2\n67.7\t-21.4\n67.5\t-21.6\n67.3\t-21.8\n67.1\t-22\n66.9\t-22.2\n66.7\t-22.4\n66.5\t-22.6\n66.3\t-22.8\n66.1\t-23\n65.9\t-23.2\n65.7\t-23.4\n65.5\t-23.6\n65.3\t-23.8\n65.1\t-24\n64.9\t-24.2\n64.7\t-24.4\n64.5\t-24.6\n64.3\t-24.8\n64.1\t-25\n63.9\t-25.2\n63.7\t-25.4\n63.5\t-25.6\n63.3\t-25.8\n63.1\t-26\n62.9\t-26.2\n62.7\t-26.4\n62.5\t-26.6\n62.3\t-26.8\n62.1\t-27\n61.9\t-27.2\n61.7\t-27.4\n61.5\t-27.6\n61.3\t-27.8\n61.1\t-28\n60.9\t-28.2\n60.7\t-28.4\n60.5\t-28.6\n60.3\t-28.8\n60.1\t-29\n59.9\t-29.2\n59.7\t-29.4\n59.5\t-29.6\n59.3\t-29.8\n59.1\t-30\n58.9\t-30.2\n58.7\t-30.4\n58.5\t-30.6\n58.3\t-30.8\n58.1\t-31\n57.9\t-31.2\n57.7\t-31.4\n57.5\t-31.6\n57.3\t-31.8\n57.1\t-32\n56.9\t-32.2\n56.7\t-32.4\n56.5\t-32.6\n56.3\t-32.8\n56.1\t-33\n55.9\t-33.2\n55.7\t-33.4\n55.5\t-33.6\n55.3\t-33.8\n55.1\t-34\n54.9\t-34.2\n54.7\t-34.4\n54.5\t-34.6\n54.3\t-34.8\n54.1\t-35\n53.9\t-35.2\n53.7\t-35.4\n53.5\t-35.6\n53.3\t-35.8\n53.1\t-36\n52.9\t-36.2\n52.7\t-36.4\n52.5\t-36.6\n52.3\t-36.8\n52.1\t-37\n51.9\t-37.2\n51.7\t-37.4\n51.5\t-37.6\n51.3\t-37.8\n51.1\t-38\n50.9\t-38.2\n50.7\t-38.4\n50.5\t-38.6\n50.3\t-38.8\n50.1\t-39\n49.9\t-39.2\n49.7\t-39.4\n49.5\t-39.6\n49.3\t-39.8\n49.1\t-40\n48.9\t-40.2\n48.7\t-40.4\n48.5\t-40.6\n48.3\t-40.8\n48.1\t-41\n47.9\t-41.2\n47.7\t-41.4\n47.5\t-41.6\n47.3\t-41.8\n47.1\t-42\n46.9\t-42.2\n46.7\t-42.4\n46.5\t-42.6\n46.3\t-42.8\n46.1\t-43\n45.9\t-43.2\n45.7\t-43.4\n45.5\t-43.6\n45.3\t-43.8\n45.1\t-44\n44.9\t-44.2\n44.7\t-44.4\n44.5\t-44.6\n44.3\t-44.8\n44.1\t-45\n43.9\t-45.2\n43.7\t-45.4\n43.5\t-45.6\n43.3\t-45.8\n43.1\t-46\n42.9\t-46.2\n42.7\t-46.4\n42.5\t-46.6\n42.3\t-46.8\n42.1\t-47\n41.9\t-47.2\n41.7\t-47.4\n41.5\t-47.6\n41.3\t-47.8\n41.1\t-48\n40.9\t-48.2\n40.7\t-48.4\n40.5\t-48.6\n40.3\t-48.8\n40.1\t-49\n39.9\t-49.2\n39.7\t-49.4\n39.5\t-49.6\n39.3\t-49.8\n39.1\t-50\n38.9\t-50.2\n38.7\t-50.4\n38.5\t-50.6\n38.3\t-50.8\n38.1\t-51\n37.9\t-51.2\n37.7\t-51.4\n37.5\t-51.6\n37.3\t-51.8\n37.1\t-52\n36.9\t-52.2\n36.7\t-52.4\n36.5\t-52.6\n36.3\t-52.8\n36.1\t-53\n35.9\t-53.2\n35.7\t-53.4\n35.5\t-53.6\n35.3\t-53.8\n35.1\t-54\n34.9\t-54.2\n34.7\t-54.4\n34.5\t-54.6\n34.3\t-54.8\n34.1\t-55\n33.9\t-55.2\n33.7\t-55.4\n33.5\t-55.6\n33.3\t-55.8\n33.1\t-56\n32.9\t-56.2\n32.7\t-56.4\n32.5\t-56.6\n32.3\t-56.8\n32.1\t-57\n31.9\t-57.2\n31.7\t-57.4\n31.5\t-57.6\n31.3\t-57.8\n31.1\t-58\n30.9\t-58.2\n30.7\t-58.4\n30.5\t-58.6\n30.3\t-58.8\n30.1\t-59\n29.9\t-59.2\n29.7\t-59.4\n29.5\t-59.6\n29.3\t-59.8\n29.1\t-60\n28.9\t-60.2\n28.7\t-60.4\n28.5\t-60.6\n28.3\t-60.8\n28.1\t-61\n27.9\t-61.2\n27.7\t-61.4\n27.5\t-61.6\n27.3\t-61.8\n27.1\t-62\n26.9\t-62.2\n26.7\t-62.4\n26.5\t-62.6\n26.3\t-62.8\n26.1\t-63\n25.9\t-63.2\n25.7\t-63.4\n25.5\t-63.6\n25.3\t-63.8\n25.1\t-64\n24.9\t-64.2\n24.7\t-64.4\n24.5\t-64.6\n24.3\t-64.8\n24.1\t-65\n23.9\t-65.2\n23.7\t-65.4\n23.5\t-65.6\n23.3\t-65.8\n23.1\t-66\n22.9\t-66.2\n22.7\t-66.4\n22.5\t-66.6\n22.3\t-66.8\n22.1\t-67\n21.9\t-67.2\n21.7\t-67.4\n21.5\t-67.6\n21.3\t-67.8\n21.1\t-68\n20.9\t-68.2\n20.7\t-68.4\n20.5\t-68.6\n20.3\t-68.8\n20.1\t-69\n19.9\t-69.2\n19.7\t-69.4\n19.5\t-69.6\n19.3\t-69.8\n19.1\t-70\n18.9\t-70.2\n18.7\t-70.4\n18.5\t-70.6\n18.3\t-70.8\n18.1\t-71\n17.9\t-71.2\n17.7\t-71.4\n17.5\t-71.6\n17.3\t-71.8\n17.1\t-72\n16.9\t-72.2\n16.7\t-72.4\n16.5\t-72.6\n16.3\t-72.8\n16.1\t-73\n15.9\t-73.2\n15.7\t-73.4\n15.5\t-73.6\n15.3\t-73.8\n15.1\t-74\n14.9\t-74.2\n14.7\t-74.4\n14.5\t-74.6\n14.3\t-74.8\n14.1\t-75\n13.9\t-75.2\n13.7\t-75.4\n13.5\t-75.6\n13.3\t-75.8\n13.1\t-76\n12.9\t-76.2\n12.7\t-76.4\n12.5\t-76.6\n12.3\t-76.8\n12.1\t-77\n11.9\t-77.2\n11.7\t-77.4\n11.5\t-77.6\n11.3\t-77.8\n11.1\t-78\n10.9\t-78.2\n10.7\t-78.4\n10.5\t-78.6\n10.3\t-78.8\n10.1\t-79\n9.9\t-79.2\n9.7\t-79.4\n9.5\t-79.6\n9.3\t-79.8\n9.1\t-80\n8.9\t-80.2\n8.7\t-80.4\n8.5\t-80.6\n8.3\t-80.8\n8.1\t-81\n7.9\t-81.2\n7.7\t-81.4\n7.5\t-81.6\n7.3\t-81.8\n7.1\t-82\n6.9\t-82.2\n6.7\t-82.4\n6.5\t-82.6\n6.3\t-82.8\n6.1\t-83\n5.9\t-83.2\n5.7\t-83.4\n5.5\t-83.6\n5.3\t-83.8\n5.1\t-84\n4.9\t-84.2\n4.7\t-84.4\n4.5\t-84.6\n4.3\t-84.8\n4.1\t-85\n3.9\t-85.2\n3.7\t-85.4\n3.5\t-85.6\n3.3\t-85.8\n3.1\t-86\n2.9\t-86.2\n2.7\t-86.4\n2.5\t-86.6\n2.3\t-86.8\n2.1\t-87\n1.9\t-87.2\n1.7\t-87.4\n1.5\t-87.6\n1.3\t-87.8\n1.1\t-88\n0.9\t-88.2\n0.7\t-88.4\n0.5\t-88.6\n0.3\t-88.8\n0.1\t-89\n-0.1\t-89.2\n-0.3\t-89.4\n-0.5\t-89.6\n-0.7\t-89.8\n-0.9\t-90\n-1.1\t-90.2\n-1.3\t-90.4\n-1.5\t-90.6\n-1.7\t-90.8\n-1.9\t-91\n-2.1\t-91.2\n-2.3\t-91.4\n-2.5\t-91.6\n-2.7\t-91.8\n-2.9\t-92\n-3.1\t-92.2\n-3.3\t-92.4\n-3.5\t-92.6\n-3.7\t-92.8\n-3.9\t-93\n-4.1\t-93.2\n-4.3\t-93.4\n-4.5\t-93.6\n-4.7\t-93.8\n-4.9\t-94\n-5.1\t-93.6\n-5.3\t-93.2\n-5.5\t-92.8\n-5.7\t-92.4\n-5.9\t-92\n-6.1\t-91.6\n-6.3\t-91.2\n-6.5\t-90.8\n-6.7\t-90.4\n-6.9\t-90\n-7.1\t-89.6\n-7.3\t-89.2\n-7.5\t-88.8\n-7.7\t-88.4\n-7.9\t-88\n-8.1\t-87.6\n-8.3\t-87.2\n-8.5\t-86.8\n-8.7\t-86.4\n-8.9\t-86\n-9.1\t-85.6\n-9.3\t-85.2\n-9.5\t-84.8\n-9.7\t-84.4\n-9.9\t-84\n-10.1\t-83.6\n-10.3\t-83.2\n-10.5\t-82.8\n-10.7\t-82.4\n-10.9\t-82\n-11.1\t-81.6\n-11.3\t-81.2\n-11.5\t-80.8\n-11.7\t-80.4\n-11.9\t-80\n-12.1\t-79.6\n-12.3\t-79.2\n-12.5\t-78.8\n-12.7\t-78.4\n-12.9\t-78\n-13.1\t-77.6\n-13.3\t-77.2\n-13.5\t-76.8\n-13.7\t-76.4\n-13.9\t-76\n-14.1\t-75.6\n-14.3\t-75.2\n-14.5\t-74.8\n-14.7\t-74.4\n-14.9\t-74\n-15.1\t-73.6\n-15.3\t-73.2\n-15.5\t-72.8\n-15.7\t-72.4\n-15.9\t-72\n-16.1\t-71.6\n-16.3\t-71.2\n-16.5\t-70.8\n-16.7\t-70.4\n-16.9\t-70\n-17.1\t-69.6\n-17.3\t-69.2\n-17.5\t-68.8\n-17.7\t-68.4\n-17.9\t-68\n-18.1\t-67.6\n-18.3\t-67.2\n-18.5\t-66.8\n-18.7\t-66.4\n-18.9\t-66\n-19.1\t-65.6\n-19.3\t-65.2\n-19.5\t-64.8\n-19.7\t-64.4\n-19.9\t-64\n-20.1\t-63.6\n-20.3\t-63.2\n-20.5\t-62.8\n-20.7\t-62.4\n-20.9\t-62\n-21.1\t-61.6\n-21.3\t-61.2\n-21.5\t-60.8\n-21.7\t-60.4\n-21.9\t-60\n-22.1\t-59.6\n-22.3\t-59.2\n-22.5\t-58.8\n-22.4\t-58.4\n-22.3\t-58\n-22.2\t-57.6\n-22.1\t-57.2\n-22\t-56.8\n-21.9\t-56.4\n-21.8\t-56\n-21.7\t-55.6\n-21.6\t-55.2\n-21.5\t-54.8\n-21.4\t-54.4\n-21.3\t-54\n-21.2\t-53.6\n-21.1\t-53.2\n-21\t-52.8\n-20.9\t-52.4\n-20.8\t-52\n-20.7\t-51.6\n-20.6\t-51.2\n-20.5\t-50.8\n-20.4\t-50.4\n-20.3\t-50\n-20.2\t-49.6\n-20.1\t-49.2\n-20\t-48.8\n-19.9\t-48.4\n-19.8\t-48\n-19.7\t-47.6\n-19.6\t-47.2\n-19.5\t-46.8\n-19.4\t-46.4\n-19.3\t-46\n-19.2\t-45.6\n-19.1\t-45.2\n-19\t-44.8\n-18.9\t-44.4\n-18.8\t-44\n-18.7\t-43.6\n-18.6\t-43.2\n-18.5\t-42.8\n-18.4\t-42.4\n-18.3\t-42\n-18.2\t-41.6\n-18.1\t-41.2\n-18\t-40.8\n-17.9\t-40.4\n-17.8\t-40\n-17.7\t-39.6\n-17.6\t-39.2\n-17.5\t-38.8\n-17.4\t-38.4\n-17.3\t-38\n-17.2\t-37.6\n-17.1\t-37.2\n-17\t-36.8\n-16.9\t-36.4\n-16.8\t-36\n-16.2\t-35.6\n-15.6\t-35.2\n-15\t-34.8\n-14.4\t-34.4\n-13.8\t-34\n-13.2\t-33.6\n-12.6\t-33.2\n-12\t-32.8\n-11.4\t-32.4\n-10.8\t-32\n-10.2\t-31.6\n-9.6\t-31.2\n-9\t-30.8\n-8.4\t-30.4\n-7.8\t-30\n-7.2\t-29.6\n-6.6\t-29.2\n-6\t-28.8\n-5.4\t-28.4\n-4.8\t-28\n-4.2\t-27.6\n-3.6\t-27.2\n-3\t-26.8\n-2.4\t-26.4\n-1.8\t-26\n-1.2\t-25.6\n-0.6\t-25.2\n-3.22831E-12\t-24.8\n-0.6\t-24.4\n-1.2\t-24\n-1.8\t-23.6\n-2.4\t-23.2\n-3\t-22.8\n-3.6\t-22.4\n-4.2\t-22\n-4.8\t-21.6\n-5.4\t-21.2\n-6\t-20.8\n-6.6\t-20.4\n-7.2\t-20\n-7.8\t-19.6\n-8.4\t-19.2\n-9\t-18.8\n-9.6\t-18.4\n-10.2\t-18\n-10.8\t-17.6\n-11.4\t-17.2\n-12\t-16.8\n-12.6\t-16.4\n-13.2\t-16\n-13.8\t-15.6\n-14.4\t-15.2\n-15\t-14.8\n-15.6\t-14.4\n-16.2\t-14\n-16.8\t-13.6\n-17.4\t-13.2\n-18\t-12.8\n-18.6\t-12.4\n-19.2\t-12\n-19.8\t-11.6\n-20.4\t-11.2\n-21\t-10.8\n-21.6\t-10.4\n-22.2\t-10\n-22.8\t-9.6\n-23.4\t-9.2\n-24\t-8.8\n-24.6\t-8.4\n-25.2\t-8\n-25.8\t-7.6\n-26.4\t-7.2\n-27\t-6.8\n-27.6\t-6.4\n-28.2\t-6\n-28.8\t-5.6\n-29.4\t-5.2\n-30\t-4.8\n-30.6\t-4.4\n-31.2\t-4\n-31.8\t-3.6\n-32.4\t-3.2\n-33\t-2.8\n-33.6\t-2.4\n-34.2\t-2\n-34.8\t-1.6\n-35.4\t-1.2\n-36\t-0.8\n-36.6\t-0.4\n-37.2\t0\n-37.8\t0\n-38.4\t0.3\n-39\t0.6\n-39.6\t0.9\n-40.2\t1.2\n-40.8\t1.5\n-41.4\t1.8\n-42\t2.1\n-42.6\t2.4\n-43.2\t2.7\n-43.8\t3\n-44.4\t3.3\n-45\t3.6\n-45.6\t3.9\n-46.2\t4.2\n-46.8\t4.5\n-47.4\t4.8\n-48\t5.1\n-48.6\t5.4\n-49.2\t5.7\n-49.8\t6\n-50.4\t6.3\n-51\t6.6\n-51.6\t6.9\n-52.2\t7.2\n-52.8\t7.5\n-53.4\t7.8\n-54\t8.1\n-54.6\t8.4\n-55.2\t8.7\n-55.8\t9\n-56.4\t9.3\n-57\t9.6\n-57.6\t9.9\n-58.2\t10.2\n-58.8\t10.5\n-59.4\t10.8\n-60\t11.1\n-60.6\t11.4\n-61.2\t11.7\n-61.8\t12\n-62.4\t12.3\n-63\t12.6\n-63.6\t12.9\n-64.2\t13.2\n-64.8\t13.5\n-65.4\t13.8\n-66\t14.1\n-66.6\t14.4\n-67.2\t14.7\n-67.8\t15\n-68.4\t15.3\n-69\t15.6\n-69.6\t15.9\n-70.2\t16.2\n-70.8\t16.5\n-71.4\t16.8\n-72\t17.1\n-72.6\t17.4\n-73.2\t17.7\n-73.8\t18\n-74.4\t18.3\n-75\t18.6\n-75.6\t18.9\n-76.2\t19.2\n-76.8\t19.5\n-77.4\t19.8\n-78\t20.1\n-78.6\t20.4\n-79.2\t20.7\n-79.8\t21\n-80.4\t21.3\n-81\t21.6\n-81.6\t21.9\n-82.2\t22.2\n-82.8\t22.5\n-83.4\t22.8\n-84\t23.1\n-84.6\t23.4\n-85.2\t23.7\n-85.8\t24\n-86.4\t24.3\n-87\t24.6\n-87.6\t24.9\n-88.2\t25.2\n-88.8\t25.5\n-89.4\t25.8\n-90\t26.1\n-89.8\t26.4\n-89.6\t26.7\n-89.4\t27\n-89.2\t27.3\n-89\t27.6\n-88.8\t27.9\n-88.6\t28.2\n-88.4\t28.5\n-88.2\t28.8\n-88\t29.1\n-87.8\t29.4\n-87.6\t29.7\n-87.4\t30\n-87.2\t30.3\n-87\t30.6\n-86.8\t30.9\n-86.6\t31.2\n-86.4\t31.5\n-86.2\t31.8\n-86\t32.1\n-85.8\t32.4\n-85.6\t32.7\n-85.4\t33\n-85.2\t33.3\n-85\t33.6\n-84.8\t33.9\n-84.6\t34.2\n-84.4\t34.5\n-84.2\t34.8\n-84\t35.1\n-83.8\t35.4\n-83.6\t35.7\n-83.4\t36\n-83.2\t36.3\n-83\t36.6\n-82.8\t36.9\n-82.6\t37.2\n-82.4\t37.5\n-82.2\t37.8\n-82\t38.1\n-81.8\t38.4\n-81.6\t38.7\n-81.4\t39\n-81.2\t39.3\n-81\t39.6\n-80.8\t39.9\n-80.6\t40.2\n-80.4\t40.5\n-80.2\t40.8\n-80\t41.1\n-79.8\t41.4\n-79.6\t41.7\n-79.4\t42\n-79.2\t42.3\n-79\t42.6\n-78.8\t42.9\n-78.6\t43.2\n-78.4\t43.5\n-78.2\t43.8\n-78\t44.1\n-77.8\t44.4\n-77.6\t44.7\n-77.4\t45\n-77.2\t45.3\n-77\t45.6\n-76.8\t45.9\n-76.6\t46.2\n-76.4\t46.5\n-76.2\t46.8\n-76\t47.1\n-75.8\t47.4\n-75.6\t47.7\n-75.4\t48\n-75.2\t48.3\n-75\t48.6\n-74.8\t48.9\n-74.6\t49.2\n-74.4\t49.5\n-74.2\t49.8\n-74\t50.1\n-73.8\t50.4\n-73.6\t50.7\n-73.4\t51\n-73.2\t51.3\n-73\t51.6\n-72.8\t51.9\n-72.6\t52.2\n-72.4\t52.5\n-72.2\t52.8\n-72\t53.1\n-71.8\t53.4\n-71.6\t53.7\n-71.4\t54\n-71.2\t54.3\n-71\t54.6\n-70.8\t54.9\n-70.6\t55.2\n-70.4\t55.5\n-70.2\t55.8\n-70\t56.1\n-69.8\t56.4\n-69.6\t56.7\n-69.4\t57\n-69.2\t57.3\n-69\t57.6\n-68.8\t57.9\n-68.6\t58.2\n-68.4\t58.5\n-68.2\t58.8\n-68\t59.1\n-67.8\t59.4\n-67.6\t59.7\n-67.4\t60\n-67.2\t60.3\n-67\t60.6\n-66.8\t60.9\n-66.6\t61.2\n-66.4\t61.5\n-66.2\t61.8\n-66\t62.1\n-65.8\t62.4\n-65.6\t62.7\n-65.4\t63\n-65.2\t63.3\n-65\t63.6\n-64.8\t63.9\n-64.6\t64.2\n-64.4\t64.5\n-64.2\t64.8\n-64\t65.1\n-63.8\t65.4\n-63.6\t65.7\n-63.4\t66\n-63.2\t66.3\n-63\t66.6\n-62.8\t66.9\n-62.6\t67.2\n-62.4\t67.5\n-62.2\t67.8\n-62\t68.1\n-61.8\t68.4\n-61.6\t68.7\n-61.4\t69\n-61.2\t69.3\n-61\t69.6\n-60.8\t69.9\n-60.6\t70.2\n-60.4\t70.5\n-60.2\t70.8\n-60\t71.1\n-59.8\t71.4\n-59.6\t71.7\n-59.4\t72\n-59.2\t72.3\n-59\t72.6\n-58.8\t72.9\n-58.6\t73.2\n-58.4\t73.5\n-58.2\t73.8\n-58\t74.1\n-57.8\t74.4\n-57.6\t74.7\n-57.4\t75\n-57.2\t75.3\n-57\t75.6\n-56.8\t75.9\n-56.6\t76.2\n-56.4\t76.5\n-56.2\t76.8\n-56\t77.1\n-55.8\t77.4\n-55.6\t77.7\n-55.4\t78\n-55.2\t78.3\n-55\t78.6\n-54.8\t78.9\n-54.6\t79.2\n-54.4\t79.5\n-54.2\t79.8\n-54\t80.1\n-53.8\t80.4\n-53.6\t80.7\n-53.4\t81\n-53.2\t81.3\n-53\t81.6\n-52.8\t81.9\n-52.6\t82.2\n-52.4\t82.5\n-52.2\t82.8\n-52\t83.1\n-51.8\t83.4\n-51.6\t83.7\n-51.4\t84\n-51.2\t84.3\n-51\t84.6\n-50.8\t84.9\n-50.6\t85.2\n-50.4\t85.5\n-50.2\t85.8\n-50\t86.1\n-49.8\t86.4\n-49.6\t86.7\n-49.4\t87\n-49.2\t87.3\n-49\t87.6\n-48.8\t87.9\n-48.6\t88.2\n-48.4\t88.5\n-48.2\t88.8\n-48\t89.1\n-47.8\t89.4\n-47.6\t89.7\n-47.4\t90\n-47.2\t90.3\n-47\t90.6\n-46.8\t90.9\n-46.6\t91.2\n-46.4\t91.5\n-46.2\t91.8\n-46\t92.1\n-45.8\t92.4\n-45.6\t92.7\n-45.4\t93\n-45.2\t93.3\n-45\t93.6\n-44.8\t93.9\n-44.6\t94.2\n-44.4\t94.5\n-44.2\t94.8\n-44\t95.1\n-43.8\t95.4\n-43.6\t95.7\n-43.4\t96\n-43.2\t96.3\n-43\t96.6\n-42.8\t96.9\n-42.6\t97.2\n-42.4\t97.5\n-42.2\t97.3\n-42\t97.1\n-41.8\t96.9\n-41.6\t96.7\n-41.4\t96.5\n-41.2\t96.3\n-41\t96.1\n-40.8\t95.9\n-40.6\t95.7\n-40.4\t95.5\n-40.2\t95.3\n-40\t95.1\n-39.8\t94.9\n-39.6\t94.7\n-39.4\t94.5\n-39.2\t94.3\n-39\t94.1\n-38.8\t93.9\n-38.6\t93.7\n-38.4\t93.5\n-38.2\t93.3\n-38\t93.1\n-37.8\t92.9\n-37.6\t92.7\n-37.4\t92.5\n-37.2\t92.3\n-37\t92.1\n-36.8\t91.9\n-36.6\t91.7\n-36.4\t91.5\n-36.2\t91.3\n-36\t91.1\n-35.8\t90.9\n-35.6\t90.7\n-35.4\t90.5\n-35.2\t90.3\n-35\t90.1\n-34.8\t89.9\n-34.6\t89.7\n-34.4\t89.5\n-34.2\t89.3\n-34\t89.1\n-33.8\t88.9\n-33.6\t88.7\n-33.4\t88.5\n-33.2\t88.3\n-33\t88.1\n-32.8\t87.9\n-32.6\t87.7\n-32.4\t87.5\n-32.2\t87.3\n-32\t87.1\n-31.8\t86.9\n-31.6\t86.7\n-31.4\t86.5\n-31.2\t86.3\n-31\t86.1\n-30.8\t85.9\n-30.6\t85.7\n-30.4\t85.5\n-30.2\t85.3\n-30\t85.1\n-29.8\t84.9\n-29.6\t84.7\n-29.4\t84.5\n-29.2\t84.3\n-29\t84.1\n-28.8\t83.9\n-28.6\t83.7\n-28.4\t83.5\n-28.2\t83.3\n-28\t83.1\n-27.8\t82.9\n-27.6\t82.7\n-27.4\t82.5\n-27.2\t82.3\n-27\t82.1\n-26.8\t81.9\n-26.6\t81.7\n-26.4\t81.5\n-26.2\t81.3\n-26\t81.1\n-25.8\t80.9\n-25.6\t80.7\n-25.4\t80.5\n-25.2\t80.3\n-25\t80.1\n-24.8\t79.9\n-24.6\t79.7\n-24.4\t79.5\n-24.2\t79.3\n-24\t79.1\n-23.8\t78.9\n-23.6\t78.7\n-23.4\t78.5\n-23.2\t78.3\n-23\t78.1\n-22.8\t77.9\n-22.6\t77.7\n-22.4\t77.5\n-22.2\t77.3\n-22\t77.1\n-21.8\t76.9\n-21.6\t76.7\n-21.4\t76.5\n-21.2\t76.3\n-21\t76.1\n-20.8\t75.9\n-20.6\t75.7\n-20.4\t75.5\n-20.2\t75.3\n-20\t75.1\n-19.8\t74.9\n-19.6\t74.7\n-19.4\t74.5\n-19.2\t74.3\n-19\t74.1\n-18.8\t73.9\n-18.6\t73.7\n-18.4\t73.5\n-18.2\t73.3\n-18\t73.1\n-17.8\t72.9\n-17.6\t72.7\n-17.4\t72.5\n-17.2\t72.3\n-17\t72.1\n-16.8\t71.9\n-16.6\t71.7\n-16.4\t71.5\n-16.2\t71.3\n-16\t71.1\n-15.8\t70.9\n-15.6\t70.7\n-15.4\t70.5\n-15.2\t70.3\n-15\t70.1\n-14.8\t69.9\n-14.6\t69.7\n-14.4\t69.5\n-14.2\t69.3\n-14\t69.1\n-13.8\t68.9\n-13.6\t68.7\n-13.4\t68.5\n-13.2\t68.3\n-13\t68.1\n-12.8\t67.9\n-12.6\t67.7\n-12.4\t67.5\n-12.2\t67.3\n-12\t67.1\n-11.8\t66.9\n-11.6\t66.7\n-11.4\t66.5\n-11.2\t66.3\n-11\t66.1\n-10.8\t65.9\n-10.6\t65.7\n-10.4\t65.5\n-10.2\t65.3\n-10\t65.1\n-9.8\t64.9\n-9.6\t64.7\n-9.4\t64.5\n-9.2\t64.3\n-9\t64.1\n-8.8\t63.9\n-8.6\t63.7\n-8.4\t63.5\n-8.2\t63.3\n-8\t63.1\n-7.8\t62.9\n-7.6\t62.7\n-7.4\t62.5\n-7.2\t62.3\n-7\t62.1\n-6.8\t61.9\n-6.6\t61.7\n-6.4\t61.5\n-6.2\t61.3\n-6\t61.1\n-5.8\t60.9\n-5.6\t60.7\n-5.4\t60.5\n-5.2\t60.3\n-5\t60.1\n-4.8\t59.9\n-4.6\t59.7\n-4.4\t59.5\n-4.2\t59.3\n-4\t59.1\n-3.8\t58.9\n-3.6\t58.7\n-3.4\t58.5\n-3.2\t58.3\n-3\t58.1\n-2.8\t57.9\n-2.6\t57.7\n-2.4\t57.5\n-2.2\t57.3\n-2\t57.1\n-1.8\t56.9\n-1.6\t56.7\n-1.4\t56.5\n-1.2\t56.3\n-1\t56.1\n-0.8\t55.9\n-0.6\t55.7\n-0.4\t55.5\n-0.2\t55.3\n-2.33974E-12\t55.1\n0.2\t54.9\n0.4\t54.7\n0.6\t54.5\n0.8\t54.3\n1\t54.1\n1.2\t53.9\n1.4\t53.7\n1.6\t53.5\n1.8\t53.3\n2\t53.1\n2.2\t52.9\n2.4\t52.7\n2.6\t52.5\n2.8\t52.3\n3\t52.1\n3.2\t51.9\n3.4\t51.7\n3.6\t51.5\n3.8\t51.3\n4\t51.1\n4.2\t50.9\n4.4\t50.7\n4.6\t50.5\n4.8\t50.3\n5\t50.1\n5.2\t49.9\n5.4\t49.7\n5.6\t49.5\n5.8\t49.3\n6\t49.1\n6.2\t48.9\n6.4\t48.7\n6.6\t48.5\n6.8\t48.3\n7\t48.1\n7.2\t47.9\n7.4\t47.7\n7.6\t47.5\n7.8\t47.3\n8\t47.1\n8.2\t46.9\n8.4\t46.7\n8.6\t46.5\n8.8\t46.3\n9\t46.1\n9.2\t45.9\n9.4\t45.7\n9.6\t45.5\n9.8\t45.3\n10\t45.1\n10.2\t44.9\n10.4\t44.7\n10.6\t44.5\n10.8\t44.3\n11\t44.1\n11.2\t43.9\n11.4\t43.7\n11.6\t43.5\n11.8\t43.3\n12\t43.1\n12.2\t42.9\n12.4\t42.7\n12.6\t42.5\n12.8\t42.3\n13\t42.1\n13.2\t41.9\n13.4\t41.7\n13.6\t41.5\n13.8\t41.3\n14\t41.1\n14.2\t40.9\n14.4\t40.7\n14.6\t40.5\n14.8\t40.3\n15\t40.1\n15.2\t39.9\n15.4\t39.7\n15.6\t39.5\n15.8\t39.3\n16\t39.1\n16.2\t38.9\n16.4\t38.7\n16.6\t38.5\n16.8\t38.3\n17\t38.1\n17.2\t37.9\n17.4\t37.7\n17.6\t37.5\n17.8\t37.3\n18\t37.1\n18.2\t36.9\n18.4\t36.7\n18.6\t36.5\n18.8\t36.3\n19\t36.1\n19.2\t35.9\n19.4\t35.7\n19.6\t35.5\n19.8\t35.3\n20\t35.1\n20.2\t34.9\n20.4\t34.7\n20.6\t34.5\n20.8\t34.3\n21\t34.1\n21.2\t33.9\n21.4\t33.7\n21.6\t33.5\n21.8\t33.3\n22\t33.1\n22.2\t32.9\n22.4\t32.7\n22.6\t32.5\n22.8\t32.3\n23\t32.1\n23.2\t31.9\n23.4\t31.7\n23.6\t31.5\n23.8\t31.3\n24\t31.1\n24.2\t30.9\n24.4\t30.7\n24.6\t30.5\n24.8\t30.3\n25\t30.1\n25.2\t29.9\n25.4\t29.7\n25.6\t29.5\n25.8\t29.3\n26\t29.1\n26.2\t28.9\n26.4\t28.7\n26.6\t28.5\n26.8\t28.3\n27\t28.1\n27.2\t27.9\n27.4\t27.7\n27.6\t27.5\n27.8\t27.3\n28\t27.1\n28.2\t26.9\n28.4\t26.7\n28.6\t26.5\n28.8\t26.3\n29\t26.1\n29.2\t25.9\n29.4\t25.7\n29.6\t25.5\n29.8\t25.3\n30\t25.1\n30.2\t24.9\n30.4\t24.7\n30.6\t24.5\n30.8\t24.3\n31\t24.1\n31.2\t23.9\n31.4\t23.7\n31.6\t23.5\n31.8\t23.3\n32\t23.1\n32.2\t22.9\n32.4\t22.7\n32.6\t22.5\n32.8\t22.3\n33\t22.1\n33.2\t21.9\n33.4\t21.7\n33.6\t21.5\n33.8\t21.3\n34\t21.1\n34.2\t20.9\n34.4\t20.7\n34.6\t20.5\n34.8\t20.3\n35\t20.1\n35.2\t19.9\n35.4\t19.7\n35.6\t19.5\n35.8\t19.3\n36\t19.1\n36.2\t18.9\n36.4\t18.7\n36.6\t18.5\n36.8\t18.3\n37\t18.1\n37.2\t17.9\n37.4\t17.7\n37.6\t17.5\n37.8\t17.3\n38\t17.1\n38.2\t16.9\n38.4\t16.7\n38.6\t16.5\n38.8\t16.3\n39\t16.1\n39.2\t15.9\n39.4\t15.7\n39.6\t15.5\n39.8\t15.3\n40\t15.1\n40.2\t14.9\n40.4\t14.7\n40.6\t14.5\n40.8\t14.3\n41\t14.1\n41.2\t13.9\n41.4\t13.7\n41.6\t13.5\n41.8\t13.3\n42\t13.1\n42.2\t12.9\n42.4\t12.7\n42.6\t12.5\n42.8\t12.3\n43\t12.1\n43.2\t11.9\n43.4\t11.7\n43.6\t11.5\n43.8\t11.3\n44\t11.1\n44.2\t10.9\n44.4\t10.7\n44.6\t11.3\n44.8\t11.9\n45\t12.5\n45.2\t13.1\n45.4\t13.7\n45.6\t14.3\n45.8\t14.9\n46\t15.5\n46.2\t16.1\n46.4\t16.7\n46.6\t17.3\n46.8\t17.9\n47\t18.5\n47.2\t19.1\n47.4\t19.7\n47.6\t20.3\n47.8\t20.9\n48\t21.5\n48.2\t22.1\n48.4\t22.7\n48.6\t23.3\n48.8\t23.9\n49\t24.5\n49.2\t25.1\n49.4\t25.7\n49.6\t26.3\n49.8\t26.9\n50\t27.5\n50.2\t28.1\n50.4\t28.7\n50.6\t29.3\n50.8\t29.9\n51\t30.5\n51.2\t31.1\n51.4\t31.7\n51.6\t32.3\n51.8\t32.9\n52\t33.5\n52.2\t34.1\n52.4\t34.7\n52.6\t35.3\n52.8\t35.9\n53\t36.5\n53.2\t37.1\n53.4\t37.7\n53.6\t38.3\n53.8\t38.9\n54\t39.5\n54.2\t40.1\n54.4\t40.7\n54.6\t41.3\n54.8\t41.9\n55\t42.5\n55.2\t43.1\n55.4\t43.7\n55.6\t44.3\n55.8\t44.9\n56\t45.5\n56.2\t46.1\n56.4\t46.7\n56.6\t47.3\n56.8\t47.9\n57\t48.5\n57.2\t49.1\n57.4\t49.7\n57.6\t50.3\n57.8\t50.9\n58\t51.5\n58.2\t52.1\n58.4\t52.7\n58.6\t53.3\n58.8\t53.9\n59\t54.5\n59.2\t55.1\n59.4\t55.7\n59.6\t56.3\n59.8\t56.9\n60\t57.5\n60.2\t58.1\n60.4\t58.7\n60.6\t59.3\n60.8\t59.9\n61\t60.5\n61.2\t61.1\n61.4\t61.7\n61.6\t62.3\n61.8\t62.9\n62\t63.5\n62.2\t64.1\n62.4\t64.7\n62.6\t65.3\n62.8\t65.9\n63\t66.5\n63.2\t67.1\n63.4\t67.7\n63.6\t68.3\n63.8\t68.9\n64\t69.5\n64.2\t70.1\n64.4\t70.7\n64.6\t71.3\n64.8\t71.9\n65\t72.5\n65.2\t73.1\n65.4\t73.7\n65.6\t74.3\n65.8\t74.9\n66\t75.5\n66.2\t76.1\n66.4\t76.7\n66.6\t77.3\n66.8\t77.9\n67\t78.5\n67.2\t79.1\n67.4\t79.7\n67\t80.3\n66.6\t80.9\n66.2\t81.5\n65.8\t82.1\n65.4\t82.7\n65\t83.3\n64.6\t83.9\n64.2\t84.5\n63.8\t85.1\n63.4\t85.7\n63\t86.3\n62.6\t86.9\n62.2\t87.5\n61.8\t88.1\n61.4\t88.7\n61\t89.3\n60.6\t89.9\n60.2\t90.5\n59.8\t91.1\n59.4\t91.7\n59\t92.3\n58.6\t92.9\n58.2\t93.5\n57.8\t94.1\n57.4\t93.8\n57\t93.5\n56.6\t93.2\n56.2\t92.9\n55.8\t92.6\n55.4\t92.3\n55\t92\n54.6\t91.7\n54.2\t91.4\n53.8\t91.1\n53.4\t90.8\n53\t90.5\n52.6\t90.2\n52.2\t89.9\n51.8\t89.6\n51.4\t89.3\n51\t89\n50.6\t88.7\n50.2\t88.4\n49.8\t88.1\n49.4\t87.8\n49\t87.5\n48.6\t87.2\n48.2\t86.9\n47.8\t86.6\n47.4\t86.3\n47\t86\n46.6\t85.7\n46.2\t85.4\n45.8\t85.1\n45.4\t84.8\n45\t84.5\n44.6\t84.2\n44.2\t83.9\n43.8\t83.6\n43.4\t83.3\n43\t83\n42.6\t82.7\n42.2\t82.4\n41.8\t82.1\n41.4\t81.8\n41\t81.5\n40.6\t81.2\n40.2\t80.9\n39.8\t80.6\n39.4\t80.3\n39\t80\n38.6\t79.7\n38.2\t79.4\n37.8\t79.1\n37.4\t78.8\n37\t78.5\n36.6\t78.2\n36.2\t77.9\n35.8\t77.6\n35.4\t77.3\n35\t77\n34.6\t76.7\n34.2\t76.4\n33.8\t76.1\n33.4\t75.8\n33\t75.5\n32.6\t75.2\n32.2\t74.9\n31.8\t74.6\n31.4\t74.3\n31\t74\n30.6\t73.7\n30.2\t73.4\n29.8\t73.1\n29.4\t72.8\n29\t72.5\n28.6\t72.2\n28.2\t71.9\n27.8\t71.6\n27.4\t71.3\n27\t71\n26.6\t70.7\n26.2\t70.4\n25.8\t70.1\n25.4\t69.8\n25\t69.5\n24.6\t69.2\n24.2\t68.9\n23.8\t68.6\n23.4\t68.3\n23\t68\n22.6\t67.7\n22.2\t67.4\n21.8\t67.1\n21.4\t66.8\n21\t66.5\n20.6\t66.2\n20.2\t65.9\n19.8\t65.6\n19.4\t65.3\n19\t65\n18.6\t64.7\n18.2\t64.4\n17.8\t64.1\n17.4\t63.8\n17\t63.5\n16.6\t63.2\n16.2\t62.9\n15.8\t62.6\n15.4\t62.3\n15\t62\n14.6\t61.7\n14.2\t61.4\n13.8\t61.1\n13.4\t60.8\n13\t60.5\n12.6\t60.2\n12.2\t59.9\n11.8\t59.6\n11.4\t59.3\n11\t59\n10.6\t58.7\n10.2\t58.4\n9.8\t58.1\n9.4\t57.8\n9\t57.5\n8.6\t57.2\n8.2\t56.9\n7.8\t56.6\n7.4\t56.3\n7\t56\n6.6\t55.7\n6.2\t55.4\n5.8\t55.1\n5.4\t54.8\n5\t54.5\n4.6\t54.2\n4.2\t53.9\n3.8\t53.6\n3.4\t53.3\n3\t53\n2.6\t52.7\n2.2\t52.4\n1.8\t52.1\n1.4\t51.8\n1\t51.5\n0.6\t51.2\n0.2\t50.9\n-0.2\t50.6\n-0.6\t50.3\n-1\t50\n-1.4\t49.7\n-1.8\t49.4\n-2.2\t49.1\n-2.6\t48.8\n-3\t48.5\n-3.4\t48.2\n-3.8\t47.9\n-4.2\t47.6\n-4.6\t47.3\n-5\t47\n-5.4\t46.7\n-5.8\t46.4\n-6.2\t46.1\n-6.6\t45.8\n-7\t45.5\n-7.4\t45.2\n-7.8\t44.9\n-8.2\t44.6\n-8.6\t44.3\n-9\t44\n-9.4\t43.7\n-9.8\t43.4\n-10.2\t43.1\n-10.6\t42.8\n-11\t42.5\n-11.4\t42.2\n-11.8\t41.9\n-12.2\t41.6\n-12.6\t41.3\n-13\t41\n-13.4\t40.7\n-13.8\t40.4\n-14.2\t40.1\n-14.6\t39.8\n-15\t39.5\n-15.4\t39.2\n-15.8\t38.9\n-16.2\t38.6\n-16.6\t38.3\n-17\t38\n-17.4\t37.7\n-17.8\t37.4\n-18.2\t37.1\n-18.6\t36.8\n-19\t36.5\n-19.4\t36.2\n-19.8\t35.9\n-20.2\t35.6\n-20.6\t35.3\n-21\t35\n-21.4\t34.7\n-21.8\t34.4\n-22.2\t34.1\n-22.6\t33.8\n-23\t33.5\n-23.4\t33.2\n-23.8\t32.9\n-24.2\t32.6\n-24.6\t32.3\n-25\t32\n-25.4\t31.7\n-25.8\t31.4\n-26.2\t31.1\n-26.6\t30.8\n-27\t30.5\n-27.4\t30.2\n-27.8\t29.9\n-28.2\t29.6\n-28.6\t29.3\n-29\t29\n-29.4\t28.7\n-29.8\t28.4\n-30.2\t28.1\n-30.6\t27.8\n-31\t27.5\n-31.4\t27.2\n-31.8\t26.9\n-32.2\t26.6\n-32.6\t26.3\n-33\t26\n-33.4\t25.7\n-33.8\t25.4\n-34.2\t25.1\n-34.6\t24.8\n-35\t24.5\n-35.4\t24.2\n-35.8\t23.9\n-36.2\t23.6\n-36.6\t23.3\n-37\t23\n-37.4\t22.7\n-37.8\t22.4\n-38.2\t22.1\n-38.6\t21.8\n-39\t21.5\n-39.4\t21.2\n-39.8\t20.9\n-40.2\t20.6\n-40.6\t20.3\n-41\t20\n-41.4\t19.7\n-41.8\t19.4\n-42.2\t19.1\n-42.6\t18.8\n-43\t18.5\n-43.4\t18.2\n-43.8\t17.9\n-44.2\t17.6\n-44.6\t17.3\n-45\t17\n-45.4\t16.7\n-45.8\t16.4\n-46.2\t16.1\n-46.6\t15.8\n-47\t15.5\n-47.4\t15.2\n-47.8\t14.9\n-48.2\t14.6\n-48.6\t14.3\n-49\t14\n-49.4\t13.7\n-49.8\t13.4\n-50.2\t13.1\n-50.6\t12.8\n-51\t12.5\n-51.4\t12.2\n-51.8\t11.9\n-52.2\t11.6\n-52.6\t11.3\n-53\t11\n-53.4\t10.7\n-53.8\t10.4\n-54.2\t10.1\n-53.6\t9.8\n-53\t9.5\n-52.4\t9.2\n-51.8\t8.9\n-51.2\t8.6\n-50.6\t8.3\n-50\t8\n-49.4\t7.7\n-48.8\t7.4\n-48.2\t7.1\n-47.6\t6.8\n-47\t6.5\n-46.4\t6.2\n-45.8\t5.9\n-45.2\t5.6\n-44.6\t5.3\n-44\t5\n-43.4\t4.7\n-42.8\t4.4\n-42.2\t4.1\n-41.6\t3.8\n-41\t3.5\n-40.4\t3.2\n-39.8\t2.9\n-39.2\t2.6\n-38.6\t2.3\n-38\t2\n-37.4\t1.7\n-36.8\t1.4\n-36.2\t1.1\n-35.6\t0.8\n-35\t0.5\n-34.4\t0.2\n-33.8\t-0.1\n-33.2\t-0.4\n-32.6\t-0.7\n-32\t-1\n-31.4\t-1.3\n-30.8\t-1.6\n-30.2\t-1.9\n-29.6\t-2.2\n-29\t-2.5\n-28.4\t-2.8\n-27.8\t-3.1\n-27.2\t-3.4\n-26.6\t-3.7\n-26\t-4\n-25.4\t-4.3\n-24.8\t-4.6\n-24.2\t-4.9\n-23.6\t-5.2\n-23\t-5.5\n-22.4\t-5.8\n-21.8\t-6.1\n-21.2\t-6.4\n-20.6\t-6.7\n-20\t-7\n-19.4\t-7.3\n-18.8\t-7.6\n-18.2\t-7.9\n-17.6\t-8.2\n-17\t-8.5\n-16.4\t-8.8\n-15.8\t-9.1\n-15.2\t-9.4\n-14.6\t-9.7\n-14\t-10\n-13.4\t-10.3\n-12.8\t-10.6\n-12.2\t-10.9\n-11.6\t-11.2\n-11\t-11.5\n-10.4\t-11.8\n-9.8\t-12.1\n-9.2\t-12.4\n-8.6\t-12.7\n-8\t-13\n-7.4\t-13.3\n-6.8\t-13.6\n-6.2\t-13.9\n-5.6\t-14.2\n-5\t-14.5\n-4.4\t-14.8\n-3.8\t-15.1\n-3.2\t-15.4\n-2.6\t-15.7\n-2\t-16\n-1.4\t-16.3\n-0.8\t-16.6\n-0.2\t-16.9\n0.4\t-17.2\n1\t-17.5\n1.6\t-17.8\n2.2\t-18.1\n2.8\t-18.4\n3.4\t-18.7\n4\t-19\n4.6\t-19.3\n5.2\t-19.6\n5.8\t-19.9\n6.4\t-20.2\n7\t-20.5\n7.6\t-20.8\n8.2\t-21.1\n8.8\t-21.4\n9.4\t-21.7\n10\t-22\n10.6\t-22.3\n11.2\t-22.6\n11.8\t-22.9\n12.4\t-23.2\n13\t-23.5\n13.6\t-23.8\n14.2\t-24.1\n14.8\t-24.4\n15.4\t-24.7\n16\t-25\n16.6\t-25.3\n17.2\t-25.6\n17.8\t-25.9\n18.4\t-26.2\n19\t-26.5\n19.6\t-26.8\n20.2\t-27.1\n20.8\t-27.4\n21.4\t-27.7\n22\t-28\n22.6\t-28.3\n23.2\t-28.6\n23.8\t-28.9\n24.4\t-29.2\n25\t-29.5\n25.6\t-29.8\n26.2\t-30.1\n26.8\t-30.4\n27.4\t-30.7\n28\t-31\n28.6\t-31.3\n29.2\t-31.6\n29.8\t-31.9\n30.4\t-32.2\n31\t-32.5\n31.6\t-32.8\n32.2\t-33.1\n32.8\t-33.4\n33.4\t-33.7\n34\t-34\n34.6\t-34.3\n35.2\t-34.6\n35.8\t-34.9\n36.4\t-35.2\n37\t-35.5\n37.6\t-35.8\n38.2\t-36.1\n38.8\t-36.4\n39.4\t-36.7\n40\t-37\n40.6\t-37.3\n41.2\t-37.6\n41.8\t-37.9\n42.4\t-38.2\n43\t-38.5\n43.6\t-38.8\n44.2\t-39.1\n44.8\t-39.4\n45.4\t-39.7\n46\t-40\n46.6\t-40.3\n47.2\t-40.6\n47.8\t-40.9\n48.4\t-41.2\n49\t-41.5\n49.6\t-41.8\n50.2\t-42.1\n50.8\t-42.4\n51.4\t-42.7\n52\t-43\n52.6\t-43.3\n53.2\t-43.6\n53.8\t-43.9\n54.4\t-44.2\n55\t-44.5\n55.6\t-44.8\n56.2\t-45.1\n56.8\t-45.4\n57.4\t-45.7\n58\t-46\n58.6\t-46.3\n59.2\t-46.6\n59.8\t-46.9\n60.4\t-47.2\n61\t-47.5\n61.6\t-47.8\n62.2\t-48.1\n62.8\t-48.4\n63.4\t-48.7\n64\t-49\n64.6\t-49.3\n65.2\t-49.6\n65.8\t-49.9\n66.4\t-50.2\n67\t-50.5\n67.6\t-50.8\n68.2\t-51.1\n68.8\t-51.4\n69.4\t-51.7\n70\t-52\n70.6\t-52.3\n71.2\t-52.6\n71.8\t-52.9\n72.4\t-53.2\n73\t-53.5\n73.6\t-53.8\n74.2\t-54.1\n74.8\t-54.4\n75.4\t-54.7\n76\t-55\n76.6\t-55.3\n77.2\t-55.6\n77.8\t-55.9\n78.4\t-56.2\n79\t-56.5\n79.6\t-56.8\n80.2\t-57.1\n80.8\t-57.4\n81.4\t-57.7\n82\t-58\n82.6\t-58.3\n83.2\t-58.6\n83.8\t-58.9\n84.4\t-59.2\n85\t-59.5\n85.6\t-59.8\n86.2\t-60.1\n86.8\t-60.4\n87.4\t-60.7\n88\t-61\n88.6\t-61.3\n89.2\t-61.6\n89.8\t-61.9\n90.4\t-62.2\n91\t-62.5\n91.6\t-62.8\n92.2\t-63.1\n92.8\t-63.4\n93.4\t-63.7\n94\t-64\n94.6\t-64.3\n95.2\t-64.6\n95\t-64.9\n94.8\t-65.2\n94.6\t-65.5\n94.4\t-65.8\n94.2\t-66.1\n94\t-66.4\n93.8\t-65.8\n93.6\t-65.2\n93.4\t-64.6\n93.2\t-64\n93\t-63.4\n92.8\t-62.8\n92.6\t-62.2\n92.4\t-61.6\n92.2\t-61\n92\t-60.4\n91.8\t-59.8\n91.6\t-59.2\n91.4\t-58.6\n91.2\t-58\n91\t-57.4\n90.8\t-56.8\n90.6\t-56.2\n90.4\t-55.6\n90.2\t-55\n90\t-54.4\n89.8\t-53.8\n89.6\t-53.2\n89.4\t-52.6\n89.2\t-52\n89\t-51.4\n88.8\t-50.8\n88.6\t-50.2\n88.4\t-49.6\n88.2\t-49\n88\t-48.4\n87.8\t-47.8\n87.6\t-47.2\n87.4\t-46.6\n87.2\t-46\n87\t-45.4\n86.8\t-44.8\n86.6\t-44.2\n86.4\t-43.6\n86.2\t-43\n86\t-42.4\n85.8\t-41.8\n85.6\t-41.2\n85.4\t-40.6\n85.2\t-40\n85\t-39.4\n84.8\t-38.8\n84.6\t-38.2\n84.4\t-37.6\n84.2\t-37\n84\t-36.4\n83.8\t-35.8\n83.6\t-35.2\n83.4\t-34.6\n83.2\t-34\n83\t-33.4\n82.8\t-32.8\n82.6\t-32.2\n82.4\t-31.6\n82.2\t-31\n82\t-30.4\n81.8\t-29.8\n81.6\t-29.2\n81.4\t-28.6\n81.2\t-28\n81\t-27.4\n80.8\t-26.8\n80.6\t-26.2\n80.4\t-25.6\n80.2\t-25\n80\t-24.4\n79.8\t-23.8\n79.6\t-23.2\n79.4\t-22.6\n79.2\t-22\n79\t-21.4\n78.8\t-20.8\n78.6\t-20.2\n78.4\t-19.6\n78.2\t-19\n78\t-18.4\n77.8\t-17.8\n77.6\t-17.2\n77.4\t-16.6\n77.2\t-16\n77\t-15.4\n76.8\t-14.8\n76.6\t-14.2\n76.4\t-13.6\n76.2\t-13\n76\t-12.4\n75.8\t-11.8\n75.6\t-11.2\n75.4\t-10.6\n75.2\t-10\n75\t-9.4\n74.8\t-8.8\n74.6\t-8.2\n74.4\t-7.6\n74.2\t-7\n74\t-6.4\n73.8\t-5.8\n73.6\t-5.2\n73.4\t-4.6\n73.2\t-4\n73\t-3.4\n72.8\t-2.8\n72.6\t-2.2\n72.4\t-1.6\n72.2\t-1\n72\t-0.4\n71.8\t0.2\n71.6\t0.8\n71.4\t1.4\n71.2\t2\n71\t2.6\n70.8\t3.2\n70.6\t3.8\n70.4\t4.4\n70.2\t5\n70\t5.6\n69.8\t6.2\n69.6\t6.8\n69.4\t7.4\n69.2\t8\n69\t8.6\n68.8\t9.2\n68.6\t9.8\n68.4\t10.4\n68.2\t11\n68\t11.6\n67.8\t12.2\n67.6\t12.8\n67.4\t13.4\n67.2\t14\n67\t14.6\n66.8\t15.2\n66.6\t15.8\n66.4\t16.4\n66.2\t17\n66\t17.6\n65.8\t18.2\n65.6\t18.8\n65.4\t19.4\n65.2\t20\n65\t20.6\n64.8\t21.2\n64.6\t21.8\n64.4\t22.4\n64.2\t23\n64\t23.6\n63.8\t24.2\n63.6\t24.8\n63.4\t25.4\n63.2\t26\n63\t26.6\n62.8\t27.2\n62.6\t27.8\n62.4\t28.4\n62.2\t29\n62\t29.6\n61.8\t30.2\n61.6\t30.8\n61.4\t31.4\n61.2\t32\n61\t32.6\n60.8\t33.2\n60.6\t33.8\n60.4\t34.4\n60.2\t35\n60\t35.6\n59.8\t36.2\n59.6\t36.8\n59.4\t37.4\n59.2\t38\n59\t38.6\n58.8\t39.2\n58.6\t39.8\n58.4\t40.4\n58.2\t40.1\n58\t39.8\n57.8\t39.5\n57.6\t39.2\n57.4\t38.9\n57.2\t38.6\n57\t38.3\n56.8\t38\n56.6\t37.7\n56.4\t37.4\n56.2\t37.1\n56\t36.8\n55.8\t36.5\n55.6\t36.2\n55.4\t35.9\n55.2\t35.6\n55\t35.3\n54.8\t35\n54.6\t34.7\n54.4\t34.4\n54.2\t34.1\n54\t33.8\n53.8\t33.5\n53.6\t33.2\n53.4\t32.9\n53.2\t32.6\n53\t32.3\n52.8\t32\n52.6\t31.7\n52.4\t31.4\n52.2\t31.1\n52\t30.8\n51.8\t30.5\n51.6\t30.2\n51.4\t29.9\n51.2\t29.6\n51\t29.3\n50.8\t29\n50.6\t28.7\n50.4\t28.4\n50.2\t28.1\n50\t27.8\n49.8\t27.5\n49.6\t27.2\n49.4\t26.9\n49.2\t26.6\n49\t26.3\n48.8\t26\n48.6\t25.7\n48.4\t25.4\n48.2\t25.1\n48\t24.8\n47.8\t24.5\n47.6\t24.2\n47.4\t23.9\n47.2\t23.6\n47\t23.3\n46.8\t23\n46.6\t22.7\n46.4\t22.4\n46.2\t22.1\n46\t21.8\n45.8\t21.5\n45.6\t21.2\n45.4\t20.9\n45.2\t20.6\n45\t20.3\n44.8\t20\n44.6\t19.7\n44.4\t19.4\n44.2\t19.1\n44\t18.8\n43.8\t18.5\n43.6\t18.2\n43.4\t17.9\n43.2\t17.6\n43\t17.3\n42.8\t17\n42.6\t16.7\n42.4\t16.4\n42.2\t16.1\n42\t15.8\n41.8\t15.5\n41.6\t15.2\n41.4\t14.9\n41.2\t14.6\n41\t14.3\n40.8\t14\n40.6\t13.7\n40.4\t13.4\n40.2\t13.1\n40\t12.8\n39.8\t12.5\n39.6\t12.2\n39.4\t11.9\n39.2\t11.6\n39\t11.3\n38.8\t11\n38.6\t10.7\n38.4\t10.4\n38.2\t10.1\n38\t9.8\n37.8\t9.5\n37.6\t9.2\n37.4\t8.9\n37.2\t8.6\n37\t8.3\n36.8\t8\n36.6\t7.7\n36.4\t7.4\n36.2\t7.1\n36\t6.8\n35.8\t6.5\n35.6\t6.2\n35.4\t5.9\n35.2\t5.6\n35\t5.3\n34.8\t5\n34.6\t4.7\n34.4\t4.4\n34.2\t4.1\n34\t3.8\n33.8\t3.5\n33.6\t3.2\n33.4\t2.9\n33.2\t2.6\n33\t2.3\n32.8\t2\n32.6\t1.7\n32.4\t1.4\n32.2\t1.1\n32\t0.8\n31.8\t0.5\n31.6\t0.2\n31.4\t-0.1\n31.2\t-0.4\n31\t-0.7\n30.8\t-1\n30.6\t-1.3\n30.4\t-1.6\n30.2\t-1.9\n30\t-2.2\n29.8\t-2.5\n29.6\t-2.8\n29.4\t-3.1\n29.2\t-3.4\n29\t-3.7\n28.8\t-4\n28.6\t-4.3\n28.4\t-4.6\n28.2\t-4.9\n28\t-5.2\n27.8\t-5.5\n27.6\t-5.8\n27.4\t-6.1\n27.2\t-6.4\n27\t-6.7\n26.8\t-7\n26.6\t-7.3\n26.4\t-7.6\n26.2\t-7.9\n26\t-8.2\n25.8\t-8.5\n25.6\t-8.8\n25.4\t-9.1\n25.2\t-9.4\n25\t-9.7\n24.8\t-10\n24.6\t-10.3\n24.4\t-10.6\n24.2\t-10.9\n24\t-11.2\n23.8\t-11.5\n23.6\t-11.8\n23.4\t-12.1\n23.2\t-12.4\n23\t-12.7\n22.8\t-13\n22.6\t-13.3\n22.4\t-13.6\n22.2\t-13.9\n22\t-14.2\n21.8\t-14.5\n21.6\t-14.8\n21.4\t-15.1\n21.2\t-15.4\n21\t-15.7\n20.8\t-16\n20.6\t-16.3\n20.4\t-16.6\n20.2\t-16.9\n20\t-17.2\n19.8\t-17.5\n19.6\t-17.8\n19.4\t-18.1\n19.2\t-18.4\n19\t-18.7\n18.8\t-19\n18.6\t-19.3\n18.4\t-19.6\n18.2\t-19.9\n18\t-20.2\n17.8\t-20.5\n17.6\t-20.8\n17.4\t-21.1\n17.2\t-21.4\n17\t-21.7\n16.8\t-22\n16.6\t-22.3\n16.4\t-22.6\n16.2\t-22.9\n16\t-23.2\n15.8\t-23.5\n15.6\t-23.8\n15.4\t-24.1\n15.2\t-24.4\n15\t-24.7\n14.8\t-25\n14.6\t-25.3\n14.4\t-25.6\n14.2\t-25.9\n14\t-26.2\n13.8\t-26.5\n13.6\t-26.8\n13.4\t-27.1\n13.2\t-27.4\n13\t-27.7\n12.8\t-28\n12.6\t-28.3\n12.4\t-28.6\n12.2\t-28.9\n12\t-29.2\n11.8\t-29.5\n11.6\t-29.8\n11.4\t-30.1\n11.2\t-30.4\n11\t-30.7\n10.8\t-31\n10.6\t-31.3\n10.4\t-31.6\n10.2\t-31.9\n10\t-32.2\n9.8\t-32.5\n9.6\t-32.8\n9.4\t-33.1\n9.2\t-33.4\n9\t-33.7\n8.8\t-34\n8.6\t-34.3\n8.4\t-34.6\n8.2\t-34.9\n8\t-35.2\n7.8\t-35.5\n7.6\t-35.8\n7.4\t-36.1\n7.2\t-36.4\n7\t-36.7\n6.8\t-37\n6.6\t-37.3\n6.4\t-37.6\n6.2\t-37.9\n6\t-38.2\n5.8\t-38.5\n5.6\t-38.8\n5.4\t-39.1\n5.2\t-39.4\n5\t-39.7\n4.8\t-40\n4.6\t-40.3\n4.4\t-40.6\n4.2\t-40.9\n4\t-41.2\n3.8\t-41.5\n3.6\t-41.8\n3.4\t-42.1\n3.2\t-42.4\n3\t-42.7\n2.8\t-43\n2.6\t-43.3\n2.4\t-43.6\n2.2\t-43.9\n2\t-44.2\n1.8\t-44.5\n1.6\t-44.8\n1.4\t-45.1\n1.2\t-45.4\n1\t-45.7\n0.8\t-46\n0.6\t-46.3\n0.4\t-46.6\n0.2\t-46.9\n-2.60275E-12\t-47.2\n-0.2\t-47.5\n-0.4\t-47.8\n-1\t-48.1\n-1.6\t-48.4\n-2.2\t-48.7\n-2.8\t-49\n-3.4\t-49.3\n-4\t-49.6\n-4.6\t-49.9\n-5.2\t-50.2\n-5.8\t-50.5\n-6.4\t-50.8\n-7\t-51.1\n-7.6\t-51.4\n-8.2\t-51.7\n-8.8\t-52\n-9.4\t-52.3\n-10\t-52.6\n-10.6\t-52.9\n-11.2\t-53.2\n-11.8\t-53.5\n-12.4\t-53.8\n-13\t-54.1\n-13.6\t-54.4\n-14.2\t-54.7\n-14.8\t-55\n-15.4\t-55.3\n-16\t-55.6\n-16.6\t-55.9\n-17.2\t-56.2\n-17.8\t-56.5\n-18.4\t-56.8\n-19\t-57.1\n-19.6\t-57.4\n-20.2\t-57.7\n-20.8\t-58\n-21.4\t-58.3\n-22\t-58.6\n-22.6\t-58.9\n-23.2\t-59.2\n-23.8\t-59.5\n-24.4\t-59.8\n-25\t-60.1\n-25.6\t-60.4\n-26.2\t-60.7\n-26.8\t-61\n-27.4\t-61.3\n-28\t-61.6\n-28.6\t-61.9\n-29.2\t-62.2\n-29.8\t-62.5\n-30.4\t-62.8\n-31\t-63.1\n-31.6\t-63.4\n-32.2\t-63.7\n-32.8\t-64\n-33.4\t-64.3\n-34\t-64.6\n-34.6\t-64.9\n-35.2\t-65.2\n-35.8\t-65.5\n-36.4\t-65.8\n-37\t-66.1\n-37.6\t-66.4\n-38.2\t-66.7\n-38.8\t-67\n-39.4\t-67.3\n-40\t-67.6\n-40.6\t-67.9\n-41.2\t-68.2\n-41.8\t-68.5\n-42.4\t-68.8\n-43\t-69.1\n-43.6\t-69.4\n-44.2\t-69.7\n-44.8\t-70\n-45.4\t-70.3\n-46\t-70.6\n-46.6\t-70.9\n-47.2\t-71.2\n-47.8\t-71.5\n-48.4\t-71.8\n-49\t-72.1\n-49.6\t-72.4\n-50.2\t-72.7\n-50.8\t-73\n-51.4\t-73.3\n-52\t-73.6\n-52.6\t-73.9\n-53.2\t-74.2\n-53.8\t-74.5\n-54.4\t-74.8\n-55\t-75.1\n-55.6\t-75.4\n-56.2\t-75.7\n-56.8\t-76\n-57.4\t-76.3\n-58\t-76.6\n-58.6\t-76.9\n-59.2\t-77.2\n-59.8\t-77.5\n-60.4\t-77.8\n-61\t-78.1\n-61.6\t-78.4\n-62.2\t-78.7\n-62.8\t-79\n-63.4\t-79.3\n-64\t-79.6\n-64.6\t-79.9\n-65.2\t-80.2\n-65.8\t-80.5\n-66.4\t-80.8\n-67\t-81.1\n-67.6\t-81.4\n-68.2\t-81.7\n-68.8\t-82\n-69.4\t-82.3\n-70\t-82.6\n-70.6\t-82.9\n-71.2\t-83.2\n-71.8\t-83.5\n-72.4\t-83.8\n-73\t-84.1\n-73.6\t-84.4\n-74.2\t-84.7\n-74.8\t-85\n-75.4\t-85.3\n-76\t-85.6\n-76.6\t-85.9\n-77.2\t-86.2\n-77.8\t-86.5\n-78.4\t-86.8\n-79\t-87.1\n-79.6\t-87.4\n-80.2\t-87.7\n-80.8\t-88\n-81.4\t-88.3\n-82\t-88.6\n-82.6\t-88.9\n-83.2\t-89.2\n-83.8\t-89.5\n-84.4\t-89.8\n-85\t-90.1\n-85.6\t-90.4\n-86.2\t-90.3\n-86.8\t-90.2\n-87.4\t-90.1\n-88\t-90\n-88.6\t-89.9\n-89.2\t-89.8\n-89.8\t-89.7\n-90.4\t-89.6\n-90.2\t-89.5\n-90\t-89.4\n-89.8\t-89.3\n-89.6\t-89.2\n-89.4\t-89.1\n-89.2\t-89\n-89\t-88.9\n-88.8\t-88.8\n-88.6\t-88.7\n-88.4\t-88.6\n-88.2\t-88.5\n-88\t-88.4\n-87.8\t-88.3\n-87.6\t-88.2\n-87.4\t-88.1\n-87.2\t-88\n-87\t-87.9\n-86.8\t-87.8\n-86.6\t-87.7\n-86.4\t-87.6\n-86.2\t-87.5\n-86\t-87.4\n-85.8\t-87.3\n-85.6\t-87.2\n-85.4\t-87.1\n-85.2\t-87\n-85\t-86.9\n-84.8\t-86.8\n-84.6\t-86.7\n-84.4\t-86.6\n-84.2\t-86.5\n-84\t-86.4\n-83.8\t-86.3\n-83.6\t-86.2\n-83.4\t-86.1\n-83.2\t-86\n-83\t-85.9\n-82.8\t-85.8\n-82.6\t-85.7\n-82.4\t-85.6\n-82.2\t-85.5\n-82\t-85.4\n-81.8\t-85.3\n-81.6\t-85.2\n-81.4\t-85.1\n-81.2\t-85\n-81\t-84.9\n-80.8\t-84.8\n-80.6\t-84.7\n-80.4\t-84.6\n-80.2\t-84.5\n-80\t-84.4\n-79.8\t-84.3\n-79.6\t-84.2\n-79.4\t-84.1\n-79.2\t-84\n-79\t-83.9\n-78.8\t-83.8\n-78.6\t-83.7\n-78.4\t-83.6\n-78.2\t-83.5\n-78\t-83.4\n-77.8\t-83.3\n-77.6\t-83.2\n-77.4\t-83.1\n-77.2\t-83\n-77\t-82.9\n-76.8\t-82.8\n-76.6\t-82.7\n-76.4\t-82.6\n-76.2\t-82.5\n-76\t-82.4\n-75.8\t-82.3\n-75.6\t-82.2\n-75.4\t-82.1\n-75.2\t-82\n-75\t-81.9\n-74.8\t-81.8\n-74.6\t-81.7\n-74.4\t-81.6\n-74.2\t-81.5\n-74\t-81.4\n-73.8\t-81.3\n-73.6\t-81.2\n-73.4\t-81.1\n-73.2\t-81\n-73\t-80.9\n-72.8\t-80.8\n-72.6\t-80.7\n-72.4\t-80.6\n-72.2\t-80.5\n-72\t-80.4\n-71.8\t-80.3\n-71.6\t-80.2\n-71.4\t-80.1\n-71.2\t-80\n-71\t-79.9\n-70.8\t-79.8\n-70.6\t-79.7\n-70.4\t-79.6\n-70.2\t-79.5\n-70\t-79.4\n-69.8\t-79.3\n-69.6\t-79.2\n-69.4\t-79.1\n-69.2\t-79\n-69\t-78.9\n-68.8\t-78.8\n-68.6\t-78.7\n-68.4\t-78.6\n-68.2\t-78.5\n-68\t-78.4\n-67.8\t-78.3\n-67.6\t-78.2\n-67.4\t-78.1\n-67.2\t-78\n-67\t-77.9\n-66.8\t-77.8\n-66.6\t-77.7\n-66.4\t-77.6\n-66.2\t-77.5\n-66\t-77.4\n-65.8\t-77.3\n-65.6\t-77.2\n-65.4\t-77.1\n-65.2\t-77\n-65\t-76.9\n-64.8\t-76.8\n-64.6\t-76.7\n-64.4\t-76.6\n-64.2\t-76.5\n-64\t-76.4\n-63.8\t-76.3\n-63.6\t-76.2\n-63.4\t-76.1\n-63.2\t-76\n-63\t-75.9\n-62.8\t-75.8\n-62.6\t-75.7\n-62.4\t-75.6\n-62.2\t-75.5\n-62\t-75.4\n-61.8\t-75.3\n-61.6\t-75.2\n-61.4\t-75.1\n-61.2\t-75\n-61\t-74.9\n-60.8\t-74.8\n-60.6\t-74.7\n-60.4\t-74.6\n-60.2\t-74.5\n-60\t-74.4\n-59.8\t-74.3\n-59.6\t-74.2\n-59.4\t-74.1\n-59.2\t-74\n-59\t-73.9\n-58.8\t-73.8\n-58.6\t-73.7\n-58.4\t-73.6\n-58.2\t-73.5\n-58\t-73.4\n-57.8\t-73.3\n-57.6\t-73.2\n-57.4\t-73.1\n-57.2\t-73\n-57\t-72.9\n-56.8\t-72.8\n-56.6\t-72.7\n-56.4\t-72.6\n-56.2\t-72.5\n-56\t-72.4\n-55.8\t-72.3\n-55.6\t-72.2\n-55.4\t-72.1\n-55.2\t-72\n-55\t-71.9\n-54.8\t-71.8\n-54.6\t-71.7\n-54.4\t-71.6\n-54.2\t-71.5\n-54\t-71.4\n-53.8\t-71.3\n-53.6\t-71.2\n-53.4\t-71.1\n-53.2\t-71\n-53\t-70.9\n-52.8\t-70.8\n-52.6\t-70.7\n-52.4\t-70.6\n-52.2\t-70.5\n-52\t-70.4\n-51.8\t-70.3\n-51.6\t-70.2\n-51.4\t-70.1\n-51.2\t-70\n-51\t-69.9\n-50.8\t-69.8\n-50.6\t-69.7\n-50.4\t-69.6\n-50.2\t-69.5\n-50\t-69.4\n-49.8\t-69.3\n-49.6\t-69.2\n-49.4\t-69.1\n-49.2\t-69\n-49\t-68.9\n-48.8\t-68.8\n-48.6\t-68.7\n-48.4\t-68.6\n-48.2\t-68.5\n-48\t-68.4\n-47.8\t-68.3\n-47.6\t-68.2\n-47.4\t-68.1\n-47.2\t-68\n-47\t-67.9\n-46.8\t-67.8\n-46.6\t-67.7\n-46.4\t-67.6\n-46.2\t-67.5\n-46\t-67.4\n-45.8\t-67.3\n-45.6\t-67.2\n-45.4\t-67.1\n-45.2\t-67\n-45\t-66.9\n-44.8\t-66.8\n-44.6\t-66.7\n-44.4\t-66.6\n-44.2\t-66.5\n-44\t-66.4\n-43.8\t-66.3\n-43.6\t-66.2\n-43.4\t-66.1\n-43.2\t-66\n-43\t-65.9\n-42.8\t-65.8\n-42.6\t-65.7\n-42.4\t-65.6\n-42.2\t-65.5\n-42\t-65.4\n-41.8\t-65.1\n-41.6\t-64.8\n-41.4\t-64.5\n-41.2\t-64.2\n-41\t-63.9\n-40.8\t-63.6\n-40.6\t-63.3\n-40.4\t-63\n-40.2\t-62.7\n-40\t-62.4\n-39.8\t-62.1\n-39.6\t-61.8\n-39.4\t-61.5\n-39.2\t-61.2\n-39\t-60.9\n-38.8\t-60.6\n-38.6\t-60.3\n-38.4\t-60\n-38.2\t-59.7\n-38\t-59.4\n-37.8\t-59.1\n-37.6\t-58.8\n-37.4\t-58.5\n-37.2\t-58.2\n-37\t-57.9\n-36.8\t-57.6\n-36.6\t-57.3\n-36.4\t-57\n-36.2\t-56.7\n-36\t-56.4\n-35.8\t-56.1\n-35.6\t-55.8\n-35.4\t-55.5\n-35.2\t-55.2\n-35\t-54.9\n-34.8\t-54.6\n-34.6\t-54.3\n-34.4\t-54\n-34.2\t-53.7\n-34\t-53.4\n-33.8\t-53.1\n-33.6\t-52.8\n-33.4\t-52.5\n-33.2\t-52.2\n-33\t-51.9\n-32.8\t-51.6\n-32.6\t-51.3\n-32.4\t-51\n-32.2\t-50.7\n-32\t-50.4\n-31.8\t-50.1\n-31.6\t-49.8\n-31.4\t-49.5\n-31.2\t-49.2\n-31\t-48.9\n-30.8\t-48.6\n-30.6\t-48.3\n-30.4\t-48\n-30.2\t-47.7\n-30\t-47.4\n-29.8\t-47.1\n-29.6\t-46.8\n-29.4\t-46.5\n-29.2\t-46.2\n-29\t-45.9\n-28.8\t-45.6\n-28.6\t-45.3\n-28.4\t-45\n-28.2\t-44.7\n-28\t-44.4\n-27.8\t-44.1\n-27.6\t-43.8\n-27.4\t-43.5\n-27.2\t-43.2\n-27\t-42.9\n-26.8\t-42.6\n-26.6\t-42.3\n-26.4\t-42\n-26.2\t-41.7\n-26\t-41.4\n-25.8\t-41.1\n-25.6\t-40.8\n-25.4\t-40.5\n-25.2\t-40.2\n-25\t-39.9\n-24.8\t-39.6\n-24.6\t-39.3\n-24.4\t-39\n-24.2\t-38.7\n-24\t-38.4\n-23.8\t-38.1\n-23.6\t-37.8\n-23.4\t-37.5\n-23.2\t-37.2\n-23\t-36.9\n-22.8\t-36.6\n-22.6\t-36.3\n-22.4\t-36\n-22.2\t-35.7\n-22\t-35.4\n-21.8\t-35.1\n-21.6\t-34.8\n-21.4\t-34.5\n-21.2\t-34.2\n-21\t-33.9\n-20.8\t-33.6\n-20.6\t-33.3\n-20.4\t-33\n-20.2\t-32.7\n-20\t-32.4\n-19.8\t-32.1\n-19.6\t-31.8\n-19.4\t-31.5\n-19.2\t-31.2\n-19\t-30.9\n-18.8\t-30.6\n-18.6\t-30.3\n-18.4\t-30\n-18.2\t-29.7\n-18\t-29.4\n-17.8\t-29.1\n-17.6\t-28.8\n-17.4\t-28.5\n-17.2\t-28.2\n-17\t-27.9\n-16.8\t-27.6\n-16.6\t-27.3\n-16.4\t-27\n-16.2\t-26.7\n-16\t-26.4\n-15.8\t-26.1\n-15.6\t-25.8\n-15.4\t-25.5\n-15.2\t-25.2\n-15\t-24.9\n-14.8\t-24.6\n-14.6\t-24.3\n-14.4\t-24\n-14.2\t-23.7\n-14\t-23.4\n-13.8\t-23.1\n-13.6\t-22.8\n-13.4\t-22.5\n-13.2\t-22.2\n-13\t-21.9\n-12.8\t-21.6\n-12.6\t-21.3\n-12.4\t-21\n-12.2\t-20.7\n-12\t-20.4\n-11.8\t-20.1\n-11.6\t-19.8\n-11.4\t-19.5\n-11.2\t-19.2\n-11\t-18.9\n-10.8\t-18.6\n-10.6\t-18.3\n-10.4\t-18\n-10.2\t-17.7\n-10\t-17.4\n-9.8\t-17.1\n-9.6\t-16.8\n-9.4\t-16.5\n-9.2\t-16.2\n-9\t-15.9\n-8.8\t-15.6\n-8.6\t-15.3\n-8.4\t-15\n-8.2\t-14.7\n-8\t-14.4\n-7.8\t-14.1\n-7.6\t-13.8\n-7.4\t-13.5\n-7.2\t-13.2\n-7\t-12.9\n-6.8\t-12.6\n-6.6\t-12.3\n-6.4\t-12\n-6.2\t-11.7\n-6\t-11.4\n-5.8\t-11.1\n-5.6\t-10.8\n-5.4\t-10.5\n-5.2\t-10.2\n-5\t-9.9\n-4.8\t-9.6\n-4.6\t-9.3\n-4.4\t-9\n-4.2\t-8.7\n-4\t-8.4\n-3.8\t-8.1\n-3.6\t-7.8\n-3.4\t-7.5\n-3.2\t-7.2\n-3\t-6.9\n-2.8\t-6.6\n-2.6\t-6.3\n-2.4\t-6\n-2.2\t-5.7\n-2\t-5.4\n-1.8\t-5.1\n-1.6\t-4.8\n-1.4\t-4.5\n-1.2\t-4.2\n-1\t-3.9\n-0.8\t-3.6\n-0.6\t-3.3\n-0.4\t-3\n-0.2\t-2.7\n-1.70025E-12\t-2.4\n0.2\t-2.1\n0.4\t-1.8\n0.6\t-1.5\n0.8\t-1.2\n1\t-0.9\n1.2\t-0.6\n1.4\t-0.3\n1.6\t-1.83087E-12\n1.8\t0.3\n2\t0.6\n2.2\t0.9\n2.4\t1.2\n2.6\t1.5\n2.8\t1.8\n3\t2.1\n3.2\t2.4\n3.4\t2.7\n3.6\t3\n3.8\t3.3\n4\t3.6\n4.2\t3.9\n4.4\t4.2\n4.6\t4.5\n4.8\t4.8\n5\t5.1\n5.2\t5.4\n5.4\t5.7\n5.6\t6\n5.8\t6.3\n6\t6.6\n6.2\t6.9\n6.4\t7.2\n6.6\t7.5\n6.8\t7.8\n7\t8.1\n7.2\t8.4\n7.4\t8.7\n7.6\t9\n7.8\t9.3\n8\t9.6\n8.2\t9.9\n8.4\t10.2\n8.6\t10.5\n8.8\t10.8\n9\t11.1\n9.2\t11.4\n9.4\t11.7\n9.6\t12\n9.8\t12.3\n10\t12.6\n10.2\t12.9\n10.4\t13.2\n10.6\t13.5\n10.8\t13.8\n11\t14.1\n11.2\t14.4\n11.4\t14.7\n11.6\t15\n11.8\t15.3\n12\t15.6\n12.2\t15.9\n12.4\t16.2\n12.6\t16.5\n12.8\t16.8\n13\t17.1\n13.2\t17.4\n13.4\t17.7\n13.6\t18\n13.8\t18.3\n14\t18.6\n14.2\t18.9\n14.4\t19.2\n14.6\t19.5\n14.8\t19.8\n15\t20.1\n15.2\t20.4\n15.4\t20.7\n15.6\t21\n15.8\t21.3\n16\t21.6\n16.2\t21.9\n16.4\t22.2\n16.6\t22.5\n16.8\t22.8\n17\t23.1\n17.2\t23.4\n17.4\t23.7\n17.6\t24\n17.8\t24.3\n18\t24.6\n18.2\t24.9\n18.4\t25.2\n18.6\t25.5\n18.8\t25.8\n19\t26.1\n19.2\t26.4\n19.4\t26.7\n19.6\t27\n19.8\t27.3\n20\t27.6\n20.2\t27.9\n20.4\t28.2\n20.6\t28.5\n20.8\t28.8\n21\t29.1\n21.2\t29.4\n21.4\t29.7\n21.6\t30\n21.8\t30.3\n22\t30.6\n22.2\t30.9\n22.4\t31.2\n22.6\t31.5\n22.8\t31.8\n23\t32.1\n23.2\t32.4\n23.4\t32.7\n23.6\t33\n23.8\t33.3\n24\t33.6\n24.2\t33.9\n24.4\t34.2\n24.6\t34.5\n24.8\t34.8\n25\t35.1\n25.2\t35.4\n25.4\t35.7\n25.6\t36\n25.8\t36.3\n26\t36.6\n26.2\t36.9\n26.4\t37.2\n26.6\t37.5\n26.8\t37.8\n27\t38.1\n27.2\t38.4\n27.4\t38.7\n27.6\t39\n27.8\t39.3\n28\t39.6\n28.2\t39.9\n28.4\t40.2\n28.6\t40.5\n28.8\t40.8\n29\t41.1\n29.2\t41.4\n29.4\t41.7\n29.6\t42\n29.8\t42.3\n30\t42.6\n30.2\t42.9\n30.4\t43.2\n30.6\t43.5\n30.8\t43.8\n31\t44.1\n31.2\t44.4\n31.4\t44.7\n31.6\t45\n31.8\t45.3\n32\t45.6\n32.2\t45.9\n32.4\t46.2\n32.6\t46.5\n32.8\t46.8\n33\t47.1\n33.2\t47.4\n33.4\t47.7\n33.6\t48\n33.8\t48.3\n34\t48.6\n34.2\t48.9\n34.4\t49.2\n34.6\t49.5\n34.8\t49.8\n35\t50.1\n35.2\t50.4\n35.4\t50.7\n35.6\t51\n35.8\t51.3\n36\t51.6\n36.2\t51.9\n36.4\t52.2\n36.6\t52.5\n36.8\t52.8\n37\t53.1\n37.2\t53.4\n37.4\t53.7\n37.6\t54\n37.8\t54.3\n38\t54.6\n38.2\t54.9\n38.4\t55.2\n38.6\t55.5\n38.8\t55.8\n39\t56.1\n39.2\t56.4\n39.4\t56.7\n39.6\t57\n39.8\t57.3\n40\t57.6\n40.2\t57.9\n40.4\t58.2\n40.6\t58.5\n40.8\t58.8\n41\t59.1\n41.2\t59.4\n41.4\t59.7\n41.6\t60\n41.8\t60.3\n42\t60.6\n42.2\t60.9\n42.4\t61.2\n42.6\t61.5\n42.8\t61.8\n43\t62.1\n43.2\t62.4\n43.4\t62.7\n43.6\t63\n43.8\t63.3\n44\t63.6\n44.2\t63.9\n44.4\t64.2\n44.6\t64.5\n44.8\t64.8\n45\t65.1\n45.2\t65.4\n45.4\t65.7\n45.6\t66\n45.8\t66.3\n46\t66.6\n46.2\t66.9\n46.4\t67.2\n46.6\t67.5\n46.8\t67.8\n47\t68.1\n47.2\t68.4\n47.4\t68.7\n47.6\t69\n47.8\t69.3\n48\t69.6\n48.2\t69.9\n48.4\t70.2\n48.6\t70.5\n48.8\t70.8\n49\t71.1\n49.2\t71.4\n49.4\t71.7\n49.6\t72\n49.8\t72.3\n50\t72.6\n50.2\t72.9\n50.4\t73.2\n50.6\t73.5\n50.8\t73.8\n51\t74.1\n51.2\t74.4\n51.4\t74.7\n51.6\t75\n51.8\t75.3\n52\t75.6\n52.2\t75.9\n52.4\t76.2\n52.6\t76.5\n52.8\t76.8\n53\t77.1\n53.2\t77.4\n53.4\t77.7\n53.6\t78\n53.8\t78.3\n54\t78.6\n54.2\t78.9\n54.4\t79.2\n54.6\t79.5\n54.8\t79.8\n55\t80.1\n55.2\t80.4\n55.4\t80.7\n55.6\t81\n55.8\t81.3\n56\t81.6\n56.2\t81.9\n56.4\t82.2\n56.6\t82.5\n56.8\t82.8\n57\t83.1\n57.2\t83.4\n57.4\t83.7\n57.6\t84\n57.8\t84.3\n58\t84.6\n58.2\t84.9\n58.4\t85.2\n58.6\t85.5\n58.8\t85.8\n59\t86.1\n59.2\t86.4\n59.4\t86.7\n59.6\t87\n59.8\t87.3\n60\t87.6\n60.2\t87.9\n60.4\t88.2\n60.6\t88.5\n60.8\t88.8\n61\t89.1\n61.2\t89.4\n61.4\t89.7\n61.6\t90\n61.8\t90.3\n62\t90.6\n62.2\t90.9\n62.4\t91.2\n62.6\t91.5\n62.8\t91.8\n63\t92.1\n63.2\t92.4\n63.4\t92.7\n63.6\t93\n63.8\t93.3\n64\t93.6\n64.2\t93.9\n64.4\t93.2\n64.6\t92.5\n64.8\t91.8\n65\t91.1\n65.2\t90.4\n65.4\t89.7\n65.6\t89\n65.8\t88.3\n66\t87.6\n66.2\t86.9\n66.4\t86.2\n66.6\t85.5\n66.8\t84.8\n67\t84.1\n66.6\t83.4\n66.2\t82.7\n65.8\t82\n65.4\t81.3\n65\t80.6\n64.6\t79.9\n64.2\t79.2\n63.8\t78.5\n63.4\t77.8\n63\t77.1\n62.6\t76.4\n62.2\t75.7\n61.8\t75\n61.4\t74.3\n61\t73.6\n60.6\t72.9\n60.2\t72.2\n59.8\t71.5\n59.4\t70.8\n59\t70.1\n58.6\t69.4\n58.2\t68.7\n57.8\t68\n57.4\t67.3\n57\t66.6\n56.6\t65.9\n56.2\t65.2\n55.8\t64.5\n55.4\t63.8\n55\t63.1\n54.6\t62.4\n54.2\t61.7\n53.8\t61\n53.4\t60.3\n53\t59.6\n52.6\t58.9\n52.2\t58.2\n51.8\t57.5\n51.4\t56.8\n51\t56.1\n50.6\t55.4\n50.2\t54.7\n49.8\t54\n49.4\t53.3\n49\t52.6\n48.6\t51.9\n48.2\t51.2\n47.8\t50.5\n47.4\t49.8\n47\t49.1\n46.6\t48.4\n46.2\t47.7\n45.8\t47\n45.4\t46.3\n45\t45.6\n44.6\t44.9\n44.2\t44.2\n43.8\t43.5\n43.4\t42.8\n43\t42.1\n42.6\t41.4\n42.2\t40.7\n41.8\t40\n41.4\t39.3\n41\t38.6\n40.6\t37.9\n40.2\t37.2\n39.8\t36.5\n39.4\t35.8\n39\t35.1\n38.6\t34.4\n38.2\t33.7\n37.8\t33\n37.4\t32.3\n37\t31.6\n36.6\t30.9\n36.2\t30.2\n35.8\t29.5\n35.4\t28.8\n35\t28.1\n34.6\t27.4\n34.2\t26.7\n33.8\t26\n33.4\t25.3\n33\t24.6\n32.6\t23.9\n32.2\t23.2\n31.8\t22.5\n31.4\t21.8\n31\t21.1\n30.6\t20.4\n30.2\t19.7\n29.8\t19\n29.4\t18.3\n29\t17.6\n28.6\t16.9\n28.2\t16.2\n27.8\t15.5\n27.4\t14.8\n27\t14.1\n26.6\t13.4\n26.2\t12.7\n25.8\t12\n25.4\t11.3\n25\t10.6\n24.6\t9.9\n24.2\t9.2\n23.8\t8.5\n23.4\t7.8\n23\t7.1\n22.6\t6.4\n22.2\t5.7\n21.8\t5\n21.4\t4.3\n21\t3.6\n20.6\t2.9\n20.2\t2.2\n19.8\t1.5\n19.4\t0.8\n19\t0.1\n18.6\t-0.6\n18.2\t-1.3\n17.8\t-2\n17.4\t-2.7\n17\t-3.4\n16.6\t-4.1\n16.2\t-4.8\n15.8\t-5.5\n15.4\t-6.2\n15\t-6.9\n14.6\t-7.6\n14.2\t-8.3\n13.8\t-9\n13.4\t-9.7\n13\t-10.4\n12.6\t-11.1\n12.2\t-11.8\n11.8\t-12.5\n11.4\t-13.2\n11\t-13.9\n10.6\t-14.6\n10.2\t-15.3\n9.8\t-16\n9.4\t-16.7\n9\t-17.4\n8.6\t-18.1\n8.2\t-18.8\n7.8\t-19.5\n7.4\t-20.2\n7\t-20.9\n6.6\t-21.6\n6.2\t-22.3\n5.8\t-23\n5.4\t-23.7\n5\t-24.4\n4.6\t-25.1\n4.2\t-25.8\n3.8\t-26.5\n3.4\t-27.2\n3\t-27.9\n2.6\t-28.6\n2.2\t-29.3\n1.8\t-30\n1.4\t-30.7\n1\t-31.4\n0.6\t-32.1\n0.2\t-32.8\n-0.2\t-33.5\n-0.6\t-34.2\n-1\t-34.9\n-1.4\t-35.6\n-1.8\t-36.3\n-2.2\t-37\n-2.6\t-37.7\n-3\t-38.4\n-3.4\t-39.1\n-3.8\t-39.8\n-4.2\t-40.5\n-4.6\t-41.2\n-5\t-41.9\n-5.4\t-42.6\n-5.8\t-43.3\n-6.2\t-44\n-6.6\t-44.7\n-7\t-45.4\n-7.4\t-46.1\n-7.8\t-46.8\n-8.2\t-47.5\n-8.6\t-48.2\n-9\t-48.9\n-9.4\t-49.6\n-9.8\t-50.3\n-10.2\t-51\n-10.6\t-51.7\n-11\t-52.4\n-11.4\t-53.1\n-11.8\t-53.8\n-12.2\t-54.5\n-12.6\t-55.2\n-13\t-55.9\n-13.4\t-56.6\n-13.8\t-57.3\n-14.2\t-58\n-14.6\t-58.7\n-15\t-59.4\n-15.4\t-60.1\n-15.8\t-60.8\n-16.2\t-61.5\n-16.6\t-62.2\n-17\t-62.9\n-17.4\t-63.6\n-17.8\t-64.3\n-18.2\t-65\n-18.6\t-65.7\n-19\t-66.4\n-19.4\t-67.1\n-19.8\t-67.8\n-20.2\t-68.5\n-20.6\t-69.2\n-21\t-69.9\n-21.4\t-70.6\n-21.8\t-71.3\n-22.2\t-72\n-22.6\t-72.7\n-23\t-73.4\n-23.4\t-74.1\n-23.8\t-74.8\n-24.2\t-75.5\n-24.6\t-75\n-25\t-74.5\n-25.4\t-74\n-25.8\t-73.5\n-26.2\t-73\n-26.6\t-72.5\n-27\t-72\n-27.4\t-71.5\n-27.8\t-71\n-28.2\t-70.5\n-28.6\t-70\n-29\t-69.5\n-29.4\t-69\n-29.8\t-68.5\n-30.2\t-68\n-30.6\t-67.5\n-31\t-67\n-31.4\t-66.5\n-31.8\t-66\n-32.2\t-65.5\n-32.6\t-65\n-33\t-64.5\n-33.4\t-64\n-33.8\t-63.5\n-34.2\t-63\n-34.6\t-62.5\n-35\t-62\n-35.4\t-61.5\n-35.8\t-61\n-36.2\t-60.5\n-36.6\t-60\n-37\t-59.5\n-37.4\t-59\n-37.8\t-58.5\n-38.2\t-58\n-38.6\t-57.5\n-39\t-57\n-39.4\t-56.5\n-39.8\t-56\n-40.2\t-55.5\n-40.6\t-55\n-41\t-54.5\n-41.4\t-54\n-41.8\t-53.5\n-42.2\t-53\n-42.6\t-52.5\n-43\t-52\n-43.4\t-51.5\n-43.8\t-51\n-44.2\t-50.5\n-44.6\t-50\n-45\t-49.5\n-45.4\t-49\n-45.8\t-48.5\n-46.2\t-48\n-46.6\t-47.5\n-47\t-47\n-47.4\t-46.5\n-47.8\t-46\n-48.2\t-45.5\n-48.6\t-45\n-49\t-44.5\n-49.4\t-44\n-49.8\t-43.5\n-50.2\t-43\n-50.6\t-42.5\n-51\t-42\n-51.4\t-41.5\n-51.8\t-41\n-52.2\t-40.5\n-52.6\t-40\n-53\t-39.5\n-53.4\t-39\n-53.8\t-38.5\n-54.2\t-38\n-54.6\t-37.5\n-54\t-37\n-53.4\t-36.5\n-52.8\t-36\n-52.2\t-35.5\n-51.6\t-35\n-51\t-34.5\n-50.4\t-34\n-49.8\t-33.5\n-49.2\t-33\n-48.6\t-32.5\n-48\t-32\n-47.4\t-31.5\n-46.8\t-31\n-46.2\t-30.5\n-45.6\t-30\n-45\t-29.5\n-44.4\t-29\n-43.8\t-28.5\n-43.2\t-28\n-42.6\t-27.5\n-42\t-27\n-41.4\t-26.5\n-40.8\t-26\n-40.2\t-25.5\n-39.6\t-25\n-39\t-24.5\n-38.4\t-24\n-37.8\t-23.5\n-37.2\t-23\n-36.6\t-22.5\n-36\t-22\n-35.4\t-21.5\n-34.8\t-21\n-34.2\t-20.5\n-33.6\t-20\n-33\t-19.5\n-32.4\t-19\n-31.8\t-18.5\n-31.2\t-18\n-30.6\t-17.5\n-30\t-17\n-29.4\t-16.5\n-28.8\t-16\n-28.2\t-15.5\n-27.6\t-15\n-27\t-14.5\n-26.4\t-14\n-25.8\t-13.5\n-25.2\t-13\n-24.6\t-12.5\n-24\t-12\n-23.4\t-11.5\n-22.8\t-11\n-22.2\t-10.5\n-21.6\t-10\n-21\t-9.5\n-20.4\t-9\n-19.8\t-8.5\n-19.2\t-8\n-18.6\t-7.5\n-18\t-7\n-17.4\t-6.5\n-16.8\t-6\n-16.2\t-5.5\n-15.6\t-5\n-15\t-4.5\n-14.4\t-4\n-13.8\t-3.5\n-13.2\t-3\n-12.6\t-2.5\n-12\t-2\n-11.4\t-1.5\n-10.8\t-1\n-10.2\t-0.5\n-9.6\t-2.74269E-12\n-9\t0.5\n-8.4\t1\n-7.8\t1.5\n-7.2\t2\n-6.6\t2.5\n-6\t3\n-5.4\t3.5\n-4.8\t4\n-4.2\t4.5\n-3.6\t5\n-3\t5.5\n-2.4\t6\n-1.8\t6.5\n-1.2\t7\n-0.6\t7.5\n-9.61675E-13\t8\n0.6\t8.5\n1.2\t9\n1.8\t9.5\n2.4\t10\n3\t10.5\n3.6\t11\n4.2\t11.5\n4.8\t12\n5.4\t12.5\n6\t13\n6.6\t13.5\n7.2\t14\n7.8\t14.5\n8.4\t15\n9\t15.5\n9.6\t16\n10.2\t16.5\n10.8\t17\n11.4\t17.5\n12\t18\n12.6\t18.5\n13.2\t19\n13.8\t19.5\n14.4\t20\n15\t20.5\n15.6\t21\n16.2\t21.5\n16.8\t22\n17.4\t22.5\n18\t23\n18.6\t23.5\n19.2\t24\n19.8\t24.5\n20.4\t25\n21\t25.5\n21.6\t26\n22.2\t26.5\n22.8\t27\n23.4\t27.5\n24\t28\n24.6\t28.5\n25.2\t29\n25.8\t29.5\n26.4\t30\n27\t30.5\n27.6\t31\n28.2\t31.5\n28.8\t32\n29.4\t32.5\n30\t33\n30.6\t33.5\n31.2\t34\n31.8\t34.5\n32.4\t35\n33\t35.5\n33.6\t36\n34.2\t35.8\n34.8\t35.6\n35.4\t35.4\n36\t35.2\n36.6\t35\n37.2\t34.8\n37.8\t34.6\n38.4\t34.4\n39\t34.2\n39.6\t34\n40.2\t33.8\n40.8\t33.6\n41.4\t33.4\n42\t33.2\n42.6\t33\n43.2\t32.8\n43.8\t32.6\n44.4\t32.4\n45\t32.2\n45.6\t32\n46.2\t31.8\n46.8\t31.6\n47.4\t31.4\n48\t31.2\n48.6\t31\n49.2\t30.8\n49.8\t30.6\n50.4\t30.4\n51\t30.2\n51.6\t30\n52.2\t29.8\n52.8\t29.6\n53.4\t29.4\n54\t29.2\n54.6\t29\n55.2\t28.8\n55.8\t28.6\n56.4\t28.4\n57\t28.2\n57.6\t28\n58.2\t27.8\n58.8\t27.6\n59.4\t27.4\n60\t27.2\n60.6\t27\n61.2\t26.8\n61.8\t26.6\n62.4\t26.4\n63\t26.2\n63.6\t26\n64.2\t25.8\n64.8\t25.6\n65.4\t25.4\n66\t25.2\n66.6\t25\n67.2\t24.8\n67.8\t24.6\n68.4\t24.4\n69\t24.2\n69.6\t24\n70.2\t23.8\n70.8\t23.6\n71.4\t23.4\n72\t23.2\n72.6\t23\n73.2\t22.8\n73.8\t22.6\n74.4\t22.4\n75\t22.2\n75.6\t22\n76.2\t21.8\n76.8\t21.6\n77.4\t21.4\n78\t21.2\n78.6\t21\n79.2\t20.8\n79.8\t20.6\n80.4\t20.4\n81\t20.2\n81.6\t20\n82.2\t19.8\n82.8\t19.6\n83.4\t19.4\n84\t19.2\n84.6\t19\n85.2\t18.8\n85.8\t18.6\n86.4\t18.4\n87\t18.2\n87.6\t18\n88.2\t17.8\n88.8\t17.6\n89.4\t17.4\n90\t17.2\n90.6\t17\n91.2\t16.8\n91.8\t16.6\n92.4\t16.4\n93\t16.2\n93.6\t16\n94.2\t15.8\n94.8\t15.6\n94.6\t15.4\n94.4\t15.2\n94.2\t15\n94\t14.8\n93.8\t14.6\n93.6\t14.4\n93.4\t14.2\n93.2\t14\n93\t13.8\n92.8\t13.6\n92.6\t13.4\n92.4\t13.2\n92.2\t13\n92\t12.8\n91.8\t12.6\n91.6\t12.4\n91.4\t12.2\n91.2\t12\n91\t11.8\n90.8\t11.6\n90.6\t11.4\n90.4\t11.2\n90.2\t11\n90\t10.8\n89.8\t10.6\n89.6\t10.4\n89.4\t10.2\n89.2\t10\n89\t9.8\n88.8\t9.6\n88.6\t9.4\n88.4\t9.2\n88.2\t9\n88\t8.8\n87.8\t8.6\n87.6\t8.4\n87.4\t8.2\n87.2\t8\n87\t7.8\n86.8\t7.6\n86.6\t7.4\n86.4\t7.2\n86.2\t7\n86\t6.8\n85.8\t6.6\n85.6\t6.4\n85.4\t6.2\n85.2\t6\n85\t5.8\n84.8\t5.6\n84.6\t5.4\n84.4\t5.2\n84.2\t5\n84\t4.8\n83.8\t4.6\n83.6\t4.4\n83.4\t4.2\n83.2\t4\n83\t3.8\n82.8\t3.6\n82.6\t3.4\n82.4\t3.2\n82.2\t3\n82\t2.8\n81.8\t2.6\n81.6\t2.4\n81.4\t2.2\n81.2\t2\n81\t1.8\n80.8\t1.6\n80.6\t1.4\n80.4\t1.2\n80.2\t1\n80\t0.8\n79.8\t0.6\n79.6\t0.4\n79.4\t0.2\n79.2\t-2.71644E-12\n79\t-0.2\n78.8\t-0.4\n78.6\t-0.6\n78.4\t-0.8\n78.2\t-1\n78\t-1.2\n77.8\t-1.4\n77.6\t-1.6\n77.4\t-1.8\n77.2\t-2\n77\t-2.2\n76.8\t-2.4\n76.6\t-2.6\n76.4\t-2.8\n76.2\t-3\n76\t-3.2\n75.8\t-3.4\n75.6\t-3.6\n75.4\t-3.8\n75.2\t-4\n75\t-4.2\n74.8\t-4.4\n74.6\t-4.6\n74.4\t-4.8\n74.2\t-5\n74\t-5.2\n73.8\t-5.4\n73.6\t-5.6\n73.4\t-5.8\n73.2\t-6\n73\t-6.2\n72.8\t-6.4\n72.6\t-6.6\n72.4\t-6.8\n72.2\t-7\n72\t-7.2\n71.8\t-7.4\n71.6\t-7.6\n71.4\t-7.8\n71.2\t-8\n71\t-8.2\n70.8\t-8.4\n70.6\t-8.6\n70.4\t-8.8\n70.2\t-9\n70\t-9.2\n69.8\t-9.4\n69.6\t-9.6\n69.4\t-9.8\n69.2\t-10\n69\t-10.2\n68.8\t-10.4\n68.6\t-10.6\n68.4\t-10.8\n68.2\t-11\n68\t-11.2\n67.8\t-11.4\n67.6\t-11.6\n67.4\t-11.8\n67.2\t-12\n67\t-12.2\n66.8\t-12.4\n66.6\t-12.6\n66.4\t-12.8\n66.2\t-13\n66\t-13.2\n65.8\t-13.4\n65.6\t-13.6\n65.4\t-13.8\n65.2\t-14\n65\t-14.2\n64.8\t-14.4\n64.6\t-14.6\n64.4\t-14.8\n64.2\t-15\n64\t-15.2\n63.8\t-15.4\n63.6\t-15.6\n63.4\t-15.8\n63.2\t-16\n63\t-16.2\n62.8\t-16.4\n62.6\t-16.6\n62.4\t-16.8\n62.2\t-17\n62\t-17.2\n61.8\t-17.4\n61.6\t-17.6\n61.4\t-17.8\n61.2\t-18\n61\t-18.2\n60.8\t-18.4\n60.6\t-18.6\n60.4\t-18.8\n60.2\t-19\n60\t-19.2\n59.8\t-19.4\n59.6\t-19.6\n59.4\t-19.8\n59.2\t-20\n59\t-20.2\n58.8\t-20.4\n58.6\t-20.6\n58.4\t-20.8\n58.2\t-21\n58\t-21.2\n57.8\t-21.4\n57.6\t-21.6\n57.4\t-21.8\n57.2\t-22\n57\t-22.2\n56.8\t-22.4\n56.6\t-22.6\n56.4\t-22.8\n56.2\t-23\n56\t-23.2\n55.8\t-23.4\n55.6\t-23.6\n55.4\t-23.8\n55.2\t-24\n55\t-24.2\n54.8\t-24.4\n54.6\t-24.6\n54.4\t-24.8\n54.2\t-25\n54\t-25.2\n53.8\t-25.4\n53.6\t-25.6\n53.4\t-25.8\n53.2\t-26\n53\t-26.2\n52.8\t-26.4\n52.6\t-26.6\n52.4\t-26.8\n52.2\t-27\n52\t-27.2\n51.8\t-27.4\n51.6\t-27.6\n51.4\t-27.8\n51.2\t-28\n51\t-28.2\n50.8\t-28.4\n50.6\t-28.6\n50.4\t-28.8\n50.2\t-29\n50\t-29.2\n49.8\t-29.4\n49.6\t-29.6\n49.4\t-29.8\n49.2\t-30\n49\t-30.2\n48.8\t-30.4\n48.6\t-30.6\n48.4\t-30.8\n48.2\t-31\n48\t-31.2\n47.8\t-31.4\n47.6\t-31.6\n47.4\t-31.8\n47.2\t-32\n47\t-32.2\n46.8\t-32.4\n46.6\t-32.6\n46.4\t-32.8\n46.2\t-33\n46\t-33.2\n45.8\t-33.4\n45.6\t-33.6\n45.4\t-33.8\n45.2\t-34\n45\t-34.2\n44.8\t-34.4\n44.6\t-34.6\n44.4\t-34.8\n44.2\t-35\n44\t-35.2\n43.8\t-35.4\n43.6\t-35.6\n43.4\t-35.8\n43.2\t-36\n43\t-36.2\n42.8\t-36.4\n42.6\t-36.6\n42.4\t-36.8\n42.2\t-37\n42\t-37.2\n41.8\t-37.4\n41.6\t-37.6\n41.4\t-37.8\n41.2\t-38\n41\t-38.2\n40.8\t-38.4\n40.6\t-38.6\n40.4\t-38.8\n40.2\t-39\n40\t-39.2\n39.8\t-39.4\n39.6\t-39.6\n39.4\t-39.8\n39.2\t-40\n39\t-40.2\n38.8\t-40.4\n38.6\t-40.6\n38.4\t-40.8\n38.2\t-41\n38\t-41.2\n37.8\t-41.4\n37.6\t-41.6\n37.4\t-41.8\n37.2\t-42\n37\t-42.2\n36.8\t-42.4\n36.6\t-42.6\n36.4\t-42.8\n36.2\t-43\n36\t-43.2\n35.8\t-43.4\n35.6\t-43.6\n35.4\t-43.8\n35.2\t-44\n35\t-44.2\n34.8\t-44.4\n34.6\t-44.6\n34.4\t-44.8\n34.2\t-45\n34\t-45.2\n33.8\t-45.4\n33.6\t-45.6\n33.4\t-45.8\n33.2\t-46\n33\t-46.2\n32.8\t-46.4\n32.6\t-46.6\n32.4\t-46.8\n32.2\t-47\n32\t-47.2\n31.8\t-47.4\n31.6\t-47.6\n31.4\t-47.8\n31.2\t-48\n31\t-48.2\n30.8\t-48.4\n30.6\t-48.6\n30.4\t-48.8\n30.2\t-49\n30\t-49.2\n29.8\t-49.4\n29.6\t-49.6\n29.4\t-49.8\n29.2\t-50\n29\t-50.2\n28.8\t-50.4\n28.6\t-50.6\n28.4\t-50.8\n28.2\t-51\n28\t-51.2\n27.8\t-51.4\n27.6\t-51.6\n27.4\t-51.8\n27.2\t-52\n27\t-52.2\n26.8\t-52.4\n26.6\t-52.6\n26.4\t-52.8\n26.2\t-53\n26\t-53.2\n25.8\t-53.4\n25.6\t-53.6\n25.4\t-53.8\n25.2\t-54\n25\t-54.2\n24.8\t-54.4\n24.6\t-54.6\n24.4\t-54.8\n24.2\t-55\n24\t-55.2\n23.8\t-55.4\n23.6\t-55.6\n23.4\t-55.8\n23.2\t-56\n23\t-56.2\n22.8\t-56.4\n22.6\t-56.6\n22.4\t-56.8\n22.2\t-57\n22\t-57.2\n21.8\t-57.4\n21.6\t-57.6\n21.4\t-57.8\n21.2\t-58\n21\t-58.2\n20.8\t-58.4\n20.6\t-58.6\n20.4\t-58.8\n20.2\t-59\n20\t-59.2\n19.8\t-59.4\n19.6\t-59.6\n19.4\t-59.8\n19.2\t-60\n19\t-60.2\n18.8\t-60.4\n18.6\t-60.6\n18.4\t-60.8\n18.2\t-61\n18\t-61.2\n17.8\t-61.4\n17.6\t-61.6\n17.4\t-61.8\n17.2\t-62\n17\t-62.2\n16.8\t-62.4\n16.6\t-62.6\n16.4\t-62.8\n16.2\t-63\n16\t-63.2\n15.8\t-63.4\n15.6\t-63.6\n15.4\t-63.8\n15.2\t-64\n15\t-64.2\n14.8\t-64.4\n14.6\t-64.6\n14.4\t-64.8\n14.2\t-65\n14\t-65.2\n13.8\t-65.4\n13.6\t-65.6\n13.4\t-65.8\n13.2\t-66\n13\t-66.2\n12.8\t-66.4\n12.6\t-66.6\n12.4\t-66.8\n12.2\t-67\n12\t-67.2\n11.8\t-67.4\n11.6\t-67.6\n11.4\t-67.8\n11.2\t-68\n11\t-68.2\n10.8\t-68.4\n10.6\t-68.6\n10.4\t-68.8\n10.2\t-69\n10\t-69.2\n9.8\t-69.4\n9.6\t-69.6\n9.4\t-69.8\n9.2\t-70\n9\t-70.2\n8.8\t-70.4\n8.6\t-70.6\n8.4\t-70.8\n8.2\t-71\n8\t-71.2\n7.8\t-71.4\n7.6\t-71.6\n7.4\t-71.8\n7.2\t-72\n7\t-72.2\n6.8\t-72.4\n6.6\t-72.6\n6.4\t-72.8\n6.2\t-73\n6\t-73.2\n5.8\t-73.4\n5.6\t-73.6\n5.4\t-73.8\n5.2\t-74\n5\t-74.2\n4.8\t-74.4\n4.6\t-74.6\n4.4\t-74.8\n4.2\t-75\n4\t-75.2\n3.8\t-75.4\n3.6\t-75.6\n3.4\t-75.8\n3.2\t-76\n3\t-76.2\n2.8\t-76.4\n2.6\t-76.6\n2.4\t-76.8\n2.2\t-77\n2\t-77.2\n1.8\t-77.4\n1.6\t-77.6\n1.4\t-77.8\n1.2\t-78\n1\t-78.2\n0.8\t-78.4\n0.6\t-78.6\n0.4\t-78.8\n0.2\t-79\n-1.96326E-12\t-79.2\n-0.2\t-79.4\n-0.4\t-79.6\n-0.6\t-79.8\n-0.8\t-80\n-1.4\t-80.2\n-2\t-80.4\n-2.6\t-80.6\n-3.2\t-80.8\n-3.8\t-81\n-4.4\t-81.2\n-5\t-81.4\n-5.6\t-81.6\n-6.2\t-81.8\n-6.8\t-82\n-7.4\t-82.2\n-8\t-82.4\n-8.6\t-82.6\n-9.2\t-82.8\n-9.8\t-83\n-10.4\t-83.2\n-11\t-83.4\n-11.6\t-83.6\n-12.2\t-83.8\n-12.8\t-84\n-13.4\t-84.2\n-14\t-84.4\n-14.6\t-84.6\n-15.2\t-84.8\n-15.8\t-85\n-16.4\t-85.2\n-17\t-85.4\n-17.6\t-85.6\n-18.2\t-85.8\n-18.8\t-86\n-19.4\t-86.2\n-20\t-86.4\n-20.6\t-86.6\n-21.2\t-86.8\n-21.8\t-87\n-22.4\t-87.2\n-23\t-87.4\n-23.6\t-87.6\n-24.2\t-87.8\n-24.8\t-88\n-25.4\t-88.2\n-26\t-88.4\n-26.6\t-88.6\n-27.2\t-88.8\n-27.8\t-89\n-28.4\t-89.2\n-29\t-89.4\n-29.6\t-89.6\n-30.2\t-89.8\n-30.8\t-90\n-31.4\t-90.2\n-32\t-90.4\n-32.6\t-90.6\n-33.2\t-90.8\n-33.8\t-91\n-34.4\t-91.2\n-35\t-91.4\n-35.6\t-91.6\n-36.2\t-91.8\n-36.8\t-92\n-37.4\t-92.2\n-38\t-92.4\n-38.6\t-92.6\n-39.2\t-92.8\n-39.8\t-93\n-40.4\t-93.2\n-41\t-93.4\n-41.6\t-93.6\n-42.2\t-93.8\n-42.8\t-94\n-43.4\t-93.6\n-44\t-93.2\n-44.6\t-92.8\n-45.2\t-92.4\n-45.8\t-92\n-46.4\t-91.6\n-47\t-91.2\n-47.6\t-90.8\n-48.2\t-90.4\n-48.8\t-90\n-49.4\t-89.6\n-50\t-89.2\n-50.6\t-88.8\n-51.2\t-88.4\n-51.8\t-88\n-52.4\t-87.6\n-53\t-87.2\n-53.6\t-86.8\n-54.2\t-86.4\n-54.8\t-86\n-55.4\t-85.6\n-56\t-85.2\n-56.6\t-84.8\n-57.2\t-84.4\n-57.8\t-84\n-58.4\t-83.6\n-59\t-83.2\n-59.6\t-82.8\n-60.2\t-82.4\n-60.8\t-82\n-61.4\t-81.6\n-62\t-81.2\n-62.6\t-80.8\n-63.2\t-80.4\n-63.8\t-80\n-64.4\t-79.6\n-65\t-79.2\n-65.6\t-78.8\n-66.2\t-78.4\n-66.8\t-78\n-67.4\t-77.6\n-68\t-77.2\n-68.6\t-76.8\n-69.2\t-76.4\n-69.8\t-76\n-70.4\t-75.6\n-71\t-75.2\n-71.6\t-74.8\n-72.2\t-74.4\n-72.8\t-74\n-73.4\t-73.6\n-74\t-73.2\n-74.6\t-72.8\n-75.2\t-72.4\n-75.8\t-72\n-76.4\t-71.6\n-77\t-71.2\n-77.6\t-70.8\n-78.2\t-70.4\n-78.8\t-70\n-79.4\t-69.6\n-80\t-69.2\n-80.6\t-68.8\n-81.2\t-68.4\n-81.8\t-68\n-82.4\t-67.6\n-83\t-67.2\n-83.6\t-66.8\n-84.2\t-66.4\n-84.8\t-66\n-85.4\t-65.6\n-86\t-65.2\n-86.6\t-64.8\n-87.2\t-64.4\n-87.8\t-64\n-88.4\t-63.6\n-89\t-63.2\n-89.6\t-62.8\n-90.2\t-62.4\n-90.8\t-62\n-90.6\t-61.6\n-90.4\t-61.2\n-90.2\t-60.8\n-90\t-60.4\n-89.8\t-60\n-89.6\t-59.6\n-89.4\t-59.2\n-89.2\t-58.8\n-89\t-58.4\n-88.8\t-58\n-88.6\t-57.6\n-88.4\t-57.2\n-88.2\t-56.8\n-88\t-56.4\n-87.8\t-56\n-87.6\t-55.6\n-87.4\t-55.2\n-87.2\t-54.8\n-87\t-54.4\n-86.8\t-54\n-86.6\t-53.6\n-86.4\t-53.2\n-86.2\t-52.8\n-86\t-52.4\n-85.8\t-52\n-85.6\t-51.6\n-85.4\t-51.2\n-85.2\t-50.8\n-85\t-50.4\n-84.8\t-50\n-84.6\t-49.6\n-84.4\t-49.2\n-84.2\t-48.8\n-84\t-48.4\n-83.8\t-48\n-83.6\t-47.6\n-83.4\t-47.2\n-83.2\t-46.8\n-83\t-46.4\n-82.8\t-46\n-82.6\t-45.6\n-82.4\t-45.2\n-82.2\t-44.8\n-82\t-44.4\n-81.8\t-44\n-81.6\t-43.6\n-81.4\t-43.2\n-81.2\t-42.8\n-81\t-42.4\n-80.8\t-42\n-80.6\t-41.6\n-80.4\t-41.2\n-80.2\t-40.8\n-80\t-40.4\n-79.8\t-40\n-79.6\t-39.6\n-79.4\t-39.2\n-79.2\t-38.8\n-79\t-38.4\n-78.8\t-38\n-78.6\t-37.6\n-78.4\t-37.2\n-78.2\t-36.8\n-78\t-36.4\n-77.8\t-36\n-77.6\t-35.6\n-77.4\t-35.2\n-77.2\t-34.8\n-77\t-34.4\n-76.8\t-34\n-76.6\t-33.6\n-76.4\t-33.2\n-76.2\t-32.8\n-76\t-32.4\n-75.8\t-32\n-75.6\t-31.6\n-75.4\t-31.2\n-75.2\t-30.8\n-75\t-30.4\n-74.8\t-30\n-74.6\t-29.6\n-74.4\t-29.2\n-74.2\t-28.8\n-74\t-28.4\n-73.8\t-28\n-73.6\t-27.6\n-73.4\t-27.2\n-73.2\t-26.8\n-73\t-26.4\n-72.8\t-26\n-72.6\t-25.6\n-72.4\t-25.2\n-72.2\t-24.8\n-72\t-24.4\n-71.8\t-24\n-71.6\t-23.6\n-71.4\t-23.2\n-71.2\t-22.8\n-71\t-22.4\n-70.8\t-22\n-70.6\t-21.6\n-70.4\t-21.2\n-70.2\t-20.8\n-70\t-20.4\n-69.8\t-20\n-69.6\t-19.6\n-69.4\t-19.2\n-69.2\t-18.8\n-69\t-18.4\n-68.8\t-18\n-68.6\t-17.6\n-68.4\t-17.2\n-68.2\t-16.8\n-68\t-16.4\n-67.8\t-16\n-67.6\t-15.6\n-67.4\t-15.2\n-67.2\t-14.8\n-67\t-14.4\n-66.8\t-14\n-66.6\t-13.6\n-66.4\t-13.2\n-66.2\t-12.8\n-66\t-12.4\n-65.8\t-12\n-65.6\t-11.6\n-65.4\t-11.2\n-65.2\t-10.8\n-65\t-10.4\n-64.8\t-10\n-64.6\t-9.6\n-64.4\t-9.2\n-64.2\t-8.8\n-64\t-8.4\n-63.8\t-8\n-63.6\t-7.6\n-63.4\t-7.2\n-63.2\t-6.8\n-63\t-6.4\n-62.8\t-6\n-62.6\t-5.6\n-62.4\t-5.2\n-62.2\t-4.8\n-62\t-4.4\n-61.8\t-4\n-61.6\t-3.6\n-61.4\t-3.2\n-61.2\t-2.8\n-61\t-2.4\n-60.8\t-2\n-60.6\t-1.6\n-60.4\t-1.2\n-60.2\t-0.8\n-60\t-0.4\n-59.8\t0\n-59.6\t0\n-59.4\t0.3\n-59.2\t0.6\n-59\t0.9\n-58.8\t1.2\n-58.6\t1.5\n-58.4\t1.8\n-58.2\t2.1\n-58\t2.4\n-57.8\t2.7\n-57.6\t3\n-57.4\t3.3\n-57.2\t3.6\n-57\t3.9\n-56.8\t4.2\n-56.6\t4.5\n-56.4\t4.8\n-56.2\t5.1\n-56\t5.4\n-55.8\t5.7\n-55.6\t6\n-55.4\t6.3\n-55.2\t6.6\n-55\t6.9\n-54.8\t7.2\n-54.6\t7.5\n-54.4\t7.8\n-54.2\t8.1\n-54\t8.4\n-53.8\t8.7\n-53.6\t9\n-53.4\t9.3\n-53.2\t9.6\n-53\t9.9\n-52.8\t10.2\n-52.6\t10.5\n-52.4\t10.8\n-52.2\t11.1\n-52\t11.4\n-51.8\t11.7\n-51.6\t12\n-51.4\t12.3\n-51.2\t12.6\n-51\t12.9\n-50.8\t13.2\n-50.6\t13.5\n-50.4\t13.8\n-50.2\t14.1\n-50\t14.4\n-49.8\t14.7\n-49.6\t15\n-49.4\t15.3\n-49.2\t15.6\n-49\t15.9\n-48.8\t16.2\n-48.6\t16.5\n-48.4\t16.8\n-48.2\t17.1\n-48\t17.4\n-47.8\t17.7\n-47.6\t18\n-47.4\t18.3\n-47.2\t18.6\n-47\t18.9\n-46.8\t19.2\n-46.6\t19.5\n-46.4\t19.8\n-46.2\t20.1\n-46\t20.4\n-45.8\t20.7\n-45.6\t21\n-45.4\t21.3\n-45.2\t21.6\n-45\t21.9\n-44.8\t22.2\n-44.6\t22.5\n-44.4\t22.8\n-44.2\t23.1\n-44\t23.4\n-43.8\t23.7\n-43.6\t24\n-43.4\t24.3\n-43.2\t24.6\n-43\t24.9\n-42.8\t25.2\n-42.6\t25.5\n-42.4\t25.8\n-42.2\t26.1\n-42\t26.4\n-41.8\t26.7\n-41.6\t27\n-41.4\t27.3\n-41.2\t27.6\n-41\t27.9\n-40.8\t28.2\n-40.6\t28.5\n-40.4\t28.8\n-40.2\t29.1\n-40\t29.4\n-39.8\t29.7\n-39.6\t30\n-39.4\t30.3\n-39.2\t30.6\n-39\t30.9\n-38.8\t31.2\n-38.6\t31.5\n-38.4\t31.8\n-38.2\t32.1\n-38\t32.4\n-37.8\t32.7\n-37.6\t33\n-37.4\t33.3\n-37.2\t33.6\n-37\t33.9\n-36.8\t34.2\n-36.6\t34.5\n-36.4\t34.8\n-36.2\t35.1\n-36\t35.4\n-35.8\t35.7\n-35.6\t36\n-35.4\t36.3\n-35.2\t36.6\n-35\t36.9\n-34.8\t37.2\n-34.6\t37.5\n-34.4\t37.8\n-34.2\t38.1\n-34\t38.4\n-33.8\t38.7\n-33.6\t39\n-33.4\t39.3\n-33.2\t39.6\n-33\t39.9\n-32.8\t40.2\n-32.6\t40.5\n-32.4\t40.8\n-32.2\t41.1\n-32\t41.4\n-31.8\t41.7\n-31.6\t42\n-31.4\t42.3\n-31.2\t42.6\n-31\t42.9\n-30.8\t43.2\n-30.6\t43.5\n-30.4\t43.8\n-30.2\t44.1\n-30\t44.4\n-29.8\t44.7\n-29.6\t45\n-29.4\t45.3\n-29.2\t45.6\n-29\t45.9\n-28.8\t46.2\n-28.6\t46.5\n-28.4\t46.8\n-28.2\t47.1\n-28\t47.4\n-27.8\t47.7\n-27.6\t48\n-27.4\t48.3\n-27.2\t48.6\n-27\t48.9\n-26.8\t49.2\n-26.6\t49.5\n-26.4\t49.8\n-26.2\t50.1\n-26\t50.4\n-25.8\t50.7\n-25.6\t51\n-25.4\t51.3\n-25.2\t51.6\n-25\t51.9\n-24.8\t52.2\n-24.6\t52.5\n-24.4\t52.8\n-24.2\t53.1\n-24\t53.4\n-23.8\t53.7\n-23.6\t54\n-23.4\t54.3\n-23.2\t54.6\n-23\t54.9\n-22.8\t55.2\n-22.6\t55.5\n-22.4\t55.8\n-22.2\t56.1\n-22\t56.4\n-21.8\t56.7\n-21.6\t57\n-21.4\t57.3\n-21.2\t57.6\n-21\t57.9\n-20.8\t58.2\n-20.6\t58.5\n-20.4\t58.8\n-20.2\t59.1\n-20\t59.4\n-19.8\t59.7\n-19.6\t60\n-19.4\t60.3\n-19.2\t60.6\n-19\t60.9\n-18.8\t61.2\n-18.6\t61.5\n-18.4\t61.8\n-18.2\t62.1\n-18\t62.4\n-17.8\t62.7\n-17.6\t63\n-17.4\t63.3\n-17.2\t63.6\n-17\t63.9\n-16.8\t64.2\n-16.6\t64.5\n-16.4\t64.8\n-16.2\t65.1\n-16\t65.4\n-15.8\t65.7\n-15.6\t66\n-15.4\t66.3\n-15.2\t66.6\n-15\t66.9\n-14.8\t67.2\n-14.6\t67.5\n-14.4\t67.8\n-14.2\t68.1\n-14\t68.4\n-13.8\t68.7\n-13.6\t69\n-13.4\t69.3\n-13.2\t69.6\n-13\t69.9\n-12.8\t70.2\n-12.6\t70.5\n-12.4\t70.8\n-12.2\t71.1\n-12\t71.4\n-11.8\t71.7\n-11.6\t72\n-11.4\t72.3\n-11.2\t72.6\n-11\t72.9\n-10.8\t73.2\n-10.6\t73.5\n-10.4\t73.8\n-10.2\t74.1\n-10\t74.4\n-9.8\t74.7\n-9.6\t75\n-9.4\t75.3\n-9.2\t75.6\n-9\t75.9\n-8.8\t76.2\n-8.6\t76.5\n-8.4\t76.8\n-8.2\t77.1\n-8\t77.4\n-7.8\t77.7\n-7.6\t78\n-7.4\t78.3\n-7.2\t78.6\n-7\t78.9\n-6.8\t79.2\n-6.6\t79.5\n-6.4\t79.8\n-6.2\t80.1\n-6\t80.4\n-5.8\t80.7\n-5.6\t81\n-5.4\t81.3\n-5.2\t81.6\n-5\t81.9\n-4.8\t82.2\n-4.6\t82.5\n-4.4\t82.8\n-4.2\t83.1\n-4\t83.4\n-3.8\t83.7\n-3.6\t84\n-3.4\t84.3\n-3.2\t84.6\n-3\t84.9\n-2.8\t85.2\n-2.6\t85.5\n-2.4\t85.8\n-2.2\t86.1\n-2\t86.4\n-1.8\t86.7\n-1.6\t87\n-1.4\t87.3\n-1.2\t87.6\n-1\t87.9\n-0.8\t88.2\n-0.6\t88.5\n-0.4\t88.8\n-0.2\t89.1\n-1.06076E-12\t89.4\n0.2\t89.7\n0.4\t90\n0.6\t90.3\n0.8\t90.6\n1\t90.9\n1.2\t91.2\n1.4\t91.5\n1.6\t91.8\n1.8\t92.1\n2\t92.4\n2.2\t92.7\n2.4\t93\n2.6\t93.3\n2.8\t93.6\n3\t93.9\n3.2\t94.2\n3.4\t94.5\n3.6\t94.8\n3.8\t95.1\n4\t95.4\n4.2\t95.7\n4.4\t96\n4.6\t96.3\n4.8\t96.6\n5\t96.9\n5.2\t97.2\n5.4\t97.5\n5.6\t97.3\n5.8\t97.1\n6\t96.9\n6.2\t96.7\n6.4\t96.5\n6.6\t96.3\n6.8\t96.1\n7\t95.9\n7.2\t95.7\n7.4\t95.5\n7.6\t95.3\n7.8\t95.1\n8\t94.9\n8.2\t94.7\n8.4\t94.5\n8.6\t94.3\n8.8\t94.1\n9\t93.9\n9.2\t93.7\n9.4\t93.5\n9.6\t93.3\n9.8\t93.1\n10\t92.9\n10.2\t92.7\n10.4\t92.5\n10.6\t92.3\n10.8\t92.1\n11\t91.9\n11.2\t91.7\n11.4\t91.5\n11.6\t91.3\n11.8\t91.1\n12\t90.9\n12.2\t90.7\n12.4\t90.5\n12.6\t90.3\n12.8\t90.1\n13\t89.9\n13.2\t89.7\n13.4\t89.5\n13.6\t89.3\n13.8\t89.1\n14\t88.9\n14.2\t88.7\n14.4\t88.5\n14.6\t88.3\n14.8\t88.1\n15\t87.9\n15.2\t87.7\n15.4\t87.5\n15.6\t87.3\n15.8\t87.1\n16\t86.9\n16.2\t86.7\n16.4\t86.5\n16.6\t86.3\n16.8\t86.1\n17\t85.9\n17.2\t85.7\n17.4\t85.5\n17.6\t85.3\n17.8\t85.1\n18\t84.9\n18.2\t84.7\n18.4\t84.5\n18.6\t84.3\n18.8\t84.1\n19\t83.9\n19.2\t83.7\n19.4\t83.5\n19.6\t83.3\n19.8\t83.1\n20\t82.9\n20.2\t82.7\n20.4\t82.5\n20.6\t82.3\n20.8\t82.1\n21\t81.9\n21.2\t81.7\n21.4\t81.5\n21.6\t81.3\n21.8\t81.1\n22\t80.9\n22.2\t80.7\n22.4\t80.5\n22.6\t80.3\n22.8\t80.1\n23\t79.9\n23.2\t79.7\n23.4\t79.5\n23.6\t79.3\n23.8\t79.1\n24\t78.9\n24.2\t78.7\n24.4\t78.5\n24.6\t78.3\n24.8\t78.1\n25\t77.9\n25.2\t77.7\n25.4\t77.5\n25.6\t77.3\n25.8\t77.1\n26\t76.9\n26.2\t76.7\n26.4\t76.5\n26.6\t76.3\n26.8\t76.1\n27\t75.9\n27.2\t75.7\n27.4\t75.5\n27.6\t75.3\n27.8\t75.1\n28\t74.9\n28.2\t74.7\n28.4\t74.5\n28.6\t74.3\n28.8\t74.1\n29\t73.9\n29.2\t73.7\n29.4\t73.5\n29.6\t73.3\n29.8\t73.1\n30\t72.9\n30.2\t72.7\n30.4\t72.5\n30.6\t72.3\n30.8\t72.1\n31\t71.9\n31.2\t71.7\n31.4\t71.5\n31.6\t71.3\n31.8\t71.1\n32\t70.9\n32.2\t70.7\n32.4\t70.5\n32.6\t70.3\n32.8\t70.1\n33\t69.9\n33.2\t69.7\n33.4\t69.5\n33.6\t69.3\n33.8\t69.1\n34\t68.9\n34.2\t68.7\n34.4\t68.5\n34.6\t68.3\n34.8\t68.1\n35\t67.9\n35.2\t67.7\n35.4\t67.5\n35.6\t67.3\n35.8\t67.1\n36\t66.9\n36.2\t66.7\n36.4\t66.5\n36.6\t66.3\n36.8\t66.1\n37\t65.9\n37.2\t65.7\n37.4\t65.5\n37.6\t65.3\n37.8\t65.1\n38\t64.9\n38.2\t64.7\n38.4\t64.5\n38.6\t64.3\n38.8\t64.1\n39\t63.9\n39.2\t63.7\n39.4\t63.5\n39.6\t63.3\n39.8\t63.1\n40\t62.9\n40.2\t62.7\n40.4\t62.5\n40.6\t62.3\n40.8\t62.1\n41\t61.9\n41.2\t61.7\n41.4\t61.5\n41.6\t61.3\n41.8\t61.1\n42\t60.9\n42.2\t60.7\n42.4\t60.5\n42.6\t60.3\n42.8\t60.1\n43\t59.9\n43.2\t59.7\n43.4\t59.5\n43.6\t59.3\n43.8\t59.1\n44\t58.9\n44.2\t58.7\n44.4\t58.5\n44.6\t58.3\n44.8\t58.1\n45\t57.9\n45.2\t57.7\n45.4\t57.5\n45.6\t57.3\n45.8\t57.1\n46\t56.9\n46.2\t56.7\n46.4\t56.5\n46.6\t56.3\n46.8\t56.1\n47\t55.9\n47.2\t55.7\n47.4\t55.5\n47.6\t55.3\n47.8\t55.1\n48\t54.9\n48.2\t54.7\n48.4\t54.5\n48.6\t54.3\n48.8\t54.1\n49\t53.9\n49.2\t53.7\n49.4\t53.5\n49.6\t53.3\n49.8\t53.1\n50\t52.9\n50.2\t52.7\n50.4\t52.5\n50.6\t52.3\n50.8\t52.1\n51\t51.9\n51.2\t51.7\n51.4\t51.5\n51.6\t51.3\n51.8\t51.1\n52\t50.9\n52.2\t50.7\n52.4\t50.5\n52.6\t50.3\n52.8\t50.1\n53\t49.9\n53.2\t49.7\n53.4\t49.5\n53.6\t49.3\n53.8\t49.1\n54\t48.9\n54.2\t48.7\n54.4\t48.5\n54.6\t48.3\n54.8\t48.1\n55\t47.9\n55.2\t47.7\n55.4\t47.5\n55.6\t47.3\n55.8\t47.1\n56\t46.9\n56.2\t46.7\n56.4\t46.5\n56.6\t46.3\n56.8\t46.1\n57\t45.9\n57.2\t45.7\n57.4\t45.5\n57.6\t45.3\n57.8\t45.1\n58\t44.9\n58.2\t44.7\n58.4\t44.5\n58.6\t44.3\n58.8\t44.1\n59\t43.9\n59.2\t43.7\n59.4\t43.5\n59.6\t43.3\n59.8\t43.1\n60\t42.9\n60.2\t42.7\n60.4\t42.5\n60.6\t42.3\n60.8\t42.1\n61\t41.9\n61.2\t41.7\n61.4\t41.5\n61.6\t41.3\n61.8\t41.1\n62\t40.9\n62.2\t40.7\n62.4\t40.5\n62.6\t40.3\n62.8\t40.1\n63\t39.9\n63.2\t39.7\n63.4\t39.5\n63.6\t39.3\n63.8\t39.1\n64\t38.9\n64.2\t38.7\n64.4\t38.5\n64.6\t38.3\n64.8\t38.1\n65\t37.9\n65.2\t37.7\n65.4\t37.5\n65.6\t37.3\n65.8\t37.1\n66\t36.9\n66.2\t36.7\n66.4\t36.5\n66.6\t36.3\n66.2\t36.1\n65.8\t35.9\n65.4\t35.7\n65\t35.5\n64.6\t35.3\n64.2\t35.1\n63.8\t34.9\n63.4\t34.7\n63\t34.5\n62.6\t34.3\n62.2\t34.1\n61.8\t33.9\n61.4\t33.7\n61\t33.5\n60.6\t33.3\n60.2\t33.1\n59.8\t32.9\n59.4\t32.7\n59\t32.5\n58.6\t32.3\n58.2\t32.1\n57.8\t31.9\n57.4\t31.7\n57\t31.5\n56.6\t31.3\n56.2\t31.1\n55.8\t30.9\n55.4\t30.7\n55\t30.5\n54.6\t30.3\n54.2\t30.1\n53.8\t29.9\n53.4\t29.7\n53\t29.5\n52.6\t29.3\n52.2\t29.1\n51.8\t28.9\n51.4\t28.7\n51\t28.5\n50.6\t28.3\n50.2\t28.1\n49.8\t27.9\n49.4\t27.7\n49\t27.5\n48.6\t27.3\n48.2\t27.1\n47.8\t26.9\n47.4\t26.7\n47\t26.5\n46.6\t26.3\n46.2\t26.1\n45.8\t25.9\n45.4\t25.7\n45\t25.5\n44.6\t25.3\n44.2\t25.1\n43.8\t24.9\n43.4\t24.7\n43\t24.5\n42.6\t24.3\n42.2\t24.1\n41.8\t23.9\n41.4\t23.7\n41\t23.5\n40.6\t23.3\n40.2\t23.1\n39.8\t22.9\n39.4\t22.7\n39\t22.5\n38.6\t22.3\n38.2\t22.1\n37.8\t21.9\n37.4\t21.7\n37\t21.5\n36.6\t21.3\n36.2\t21.1\n35.8\t20.9\n35.4\t20.7\n35\t20.5\n34.6\t20.3\n34.2\t20.1\n33.8\t19.9\n33.4\t19.7\n33\t19.5\n32.6\t19.3\n32.2\t19.1\n31.8\t18.9\n31.4\t18.7\n31\t18.5\n30.6\t18.3\n30.2\t18.1\n29.8\t17.9\n29.4\t17.7\n29\t17.5\n28.6\t17.3\n28.2\t17.1\n27.8\t16.9\n27.4\t16.7\n27\t16.5\n26.6\t16.3\n26.2\t16.1\n25.8\t15.9\n25.4\t15.7\n25\t15.5\n24.6\t15.3\n24.2\t15.1\n23.8\t14.9\n23.4\t14.7\n23\t14.5\n22.6\t14.3\n22.2\t14.1\n21.8\t13.9\n21.4\t13.7\n21\t13.5\n20.6\t13.3\n20.2\t13.1\n19.8\t12.9\n19.4\t12.7\n19\t12.5\n18.6\t12.3\n18.2\t12.1\n17.8\t11.9\n17.4\t11.7\n17\t11.5\n16.6\t11.3\n16.2\t11.1\n15.8\t10.9\n15.4\t10.7\n15\t11.3\n14.6\t11.9\n14.2\t12.5\n13.8\t13.1\n13.4\t13.7\n13\t14.3\n12.6\t14.9\n12.2\t15.5\n11.8\t16.1\n11.4\t16.7\n11\t17.3\n10.6\t17.9\n10.2\t18.5\n9.8\t19.1\n9.4\t19.7\n9\t20.3\n8.6\t20.9\n8.2\t21.5\n7.8\t22.1\n7.4\t22.7\n7\t23.3\n6.6\t23.9\n6.2\t24.5\n5.8\t25.1\n5.4\t25.7\n5\t26.3\n4.6\t26.9\n4.2\t27.5\n3.8\t28.1\n3.4\t28.7\n3\t29.3\n2.6\t29.9\n2.2\t30.5\n1.8\t31.1\n1.4\t31.7\n1\t32.3\n0.6\t32.9\n0.2\t33.5\n-0.2\t34.1\n-0.6\t34.7\n-1\t35.3\n-1.4\t35.9\n-1.8\t36.5\n-2.2\t37.1\n-2.6\t37.7\n-3\t38.3\n-3.4\t38.9\n-3.8\t39.5\n-4.2\t40.1\n-4.6\t40.7\n-5\t41.3\n-5.4\t41.9\n-5.8\t42.5\n-6.2\t43.1\n-6.6\t43.7\n-7\t44.3\n-7.4\t44.9\n-7.8\t45.5\n-8.2\t46.1\n-8.6\t46.7\n-9\t47.3\n-9.4\t47.9\n-9.8\t48.5\n-10.2\t49.1\n-10.6\t49.7\n-11\t50.3\n-11.4\t50.9\n-11.8\t51.5\n-12.2\t52.1\n-12.6\t52.7\n-13\t53.3\n-13.4\t53.9\n-13.8\t54.5\n-14.2\t55.1\n-14.6\t55.7\n-15\t56.3\n-15.4\t56.9\n-15.8\t57.5\n-16.2\t58.1\n-16.6\t58.7\n-17\t59.3\n-17.4\t59.9\n-17.8\t60.5\n-18.2\t61.1\n-18.6\t61.7\n-19\t62.3\n-19.4\t62.9\n-19.8\t63.5\n-20.2\t64.1\n-20.6\t64.7\n-21\t65.3\n-21.4\t65.9\n-21.8\t66.5\n-22.2\t67.1\n-22.6\t67.7\n-23\t68.3\n-23.4\t68.9\n-23.8\t69.5\n-24.2\t70.1\n-24.6\t70.7\n-25\t71.3\n-25.4\t71.9\n-25.8\t72.5\n-26.2\t73.1\n-26.6\t73.7\n-27\t74.3\n-27.4\t74.9\n-27.8\t75.5\n-28.2\t76.1\n-28.6\t76.7\n-29\t77.3\n-29.4\t77.9\n-29.8\t78.5\n-30.2\t79.1\n-30.6\t79.7\n-31\t80.3\n-31.4\t80.9\n-31.8\t81.5\n-32.2\t82.1\n-32.6\t82.7\n-33\t83.3\n-33.4\t83.9\n-33.8\t84.5\n-34.2\t85.1\n-34.6\t85.7\n-35\t86.3\n-35.4\t86.9\n-35.8\t87.5\n-36.2\t88.1\n-36.6\t88.7\n-37\t89.3\n-37.4\t89.9\n-37.8\t90.5\n-38.2\t91.1\n-38.6\t91.7\n-39\t92.3\n-39.4\t92.9\n-39.8\t93.5\n-40.2\t94.1\n-40.6\t93.8\n-41\t93.5\n-41.4\t93.2\n-41.8\t92.9\n-42.2\t92.6\n-42.6\t92.3\n-43\t92\n-43.4\t91.7\n-43.8\t91.4\n-44.2\t91.1\n-44.6\t90.8\n-45\t90.5\n-45.4\t90.2\n-45.8\t89.9\n-46.2\t89.6\n-46.6\t89.3\n-47\t89\n-47.4\t88.7\n-47.8\t88.4\n-48.2\t88.1\n-48.6\t87.8\n-49\t87.5\n-49.4\t87.2\n-49.8\t86.9\n-50.2\t86.6\n-50.6\t86.3\n-51\t86\n-51.4\t85.7\n-51.8\t85.4\n-52.2\t85.1\n-52.6\t84.8\n-53\t84.5\n-53.4\t84.2\n-53.8\t83.9\n-54.2\t83.6\n-54.6\t83.3\n-55\t83\n-54.4\t82.7\n-53.8\t82.4\n-53.2\t82.1\n-52.6\t81.8\n-52\t81.5\n-51.4\t81.2\n-50.8\t80.9\n-50.2\t80.6\n-49.6\t80.3\n-49\t80\n-48.4\t79.7\n-47.8\t79.4\n-47.2\t79.1\n-46.6\t78.8\n-46\t78.5\n-45.4\t78.2\n-44.8\t77.9\n-44.2\t77.6\n-43.6\t77.3\n-43\t77\n-42.4\t76.7\n-41.8\t76.4\n-41.2\t76.1\n-40.6\t75.8\n-40\t75.5\n-39.4\t75.2\n-38.8\t74.9\n-38.2\t74.6\n-37.6\t74.3\n-37\t74\n-36.4\t73.7\n-35.8\t73.4\n-35.2\t73.1\n-34.6\t72.8\n-34\t72.5\n-33.4\t72.2\n-32.8\t71.9\n-32.2\t71.6\n-31.6\t71.3\n-31\t71\n-30.4\t70.7\n-29.8\t70.4\n-29.2\t70.1\n-28.6\t69.8\n-28\t69.5\n-27.4\t69.2\n-26.8\t68.9\n-26.2\t68.6\n-25.6\t68.3\n-25\t68\n-24.4\t67.7\n-23.8\t67.4\n-23.2\t67.1\n-22.6\t66.8\n-22\t66.5\n-21.4\t66.2\n-20.8\t65.9\n-20.2\t65.6\n-19.6\t65.3\n-19\t65\n-18.4\t64.7\n-17.8\t64.4\n-17.2\t64.1\n-16.6\t63.8\n-16\t63.5\n-15.4\t63.2\n-14.8\t62.9\n-14.2\t62.6\n-13.6\t62.3\n-13\t62\n-12.4\t61.7\n-11.8\t61.4\n-11.2\t61.1\n-10.6\t60.8\n-10\t60.5\n-9.4\t60.2\n-8.8\t59.9\n-8.2\t59.6\n-7.6\t59.3\n-7\t59\n-6.4\t58.7\n-5.8\t58.4\n-5.2\t58.1\n-4.6\t57.8\n-4\t57.5\n-3.4\t57.2\n-2.8\t56.9\n-2.2\t56.6\n-1.6\t56.3\n-1\t56\n-0.4\t55.7\n0.2\t55.4\n0.8\t55.1\n1.4\t54.8\n2\t54.5\n2.6\t54.2\n3.2\t53.9\n3.8\t53.6\n4.4\t53.3\n5\t53\n5.6\t52.7\n6.2\t52.4\n6.8\t52.1\n7.4\t51.8\n8\t51.5\n8.6\t51.2\n9.2\t50.9\n9.8\t50.6\n10.4\t50.3\n11\t50\n11.6\t49.7\n12.2\t49.4\n12.8\t49.1\n13.4\t48.8\n14\t48.5\n14.6\t48.2\n15.2\t47.9\n15.8\t47.6\n16.4\t47.3\n17\t47\n17.6\t46.7\n18.2\t46.4\n18.8\t46.1\n19.4\t45.8\n20\t45.5\n20.6\t45.2\n21.2\t44.9\n21.8\t44.6\n22.4\t44.3\n23\t44\n23.6\t43.7\n24.2\t43.4\n24.8\t43.1\n25.4\t42.8\n26\t42.5\n26.6\t42.2\n27.2\t41.9\n27.8\t41.6\n28.4\t41.3\n29\t41\n29.6\t40.7\n30.2\t40.4\n30.8\t40.1\n31.4\t39.8\n32\t39.5\n32.6\t39.2\n33.2\t38.9\n33.8\t38.6\n34.4\t38.3\n35\t38\n35.6\t37.7\n36.2\t37.4\n36.8\t37.1\n37.4\t36.8\n38\t36.5\n38.6\t36.2\n39.2\t35.9\n39.8\t35.6\n40.4\t35.3\n41\t35\n41.6\t34.7\n42.2\t34.4\n42.8\t34.1\n43.4\t33.8\n44\t33.5\n44.6\t33.2\n45.2\t32.9\n45.8\t32.6\n46.4\t32.3\n47\t32\n47.6\t31.7\n48.2\t31.4\n48.8\t31.1\n49.4\t30.8\n50\t30.5\n50.6\t30.2\n51.2\t29.9\n51.8\t29.6\n52.4\t29.3\n53\t29\n53.6\t28.7\n54.2\t28.4\n54.8\t28.1\n55.4\t27.8\n56\t27.5\n56.6\t27.2\n57.2\t26.9\n57.8\t26.6\n58.4\t26.3\n59\t26\n59.6\t25.7\n60.2\t25.4\n60.8\t25.1\n61.4\t24.8\n62\t24.5\n62.6\t24.2\n63.2\t23.9\n63.8\t23.6\n64.4\t23.3\n65\t23\n65.6\t22.7\n66.2\t22.4\n66.8\t22.1\n67.4\t21.8\n68\t21.5\n68.6\t21.2\n69.2\t20.9\n69.8\t20.6\n70.4\t20.3\n71\t20\n71.6\t19.7\n72.2\t19.4\n72.8\t19.1\n73.4\t18.8\n74\t18.5\n74.6\t18.2\n75.2\t17.9\n75.8\t17.6\n76.4\t17.3\n77\t17\n77.6\t16.7\n78.2\t16.4\n78.8\t16.1\n79.4\t15.8\n80\t15.5\n80.6\t15.2\n81.2\t14.9\n81.8\t14.6\n82.4\t14.3\n83\t14\n83.6\t13.7\n84.2\t13.4\n84.8\t13.1\n85.4\t12.8\n86\t12.5\n86.6\t12.2\n87.2\t11.9\n87.8\t11.6\n88.4\t11.3\n89\t11\n89.6\t10.7\n90.2\t10.4\n90.8\t10.1\n91.4\t9.8\n92\t9.5\n92.6\t9.2\n93.2\t8.9\n93.8\t8.6\n94.4\t8.3\n94.2\t8\n94\t7.7\n93.8\t7.4\n93.6\t7.1\n93.4\t6.8\n93.2\t6.5\n93\t6.2\n92.8\t5.9\n92.6\t5.6\n92.4\t5.3\n92.2\t5\n92\t4.7\n91.8\t4.4\n91.6\t4.1\n91.4\t3.8\n91.2\t3.5\n91\t3.2\n90.8\t2.9\n90.6\t2.6\n90.4\t2.3\n90.2\t2\n90\t1.7\n89.8\t1.4\n89.6\t1.1\n89.4\t0.8\n89.2\t0.5\n89\t0.2\n88.8\t-0.1\n88.6\t-0.4\n88.4\t-0.7\n88.2\t-1\n88\t-1.3\n87.8\t-1.6\n87.6\t-1.9\n87.4\t-2.2\n87.2\t-2.5\n87\t-2.8\n86.8\t-3.1\n86.6\t-3.4\n86.4\t-3.7\n86.2\t-4\n86\t-4.3\n85.8\t-4.6\n85.6\t-4.9\n85.4\t-5.2\n85.2\t-5.5\n85\t-5.8\n84.8\t-6.1\n84.6\t-6.4\n84.4\t-6.7\n84.2\t-7\n84\t-7.3\n83.8\t-7.6\n83.6\t-7.9\n83.4\t-8.2\n83.2\t-8.5\n83\t-8.8\n82.8\t-9.1\n82.6\t-9.4\n82.4\t-9.7\n82.2\t-10\n82\t-10.3\n81.8\t-10.6\n81.6\t-10.9\n81.4\t-11.2\n81.2\t-11.5\n81\t-11.8\n80.8\t-12.1\n80.6\t-12.4\n80.4\t-12.7\n80.2\t-13\n80\t-13.3\n79.8\t-13.6\n79.6\t-13.9\n79.4\t-14.2\n79.2\t-14.5\n79\t-14.8\n78.8\t-15.1\n78.6\t-15.4\n78.4\t-15.7\n78.2\t-16\n78\t-16.3\n77.8\t-16.6\n77.6\t-16.9\n77.4\t-17.2\n77.2\t-17.5\n77\t-17.8\n76.8\t-18.1\n76.6\t-18.4\n76.4\t-18.7\n76.2\t-19\n76\t-19.3\n75.8\t-19.6\n75.6\t-19.9\n75.4\t-20.2\n75.2\t-20.5\n75\t-20.8\n74.8\t-21.1\n74.6\t-21.4\n74.4\t-21.7\n74.2\t-22\n74\t-22.3\n73.8\t-22.6\n73.6\t-22.9\n73.4\t-23.2\n73.2\t-23.5\n73\t-23.8\n72.8\t-24.1\n72.6\t-24.4\n72.4\t-24.7\n72.2\t-25\n72\t-25.3\n71.8\t-25.6\n71.6\t-25.9\n71.4\t-26.2\n71.2\t-26.5\n71\t-26.8\n70.8\t-27.1\n70.6\t-27.4\n70.4\t-27.7\n70.2\t-28\n70\t-28.3\n69.8\t-28.6\n69.6\t-28.9\n69.4\t-29.2\n69.2\t-29.5\n69\t-29.8\n68.8\t-30.1\n68.6\t-30.4\n68.4\t-30.7\n68.2\t-31\n68\t-31.3\n67.8\t-31.6\n67.6\t-31.9\n67.4\t-32.2\n67.2\t-32.5\n67\t-32.8\n66.8\t-33.1\n66.6\t-33.4\n66.4\t-33.7\n66.2\t-34\n66\t-34.3\n65.8\t-34.6\n65.6\t-34.9\n65.4\t-35.2\n65.2\t-35.5\n65\t-35.8\n64.8\t-36.1\n64.6\t-36.4\n64.4\t-36.7\n64.2\t-37\n64\t-37.3\n63.8\t-37.6\n63.6\t-37.9\n63.4\t-38.2\n63.2\t-38.5\n63\t-38.8\n62.8\t-39.1\n62.6\t-39.4\n62.4\t-39.7\n62.2\t-40\n62\t-40.3\n61.8\t-40.6\n61.6\t-40.9\n61.4\t-41.2\n61.2\t-41.5\n61\t-41.8\n60.8\t-42.1\n60.6\t-42.4\n60.4\t-42.7\n60.2\t-43\n60\t-43.3\n59.8\t-43.6\n59.6\t-43.9\n59.4\t-44.2\n59.2\t-44.5\n59\t-44.8\n58.8\t-45.1\n58.6\t-45.4\n58.4\t-45.7\n58.2\t-46\n58\t-46.3\n57.8\t-46.6\n57.6\t-46.9\n57.4\t-47.2\n57.2\t-47.5\n57\t-47.8\n56.8\t-48.1\n56.6\t-48.4\n56.4\t-48.7\n56.2\t-49\n56\t-49.3\n55.8\t-49.6\n55.6\t-49.9\n55.4\t-50.2\n55.2\t-50.5\n55\t-50.8\n54.8\t-51.1\n54.6\t-51.4\n54.4\t-51.7\n54.2\t-52\n54\t-52.3\n53.8\t-52.6\n53.6\t-52.9\n53.4\t-53.2\n53.2\t-53.5\n53\t-53.8\n52.8\t-54.1\n52.6\t-54.4\n52.4\t-54.7\n52.2\t-55\n52\t-55.3\n51.8\t-55.6\n51.6\t-55.9\n51.4\t-56.2\n51.2\t-56.5\n51\t-56.8\n50.8\t-57.1\n50.6\t-57.4\n50.4\t-57.7\n50.2\t-58\n50\t-58.3\n49.8\t-58.6\n49.6\t-58.9\n49.4\t-59.2\n49.2\t-59.5\n49\t-59.8\n48.8\t-60.1\n48.6\t-60.4\n48.4\t-60.7\n48.2\t-61\n48\t-61.3\n47.8\t-61.6\n47.6\t-61.9\n47.4\t-62.2\n47.2\t-62.5\n47\t-62.8\n46.8\t-63.1\n46.6\t-63.4\n46.4\t-63.7\n46.2\t-64\n46\t-64.3\n45.8\t-64.6\n45.6\t-64.9\n45.4\t-65.2\n45.2\t-65.5\n45\t-65.8\n44.8\t-66.1\n44.6\t-66.4\n44.4\t-65.8\n44.2\t-65.2\n44\t-64.6\n43.8\t-64\n43.6\t-63.4\n43.4\t-62.8\n43.2\t-62.2\n43\t-61.6\n42.8\t-61\n42.6\t-60.4\n42.4\t-59.8\n42.2\t-59.2\n42\t-58.6\n41.8\t-58\n41.6\t-57.4\n41.4\t-56.8\n41.2\t-56.2\n41\t-55.6\n40.8\t-55\n40.6\t-54.4\n40.4\t-53.8\n40.2\t-53.2\n40\t-52.6\n39.8\t-52\n39.6\t-51.4\n39.4\t-50.8\n39.2\t-50.2\n39\t-49.6\n38.8\t-49\n38.6\t-48.4\n38.4\t-47.8\n38.2\t-47.2\n38\t-46.6\n37.8\t-46\n37.6\t-45.4\n37.4\t-44.8\n37.2\t-44.2\n37\t-43.6\n36.8\t-43\n36.6\t-42.4\n36.4\t-41.8\n36.2\t-41.2\n36\t-40.6\n35.8\t-40\n35.6\t-39.4\n35.4\t-38.8\n35.2\t-38.2\n35\t-37.6\n34.8\t-37\n34.6\t-36.4\n34.4\t-35.8\n34.2\t-35.2\n34\t-34.6\n33.8\t-34\n33.6\t-33.4\n33.4\t-32.8\n33.2\t-32.2\n33\t-31.6\n32.8\t-31\n32.6\t-30.4\n32.4\t-29.8\n32.2\t-29.2\n32\t-28.6\n31.8\t-28\n31.6\t-27.4\n31.4\t-26.8\n31.2\t-26.2\n31\t-25.6\n30.8\t-25\n30.6\t-24.4\n30.4\t-23.8\n30.2\t-23.2\n30\t-22.6\n29.8\t-22\n29.6\t-21.4\n29.4\t-20.8\n29.2\t-20.2\n29\t-19.6\n28.8\t-19\n28.6\t-18.4\n28.4\t-17.8\n28.2\t-17.2\n28\t-16.6\n27.8\t-16\n27.6\t-15.4\n27.4\t-14.8\n27.2\t-14.2\n27\t-13.6\n26.8\t-13\n26.6\t-12.4\n26.4\t-11.8\n26.2\t-11.2\n26\t-10.6\n25.8\t-10\n25.6\t-9.4\n25.4\t-8.8\n25.2\t-8.2\n25\t-7.6\n24.8\t-7\n24.6\t-6.4\n24.4\t-5.8\n24.2\t-5.2\n24\t-4.6\n23.8\t-4\n23.6\t-3.4\n23.4\t-2.8\n23.2\t-2.2\n23\t-1.6\n22.8\t-1\n22.6\t-0.4\n22.4\t0.2\n22.2\t0.8\n22\t1.4\n21.8\t2\n21.6\t2.6\n21.4\t3.2\n21.2\t3.8\n21\t4.4\n20.8\t5\n20.6\t5.6\n20.4\t6.2\n20.2\t6.8\n20\t7.4\n19.8\t8\n19.6\t8.6\n19.4\t9.2\n19.2\t9.8\n19\t10.4\n18.8\t11\n18.6\t11.6\n18.4\t12.2\n18.2\t12.8\n18\t13.4\n17.8\t14\n17.6\t14.6\n17.4\t15.2\n17.2\t15.8\n17\t16.4\n16.8\t17\n16.6\t17.6\n16.4\t18.2\n16.2\t18.8\n16\t19.4\n15.8\t20\n15.6\t20.6\n15.4\t21.2\n15.2\t21.8\n15\t22.4\n14.8\t23\n14.6\t23.6\n14.4\t24.2\n14.2\t24.8\n14\t25.4\n13.8\t26\n13.6\t26.6\n13.4\t27.2\n13.2\t27.8\n13\t28.4\n12.8\t29\n12.6\t29.6\n12.4\t30.2\n12.2\t30.8\n12\t31.4\n11.8\t32\n11.6\t32.6\n11.4\t33.2\n11.2\t33.8\n11\t34.4\n10.8\t35\n10.6\t35.6\n10.4\t36.2\n10.2\t36.8\n10\t37.4\n9.8\t38\n9.6\t38.6\n9.4\t39.2\n9.2\t39.8\n9\t40.4\n8.8\t40.1\n8.6\t39.8\n8.4\t39.5\n8.2\t39.2\n8\t38.9\n7.8\t38.6\n7.6\t38.3\n7.4\t38\n7.2\t37.7\n7\t37.4\n6.8\t37.1\n6.6\t36.8\n6.4\t36.5\n6.2\t36.2\n6\t35.9\n5.8\t35.6\n5.6\t35.3\n5.4\t35\n5.2\t34.7\n5\t34.4\n4.8\t34.1\n4.6\t33.8\n4.4\t33.5\n4.2\t33.2\n4\t32.9\n3.8\t32.6\n3.6\t32.3\n3.4\t32\n3.2\t31.7\n3\t31.4\n2.8\t31.1\n2.6\t30.8\n2.4\t30.5\n2.2\t30.2\n2\t29.9\n1.8\t29.6\n1.6\t29.3\n1.4\t29\n1.2\t28.7\n1\t28.4\n0.8\t28.1\n0.6\t27.8\n0.4\t27.5\n0.2\t27.2\n-1.30956E-12\t26.9\n-0.2\t26.6\n-0.4\t26.3\n-0.6\t26\n-0.8\t25.7\n-1\t25.4\n-1.2\t25.1\n-1.8\t24.8\n-2.4\t24.5\n-3\t24.2\n-3.6\t23.9\n-4.2\t23.6\n-4.8\t23.3\n-5.4\t23\n-6\t22.7\n-6.6\t22.4\n-7.2\t22.1\n-7.8\t21.8\n-8.4\t21.5\n-9\t21.2\n-9.6\t20.9\n-10.2\t20.6\n-10.8\t20.3\n-11.4\t20\n-12\t19.7\n-12.6\t19.4\n-13.2\t19.1\n-13.8\t18.8\n-14.4\t18.5\n-15\t18.2\n-15.6\t17.9\n-16.2\t17.6\n-16.8\t17.3\n-17.4\t17\n-18\t16.7\n-18.6\t16.4\n-19.2\t16.1\n-19.8\t15.8\n-20.4\t15.5\n-21\t15.2\n-21.6\t14.9\n-22.2\t14.6\n-22.8\t14.3\n-23.4\t14\n-24\t13.7\n-24.6\t13.4\n-25.2\t13.1\n-25.8\t12.8\n-26.4\t12.5\n-27\t12.2\n-27.6\t11.9\n-28.2\t11.6\n-28.8\t11.3\n-29.4\t11\n-30\t10.7\n-30.6\t10.4\n-31.2\t10.1\n-31.8\t9.8\n-32.4\t9.5\n-33\t9.2\n-33.6\t8.9\n-34.2\t8.6\n-34.8\t8.3\n-35.4\t8\n-36\t7.7\n-36.6\t7.4\n-37.2\t7.1\n-37.8\t6.8\n-38.4\t6.5\n-39\t6.2\n-39.6\t5.9\n-40.2\t5.6\n-40.8\t5.3\n-41.4\t5\n-42\t4.7\n-42.6\t4.4\n-43.2\t4.1\n-43.8\t3.8\n-44.4\t3.5\n-45\t3.2\n-45.6\t2.9\n-46.2\t2.6\n-46.8\t2.3\n-47.4\t2\n-48\t1.7\n-48.6\t1.4\n-49.2\t1.1\n-49.8\t0.8\n-50.4\t0.5\n-51\t0.2\n-51.6\t-0.1\n-52.2\t-0.4\n-52.8\t-0.7\n-53.4\t-1\n-54\t-1.3\n-54.6\t-1.6\n-55.2\t-1.9\n-55.8\t-2.2\n-56.4\t-2.5\n-57\t-2.8\n-57.6\t-3.1\n-58.2\t-3.4\n-58.8\t-3.7\n-59.4\t-4\n-60\t-4.3\n-60.6\t-4.6\n-61.2\t-4.9\n-61.8\t-5.2\n-62.4\t-5.5\n-63\t-5.8\n-63.6\t-6.1\n-64.2\t-6.4\n-64.8\t-6.7\n-65.4\t-7\n-66\t-7.3\n-66.6\t-7.6\n-67.2\t-7.9\n-67.8\t-8.2\n-68.4\t-8.5\n-69\t-8.8\n-69.6\t-9.1\n-70.2\t-9.4\n-70.8\t-9.7\n-71.4\t-10\n-72\t-10.3\n-72.6\t-10.6\n-73.2\t-10.9\n-73.8\t-11.2\n-74.4\t-11.5\n-75\t-11.8\n-75.6\t-12.1\n-76.2\t-12.4\n-76.8\t-12.7\n-77.4\t-13\n-78\t-13.3\n-78.6\t-13.6\n-79.2\t-13.9\n-79.8\t-14.2\n-80.4\t-14.5\n-81\t-14.8\n-81.6\t-15.1\n-82.2\t-15.4\n-82.8\t-15.7\n-83.4\t-16\n-84\t-16.3\n-84.6\t-16.6\n-85.2\t-16.9\n-85.8\t-17.2\n-86.4\t-17.5\n-87\t-17.8\n-87.6\t-18.1\n-88.2\t-18.4\n-88.8\t-18.7\n-89.4\t-19\n-90\t-19.3\n-90.6\t-19.6\n-91.2\t-19.9\n-91\t-20.2\n-90.8\t-20.5\n-90.6\t-20.8\n-90.4\t-21.1\n-90.2\t-21.4\n-90\t-21.7\n-89.8\t-22\n-89.6\t-22.3\n-89.4\t-22.6\n-89.2\t-22.9\n-89\t-23.2\n-88.8\t-23.5\n-88.6\t-23.8\n-88.4\t-24.1\n-88.2\t-24.4\n-88\t-24.7\n-87.8\t-25\n-87.6\t-25.3\n-87.4\t-25.6\n-87.2\t-25.9\n-87\t-26.2\n-86.8\t-26.5\n-86.6\t-26.8\n-86.4\t-27.1\n-86.2\t-27.4\n-86\t-27.7\n-85.8\t-28\n-85.6\t-28.3\n-85.4\t-28.6\n-85.2\t-28.9\n-85\t-29.2\n-84.8\t-29.5\n-84.6\t-29.8\n-84.4\t-30.1\n-84.2\t-30.4\n-84\t-30.7\n-83.8\t-31\n-83.6\t-31.3\n-83.4\t-31.6\n-83.2\t-31.9\n-83\t-32.2\n-82.8\t-32.5\n-82.6\t-32.8\n-82.4\t-33.1\n-82.2\t-33.4\n-82\t-33.7\n-81.8\t-34\n-81.6\t-34.3\n-81.4\t-34.6\n-81.2\t-34.9\n-81\t-35.2\n-80.8\t-35.5\n-80.6\t-35.8\n-80.4\t-36.1\n-80.2\t-36.4\n-80\t-36.7\n-79.8\t-37\n-79.6\t-37.3\n-79.4\t-37.6\n-79.2\t-37.9\n-79\t-38.2\n-78.8\t-38.5\n-78.6\t-38.8\n-78.4\t-39.1\n-78.2\t-39.4\n-78\t-39.7\n-77.8\t-40\n-77.6\t-40.3\n-77.4\t-40.6\n-77.2\t-40.9\n-77\t-41.2\n-76.8\t-41.5\n-76.6\t-41.8\n-76.4\t-42.1\n-76.2\t-42.4\n-76\t-42.7\n-75.8\t-43\n-75.6\t-43.3\n-75.4\t-43.6\n-75.2\t-43.9\n-75\t-44.2\n-74.8\t-44.5\n-74.6\t-44.8\n-74.4\t-45.1\n-74.2\t-45.4\n-74\t-45.7\n-73.8\t-46\n-73.6\t-46.3\n-73.4\t-46.6\n-73.2\t-46.9\n-73\t-47.2\n-72.8\t-47.5\n-72.6\t-47.8\n-72.4\t-48.1\n-72.2\t-48.4\n-72\t-48.7\n-71.8\t-49\n-71.6\t-49.3\n-71.4\t-49.6\n-71.2\t-49.9\n-71\t-50.2\n-70.8\t-50.5\n-70.6\t-50.8\n-70.4\t-51.1\n-70.2\t-51.4\n-70\t-51.7\n-69.8\t-52\n-69.6\t-52.3\n-69.4\t-52.6\n-69.2\t-52.9\n-69\t-53.2\n-68.8\t-53.5\n-68.6\t-53.8\n-68.4\t-54.1\n-68.2\t-54.4\n-68\t-54.7\n-67.8\t-55\n-67.6\t-55.3\n-67.4\t-55.6\n-67.2\t-55.9\n-67\t-56.2\n-66.8\t-56.5\n-66.6\t-56.8\n-66.4\t-57.1\n-66.2\t-57.4\n-66\t-57.7\n-65.8\t-58\n-65.6\t-58.3\n-65.4\t-58.6\n-65.2\t-58.9\n-65\t-59.2\n-64.8\t-59.5\n-64.6\t-59.8\n-64.4\t-60.1\n-64.2\t-60.4\n-64\t-60.7\n-63.8\t-61\n-63.6\t-61.3\n-63.4\t-61.6\n-63.2\t-61.9\n-63\t-62.2\n-62.8\t-62.5\n-62.6\t-62.8\n-62.4\t-63.1\n-62.2\t-63.4\n-62\t-63.7\n-61.8\t-64\n-61.6\t-64.3\n-61.4\t-64.6\n-61.2\t-64.9\n-61\t-65.2\n-60.8\t-65.5\n-60.6\t-65.8\n-60.4\t-66.1\n-60.2\t-66.4\n-60\t-66.7\n-59.8\t-67\n-59.6\t-67.3\n-59.4\t-67.6\n-59.2\t-67.9\n-59\t-68.2\n-58.8\t-68.5\n-58.6\t-68.8\n-58.4\t-69.1\n-58.2\t-69.4\n-58\t-69.7\n-57.8\t-70\n-57.6\t-70.3\n-57.4\t-70.6\n-57.2\t-70.9\n-57\t-71.2\n-56.8\t-71.5\n-56.6\t-71.8\n-56.4\t-72.1\n-56.2\t-72.4\n-56\t-72.7\n-55.8\t-73\n-55.6\t-73.3\n-55.4\t-73.6\n-55.2\t-73.9\n-55\t-74.2\n-54.8\t-74.5\n-54.6\t-74.8\n-54.4\t-75.1\n-54.2\t-75.4\n-54\t-75.7\n-53.8\t-76\n-53.6\t-76.3\n-53.4\t-76.6\n-53.2\t-76.9\n-53\t-77.2\n-52.8\t-77.5\n-52.6\t-77.8\n-52.4\t-78.1\n-52.2\t-78.4\n-52\t-78.7\n-51.8\t-79\n-51.6\t-79.3\n-51.4\t-79.6\n-51.2\t-79.9\n-51\t-80.2\n-50.8\t-80.5\n-50.6\t-80.8\n-50.4\t-81.1\n-50.2\t-81.4\n-50\t-81.7\n-49.8\t-82\n-49.6\t-82.3\n-49.4\t-82.6\n-49.2\t-82.9\n-49\t-83.2\n-48.8\t-83.5\n-48.6\t-83.8\n-48.4\t-84.1\n-48.2\t-84.4\n-48\t-84.7\n-47.8\t-85\n-47.6\t-85.3\n-47.4\t-85.6\n-47.2\t-85.9\n-47\t-86.2\n-46.8\t-86.5\n-46.6\t-86.8\n-46.4\t-87.1\n-46.2\t-87.4\n-46\t-87.7\n-45.8\t-88\n-45.6\t-88.3\n-45.4\t-88.6\n-45.2\t-88.9\n-45\t-89.2\n-44.8\t-89.5\n-44.6\t-89.8\n-44.4\t-90.1\n-44.2\t-90.4\n-44\t-90.3\n-43.8\t-90.2\n-43.6\t-90.1\n-43.4\t-90\n-43.2\t-89.9\n-43\t-89.8\n-42.8\t-89.7\n-42.6\t-89.6\n-42.4\t-89.5\n-42.2\t-89.4\n-42\t-89.3\n-41.8\t-89.2\n-41.6\t-89.1\n-41.4\t-89\n-41.2\t-88.9\n-41\t-88.8\n-40.8\t-88.7\n-40.6\t-88.6\n-40.4\t-88.5\n-40.2\t-88.4\n-40\t-88.3\n-39.8\t-88.2\n-39.6\t-88.1\n-39.4\t-88\n-39.2\t-87.9\n-39\t-87.8\n-38.8\t-87.7\n-38.6\t-87.6\n-38.4\t-87.5\n-38.2\t-87.4\n-38\t-87.3\n-37.8\t-87.2\n-37.6\t-87.1\n-37.4\t-87\n-37.2\t-86.9\n-37\t-86.8\n-36.8\t-86.7\n-36.6\t-86.6\n-36.4\t-86.5\n-36.2\t-86.4\n-36\t-86.3\n-35.8\t-86.2\n-35.6\t-86.1\n-35.4\t-86\n-35.2\t-85.9\n-35\t-85.8\n-34.8\t-85.7\n-34.6\t-85.6\n-34.4\t-85.5\n-34.2\t-85.4\n-34\t-85.3\n-33.8\t-85.2\n-33.6\t-85.1\n-33.4\t-85\n-33.2\t-84.9\n-33\t-84.8\n-32.8\t-84.7\n-32.6\t-84.6\n-32.4\t-84.5\n-32.2\t-84.4\n-32\t-84.3\n-31.8\t-84.2\n-31.6\t-84.1\n-31.4\t-84\n-31.2\t-83.9\n-31\t-83.8\n-30.8\t-83.7\n-30.6\t-83.6\n-30.4\t-83.5\n-30.2\t-83.4\n-30\t-83.3\n-29.8\t-83.2\n-29.6\t-83.1\n-29.4\t-83\n-29.2\t-82.9\n-29\t-82.8\n-28.8\t-82.7\n-28.6\t-82.6\n-28.4\t-82.5\n-28.2\t-82.4\n-28\t-82.3\n-27.8\t-82.2\n-27.6\t-82.1\n-27.4\t-82\n-27.2\t-81.9\n-27\t-81.8\n-26.8\t-81.7\n-26.6\t-81.6\n-26.4\t-81.5\n-26.2\t-81.4\n-26\t-81.3\n-25.8\t-81.2\n-25.6\t-81.1\n-25.4\t-81\n-25.2\t-80.9\n-25\t-80.8\n-24.8\t-80.7\n-24.6\t-80.6\n-24.4\t-80.5\n-24.2\t-80.4\n-24\t-80.3\n-23.8\t-80.2\n-23.6\t-80.1\n-23.4\t-80\n-23.2\t-79.9\n-23\t-79.8\n-22.8\t-79.7\n-22.6\t-79.6\n-22.4\t-79.5\n-22.2\t-79.4\n-22\t-79.3\n-21.8\t-79.2\n-21.6\t-79.1\n-21.4\t-79\n-21.2\t-78.9\n-21\t-78.8\n-20.8\t-78.7\n-20.6\t-78.6\n-20.4\t-78.5\n-20.2\t-78.4\n-20\t-78.3\n-19.8\t-78.2\n-19.6\t-78.1\n-19.4\t-78\n-19.2\t-77.9\n-19\t-77.8\n-18.8\t-77.7\n-18.6\t-77.6\n-18.4\t-77.5\n-18.2\t-77.4\n-18\t-77.3\n-17.8\t-77.2\n-17.6\t-77.1\n-17.4\t-77\n-17.2\t-76.9\n-17\t-76.8\n-16.8\t-76.7\n-16.6\t-76.6\n-16.4\t-76.5\n-16.2\t-76.4\n-16\t-76.3\n-15.8\t-76.2\n-15.6\t-76.1\n-15.4\t-76\n-15.2\t-75.9\n-15\t-75.8\n-14.8\t-75.7\n-14.6\t-75.6\n-14.4\t-75.5\n-14.2\t-75.4\n-14\t-75.3\n-13.8\t-75.2\n-13.6\t-75.1\n-13.4\t-75\n-13.2\t-74.9\n-13\t-74.8\n-12.8\t-74.7\n-12.6\t-74.6\n-12.4\t-74.5\n-12.2\t-74.4\n-12\t-74.3\n-11.8\t-74.2\n-11.6\t-74.1\n-11.4\t-74\n-11.2\t-73.9\n-11\t-73.8\n-10.8\t-73.7\n-10.6\t-73.6\n-10.4\t-73.5\n-10.2\t-73.4\n-10\t-73.3\n-9.8\t-73.2\n-9.6\t-73.1\n-9.4\t-73\n-9.2\t-72.9\n-9\t-72.8\n-8.8\t-72.7\n-8.6\t-72.6\n-8.4\t-72.5\n-8.2\t-72.4\n-8\t-72.3\n-7.8\t-72.2\n-7.6\t-72.1\n-7.4\t-72\n-7.2\t-71.9\n-7\t-71.8\n-6.8\t-71.7\n-6.6\t-71.6\n-6.4\t-71.5\n-6.2\t-71.4\n-6\t-71.3\n-5.8\t-71.2\n-5.6\t-71.1\n-5.4\t-71\n-5.2\t-70.9\n-5\t-70.8\n-4.8\t-70.7\n-4.6\t-70.6\n-4.4\t-70.5\n-4.2\t-70.4\n-4\t-70.3\n-3.8\t-70.2\n-3.6\t-70.1\n-3.4\t-70\n-3.2\t-69.9\n-3\t-69.8\n-2.8\t-69.7\n-2.6\t-69.6\n-2.4\t-69.5\n-2.2\t-69.4\n-2\t-69.3\n-1.8\t-69.2\n-1.6\t-69.1\n-1.4\t-69\n-1.2\t-68.9\n-1\t-68.8\n-0.8\t-68.7\n-0.6\t-68.6\n-0.4\t-68.5\n-0.2\t-68.4\n-3.92852E-13\t-68.3\n0.2\t-68.2\n0.4\t-68.1\n0.6\t-68\n0.8\t-67.9\n1\t-67.8\n1.2\t-67.7\n1.4\t-67.6\n1.6\t-67.5\n1.8\t-67.4\n2\t-67.3\n2.2\t-67.2\n2.4\t-67.1\n2.6\t-67\n2.8\t-66.9\n3\t-66.8\n3.2\t-66.7\n3.4\t-66.6\n3.6\t-66.5\n3.8\t-66.4\n4\t-66.3\n4.2\t-66.2\n4.4\t-66.1\n4.6\t-66\n4.8\t-65.9\n5\t-65.8\n5.2\t-65.7\n5.4\t-65.6\n5.6\t-65.5\n5.8\t-65.4\n6\t-65.1\n6.2\t-64.8\n6.4\t-64.5\n6.6\t-64.2\n6.8\t-63.9\n7\t-63.6\n7.2\t-63.3\n7.4\t-63\n7.6\t-62.7\n7.8\t-62.4\n8\t-62.1\n8.2\t-61.8\n8.4\t-61.5\n8.6\t-61.2\n8.8\t-60.9\n9\t-60.6\n9.2\t-60.3\n9.4\t-60\n9.6\t-59.7\n9.8\t-59.4\n10\t-59.1\n10.2\t-58.8\n10.4\t-58.5\n10.6\t-58.2\n10.8\t-57.9\n11\t-57.6\n11.2\t-57.3\n11.4\t-57\n11.6\t-56.7\n11.8\t-56.4\n12\t-56.1\n12.2\t-55.8\n12.4\t-55.5\n12.6\t-55.2\n12.8\t-54.9\n13\t-54.6\n13.2\t-54.3\n13.4\t-54\n13.6\t-53.7\n13.8\t-53.4\n14\t-53.1\n14.2\t-52.8\n14.4\t-52.5\n14.6\t-52.2\n14.8\t-51.9\n15\t-51.6\n15.2\t-51.3\n15.4\t-51\n15.6\t-50.7\n15.8\t-50.4\n16\t-50.1\n16.2\t-49.8\n16.4\t-49.5\n16.6\t-49.2\n16.8\t-48.9\n17\t-48.6\n17.2\t-48.3\n17.4\t-48\n17.6\t-47.7\n17.8\t-47.4\n18\t-47.1\n18.2\t-46.8\n18.4\t-46.5\n18.6\t-46.2\n18.8\t-45.9\n19\t-45.6\n19.2\t-45.3\n19.4\t-45\n19.6\t-44.7\n19.8\t-44.4\n20\t-44.1\n20.2\t-43.8\n20.4\t-43.5\n20.6\t-43.2\n20.8\t-42.9\n21\t-42.6\n21.2\t-42.3\n21.4\t-42\n21.6\t-41.7\n21.8\t-41.4\n22\t-41.1\n22.2\t-40.8\n22.4\t-40.5\n22.6\t-40.2\n22.8\t-39.9\n23\t-39.6\n23.2\t-39.3\n23.4\t-39\n23.6\t-38.7\n23.8\t-38.4\n24\t-38.1\n24.2\t-37.8\n24.4\t-37.5\n24.6\t-37.2\n24.8\t-36.9\n25\t-36.6\n25.2\t-36.3\n25.4\t-36\n25.6\t-35.7\n25.8\t-35.4\n26\t-35.1\n26.2\t-34.8\n26.4\t-34.5\n26.6\t-34.2\n26.8\t-33.9\n27\t-33.6\n27.2\t-33.3\n27.4\t-33\n27.6\t-32.7\n27.8\t-32.4\n28\t-32.1\n28.2\t-31.8\n28.4\t-31.5\n28.6\t-31.2\n28.8\t-30.9\n29\t-30.6\n29.2\t-30.3\n29.4\t-30\n29.6\t-29.7\n29.8\t-29.4\n30\t-29.1\n30.2\t-28.8\n30.4\t-28.5\n30.6\t-28.2\n30.8\t-27.9\n31\t-27.6\n31.2\t-27.3\n31.4\t-27\n31.6\t-26.7\n31.8\t-26.4\n32\t-26.1\n32.2\t-25.8\n32.4\t-25.5\n32.6\t-25.2\n32.8\t-24.9\n33\t-24.6\n33.2\t-24.3\n33.4\t-24\n33.6\t-23.7\n33.8\t-23.4\n34\t-23.1\n34.2\t-22.8\n34.4\t-22.5\n34.6\t-22.2\n34.8\t-21.9\n35\t-21.6\n35.2\t-21.3\n35.4\t-21\n35.6\t-20.7\n35.8\t-20.4\n36\t-20.1\n36.2\t-19.8\n36.4\t-19.5\n36.6\t-19.2\n36.8\t-18.9\n37\t-18.6\n37.2\t-18.3\n37.4\t-18\n37.6\t-17.7\n37.8\t-17.4\n38\t-17.1\n38.2\t-16.8\n38.4\t-16.5\n38.6\t-16.2\n38.8\t-15.9\n39\t-15.6\n39.2\t-15.3\n39.4\t-15\n39.6\t-14.7\n39.8\t-14.4\n40\t-14.1\n40.2\t-13.8\n40.4\t-13.5\n40.6\t-13.2\n40.8\t-12.9\n41\t-12.6\n41.2\t-12.3\n41.4\t-12\n41.6\t-11.7\n41.8\t-11.4\n42\t-11.1\n42.2\t-10.8\n42.4\t-10.5\n42.6\t-10.2\n42.8\t-9.9\n43\t-9.6\n43.2\t-9.3\n43.4\t-9\n43.6\t-8.7\n43.8\t-8.4\n44\t-8.1\n44.2\t-7.8\n44.4\t-7.5\n44.6\t-7.2\n44.8\t-6.9\n45\t-6.6\n45.2\t-6.3\n45.4\t-6\n45.6\t-5.7\n45.8\t-5.4\n46\t-5.1\n46.2\t-4.8\n46.4\t-4.5\n46.6\t-4.2\n46.8\t-3.9\n47\t-3.6\n47.2\t-3.3\n47.4\t-3\n47.6\t-2.7\n47.8\t-2.4\n48\t-2.1\n48.2\t-1.8\n48.4\t-1.5\n48.6\t-1.2\n48.8\t-0.9\n49\t-0.6\n49.2\t-0.3\n49.4\t-1.83087E-12\n49.6\t0.3\n49.8\t0.6\n50\t0.9\n50.2\t1.2\n50.4\t1.5\n50.6\t1.8\n50.8\t2.1\n51\t2.4\n51.2\t2.7\n51.4\t3\n51.6\t3.3\n51.8\t3.6\n52\t3.9\n52.2\t4.2\n52.4\t4.5\n52.6\t4.8\n52.8\t5.1\n53\t5.4\n53.2\t5.7\n53.4\t6\n53.6\t6.3\n53.8\t6.6\n54\t6.9\n54.2\t7.2\n54.4\t7.5\n54.6\t7.8\n54.8\t8.1\n55\t8.4\n55.2\t8.7\n55.4\t9\n55.6\t9.3\n55.8\t9.6\n56\t9.9\n56.2\t10.2\n56.4\t10.5\n56.6\t10.8\n56.8\t11.1\n57\t11.4\n57.2\t11.7\n57.4\t12\n57.6\t12.3\n57.8\t12.6\n58\t12.9\n58.2\t13.2\n58.4\t13.5\n58.6\t13.8\n58.8\t14.1\n59\t14.4\n59.2\t14.7\n59.4\t15\n59.6\t15.3\n59.8\t15.6\n60\t15.9\n60.2\t16.2\n60.4\t16.5\n60.6\t16.8\n60.8\t17.1\n61\t17.4\n61.2\t17.7\n61.4\t18\n61.6\t18.3\n61.8\t18.6\n62\t18.9\n62.2\t19.2\n62.4\t19.5\n62.6\t19.8\n62.8\t20.1\n63\t20.4\n63.2\t20.7\n63.4\t21\n63.6\t21.3\n63.8\t21.6\n64\t21.9\n64.2\t22.2\n64.4\t22.5\n64.6\t22.8\n64.8\t23.1\n65\t23.4\n65.2\t23.7\n65.4\t24\n65.6\t24.3\n65.8\t24.6\n66\t24.9\n66.2\t25.2\n65.8\t25.5\n65.4\t25.8\n65\t26.1\n64.6\t26.4\n64.2\t26.7\n63.8\t27\n63.4\t27.3\n63\t27.6\n62.6\t27.9\n62.2\t28.2\n61.8\t28.5\n61.4\t28.8\n61\t29.1\n60.6\t29.4\n60.2\t29.7\n59.8\t30\n59.4\t30.3\n59\t30.6\n58.6\t30.9\n58.2\t31.2\n57.8\t31.5\n57.4\t31.8\n57\t32.1\n56.6\t32.4\n56.2\t32.7\n55.8\t33\n55.4\t33.3\n55\t33.6\n54.6\t33.9\n54.2\t34.2\n53.8\t34.5\n53.4\t34.8\n53\t35.1\n52.6\t35.4\n52.2\t35.7\n51.8\t36\n51.4\t36.3\n51\t36.6\n50.6\t36.9\n50.2\t37.2\n49.8\t37.5\n49.4\t37.8\n49\t38.1\n48.6\t38.4\n48.2\t38.7\n47.8\t39\n47.4\t39.3\n47\t39.6\n46.6\t39.9\n46.2\t40.2\n45.8\t40.5\n45.4\t40.8\n45\t41.1\n44.6\t41.4\n44.2\t41.7\n43.8\t42\n43.4\t42.3\n43\t42.6\n42.6\t42.9\n42.2\t43.2\n41.8\t43.5\n41.4\t43.8\n41\t44.1\n40.6\t44.4\n40.2\t44.7\n39.8\t45\n39.4\t45.3\n39\t45.6\n38.6\t45.9\n38.2\t46.2\n37.8\t46.5\n37.4\t46.8\n37\t47.1\n36.6\t47.4\n36.2\t47.7\n35.8\t48\n35.4\t48.3\n35\t48.6\n34.6\t48.9\n34.2\t49.2\n33.8\t49.5\n33.4\t49.8\n33\t50.1\n32.6\t50.4\n32.2\t50.7\n31.8\t51\n31.4\t51.3\n31\t51.6\n30.6\t51.9\n30.2\t52.2\n29.8\t52.5\n29.4\t52.8\n29\t53.1\n28.6\t53.4\n28.2\t53.7\n27.8\t54\n27.4\t54.3\n27\t54.6\n26.6\t54.9\n26.2\t55.2\n25.8\t55.5\n25.4\t55.8\n25\t56.1\n24.6\t56.4\n24.2\t56.7\n23.8\t57\n23.4\t57.3\n23\t57.6\n22.6\t57.9\n22.2\t58.2\n21.8\t58.5\n21.4\t58.8\n21\t59.1\n20.6\t59.4\n20.2\t59.7\n19.8\t60\n19.4\t60.3\n19\t60.6\n18.6\t60.9\n18.2\t61.2\n17.8\t61.5\n17.4\t61.8\n17\t62.1\n16.6\t62.4\n16.2\t62.7\n15.8\t63\n15.4\t63.3\n15\t63.6\n14.6\t63.9\n14.2\t64.2\n13.8\t64.5\n13.4\t64.8\n13\t65.1\n12.6\t65.4\n12.2\t65.7\n11.8\t66\n11.4\t66.3\n11\t66.6\n10.6\t66.9\n10.2\t67.2\n9.8\t67.5\n9.4\t67.8\n9\t68.1\n8.6\t68.4\n8.2\t68.7\n7.8\t69\n7.4\t69.3\n7\t69.6\n6.6\t69.9\n6.2\t70.2\n5.8\t70.5\n5.4\t70.8\n5\t71.1\n4.6\t71.4\n4.2\t71.7\n3.8\t72\n3.4\t72.3\n3\t72.6\n2.6\t72.9\n2.2\t73.2\n1.8\t73.5\n1.4\t73.8\n1\t74.1\n0.6\t74.4\n0.2\t74.7\n-0.2\t75\n-0.6\t75.3\n-1\t75.6\n-1.4\t75.9\n-1.8\t76.2\n-2.2\t76.5\n-2.6\t76.8\n-3\t77.1\n-3.4\t77.4\n-3.8\t77.7\n-4.2\t78\n-4.6\t78.3\n-5\t78.6\n-5.4\t78.9\n-5.8\t79.2\n-6.2\t79.5\n-6.6\t79.8\n-7\t80.1\n-7.4\t80.4\n-7.8\t80.7\n-8.2\t81\n-8.6\t81.3\n-9\t81.6\n-9.4\t81.9\n-9.8\t82.2\n-10.2\t82.5\n-10.6\t82.8\n-11\t83.1\n-11.4\t83.4\n-11.8\t83.7\n-12.2\t84\n-12.6\t84.3\n-13\t84.6\n-13.4\t84.9\n-13.8\t85.2\n-14.2\t85.5\n-14.6\t85.8\n-15\t86.1\n-15.4\t86.4\n-15.8\t86.7\n-16.2\t87\n-16.6\t87.3\n-17\t87.6\n-17.4\t87.9\n-17.8\t88.2\n-18.2\t88.5\n-18.6\t88.8\n-19\t89.1\n-19.4\t89.4\n-19.8\t89.7\n-20.2\t90\n-20.6\t90.3\n-21\t90.6\n-21.4\t90.9\n-21.8\t91.2\n-22.2\t91.5\n-22.6\t91.8\n-23\t92.1\n-23.4\t92.4\n-23.8\t92.7\n-24.2\t93\n-24.6\t93.3\n-25\t93.6\n-25.4\t93.9\n-25.8\t93.2\n-26.2\t92.5\n-26.6\t91.8\n-27\t91.1\n-27.4\t90.4\n-27.8\t89.7\n-28.2\t89\n-28.6\t88.3\n-29\t87.6\n-29.4\t86.9\n-29.8\t86.2\n-30.2\t85.5\n-30.6\t84.8\n-31\t84.1\n-31.4\t83.4\n-31.8\t82.7\n-32.2\t82\n-32.6\t81.3\n-33\t80.6\n-33.4\t79.9\n-33.8\t79.2\n-34.2\t78.5\n-34.6\t77.8\n-35\t77.1\n-35.4\t76.4\n-35.8\t75.7\n-36.2\t75\n-36.6\t74.3\n-37\t73.6\n-37.4\t72.9\n-37.8\t72.2\n-38.2\t71.5\n-38.6\t70.8\n-39\t70.1\n-39.4\t69.4\n-39.8\t68.7\n-40.2\t68\n-40.6\t67.3\n-41\t66.6\n-41.4\t65.9\n-41.8\t65.2\n-42.2\t64.5\n-42.6\t63.8\n-43\t63.1\n-43.4\t62.4\n-43.8\t61.7\n-44.2\t61\n-44.6\t60.3\n-45\t59.6\n-45.4\t58.9\n-45.8\t58.2\n-46.2\t57.5\n-46.6\t56.8\n-47\t56.1\n-47.4\t55.4\n-47.8\t54.7\n-48.2\t54\n-48.6\t53.3\n-49\t52.6\n-49.4\t51.9\n-49.8\t51.2\n-50.2\t50.5\n-50.6\t49.8\n-51\t49.1\n-51.4\t48.4\n-51.8\t47.7\n-52.2\t47\n-52.6\t46.3\n-53\t45.6\n-53.4\t44.9\n-53.8\t44.2\n-54.2\t43.5\n-54.6\t42.8\n-55\t42.1\n-55.4\t41.4\n-54.8\t40.7\n-54.2\t40\n-53.6\t39.3\n-53\t38.6\n-52.4\t37.9\n-51.8\t37.2\n-51.2\t36.5\n-50.6\t35.8\n-50\t35.1\n-49.4\t34.4\n-48.8\t33.7\n-48.2\t33\n-47.6\t32.3\n-47\t31.6\n-46.4\t30.9\n-45.8\t30.2\n-45.2\t29.5\n-44.6\t28.8\n-44\t28.1\n-43.4\t27.4\n-42.8\t26.7\n-42.2\t26\n-41.6\t25.3\n-41\t24.6\n-40.4\t23.9\n-39.8\t23.2\n-39.2\t22.5\n-38.6\t21.8\n-38\t21.1\n-37.4\t20.4\n-36.8\t19.7\n-36.2\t19\n-35.6\t18.3\n-35\t17.6\n-34.4\t16.9\n-33.8\t16.2\n-33.2\t15.5\n-32.6\t14.8\n-32\t14.1\n-31.4\t13.4\n-30.8\t12.7\n-30.2\t12\n-29.6\t11.3\n-29\t10.6\n-28.4\t9.9\n-27.8\t9.2\n-27.2\t8.5\n-26.6\t7.8\n-26\t7.1\n-25.4\t6.4\n-24.8\t5.7\n-24.2\t5\n-23.6\t4.3\n-23\t3.6\n-22.4\t2.9\n-21.8\t2.2\n-21.2\t1.5\n-20.6\t0.8\n-20\t0.1\n-19.4\t-0.6\n-18.8\t-1.3\n-18.2\t-2\n-17.6\t-2.7\n-17\t-3.4\n-16.4\t-4.1\n-15.8\t-4.8\n-15.2\t-5.5\n-14.6\t-6.2\n-14\t-6.9\n-13.4\t-7.6\n-12.8\t-8.3\n-12.2\t-9\n-11.6\t-9.7\n-11\t-10.4\n-10.4\t-11.1\n-9.8\t-11.8\n-9.2\t-12.5\n-8.6\t-13.2\n-8\t-13.9\n-7.4\t-14.6\n-6.8\t-15.3\n-6.2\t-16\n-5.6\t-16.7\n-5\t-17.4\n-4.4\t-18.1\n-3.8\t-18.8\n-3.2\t-19.5\n-2.6\t-20.2\n-2\t-20.9\n-1.4\t-21.6\n-0.8\t-22.3\n-0.2\t-23\n0.4\t-23.7\n1\t-24.4\n1.6\t-25.1\n2.2\t-25.8\n2.8\t-26.5\n3.4\t-27.2\n4\t-27.9\n4.6\t-28.6\n5.2\t-29.3\n5.8\t-30\n6.4\t-30.7\n7\t-31.4\n7.6\t-32.1\n8.2\t-32.8\n8.8\t-33.5\n9.4\t-34.2\n10\t-34.9\n10.6\t-35.6\n11.2\t-36.3\n11.8\t-37\n12.4\t-37.7\n13\t-38.4\n13.6\t-39.1\n14.2\t-39.8\n14.8\t-40.5\n15.4\t-41.2\n16\t-41.9\n16.6\t-42.6\n17.2\t-43.3\n17.8\t-44\n18.4\t-44.7\n19\t-45.4\n19.6\t-46.1\n20.2\t-46.8\n20.8\t-47.5\n21.4\t-48.2\n22\t-48.9\n22.6\t-49.6\n23.2\t-50.3\n23.8\t-51\n24.4\t-51.7\n25\t-52.4\n25.6\t-53.1\n26.2\t-53.8\n26.8\t-54.5\n27.4\t-55.2\n28\t-55.9\n28.6\t-56.6\n29.2\t-57.3\n29.8\t-58\n30.4\t-58.7\n31\t-59.4\n31.6\t-60.1\n32.2\t-60.8\n32.8\t-61.5\n33.4\t-62.2\n34\t-62.9\n34.6\t-63.6\n35.2\t-64.3\n35.8\t-65\n36.4\t-65.7\n37\t-66.4\n37.6\t-67.1\n38.2\t-67.8\n38.8\t-68.5\n39.4\t-69.2\n40\t-69.9\n40.6\t-70.6\n41.2\t-71.3\n41.8\t-72\n42.4\t-72.7\n43\t-73.4\n43.6\t-74.1\n44.2\t-74.8\n44.8\t-75.5\n45.4\t-75\n46\t-74.5\n46.6\t-74\n47.2\t-73.5\n47.8\t-73\n48.4\t-72.5\n49\t-72\n49.6\t-71.5\n50.2\t-71\n50.8\t-70.5\n51.4\t-70\n52\t-69.5\n52.6\t-69\n53.2\t-68.5\n53.8\t-68\n54.4\t-67.5\n55\t-67\n55.6\t-66.5\n56.2\t-66\n56.8\t-65.5\n57.4\t-65\n58\t-64.5\n58.6\t-64\n59.2\t-63.5\n59.8\t-63\n60.4\t-62.5\n61\t-62\n61.6\t-61.5\n62.2\t-61\n62.8\t-60.5\n63.4\t-60\n64\t-59.5\n64.6\t-59\n65.2\t-58.5\n65.8\t-58\n66.4\t-57.5\n67\t-57\n67.6\t-56.5\n68.2\t-56\n68.8\t-55.5\n69.4\t-55\n70\t-54.5\n70.6\t-54\n71.2\t-53.5\n71.8\t-53\n72.4\t-52.5\n73\t-52\n73.6\t-51.5\n74.2\t-51\n74.8\t-50.5\n75.4\t-50\n76\t-49.5\n76.6\t-49\n77.2\t-48.5\n77.8\t-48\n78.4\t-47.5\n79\t-47\n79.6\t-46.5\n80.2\t-46\n80.8\t-45.5\n81.4\t-45\n82\t-44.5\n82.6\t-44\n83.2\t-43.5\n83.8\t-43\n84.4\t-42.5\n85\t-42\n85.6\t-41.5\n86.2\t-41\n86.8\t-40.5\n87.4\t-40\n88\t-39.5\n88.6\t-39\n89.2\t-38.5\n89.8\t-38\n90.4\t-37.5\n91\t-37\n91.6\t-36.5\n92.2\t-36\n92.8\t-35.5\n93.4\t-35\n94\t-34.5\n93.8\t-34\n93.6\t-33.5\n93.4\t-33\n93.2\t-32.5\n93\t-32\n92.8\t-31.5\n92.6\t-31\n92.4\t-30.5\n92.2\t-30\n92\t-29.5\n91.8\t-29\n91.6\t-28.5\n91.4\t-28\n91.2\t-27.5\n91\t-27\n90.8\t-26.5\n90.6\t-26\n90.4\t-25.5\n90.2\t-25\n90\t-24.5\n89.8\t-24\n89.6\t-23.5\n89.4\t-23\n89.2\t-22.5\n89\t-22\n88.8\t-21.5\n88.6\t-21\n88.4\t-20.5\n88.2\t-20\n88\t-19.5\n87.8\t-19\n87.6\t-18.5\n87.4\t-18\n87.2\t-17.5\n87\t-17\n86.8\t-16.5\n86.6\t-16\n86.4\t-15.5\n86.2\t-15\n86\t-14.5\n85.8\t-14\n85.6\t-13.5\n85.4\t-13\n85.2\t-12.5\n85\t-12\n84.8\t-11.5\n84.6\t-11\n84.4\t-10.5\n84.2\t-10\n84\t-9.5\n83.8\t-9\n83.6\t-8.5\n83.4\t-8\n83.2\t-7.5\n83\t-7\n82.8\t-6.5\n82.6\t-6\n82.4\t-5.5\n82.2\t-5\n82\t-4.5\n81.8\t-4\n81.6\t-3.5\n81.4\t-3\n81.2\t-2.5\n81\t-2\n80.8\t-1.5\n80.6\t-1\n80.4\t-0.5\n80.2\t-2.74269E-12\n80\t0.5\n79.8\t1\n79.6\t1.5\n79.4\t2\n79.2\t2.5\n79\t3\n78.8\t3.5\n78.6\t4\n78.4\t4.5\n78.2\t5\n78\t5.5\n77.8\t6\n77.6\t6.5\n77.4\t7\n77.2\t7.5\n77\t8\n76.8\t8.5\n76.6\t9\n76.4\t9.5\n76.2\t10\n76\t10.5\n75.8\t11\n75.6\t11.5\n75.4\t12\n75.2\t12.5\n75\t13\n74.8\t13.5\n74.6\t14\n74.4\t14.5\n74.2\t15\n74\t15.5\n73.8\t16\n73.6\t16.5\n73.4\t17\n73.2\t17.5\n73\t18\n72.8\t18.5\n72.6\t19\n72.4\t19.5\n72.2\t20\n72\t20.5\n71.8\t21\n71.6\t21.5\n71.4\t22\n71.2\t22.5\n71\t23\n70.8\t23.5\n70.6\t24\n70.4\t24.5\n70.2\t25\n70\t25.5\n69.8\t26\n69.6\t26.5\n69.4\t27\n69.2\t27.5\n69\t28\n68.8\t28.5\n68.6\t29\n68.4\t29.5\n68.2\t30\n68\t30.5\n67.8\t31\n67.6\t31.5\n67.4\t32\n67.2\t32.5\n67\t33\n66.8\t33.5\n66.6\t34\n66.4\t34.5\n66.2\t35\n66\t35.5\n65.8\t36\n65.6\t35.8\n65.4\t35.6\n65.2\t35.4\n65\t35.2\n64.8\t35\n64.6\t34.8\n64.4\t34.6\n64.2\t34.4\n64\t34.2\n63.8\t34\n63.6\t33.8\n63.4\t33.6\n63.2\t33.4\n63\t33.2\n62.8\t33\n62.6\t32.8\n62.4\t32.6\n62.2\t32.4\n62\t32.2\n61.8\t32\n61.6\t31.8\n61.4\t31.6\n61.2\t31.4\n61\t31.2\n60.8\t31\n60.6\t30.8\n60.4\t30.6\n60.2\t30.4\n60\t30.2\n59.8\t30\n59.6\t29.8\n59.4\t29.6\n59.2\t29.4\n59\t29.2\n58.8\t29\n58.6\t28.8\n58.4\t28.6\n58.2\t28.4\n58\t28.2\n57.8\t28\n57.6\t27.8\n57.4\t27.6\n57.2\t27.4\n57\t27.2\n56.8\t27\n56.6\t26.8\n56.4\t26.6\n56.2\t26.4\n56\t26.2\n55.8\t26\n55.6\t25.8\n55.4\t25.6\n55.2\t25.4\n55\t25.2\n54.8\t25\n54.6\t24.8\n54.4\t24.6\n54.2\t24.4\n54\t24.2\n53.8\t24\n53.6\t23.8\n53.4\t23.6\n53.2\t23.4\n53\t23.2\n52.8\t23\n52.6\t22.8\n52.4\t22.6\n52.2\t22.4\n52\t22.2\n51.8\t22\n51.6\t21.8\n51.4\t21.6\n51.2\t21.4\n51\t21.2\n50.8\t21\n50.6\t20.8\n50.4\t20.6\n50.2\t20.4\n50\t20.2\n49.8\t20\n49.6\t19.8\n49.4\t19.6\n49.2\t19.4\n49\t19.2\n48.8\t19\n48.6\t18.8\n48.4\t18.6\n48.2\t18.4\n48\t18.2\n47.8\t18\n47.6\t17.8\n47.4\t17.6\n47.2\t17.4\n47\t17.2\n46.8\t17\n46.6\t16.8\n46.4\t16.6\n46.2\t16.4\n46\t16.2\n45.8\t16\n45.6\t15.8\n45.4\t15.6\n45.2\t15.4\n45\t15.2\n44.8\t15\n44.6\t14.8\n44.4\t14.6\n44.2\t14.4\n44\t14.2\n43.8\t14\n43.6\t13.8\n43.4\t13.6\n43.2\t13.4\n43\t13.2\n42.8\t13\n42.6\t12.8\n42.4\t12.6\n42.2\t12.4\n42\t12.2\n41.8\t12\n41.6\t11.8\n41.4\t11.6\n41.2\t11.4\n41\t11.2\n40.8\t11\n40.6\t10.8\n40.4\t10.6\n40.2\t10.4\n40\t10.2\n39.8\t10\n39.6\t9.8\n39.4\t9.6\n39.2\t9.4\n39\t9.2\n38.8\t9\n38.6\t8.8\n38.4\t8.6\n38.2\t8.4\n38\t8.2\n37.8\t8\n37.6\t7.8\n37.4\t7.6\n37.2\t7.4\n37\t7.2\n36.8\t7\n36.6\t6.8\n36.4\t6.6\n36.2\t6.4\n36\t6.2\n35.8\t6\n35.6\t5.8\n35.4\t5.6\n35.2\t5.4\n35\t5.2\n34.8\t5\n34.6\t4.8\n34.4\t4.6\n34.2\t4.4\n34\t4.2\n33.8\t4\n33.6\t3.8\n33.4\t3.6\n33.2\t3.4\n33\t3.2\n32.8\t3\n32.6\t2.8\n32.4\t2.6\n32.2\t2.4\n32\t2.2\n31.8\t2\n31.6\t1.8\n31.4\t1.6\n31.2\t1.4\n31\t1.2\n30.8\t1\n30.6\t0.8\n30.4\t0.6\n30.2\t0.4\n30\t0.2\n29.8\t-2.71644E-12\n29.6\t-0.2\n29.4\t-0.4\n29.2\t-0.6\n29\t-0.8\n28.8\t-1\n28.6\t-1.2\n28.4\t-1.4\n28.2\t-1.6\n28\t-1.8\n27.8\t-2\n27.6\t-2.2\n27.4\t-2.4\n27.2\t-2.6\n27\t-2.8\n26.8\t-3\n26.6\t-3.2\n26.4\t-3.4\n26.2\t-3.6\n26\t-3.8\n25.8\t-4\n25.6\t-4.2\n25.4\t-4.4\n25.2\t-4.6\n25\t-4.8\n24.8\t-5\n24.6\t-5.2\n24.4\t-5.4\n24.2\t-5.6\n24\t-5.8\n23.8\t-6\n23.6\t-6.2\n23.4\t-6.4\n23.2\t-6.6\n23\t-6.8\n22.8\t-7\n22.6\t-7.2\n22.4\t-7.4\n22.2\t-7.6\n22\t-7.8\n21.8\t-8\n21.6\t-8.2\n21.4\t-8.4\n21.2\t-8.6\n21\t-8.8\n20.8\t-9\n20.6\t-9.2\n20.4\t-9.4\n20.2\t-9.6\n20\t-9.8\n19.8\t-10\n19.6\t-10.2\n19.4\t-10.4\n19.2\t-10.6\n19\t-10.8\n18.8\t-11\n18.6\t-11.2\n18.4\t-11.4\n18.2\t-11.6\n18\t-11.8\n17.8\t-12\n17.6\t-12.2\n17.4\t-12.4\n17.2\t-12.6\n17\t-12.8\n16.8\t-13\n16.6\t-13.2\n16.4\t-13.4\n16.2\t-13.6\n16\t-13.8\n15.8\t-14\n15.6\t-14.2\n15.4\t-14.4\n15.2\t-14.6\n15\t-14.8\n14.8\t-15\n14.6\t-15.2\n14.4\t-15.4\n14.2\t-15.6\n14\t-15.8\n13.8\t-16\n13.6\t-16.2\n13.4\t-16.4\n13.2\t-16.6\n13\t-16.8\n12.8\t-17\n12.6\t-17.2\n12.4\t-17.4\n12.2\t-17.6\n12\t-17.8\n11.8\t-18\n11.6\t-18.2\n11.4\t-18.4\n11.2\t-18.6\n11\t-18.8\n10.8\t-19\n10.6\t-19.2\n10.4\t-19.4\n10.2\t-19.6\n10\t-19.8\n9.8\t-20\n9.6\t-20.2\n9.4\t-20.4\n9.2\t-20.6\n9\t-20.8\n8.8\t-21\n8.6\t-21.2\n8.4\t-21.4\n8.2\t-21.6\n8\t-21.8\n7.8\t-22\n7.6\t-22.2\n7.4\t-22.4\n7.2\t-22.6\n7\t-22.8\n6.8\t-23\n6.6\t-23.2\n6.4\t-23.4\n6.2\t-23.6\n6\t-23.8\n5.8\t-24\n5.6\t-24.2\n5.4\t-24.4\n5.2\t-24.6\n5\t-24.8\n4.8\t-25\n4.6\t-25.2\n4.4\t-25.4\n4.2\t-25.6\n4\t-25.8\n3.8\t-26\n3.6\t-26.2\n3.4\t-26.4\n3.2\t-26.6\n3\t-26.8\n2.8\t-27\n2.6\t-27.2\n2.4\t-27.4\n2.2\t-27.6\n2\t-27.8\n1.8\t-28\n1.6\t-28.2\n1.4\t-28.4\n1.2\t-28.6\n1\t-28.8\n0.8\t-29\n0.6\t-29.2\n0.4\t-29.4\n0.2\t-29.6\n-6.27443E-13\t-29.8\n-0.2\t-30\n-0.4\t-30.2\n-0.6\t-30.4\n-0.8\t-30.6\n-1\t-30.8\n-1.2\t-31\n-1.4\t-31.2\n-1.6\t-31.4\n-2.2\t-31.6\n-2.8\t-31.8\n-3.4\t-32\n-4\t-32.2\n-4.6\t-32.4\n-5.2\t-32.6\n-5.8\t-32.8\n-6.4\t-33\n-7\t-33.2\n-7.6\t-33.4\n-8.2\t-33.6\n-8.8\t-33.8\n-9.4\t-34\n-10\t-34.2\n-10.6\t-34.4\n-11.2\t-34.6\n-11.8\t-34.8\n-12.4\t-35\n-13\t-35.2\n-13.6\t-35.4\n-14.2\t-35.6\n-14.8\t-35.8\n-15.4\t-36\n-16\t-36.2\n-16.6\t-36.4\n-17.2\t-36.6\n-17.8\t-36.8\n-18.4\t-37\n-19\t-37.2\n-19.6\t-37.4\n-20.2\t-37.6\n-20.8\t-37.8\n-21.4\t-38\n-22\t-38.2\n-22.6\t-38.4\n-23.2\t-38.6\n-23.8\t-38.8\n-24.4\t-39\n-25\t-39.2\n-25.6\t-39.4\n-26.2\t-39.6\n-26.8\t-39.8\n-27.4\t-40\n-28\t-40.2\n-28.6\t-40.4\n-29.2\t-40.6\n-29.8\t-40.8\n-30.4\t-41\n-31\t-41.2\n-31.6\t-41.4\n-32.2\t-41.6\n-32.8\t-41.8\n-33.4\t-42\n-34\t-42.2\n-34.6\t-42.4\n-35.2\t-42.6\n-35.8\t-42.8\n-36.4\t-43\n-37\t-43.2\n-37.6\t-43.4\n-38.2\t-43.6\n-38.8\t-43.8\n-39.4\t-44\n-40\t-44.2\n-40.6\t-44.4\n-41.2\t-44.6\n-41.8\t-44.8\n-42.4\t-45\n-43\t-45.2\n-43.6\t-45.4\n-44.2\t-45.6\n-44.8\t-45.8\n-45.4\t-46\n-46\t-46.2\n-46.6\t-46.4\n-47.2\t-46.6\n-47.8\t-46.8\n-48.4\t-47\n-49\t-47.2\n-49.6\t-47.4\n-50.2\t-47.6\n-50.8\t-47.8\n-51.4\t-48\n-52\t-48.2\n-52.6\t-48.4\n-53.2\t-48.6\n-53.8\t-48.8\n-54.4\t-49\n-55\t-49.2\n-55.6\t-49.4\n-56.2\t-49.6\n-56.8\t-49.8\n-57.4\t-50\n-58\t-50.2\n-58.6\t-50.4\n-59.2\t-50.6\n-59.8\t-50.8\n-60.4\t-51\n-61\t-51.2\n-61.6\t-51.4\n-62.2\t-51.6\n-62.8\t-51.8\n-63.4\t-52\n-64\t-52.2\n-64.6\t-52.4\n-65.2\t-52.6\n-65.8\t-52.8\n-66.4\t-53\n-67\t-53.2\n-67.6\t-53.4\n-68.2\t-53.6\n-68.8\t-53.8\n-69.4\t-54\n-70\t-54.2\n-70.6\t-54.4\n-71.2\t-54.6\n-71.8\t-54.8\n-72.4\t-55\n-73\t-55.2\n-73.6\t-55.4\n-74.2\t-55.6\n-74.8\t-55.8\n-75.4\t-56\n-76\t-56.2\n-76.6\t-56.4\n-77.2\t-56.6\n-77.8\t-56.8\n-78.4\t-57\n-79\t-57.2\n-79.6\t-57.4\n-80.2\t-57.6\n-80.8\t-57.8\n-81.4\t-58\n-82\t-58.2\n-82.6\t-58.4\n-83.2\t-58.6\n-83.8\t-58.8\n-84.4\t-59\n-85\t-59.2\n-85.6\t-59.4\n-86.2\t-59.6\n-86.8\t-59.8\n-87.4\t-60\n-88\t-60.2\n-88.6\t-60.4\n-89.2\t-60.6\n-89.8\t-60.8\n-90.4\t-61\n-91\t-61.2\n-91.6\t-61.4\n-91.4\t-61.6\n-91.2\t-61.8\n-91\t-62\n-90.8\t-62.2\n-90.6\t-62.4\n-90.4\t-62.6\n-90.2\t-62.8\n-90\t-63\n-89.8\t-63.2\n-89.6\t-63.4\n-89.4\t-63.6\n-89.2\t-63.8\n-89\t-64\n-88.8\t-64.2\n-88.6\t-64.4\n-88.4\t-64.6\n-88.2\t-64.8\n-88\t-65\n-87.8\t-65.2\n-87.6\t-65.4\n-87.4\t-65.6\n-87.2\t-65.8\n-87\t-66\n-86.8\t-66.2\n-86.6\t-66.4\n-86.4\t-66.6\n-86.2\t-66.8\n-86\t-67\n-85.8\t-67.2\n-85.6\t-67.4\n-85.4\t-67.6\n-85.2\t-67.8\n-85\t-68\n-84.8\t-68.2\n-84.6\t-68.4\n-84.4\t-68.6\n-84.2\t-68.8\n-84\t-69\n-83.8\t-69.2\n-83.6\t-69.4\n-83.4\t-69.6\n-83.2\t-69.8\n-83\t-70\n-82.8\t-70.2\n-82.6\t-70.4\n-82.4\t-70.6\n-82.2\t-70.8\n-82\t-71\n-81.8\t-71.2\n-81.6\t-71.4\n-81.4\t-71.6\n-81.2\t-71.8\n-81\t-72\n-80.8\t-72.2\n-80.6\t-72.4\n-80.4\t-72.6\n-80.2\t-72.8\n-80\t-73\n-79.8\t-73.2\n-79.6\t-73.4\n-79.4\t-73.6\n-79.2\t-73.8\n-79\t-74\n-78.8\t-74.2\n-78.6\t-74.4\n-78.4\t-74.6\n-78.2\t-74.8\n-78\t-75\n-77.8\t-75.2\n-77.6\t-75.4\n-77.4\t-75.6\n-77.2\t-75.8\n-77\t-76\n-76.8\t-76.2\n-76.6\t-76.4\n-76.4\t-76.6\n-76.2\t-76.8\n-76\t-77\n-75.8\t-77.2\n-75.6\t-77.4\n-75.4\t-77.6\n-75.2\t-77.8\n-75\t-78\n-74.8\t-78.2\n-74.6\t-78.4\n-74.4\t-78.6\n-74.2\t-78.8\n-74\t-79\n-73.8\t-79.2\n-73.6\t-79.4\n-73.4\t-79.6\n-73.2\t-79.8\n-73\t-80\n-72.8\t-80.2\n-72.6\t-80.4\n-72.4\t-80.6\n-72.2\t-80.8\n-72\t-81\n-71.8\t-81.2\n-71.6\t-81.4\n-71.4\t-81.6\n-71.2\t-81.8\n-71\t-82\n-70.8\t-82.2\n-70.6\t-82.4\n-70.4\t-82.6\n-70.2\t-82.8\n-70\t-83\n-69.8\t-83.2\n-69.6\t-83.4\n-69.4\t-83.6\n-69.2\t-83.8\n-69\t-84\n-68.8\t-84.2\n-68.6\t-84.4\n-68.4\t-84.6\n-68.2\t-84.8\n-68\t-85\n-67.8\t-85.2\n-67.6\t-85.4\n-67.4\t-85.6\n-67.2\t-85.8\n-67\t-86\n-66.8\t-86.2\n-66.6\t-86.4\n-66.4\t-86.6\n-66.2\t-86.8\n-66\t-87\n-65.8\t-87.2\n-65.6\t-87.4\n-65.4\t-87.6\n-65.2\t-87.8\n-65\t-88\n-64.8\t-88.2\n-64.6\t-88.4\n-64.4\t-88.6\n-64.2\t-88.8\n-64\t-89\n-63.8\t-89.2\n-63.6\t-89.4\n-63.4\t-89.6\n-63.2\t-89.8\n-63\t-90\n-62.8\t-90.2\n-62.6\t-90.4\n-62.4\t-90.6\n-62.2\t-90.8\n-62\t-91\n-61.8\t-91.2\n-61.6\t-91.4\n-61.4\t-91.6\n-61.2\t-91.8\n-61\t-92\n-60.8\t-92.2\n-60.6\t-92.4\n-60.4\t-92.6\n-60.2\t-92.8\n-60\t-93\n-59.8\t-93.2\n-59.6\t-93.4\n-59.4\t-93.6\n-59.2\t-93.8\n-59\t-94\n-58.8\t-93.6\n-58.6\t-93.2\n-58.4\t-92.8\n-58.2\t-92.4\n-58\t-92\n-57.8\t-91.6\n-57.6\t-91.2\n-57.4\t-90.8\n-57.2\t-90.4\n-57\t-90\n-56.8\t-89.6\n-56.6\t-89.2\n-56.4\t-88.8\n-56.2\t-88.4\n-56\t-88\n-55.8\t-87.6\n-55.6\t-87.2\n-55.4\t-86.8\n-55.2\t-86.4\n-55\t-86\n-54.8\t-85.6\n-54.6\t-85.2\n-54.4\t-84.8\n-54.2\t-84.4\n-54\t-84\n-53.8\t-83.6\n-53.6\t-83.2\n-53.4\t-82.8\n-53.2\t-82.4\n-53\t-82\n-52.8\t-81.6\n-52.6\t-81.2\n-52.4\t-80.8\n-52.2\t-80.4\n-52\t-80\n-51.8\t-79.6\n-51.6\t-79.2\n-51.4\t-78.8\n-51.2\t-78.4\n-51\t-78\n-50.8\t-77.6\n-50.6\t-77.2\n-50.4\t-76.8\n-50.2\t-76.4\n-50\t-76\n-49.8\t-75.6\n-49.6\t-75.2\n-49.4\t-74.8\n-49.2\t-74.4\n-49\t-74\n-48.8\t-73.6\n-48.6\t-73.2\n-48.4\t-72.8\n-48.2\t-72.4\n-48\t-72\n-47.8\t-71.6\n-47.6\t-71.2\n-47.4\t-70.8\n-47.2\t-70.4\n-47\t-70\n-46.8\t-69.6\n-46.6\t-69.2\n-46.4\t-68.8\n-46.2\t-68.4\n-46\t-68\n-45.8\t-67.6\n-45.6\t-67.2\n-45.4\t-66.8\n-45.2\t-66.4\n-45\t-66\n-44.8\t-65.6\n-44.6\t-65.2\n-44.4\t-64.8\n-44.2\t-64.4\n-44\t-64\n-43.8\t-63.6\n-43.6\t-63.2\n-43.4\t-62.8\n-43.2\t-62.4\n-43\t-62\n-42.8\t-61.6\n-42.6\t-61.2\n-42.4\t-60.8\n-42.2\t-60.4\n-42\t-60\n-41.8\t-59.6\n-41.6\t-59.2\n-41.4\t-58.8\n-41.2\t-58.4\n-41\t-58\n-40.8\t-57.6\n-40.6\t-57.2\n-40.4\t-56.8\n-40.2\t-56.4\n-40\t-56\n-39.8\t-55.6\n-39.6\t-55.2\n-39.4\t-54.8\n-39.2\t-54.4\n-39\t-54\n-38.8\t-53.6\n-38.6\t-53.2\n-38.4\t-52.8\n-38.2\t-52.4\n-38\t-52\n-37.8\t-51.6\n-37.6\t-51.2\n-37.4\t-50.8\n-37.2\t-50.4\n-37\t-50\n-36.8\t-49.6\n-36.6\t-49.2\n-36.4\t-48.8\n-36.2\t-48.4\n-36\t-48\n-35.8\t-47.6\n-35.6\t-47.2\n-35.4\t-46.8\n-35.2\t-46.4\n-35\t-46\n-34.8\t-45.6\n-34.6\t-45.2\n-34.4\t-44.8\n-34.2\t-44.4\n-34\t-44\n-33.8\t-43.6\n-33.6\t-43.2\n-33.4\t-42.8\n-33.2\t-42.4\n-33\t-42\n-32.8\t-41.6\n-32.6\t-41.2\n-32.4\t-40.8\n-32.2\t-40.4\n-32\t-40\n-31.8\t-39.6\n-31.6\t-39.2\n-31.4\t-38.8\n-31.2\t-38.4\n-31\t-38\n-30.8\t-37.6\n-30.6\t-37.2\n-30.4\t-36.8\n-30.2\t-36.4\n-30\t-36\n-29.8\t-35.6\n-29.6\t-35.2\n-29.4\t-34.8\n-29.2\t-34.4\n-29\t-34\n-28.8\t-33.6\n-28.6\t-33.2\n-28.4\t-32.8\n-28.2\t-32.4\n-28\t-32\n-27.8\t-31.6\n-27.6\t-31.2\n-27.4\t-30.8\n-27.2\t-30.4\n-27\t-30\n-26.8\t-29.6\n-26.6\t-29.2\n-26.4\t-28.8\n-26.2\t-28.4\n-26\t-28\n-25.8\t-27.6\n-25.6\t-27.2\n-25.4\t-26.8\n-25.2\t-26.4\n-25\t-26\n-24.8\t-25.6\n-24.6\t-25.2\n-24.4\t-24.8\n-24.2\t-24.4\n-24\t-24\n-23.8\t-23.6\n-23.6\t-23.2\n-23.4\t-22.8\n-23.2\t-22.4\n-23\t-22\n-22.8\t-21.6\n-22.6\t-21.2\n-22.4\t-20.8\n-22.2\t-20.4\n-22\t-20\n-21.8\t-19.6\n-21.6\t-19.2\n-21.4\t-18.8\n-21.2\t-18.4\n-21\t-18\n-20.8\t-17.6\n-20.6\t-17.2\n-20.4\t-16.8\n-20.2\t-16.4\n-20\t-16\n-19.8\t-15.6\n-19.6\t-15.2\n-19.4\t-14.8\n-19.2\t-14.4\n-19\t-14\n-18.8\t-13.6\n-18.6\t-13.2\n-18.4\t-12.8\n-18.2\t-12.4\n-18\t-12\n-17.8\t-11.6\n-17.6\t-11.2\n-17.4\t-10.8\n-17.2\t-10.4\n-17\t-10\n-16.8\t-9.6\n-16.6\t-9.2\n-16.4\t-8.8\n-16.2\t-8.4\n-16\t-8\n-15.8\t-7.6\n-15.6\t-7.2\n-15.4\t-6.8\n-15.2\t-6.4\n-15\t-6\n-14.8\t-5.6\n-14.6\t-5.2\n-14.4\t-4.8\n-14.2\t-4.4\n-14\t-4\n-13.8\t-3.6\n-13.6\t-3.2\n-13.4\t-2.8\n-13.2\t-2.4\n-13\t-2\n-12.8\t-1.6\n-12.6\t-1.2\n-12.4\t-0.8\n-12.2\t-0.4\n-12\t0\n-11.8\t0\n-11.6\t0.3\n-11.4\t0.6\n-11.2\t0.9\n-11\t1.2\n-10.8\t1.5\n-10.6\t1.8\n-10.4\t2.1\n-10.2\t2.4\n-10\t2.7\n-9.8\t3\n-9.6\t3.3\n-9.4\t3.6\n-9.2\t3.9\n-9\t4.2\n-8.8\t4.5\n-8.6\t4.8\n-8.4\t5.1\n-8.2\t5.4\n-8\t5.7\n-7.8\t6\n-7.6\t6.3\n-7.4\t6.6\n-7.2\t6.9\n-7\t7.2\n-6.8\t7.5\n-6.6\t7.8\n-6.4\t8.1\n-6.2\t8.4\n-6\t8.7\n-5.8\t9\n-5.6\t9.3\n-5.4\t9.6\n-5.2\t9.9\n-5\t10.2\n-4.8\t10.5\n-4.6\t10.8\n-4.4\t11.1\n-4.2\t11.4\n-4\t11.7\n-3.8\t12\n-3.6\t12.3\n-3.4\t12.6\n-3.2\t12.9\n-3\t13.2\n-2.8\t13.5\n-2.6\t13.8\n-2.4\t14.1\n-2.2\t14.4\n-2\t14.7\n-1.8\t15\n-1.6\t15.3\n-1.4\t15.6\n-1.2\t15.9\n-1\t16.2\n-0.8\t16.5\n-0.6\t16.8\n-0.4\t17.1\n-0.2\t17.4\n3.00593E-13\t17.7\n0.2\t18\n0.4\t18.3\n0.6\t18.6\n0.8\t18.9\n1\t19.2\n1.2\t19.5\n1.4\t19.8\n1.6\t20.1\n1.8\t20.4\n2\t20.7\n2.2\t21\n2.4\t21.3\n2.6\t21.6\n2.8\t21.9\n3\t22.2\n3.2\t22.5\n3.4\t22.8\n3.6\t23.1\n3.8\t23.4\n4\t23.7\n4.2\t24\n4.4\t24.3\n4.6\t24.6\n4.8\t24.9\n5\t25.2\n5.2\t25.5\n5.4\t25.8\n5.6\t26.1\n5.8\t26.4\n6\t26.7\n6.2\t27\n6.4\t27.3\n6.6\t27.6\n6.8\t27.9\n7\t28.2\n7.2\t28.5\n7.4\t28.8\n7.6\t29.1\n7.8\t29.4\n8\t29.7\n8.2\t30\n8.4\t30.3\n8.6\t30.6\n8.8\t30.9\n9\t31.2\n9.2\t31.5\n9.4\t31.8\n9.6\t32.1\n9.8\t32.4\n10\t32.7\n10.2\t33\n10.4\t33.3\n10.6\t33.6\n10.8\t33.9\n11\t34.2\n11.2\t34.5\n11.4\t34.8\n11.6\t35.1\n11.8\t35.4\n12\t35.7\n12.2\t36\n12.4\t36.3\n12.6\t36.6\n12.8\t36.9\n13\t37.2\n13.2\t37.5\n13.4\t37.8\n13.6\t38.1\n13.8\t38.4\n14\t38.7\n14.2\t39\n14.4\t39.3\n14.6\t39.6\n14.8\t39.9\n15\t40.2\n15.2\t40.5\n15.4\t40.8\n15.6\t41.1\n15.8\t41.4\n16\t41.7\n16.2\t42\n16.4\t42.3\n16.6\t42.6\n16.8\t42.9\n17\t43.2\n17.2\t43.5\n17.4\t43.8\n17.6\t44.1\n17.8\t44.4\n18\t44.7\n18.2\t45\n18.4\t45.3\n18.6\t45.6\n18.8\t45.9\n19\t46.2\n19.2\t46.5\n19.4\t46.8\n19.6\t47.1\n19.8\t47.4\n20\t47.7\n20.2\t48\n20.4\t48.3\n20.6\t48.6\n20.8\t48.9\n21\t49.2\n21.2\t49.5\n21.4\t49.8\n21.6\t50.1\n21.8\t50.4\n22\t50.7\n22.2\t51\n22.4\t51.3\n22.6\t51.6\n22.8\t51.9\n23\t52.2\n23.2\t52.5\n23.4\t52.8\n23.6\t53.1\n23.8\t53.4\n24\t53.7\n24.2\t54\n24.4\t54.3\n24.6\t54.6\n24.8\t54.9\n25\t55.2\n25.2\t55.5\n25.4\t55.8\n25.6\t56.1\n25.8\t56.4\n26\t56.7\n26.2\t57\n26.4\t57.3\n26.6\t57.6\n26.8\t57.9\n27\t58.2\n27.2\t58.5\n27.4\t58.8\n27.6\t59.1\n27.8\t59.4\n28\t59.7\n28.2\t60\n28.4\t60.3\n28.6\t60.6\n28.8\t60.9\n29\t61.2\n29.2\t61.5\n29.4\t61.8\n29.6\t62.1\n29.8\t62.4\n30\t62.7\n30.2\t63\n30.4\t63.3\n30.6\t63.6\n30.8\t63.9\n31\t64.2\n31.2\t64.5\n31.4\t64.8\n31.6\t65.1\n31.8\t65.4\n32\t65.7\n32.2\t66\n32.4\t66.3\n32.6\t66.6\n32.8\t66.9\n33\t67.2\n33.2\t67.5\n33.4\t67.8\n33.6\t68.1\n33.8\t68.4\n34\t68.7\n34.2\t69\n34.4\t69.3\n34.6\t69.6\n34.8\t69.9\n35\t70.2\n35.2\t70.5\n35.4\t70.8\n35.6\t71.1\n35.8\t71.4\n36\t71.7\n36.2\t72\n36.4\t72.3\n36.6\t72.6\n36.8\t72.9\n37\t73.2\n37.2\t73.5\n37.4\t73.8\n37.6\t74.1\n37.8\t74.4\n38\t74.7\n38.2\t75\n38.4\t75.3\n38.6\t75.6\n38.8\t75.9\n39\t76.2\n39.2\t76.5\n39.4\t76.8\n39.6\t77.1\n39.8\t77.4\n40\t77.7\n40.2\t78\n40.4\t78.3\n40.6\t78.6\n40.8\t78.9\n41\t79.2\n41.2\t79.5\n41.4\t79.8\n41.6\t80.1\n41.8\t80.4\n42\t80.7\n42.2\t81\n42.4\t81.3\n42.6\t81.6\n42.8\t81.9\n43\t82.2\n43.2\t82.5\n43.4\t82.8\n43.6\t83.1\n43.8\t83.4\n44\t83.7\n44.2\t84\n44.4\t84.3\n44.6\t84.6\n44.8\t84.9\n45\t85.2\n45.2\t85.5\n45.4\t85.8\n45.6\t86.1\n45.8\t86.4\n46\t86.7\n46.2\t87\n46.4\t87.3\n46.6\t87.6\n46.8\t87.9\n47\t88.2\n47.2\t88.5\n47.4\t88.8\n47.6\t89.1\n47.8\t89.4\n48\t89.7\n48.2\t90\n48.4\t90.3\n48.6\t90.6\n48.8\t90.9\n49\t91.2\n49.2\t91.5\n49.4\t91.8\n49.6\t92.1\n49.8\t92.4\n50\t92.7\n50.2\t93\n50.4\t93.3\n50.6\t93.6\n50.8\t93.9\n51\t94.2\n51.2\t94.5\n51.4\t94.8\n51.6\t95.1\n51.8\t95.4\n52\t95.7\n52.2\t96\n52.4\t96.3\n52.6\t96.6\n52.8\t96.9\n53\t97.2\n53.2\t97.5\n53.4\t97.3\n53.6\t97.1\n53.8\t96.9\n54\t96.7\n54.2\t96.5\n54.4\t96.3\n54.6\t96.1\n54.8\t95.9\n55\t95.7\n55.2\t95.5\n55.4\t95.3\n55.6\t95.1\n55.8\t94.9\n56\t94.7\n56.2\t94.5\n56.4\t94.3\n56.6\t94.1\n56.8\t93.9\n57\t93.7\n57.2\t93.5\n57.4\t93.3\n57.6\t93.1\n57.8\t92.9\n58\t92.7\n58.2\t92.5\n58.4\t92.3\n58.6\t92.1\n58.8\t91.9\n59\t91.7\n59.2\t91.5\n59.4\t91.3\n59.6\t91.1\n59.8\t90.9\n60\t90.7\n60.2\t90.5\n60.4\t90.3\n60.6\t90.1\n60.8\t89.9\n61\t89.7\n61.2\t89.5\n61.4\t89.3\n61.6\t89.1\n61.8\t88.9\n62\t88.7\n62.2\t88.5\n62.4\t88.3\n62.6\t88.1\n62.8\t87.9\n63\t87.7\n63.2\t87.5\n63.4\t87.3\n63.6\t87.1\n63.8\t86.9\n64\t86.7\n64.2\t86.5\n64.4\t86.3\n64.6\t86.1\n64.8\t85.9\n65\t85.7\n65.2\t85.5\n65.4\t85.3\n65.6\t85.1\n65.8\t84.9\n65.4\t84.7\n65\t84.5\n64.6\t84.3\n64.2\t84.1\n63.8\t83.9\n63.4\t83.7\n63\t83.5\n62.6\t83.3\n62.2\t83.1\n61.8\t82.9\n61.4\t82.7\n61\t82.5\n60.6\t82.3\n60.2\t82.1\n59.8\t81.9\n59.4\t81.7\n59\t81.5\n58.6\t81.3\n58.2\t81.1\n57.8\t80.9\n57.4\t80.7\n57\t80.5\n56.6\t80.3\n56.2\t80.1\n55.8\t79.9\n55.4\t79.7\n55\t79.5\n54.6\t79.3\n54.2\t79.1\n53.8\t78.9\n53.4\t78.7\n53\t78.5\n52.6\t78.3\n52.2\t78.1\n51.8\t77.9\n51.4\t77.7\n51\t77.5\n50.6\t77.3\n50.2\t77.1\n49.8\t76.9\n49.4\t76.7\n49\t76.5\n48.6\t76.3\n48.2\t76.1\n47.8\t75.9\n47.4\t75.7\n47\t75.5\n46.6\t75.3\n46.2\t75.1\n45.8\t74.9\n45.4\t74.7\n45\t74.5\n44.6\t74.3\n44.2\t74.1\n43.8\t73.9\n43.4\t73.7\n43\t73.5\n42.6\t73.3\n42.2\t73.1\n41.8\t72.9\n41.4\t72.7\n41\t72.5\n40.6\t72.3\n40.2\t72.1\n39.8\t71.9\n39.4\t71.7\n39\t71.5\n38.6\t71.3\n38.2\t71.1\n37.8\t70.9\n37.4\t70.7\n37\t70.5\n36.6\t70.3\n36.2\t70.1\n35.8\t69.9\n35.4\t69.7\n35\t69.5\n34.6\t69.3\n34.2\t69.1\n33.8\t68.9\n33.4\t68.7\n33\t68.5\n32.6\t68.3\n32.2\t68.1\n31.8\t67.9\n31.4\t67.7\n31\t67.5\n30.6\t67.3\n30.2\t67.1\n29.8\t66.9\n29.4\t66.7\n29\t66.5\n28.6\t66.3\n28.2\t66.1\n27.8\t65.9\n27.4\t65.7\n27\t65.5\n26.6\t65.3\n26.2\t65.1\n25.8\t64.9\n25.4\t64.7\n25\t64.5\n24.6\t64.3\n24.2\t64.1\n23.8\t63.9\n23.4\t63.7\n23\t63.5\n22.6\t63.3\n22.2\t63.1\n21.8\t62.9\n21.4\t62.7\n21\t62.5\n20.6\t62.3\n20.2\t62.1\n19.8\t61.9\n19.4\t61.7\n19\t61.5\n18.6\t61.3\n18.2\t61.1\n17.8\t60.9\n17.4\t60.7\n17\t60.5\n16.6\t60.3\n16.2\t60.1\n15.8\t59.9\n15.4\t59.7\n15\t59.5\n14.6\t59.3\n14.2\t59.1\n13.8\t58.9\n13.4\t58.7\n13\t58.5\n12.6\t58.3\n12.2\t58.1\n11.8\t57.9\n11.4\t57.7\n11\t57.5\n10.6\t57.3\n10.2\t57.1\n9.8\t56.9\n9.4\t56.7\n9\t56.5\n8.6\t56.3\n8.2\t56.1\n7.8\t55.9\n7.4\t55.7\n7\t55.5\n6.6\t55.3\n6.2\t55.1\n5.8\t54.9\n5.4\t54.7\n5\t54.5\n4.6\t54.3\n4.2\t54.1\n3.8\t53.9\n3.4\t53.7\n3\t53.5\n2.6\t53.3\n2.2\t53.1\n1.8\t52.9\n1.4\t52.7\n1\t52.5\n0.6\t52.3\n0.2\t52.1\n-0.2\t51.9\n-0.6\t51.7\n-1\t51.5\n-1.4\t51.3\n-1.8\t51.1\n-2.2\t50.9\n-2.6\t50.7\n-3\t50.5\n-3.4\t50.3\n-3.8\t50.1\n-4.2\t49.9\n-4.6\t49.7\n-5\t49.5\n-5.4\t49.3\n-5.8\t49.1\n-6.2\t48.9\n-6.6\t48.7\n-7\t48.5\n-7.4\t48.3\n-7.8\t48.1\n-8.2\t47.9\n-8.6\t47.7\n-9\t47.5\n-9.4\t47.3\n-9.8\t47.1\n-10.2\t46.9\n-10.6\t46.7\n-11\t46.5\n-11.4\t46.3\n-11.8\t46.1\n-12.2\t45.9\n-12.6\t45.7\n-13\t45.5\n-13.4\t45.3\n-13.8\t45.1\n-14.2\t44.9\n-14.6\t44.7\n-15\t44.5\n-15.4\t44.3\n-15.8\t44.1\n-16.2\t43.9\n-16.6\t43.7\n-17\t43.5\n-17.4\t43.3\n-17.8\t43.1\n-18.2\t42.9\n-18.6\t42.7\n-19\t42.5\n-19.4\t42.3\n-19.8\t42.1\n-20.2\t41.9\n-20.6\t41.7\n-21\t41.5\n-21.4\t41.3\n-21.8\t41.1\n-22.2\t40.9\n-22.6\t40.7\n-23\t40.5\n-23.4\t40.3\n-23.8\t40.1\n-24.2\t39.9\n-24.6\t39.7\n-25\t39.5\n-25.4\t39.3\n-25.8\t39.1\n-26.2\t38.9\n-26.6\t38.7\n-27\t38.5\n-27.4\t38.3\n-27.8\t38.1\n-28.2\t37.9\n-28.6\t37.7\n-29\t37.5\n-29.4\t37.3\n-29.8\t37.1\n-30.2\t36.9\n-30.6\t36.7\n-31\t36.5\n-31.4\t36.3\n-31.8\t36.1\n-32.2\t35.9\n-32.6\t35.7\n-33\t35.5\n-33.4\t35.3\n-33.8\t35.1\n-34.2\t34.9\n-34.6\t34.7\n-35\t34.5\n-35.4\t34.3\n-35.8\t34.1\n-36.2\t33.9\n-36.6\t33.7\n-37\t33.5\n-37.4\t33.3\n-37.8\t33.1\n-38.2\t32.9\n-38.6\t32.7\n-39\t32.5\n-39.4\t32.3\n-39.8\t32.1\n-40.2\t31.9\n-40.6\t31.7\n-41\t31.5\n-41.4\t31.3\n-41.8\t31.1\n-42.2\t30.9\n-42.6\t30.7\n-43\t30.5\n-43.4\t30.3\n-43.8\t30.1\n-44.2\t29.9\n-44.6\t29.7\n-45\t29.5\n-45.4\t29.3\n-45.8\t29.1\n-46.2\t28.9\n-46.6\t28.7\n-47\t28.5\n-47.4\t28.3\n-47.8\t28.1\n-48.2\t27.9\n-48.6\t27.7\n-49\t27.5\n-49.4\t27.3\n-49.8\t27.1\n-50.2\t26.9\n-50.6\t26.7\n-51\t26.5\n-51.4\t26.3\n-51.8\t26.1\n-52.2\t25.9\n-52.6\t25.7\n-53\t25.5\n-53.4\t25.3\n-53.8\t25.1\n-54.2\t24.9\n-54.6\t24.7\n-55\t24.5\n-55.4\t24.3\n-55.8\t24.1\n-55.2\t23.9\n-54.6\t23.7\n-54\t23.5\n-53.4\t23.3\n-52.8\t23.1\n-52.2\t22.9\n-51.6\t22.7\n-51\t22.5\n-50.4\t22.3\n-49.8\t22.1\n-49.2\t21.9\n-48.6\t21.7\n-48\t21.5\n-47.4\t21.3\n-46.8\t21.1\n-46.2\t20.9\n-45.6\t20.7\n-45\t20.5\n-44.4\t20.3\n-43.8\t20.1\n-43.2\t19.9\n-42.6\t19.7\n-42\t19.5\n-41.4\t19.3\n-40.8\t19.1\n-40.2\t18.9\n-39.6\t18.7\n-39\t18.5\n-38.4\t18.3\n-37.8\t18.1\n-37.2\t17.9\n-36.6\t17.7\n-36\t17.5\n-35.4\t17.3\n-34.8\t17.1\n-34.2\t16.9\n-33.6\t16.7\n-33\t16.5\n-32.4\t16.3\n-31.8\t16.1\n-31.2\t15.9\n-30.6\t15.7\n-30\t15.5\n-29.4\t15.3\n-28.8\t15.1\n-28.2\t14.9\n-27.6\t14.7\n-27\t14.5\n-26.4\t14.3\n-25.8\t14.1\n-25.2\t13.9\n-24.6\t13.7\n-24\t13.5\n-23.4\t13.3\n-22.8\t13.1\n-22.2\t12.9\n-21.6\t12.7\n-21\t12.5\n-20.4\t12.3\n-19.8\t12.1\n-19.2\t11.9\n-18.6\t11.7\n-18\t11.5\n-17.4\t11.3\n-16.8\t11.1\n-16.2\t10.9\n-15.6\t10.7\n-15\t11.3\n-14.4\t11.9\n-13.8\t12.5\n-13.2\t13.1\n-12.6\t13.7\n-12\t14.3\n-11.4\t14.9\n-10.8\t15.5\n-10.2\t16.1\n-9.6\t16.7\n-9\t17.3\n-8.4\t17.9\n-7.8\t18.5\n-7.2\t19.1\n-6.6\t19.7\n-6\t20.3\n-5.4\t20.9\n-4.8\t21.5\n-4.2\t22.1\n-3.6\t22.7\n-3\t23.3\n-2.4\t23.9\n-1.8\t24.5\n-1.2\t25.1\n-0.6\t25.7\n1.04916E-12\t26.3\n0.6\t26.9\n1.2\t27.5\n1.8\t28.1\n2.4\t28.7\n3\t29.3\n3.6\t29.9\n4.2\t30.5\n4.8\t31.1\n5.4\t31.7\n6\t32.3\n6.6\t32.9\n7.2\t33.5\n7.8\t34.1\n8.4\t34.7\n9\t35.3\n9.6\t35.9\n10.2\t36.5\n10.8\t37.1\n11.4\t37.7\n12\t38.3\n12.6\t38.9\n13.2\t39.5\n13.8\t40.1\n14.4\t40.7\n15\t41.3\n15.6\t41.9\n16.2\t42.5\n16.8\t43.1\n17.4\t43.7\n18\t44.3\n18.6\t44.9\n19.2\t45.5\n19.8\t46.1\n20.4\t46.7\n21\t47.3\n21.6\t47.9\n22.2\t48.5\n22.8\t49.1\n23.4\t49.7\n24\t50.3\n24.6\t50.9\n25.2\t51.5\n25.8\t52.1\n26.4\t52.7\n27\t53.3\n27.6\t53.9\n28.2\t54.5\n28.8\t55.1\n29.4\t55.7\n30\t56.3\n30.6\t56.9\n31.2\t57.5\n31.8\t58.1\n32.4\t58.7\n33\t59.3\n33.6\t59.9\n34.2\t60.5\n34.8\t61.1\n35.4\t61.7\n36\t62.3\n36.6\t62.9\n37.2\t63.5\n37.8\t64.1\n38.4\t64.7\n39\t65.3\n39.6\t65.9\n40.2\t66.5\n40.8\t67.1\n41.4\t67.7\n42\t68.3\n42.6\t68.9\n43.2\t69.5\n43.8\t70.1\n44.4\t70.7\n45\t71.3\n45.6\t71.9\n46.2\t72.5\n46.8\t73.1\n47.4\t73.7\n48\t74.3\n48.6\t74.9\n49.2\t75.5\n49.8\t76.1\n50.4\t76.7\n51\t77.3\n51.6\t77.9\n52.2\t78.5\n52.8\t79.1\n53.4\t79.7\n54\t80.3\n54.6\t80.9\n55.2\t81.5\n55.8\t82.1\n56.4\t82.7\n57\t83.3\n57.6\t83.9\n58.2\t84.5\n58.8\t85.1\n59.4\t85.7\n60\t86.3\n60.6\t86.9\n61.2\t87.5\n61.8\t88.1\n62.4\t88.7\n63\t89.3\n63.6\t89.9\n64.2\t90.5\n64.8\t91.1\n65.4\t91.7\n66\t92.3\n66.6\t92.9\n67.2\t93.5\n67.8\t94.1\n68.4\t93.8\n69\t93.5\n69.6\t93.2\n70.2\t92.9\n70.8\t92.6\n71.4\t92.3\n72\t92\n72.6\t91.7\n73.2\t91.4\n73.8\t91.1\n74.4\t90.8\n75\t90.5\n75.6\t90.2\n76.2\t89.9\n76.8\t89.6\n77.4\t89.3\n78\t89\n78.6\t88.7\n79.2\t88.4\n79.8\t88.1\n80.4\t87.8\n81\t87.5\n81.6\t87.2\n82.2\t86.9\n82.8\t86.6\n83.4\t86.3\n84\t86\n84.6\t85.7\n85.2\t85.4\n85.8\t85.1\n86.4\t84.8\n87\t84.5\n87.6\t84.2\n88.2\t83.9\n88.8\t83.6\n89.4\t83.3\n90\t83\n90.6\t82.7\n91.2\t82.4\n91.8\t82.1\n92.4\t81.8\n93\t81.5\n93.6\t81.2\n93.4\t80.9\n93.2\t80.6\n93\t80.3\n92.8\t80\n92.6\t79.7\n92.4\t79.4\n92.2\t79.1\n92\t78.8\n91.8\t78.5\n91.6\t78.2\n91.4\t77.9\n91.2\t77.6\n91\t77.3\n90.8\t77\n90.6\t76.7\n90.4\t76.4\n90.2\t76.1\n90\t75.8\n89.8\t75.5\n89.6\t75.2\n89.4\t74.9\n89.2\t74.6\n89\t74.3\n88.8\t74\n88.6\t73.7\n88.4\t73.4\n88.2\t73.1\n88\t72.8\n87.8\t72.5\n87.6\t72.2\n87.4\t71.9\n87.2\t71.6\n87\t71.3\n86.8\t71\n86.6\t70.7\n86.4\t70.4\n86.2\t70.1\n86\t69.8\n85.8\t69.5\n85.6\t69.2\n85.4\t68.9\n85.2\t68.6\n85\t68.3\n84.8\t68\n84.6\t67.7\n84.4\t67.4\n84.2\t67.1\n84\t66.8\n83.8\t66.5\n83.6\t66.2\n83.4\t65.9\n83.2\t65.6\n83\t65.3\n82.8\t65\n82.6\t64.7\n82.4\t64.4\n82.2\t64.1\n82\t63.8\n81.8\t63.5\n81.6\t63.2\n81.4\t62.9\n81.2\t62.6\n81\t62.3\n80.8\t62\n80.6\t61.7\n80.4\t61.4\n80.2\t61.1\n80\t60.8\n79.8\t60.5\n79.6\t60.2\n79.4\t59.9\n79.2\t59.6\n79\t59.3\n78.8\t59\n78.6\t58.7\n78.4\t58.4\n78.2\t58.1\n78\t57.8\n77.8\t57.5\n77.6\t57.2\n77.4\t56.9\n77.2\t56.6\n77\t56.3\n76.8\t56\n76.6\t55.7\n76.4\t55.4\n76.2\t55.1\n76\t54.8\n75.8\t54.5\n75.6\t54.2\n75.4\t53.9\n75.2\t53.6\n75\t53.3\n74.8\t53\n74.6\t52.7\n74.4\t52.4\n74.2\t52.1\n74\t51.8\n73.8\t51.5\n73.6\t51.2\n73.4\t50.9\n73.2\t50.6\n73\t50.3\n72.8\t50\n72.6\t49.7\n72.4\t49.4\n72.2\t49.1\n72\t48.8\n71.8\t48.5\n71.6\t48.2\n71.4\t47.9\n71.2\t47.6\n71\t47.3\n70.8\t47\n70.6\t46.7\n70.4\t46.4\n70.2\t46.1\n70\t45.8\n69.8\t45.5\n69.6\t45.2\n69.4\t44.9\n69.2\t44.6\n69\t44.3\n68.8\t44\n68.6\t43.7\n68.4\t43.4\n68.2\t43.1\n68\t42.8\n67.8\t42.5\n67.6\t42.2\n67.4\t41.9\n67.2\t41.6\n67\t41.3\n66.8\t41\n66.6\t40.7\n66.4\t40.4\n66.2\t40.1\n66\t39.8\n65.8\t39.5\n65.6\t39.2\n65.4\t38.9\n65.2\t38.6\n65\t38.3\n64.8\t38\n64.6\t37.7\n64.4\t37.4\n64.2\t37.1\n64\t36.8\n63.8\t36.5\n63.6\t36.2\n63.4\t35.9\n63.2\t35.6\n63\t35.3\n62.8\t35\n62.6\t34.7\n62.4\t34.4\n62.2\t34.1\n62\t33.8\n61.8\t33.5\n61.6\t33.2\n61.4\t32.9\n61.2\t32.6\n61\t32.3\n60.8\t32\n60.6\t31.7\n60.4\t31.4\n60.2\t31.1\n60\t30.8\n59.8\t30.5\n59.6\t30.2\n59.4\t29.9\n59.2\t29.6\n59\t29.3\n58.8\t29\n58.6\t28.7\n58.4\t28.4\n58.2\t28.1\n58\t27.8\n57.8\t27.5\n57.6\t27.2\n57.4\t26.9\n57.2\t26.6\n57\t26.3\n56.8\t26\n56.6\t25.7\n56.4\t25.4\n56.2\t25.1\n56\t24.8\n55.8\t24.5\n55.6\t24.2\n55.4\t23.9\n55.2\t23.6\n55\t23.3\n54.8\t23\n54.6\t22.7\n54.4\t22.4\n54.2\t22.1\n54\t21.8\n53.8\t21.5\n53.6\t21.2\n53.4\t20.9\n53.2\t20.6\n53\t20.3\n52.8\t20\n52.6\t19.7\n52.4\t19.4\n52.2\t19.1\n52\t18.8\n51.8\t18.5\n51.6\t18.2\n51.4\t17.9\n51.2\t17.6\n51\t17.3\n50.8\t17\n50.6\t16.7\n50.4\t16.4\n50.2\t16.1\n50\t15.8\n49.8\t15.5\n49.6\t15.2\n49.4\t14.9\n49.2\t14.6\n49\t14.3\n48.8\t14\n48.6\t13.7\n48.4\t13.4\n48.2\t13.1\n48\t12.8\n47.8\t12.5\n47.6\t12.2\n47.4\t11.9\n47.2\t11.6\n47\t11.3\n46.8\t11\n46.6\t10.7\n46.4\t10.4\n46.2\t10.1\n46\t9.8\n45.8\t9.5\n45.6\t9.2\n45.4\t8.9\n45.2\t8.6\n45\t8.3\n44.8\t8\n44.6\t7.7\n44.4\t7.4\n44.2\t7.1\n44\t6.8\n43.8\t6.5\n43.6\t6.2\n43.4\t5.9\n43.2\t5.6\n43\t5.3\n42.8\t5\n42.6\t4.7\n42.4\t4.4\n42.2\t4.1\n42\t3.8\n41.8\t3.5\n41.6\t3.2\n41.4\t2.9\n41.2\t2.6\n41\t2.3\n40.8\t2\n40.6\t1.7\n40.4\t1.4\n40.2\t1.1\n40\t0.8\n39.8\t0.5\n39.6\t0.2\n39.4\t-0.1\n39.2\t-0.4\n39\t-0.7\n38.8\t-1\n38.6\t-1.3\n38.4\t-1.6\n38.2\t-1.9\n38\t-2.2\n37.8\t-2.5\n37.6\t-2.8\n37.4\t-3.1\n37.2\t-3.4\n37\t-3.7\n36.8\t-4\n36.6\t-4.3\n36.4\t-4.6\n36.2\t-4.9\n36\t-5.2\n35.8\t-5.5\n35.6\t-5.8\n35.4\t-6.1\n35.2\t-6.4\n35\t-6.7\n34.8\t-7\n34.6\t-7.3\n34.4\t-7.6\n34.2\t-7.9\n34\t-8.2\n33.8\t-8.5\n33.6\t-8.8\n33.4\t-9.1\n33.2\t-9.4\n33\t-9.7\n32.8\t-10\n32.6\t-10.3\n32.4\t-10.6\n32.2\t-10.9\n32\t-11.2\n31.8\t-11.5\n31.6\t-11.8\n31.4\t-12.1\n31.2\t-12.4\n31\t-12.7\n30.8\t-13\n30.6\t-13.3\n30.4\t-13.6\n30.2\t-13.9\n30\t-14.2\n29.8\t-14.5\n29.6\t-14.8\n29.4\t-15.1\n29.2\t-15.4\n29\t-15.7\n28.8\t-16\n28.6\t-16.3\n28.4\t-16.6\n28.2\t-16.9\n28\t-17.2\n27.8\t-17.5\n27.6\t-17.8\n27.4\t-18.1\n27.2\t-18.4\n27\t-18.7\n26.8\t-19\n26.6\t-19.3\n26.4\t-19.6\n26.2\t-19.9\n26\t-20.2\n25.8\t-20.5\n25.6\t-20.8\n25.4\t-21.1\n25.2\t-21.4\n25\t-21.7\n24.8\t-22\n24.6\t-22.3\n24.4\t-22.6\n24.2\t-22.9\n24\t-23.2\n23.8\t-23.5\n23.6\t-23.8\n23.4\t-24.1\n23.2\t-24.4\n23\t-24.7\n22.8\t-25\n22.6\t-25.3\n22.4\t-25.6\n22.2\t-25.9\n22\t-26.2\n21.8\t-26.5\n21.6\t-26.8\n21.4\t-27.1\n21.2\t-27.4\n21\t-27.7\n20.8\t-28\n20.6\t-28.3\n20.4\t-28.6\n20.2\t-28.9\n20\t-29.2\n19.8\t-29.5\n19.6\t-29.8\n19.4\t-30.1\n19.2\t-30.4\n19\t-30.7\n18.8\t-31\n18.6\t-31.3\n18.4\t-31.6\n18.2\t-31.9\n18\t-32.2\n17.8\t-32.5\n17.6\t-32.8\n17.4\t-33.1\n17.2\t-33.4\n17\t-33.7\n16.8\t-34\n16.6\t-34.3\n16.4\t-34.6\n16.2\t-34.9\n16\t-35.2\n15.8\t-35.5\n15.6\t-35.8\n15.4\t-36.1\n15.2\t-36.4\n15\t-36.7\n14.8\t-37\n14.6\t-37.3\n14.4\t-37.6\n14.2\t-37.9\n14\t-38.2\n13.8\t-38.5\n13.6\t-38.8\n13.4\t-39.1\n13.2\t-39.4\n13\t-39.7\n12.8\t-40\n12.6\t-40.3\n12.4\t-40.6\n12.2\t-40.9\n12\t-41.2\n11.8\t-41.5\n11.6\t-41.8\n11.4\t-42.1\n11.2\t-42.4\n11\t-42.7\n10.8\t-43\n10.6\t-43.3\n10.4\t-43.6\n10.2\t-43.9\n10\t-44.2\n9.8\t-44.5\n9.6\t-44.8\n9.4\t-45.1\n9.2\t-45.4\n9\t-45.7\n8.8\t-46\n8.6\t-46.3\n8.4\t-46.6\n8.2\t-46.9\n8\t-47.2\n7.8\t-47.5\n7.6\t-47.8\n7.4\t-48.1\n7.2\t-48.4\n7\t-48.7\n6.8\t-49\n6.6\t-49.3\n6.4\t-49.6\n6.2\t-49.9\n6\t-50.2\n5.8\t-50.5\n5.6\t-50.8\n5.4\t-51.1\n5.2\t-51.4\n5\t-51.7\n4.8\t-52\n4.6\t-52.3\n4.4\t-52.6\n4.2\t-52.9\n4\t-53.2\n3.8\t-53.5\n3.6\t-53.8\n3.4\t-54.1\n3.2\t-54.4\n3\t-54.7\n2.8\t-55\n2.6\t-55.3\n2.4\t-55.6\n2.2\t-55.9\n2\t-56.2\n1.8\t-56.5\n1.6\t-56.8\n1.4\t-57.1\n1.2\t-57.4\n1\t-57.7\n0.8\t-58\n0.6\t-58.3\n0.4\t-58.6\n0.2\t-58.9\n8.02136E-14\t-59.2\n-0.2\t-59.5\n-0.4\t-59.8\n-0.6\t-60.1\n-0.8\t-60.4\n-1\t-60.7\n-1.2\t-61\n-1.4\t-61.3\n-1.6\t-61.6\n-1.8\t-61.9\n-2\t-62.2\n-2.6\t-62.5\n-3.2\t-62.8\n-3.8\t-63.1\n-4.4\t-63.4\n-5\t-63.7\n-5.6\t-64\n-6.2\t-64.3\n-6.8\t-64.6\n-7.4\t-64.9\n-8\t-65.2\n-8.6\t-65.5\n-9.2\t-65.8\n-9.8\t-66.1\n-10.4\t-66.4\n-11\t-65.8\n-11.6\t-65.2\n-12.2\t-64.6\n-12.8\t-64\n-13.4\t-63.4\n-14\t-62.8\n-14.6\t-62.2\n-15.2\t-61.6\n-15.8\t-61\n-16.4\t-60.4\n-17\t-59.8\n-17.6\t-59.2\n-18.2\t-58.6\n-18.8\t-58\n-19.4\t-57.4\n-20\t-56.8\n-20.6\t-56.2\n-21.2\t-55.6\n-21.8\t-55\n-22.4\t-54.4\n-23\t-53.8\n-23.6\t-53.2\n-24.2\t-52.6\n-24.8\t-52\n-25.4\t-51.4\n-26\t-50.8\n-26.6\t-50.2\n-27.2\t-49.6\n-27.8\t-49\n-28.4\t-48.4\n-29\t-47.8\n-29.6\t-47.2\n-30.2\t-46.6\n-30.8\t-46\n-31.4\t-45.4\n-32\t-44.8\n-32.6\t-44.2\n-33.2\t-43.6\n-33.8\t-43\n-34.4\t-42.4\n-35\t-41.8\n-35.6\t-41.2\n-36.2\t-40.6\n-36.8\t-40\n-37.4\t-39.4\n-38\t-38.8\n-38.6\t-38.2\n-39.2\t-37.6\n-39.8\t-37\n-40.4\t-36.4\n-41\t-35.8\n-41.6\t-35.2\n-42.2\t-34.6\n-42.8\t-34\n-43.4\t-33.4\n-44\t-32.8\n-44.6\t-32.2\n-45.2\t-31.6\n-45.8\t-31\n-46.4\t-30.4\n-47\t-29.8\n-47.6\t-29.2\n-48.2\t-28.6\n-48.8\t-28\n-49.4\t-27.4\n-50\t-26.8\n-50.6\t-26.2\n-51.2\t-25.6\n-51.8\t-25\n-52.4\t-24.4\n-53\t-23.8\n-53.6\t-23.2\n-54.2\t-22.6\n-54.8\t-22\n-55.4\t-21.4\n-56\t-20.8\n-56.6\t-20.2\n-57.2\t-19.6\n-57.8\t-19\n-58.4\t-18.4\n-59\t-17.8\n-59.6\t-17.2\n-60.2\t-16.6\n-60.8\t-16\n-61.4\t-15.4\n-62\t-14.8\n-62.6\t-14.2\n-63.2\t-13.6\n-63.8\t-13\n-64.4\t-12.4\n-65\t-11.8\n-65.6\t-11.2\n-66.2\t-10.6\n-66.8\t-10\n-67.4\t-9.4\n-68\t-8.8\n-68.6\t-8.2\n-69.2\t-7.6\n-69.8\t-7\n-70.4\t-6.4\n-71\t-5.8\n-71.6\t-5.2\n-72.2\t-4.6\n-72.8\t-4\n-73.4\t-3.4\n-74\t-2.8\n-74.6\t-2.2\n-75.2\t-1.6\n-75.8\t-1\n-76.4\t-0.4\n-77\t0.2\n-77.6\t0.8\n-78.2\t1.4\n-78.8\t2\n-79.4\t2.6\n-80\t3.2\n-80.6\t3.8\n-81.2\t4.4\n-81.8\t5\n-82.4\t5.6\n-83\t6.2\n-83.6\t6.8\n-84.2\t7.4\n-84.8\t8\n-85.4\t8.6\n-86\t9.2\n-86.6\t9.8\n-87.2\t10.4\n-87.8\t11\n-88.4\t11.6\n-89\t12.2\n-89.6\t12.8\n-90.2\t13.4\n-90.8\t14\n-91.4\t14.6\n-92\t15.2\n-91.8\t15.8\n-91.6\t16.4\n-91.4\t17\n-91.2\t17.6\n-91\t18.2\n-90.8\t18.8\n-90.6\t19.4\n-90.4\t20\n-90.2\t20.6\n-90\t21.2\n-89.8\t21.8\n-89.6\t22.4\n-89.4\t23\n-89.2\t23.6\n-89\t24.2\n-88.8\t24.8\n-88.6\t25.4\n-88.4\t26\n-88.2\t26.6\n-88\t27.2\n-87.8\t27.8\n-87.6\t28.4\n-87.4\t29\n-87.2\t29.6\n-87\t30.2\n-86.8\t30.8\n-86.6\t31.4\n-86.4\t32\n-86.2\t32.6\n-86\t33.2\n-85.8\t33.8\n-85.6\t34.4\n-85.4\t35\n-85.2\t35.6\n-85\t36.2\n-84.8\t36.8\n-84.6\t37.4\n-84.4\t38\n-84.2\t38.6\n-84\t39.2\n-83.8\t39.8\n-83.6\t40.4\n-83.4\t40.1\n-83.2\t39.8\n-83\t39.5\n-82.8\t39.2\n-82.6\t38.9\n-82.4\t38.6\n-82.2\t38.3\n-82\t38\n-81.8\t37.7\n-81.6\t37.4\n-81.4\t37.1\n-81.2\t36.8\n-81\t36.5\n-80.8\t36.2\n-80.6\t35.9\n-80.4\t35.6\n-80.2\t35.3\n-80\t35\n-79.8\t34.7\n-79.6\t34.4\n-79.4\t34.1\n-79.2\t33.8\n-79\t33.5\n-78.8\t33.2\n-78.6\t32.9\n-78.4\t32.6\n-78.2\t32.3\n-78\t32\n-77.8\t31.7\n-77.6\t31.4\n-77.4\t31.1\n-77.2\t30.8\n-77\t30.5\n-76.8\t30.2\n-76.6\t29.9\n-76.4\t29.6\n-76.2\t29.3\n-76\t29\n-75.8\t28.7\n-75.6\t28.4\n-75.4\t28.1\n-75.2\t27.8\n-75\t27.5\n-74.8\t27.2\n-74.6\t26.9\n-74.4\t26.6\n-74.2\t26.3\n-74\t26\n-73.8\t25.7\n-73.6\t25.4\n-73.4\t25.1\n-73.2\t24.8\n-73\t24.5\n-72.8\t24.2\n-72.6\t23.9\n-72.4\t23.6\n-72.2\t23.3\n-72\t23\n-71.8\t22.7\n-71.6\t22.4\n-71.4\t22.1\n-71.2\t21.8\n-71\t21.5\n-70.8\t21.2\n-70.6\t20.9\n-70.4\t20.6\n-70.2\t20.3\n-70\t20\n-69.8\t19.7\n-69.6\t19.4\n-69.4\t19.1\n-69.2\t18.8\n-69\t18.5\n-68.8\t18.2\n-68.6\t17.9\n-68.4\t17.6\n-68.2\t17.3\n-68\t17\n-67.8\t16.7\n-67.6\t16.4\n-67.4\t16.1\n-67.2\t15.8\n-67\t15.5\n-66.8\t15.2\n-66.6\t14.9\n-66.4\t14.6\n-66.2\t14.3\n-66\t14\n-65.8\t13.7\n-65.6\t13.4\n-65.4\t13.1\n-65.2\t12.8\n-65\t12.5\n-64.8\t12.2\n-64.6\t11.9\n-64.4\t11.6\n-64.2\t11.3\n-64\t11\n-63.8\t10.7\n-63.6\t10.4\n-63.4\t10.1\n-63.2\t9.8\n-63\t9.5\n-62.8\t9.2\n-62.6\t8.9\n-62.4\t8.6\n-62.2\t8.3\n-62\t8\n-61.8\t7.7\n-61.6\t7.4\n-61.4\t7.1\n-61.2\t6.8\n-61\t6.5\n-60.8\t6.2\n-60.6\t5.9\n-60.4\t5.6\n-60.2\t5.3\n-60\t5\n-59.8\t4.7\n-59.6\t4.4\n-59.4\t4.1\n-59.2\t3.8\n-59\t3.5\n-58.8\t3.2\n-58.6\t2.9\n-58.4\t2.6\n-58.2\t2.3\n-58\t2\n-57.8\t1.7\n-57.6\t1.4\n-57.4\t1.1\n-57.2\t0.8\n-57\t0.5\n-56.8\t0.2\n-56.6\t-0.1\n-56.4\t-0.4\n-56.2\t-0.7\n-56\t-1\n-55.8\t-1.3\n-55.6\t-1.6\n-55.4\t-1.9\n-55.2\t-2.2\n-55\t-2.5\n-54.8\t-2.8\n-54.6\t-3.1\n-54.4\t-3.4\n-54.2\t-3.7\n-54\t-4\n-53.8\t-4.3\n-53.6\t-4.6\n-53.4\t-4.9\n-53.2\t-5.2\n-53\t-5.5\n-52.8\t-5.8\n-52.6\t-6.1\n-52.4\t-6.4\n-52.2\t-6.7\n-52\t-7\n-51.8\t-7.3\n-51.6\t-7.6\n-51.4\t-7.9\n-51.2\t-8.2\n-51\t-8.5\n-50.8\t-8.8\n-50.6\t-9.1\n-50.4\t-9.4\n-50.2\t-9.7\n-50\t-10\n-49.8\t-10.3\n-49.6\t-10.6\n-49.4\t-10.9\n-49.2\t-11.2\n-49\t-11.5\n-48.8\t-11.8\n-48.6\t-12.1\n-48.4\t-12.4\n-48.2\t-12.7\n-48\t-13\n-47.8\t-13.3\n-47.6\t-13.6\n-47.4\t-13.9\n-47.2\t-14.2\n-47\t-14.5\n-46.8\t-14.8\n-46.6\t-15.1\n-46.4\t-15.4\n-46.2\t-15.7\n-46\t-16\n-45.8\t-16.3\n-45.6\t-16.6\n-45.4\t-16.9\n-45.2\t-17.2\n-45\t-17.5\n-44.8\t-17.8\n-44.6\t-18.1\n-44.4\t-18.4\n-44.2\t-18.7\n-44\t-19\n-43.8\t-19.3\n-43.6\t-19.6\n-43.4\t-19.9\n-43.2\t-20.2\n-43\t-20.5\n-42.8\t-20.8\n-42.6\t-21.1\n-42.4\t-21.4\n-42.2\t-21.7\n-42\t-22\n-41.8\t-22.3\n-41.6\t-22.6\n-41.4\t-22.9\n-41.2\t-23.2\n-41\t-23.5\n-40.8\t-23.8\n-40.6\t-24.1\n-40.4\t-24.4\n-40.2\t-24.7\n-40\t-25\n-39.8\t-25.3\n-39.6\t-25.6\n-39.4\t-25.9\n-39.2\t-26.2\n-39\t-26.5\n-38.8\t-26.8\n-38.6\t-27.1\n-38.4\t-27.4\n-38.2\t-27.7\n-38\t-28\n-37.8\t-28.3\n-37.6\t-28.6\n-37.4\t-28.9\n-37.2\t-29.2\n-37\t-29.5\n-36.8\t-29.8\n-36.6\t-30.1\n-36.4\t-30.4\n-36.2\t-30.7\n-36\t-31\n-35.8\t-31.3\n-35.6\t-31.6\n-35.4\t-31.9\n-35.2\t-32.2\n-35\t-32.5\n-34.8\t-32.8\n-34.6\t-33.1\n-34.4\t-33.4\n-34.2\t-33.7\n-34\t-34\n-33.8\t-34.3\n-33.6\t-34.6\n-33.4\t-34.9\n-33.2\t-35.2\n-33\t-35.5\n-32.8\t-35.8\n-32.6\t-36.1\n-32.4\t-36.4\n-32.2\t-36.7\n-32\t-37\n-31.8\t-37.3\n-31.6\t-37.6\n-31.4\t-37.9\n-31.2\t-38.2\n-31\t-38.5\n-30.8\t-38.8\n-30.6\t-39.1\n-30.4\t-39.4\n-30.2\t-39.7\n-30\t-40\n-29.8\t-40.3\n-29.6\t-40.6\n-29.4\t-40.9\n-29.2\t-41.2\n-29\t-41.5\n-28.8\t-41.8\n-28.6\t-42.1\n-28.4\t-42.4\n-28.2\t-42.7\n-28\t-43\n-27.8\t-43.3\n-27.6\t-43.6\n-27.4\t-43.9\n-27.2\t-44.2\n-27\t-44.5\n-26.8\t-44.8\n-26.6\t-45.1\n-26.4\t-45.4\n-26.2\t-45.7\n-26\t-46\n-25.8\t-46.3\n-25.6\t-46.6\n-25.4\t-46.9\n-25.2\t-47.2\n-25\t-47.5\n-24.8\t-47.8\n-24.6\t-48.1\n-24.4\t-48.4\n-24.2\t-48.7\n-24\t-49\n-23.8\t-49.3\n-23.6\t-49.6\n-23.4\t-49.9\n-23.2\t-50.2\n-23\t-50.5\n-22.8\t-50.8\n-22.6\t-51.1\n-22.4\t-51.4\n-22.2\t-51.7\n-22\t-52\n-21.8\t-52.3\n-21.6\t-52.6\n-21.4\t-52.9\n-21.2\t-53.2\n-21\t-53.5\n-20.8\t-53.8\n-20.6\t-54.1\n-20.4\t-54.4\n-20.2\t-54.7\n-20\t-55\n-19.8\t-55.3\n-19.6\t-55.6\n-19.4\t-55.9\n-19.2\t-56.2\n-19\t-56.5\n-18.8\t-56.8\n-18.6\t-57.1\n-18.4\t-57.4\n-18.2\t-57.7\n-18\t-58\n-17.8\t-58.3\n-17.6\t-58.6\n-17.4\t-58.9\n-17.2\t-59.2\n-17\t-59.5\n-16.8\t-59.8\n-16.6\t-60.1\n-16.4\t-60.4\n-16.2\t-60.7\n-16\t-61\n-15.8\t-61.3\n-15.6\t-61.6\n-15.4\t-61.9\n-15.2\t-62.2\n-15\t-62.5\n-14.8\t-62.8\n-14.6\t-63.1\n-14.4\t-63.4\n-14.2\t-63.7\n-14\t-64\n-13.8\t-64.3\n-13.6\t-64.6\n-13.4\t-64.9\n-13.2\t-65.2\n-13\t-65.5\n-12.8\t-65.8\n-12.6\t-66.1\n-12.4\t-66.4\n-12.2\t-66.7\n-12\t-67\n-11.8\t-67.3\n-11.6\t-67.6\n-11.4\t-67.9\n-11.2\t-68.2\n-11\t-68.5\n-10.8\t-68.8\n-10.6\t-69.1\n-10.4\t-69.4\n-10.2\t-69.7\n-10\t-70\n-9.8\t-70.3\n-9.6\t-70.6\n-9.4\t-70.9\n-9.2\t-71.2\n-9\t-71.5\n-8.8\t-71.8\n-8.6\t-72.1\n-8.4\t-72.4\n-8.2\t-72.7\n-8\t-73\n-7.8\t-73.3\n-7.6\t-73.6\n-7.4\t-73.9\n-7.2\t-74.2\n-7\t-74.5\n-6.8\t-74.8\n-6.6\t-75.1\n-6.4\t-75.4\n-6.2\t-75.7\n-6\t-76\n-5.8\t-76.3\n-5.6\t-76.6\n-5.4\t-76.9\n-5.2\t-77.2\n-5\t-77.5\n-4.8\t-77.8\n-4.6\t-78.1\n-4.4\t-78.4\n-4.2\t-78.7\n-4\t-79\n-3.8\t-79.3\n-3.6\t-79.6\n-3.4\t-79.9\n-3.2\t-80.2\n-3\t-80.5\n-2.8\t-80.8\n-2.6\t-81.1\n-2.4\t-81.4\n-2.2\t-81.7\n-2\t-82\n-1.8\t-82.3\n-1.6\t-82.6\n-1.4\t-82.9\n-1.2\t-83.2\n-1\t-83.5\n-0.8\t-83.8\n-0.6\t-84.1\n-0.4\t-84.4\n-0.2\t-84.7\n1.01114E-12\t-85\n0.2\t-85.3\n0.4\t-85.6\n0.6\t-85.9\n0.8\t-86.2\n1\t-86.5\n1.2\t-86.8\n1.4\t-87.1\n1.6\t-87.4\n1.8\t-87.7\n2\t-88\n2.2\t-88.3\n2.4\t-88.6\n2.6\t-88.9\n2.8\t-89.2\n3\t-89.5\n3.2\t-89.8\n3.4\t-90.1\n3.6\t-90.4\n3.8\t-90.3\n4\t-90.2\n4.2\t-90.1\n4.4\t-90\n4.6\t-89.9\n4.8\t-89.8\n5\t-89.7\n5.2\t-89.6\n5.4\t-89.5\n5.6\t-89.4\n5.8\t-89.3\n6\t-89.2\n6.2\t-89.1\n6.4\t-89\n6.6\t-88.9\n6.8\t-88.8\n7\t-88.7\n7.2\t-88.6\n7.4\t-88.5\n7.6\t-88.4\n7.8\t-88.3\n8\t-88.2\n8.2\t-88.1\n8.4\t-88\n8.6\t-87.9\n8.8\t-87.8\n9\t-87.7\n9.2\t-87.6\n9.4\t-87.5\n9.6\t-87.4\n9.8\t-87.3\n10\t-87.2\n10.2\t-87.1\n10.4\t-87\n10.6\t-86.9\n10.8\t-86.8\n11\t-86.7\n11.2\t-86.6\n11.4\t-86.5\n11.6\t-86.4\n11.8\t-86.3\n12\t-86.2\n12.2\t-86.1\n12.4\t-86\n12.6\t-85.9\n12.8\t-85.8\n13\t-85.7\n13.2\t-85.6\n13.4\t-85.5\n13.6\t-85.4\n13.8\t-85.3\n14\t-85.2\n14.2\t-85.1\n14.4\t-85\n14.6\t-84.9\n14.8\t-84.8\n15\t-84.7\n15.2\t-84.6\n15.4\t-84.5\n15.6\t-84.4\n15.8\t-84.3\n16\t-84.2\n16.2\t-84.1\n16.4\t-84\n16.6\t-83.9\n16.8\t-83.8\n17\t-83.7\n17.2\t-83.6\n17.4\t-83.5\n17.6\t-83.4\n17.8\t-83.3\n18\t-83.2\n18.2\t-83.1\n18.4\t-83\n18.6\t-82.9\n18.8\t-82.8\n19\t-82.7\n19.2\t-82.6\n19.4\t-82.5\n19.6\t-82.4\n19.8\t-82.3\n20\t-82.2\n20.2\t-82.1\n20.4\t-82\n20.6\t-81.9\n20.8\t-81.8\n21\t-81.7\n21.2\t-81.6\n21.4\t-81.5\n21.6\t-81.4\n21.8\t-81.3\n22\t-81.2\n22.2\t-81.1\n22.4\t-81\n22.6\t-80.9\n22.8\t-80.8\n23\t-80.7\n23.2\t-80.6\n23.4\t-80.5\n23.6\t-80.4\n23.8\t-80.3\n24\t-80.2\n24.2\t-80.1\n24.4\t-80\n24.6\t-79.9\n24.8\t-79.8\n25\t-79.7\n25.2\t-79.6\n25.4\t-79.5\n25.6\t-79.4\n25.8\t-79.3\n26\t-79.2\n26.2\t-79.1\n26.4\t-79\n26.6\t-78.9\n26.8\t-78.8\n27\t-78.7\n27.2\t-78.6\n27.4\t-78.5\n27.6\t-78.4\n27.8\t-78.3\n28\t-78.2\n28.2\t-78.1\n28.4\t-78\n28.6\t-77.9\n28.8\t-77.8\n29\t-77.7\n29.2\t-77.6\n29.4\t-77.5\n29.6\t-77.4\n29.8\t-77.3\n30\t-77.2\n30.2\t-77.1\n30.4\t-77\n30.6\t-76.9\n30.8\t-76.8\n31\t-76.7\n31.2\t-76.6\n31.4\t-76.5\n31.6\t-76.4\n31.8\t-76.3\n32\t-76.2\n32.2\t-76.1\n32.4\t-76\n32.6\t-75.9\n32.8\t-75.8\n33\t-75.7\n33.2\t-75.6\n33.4\t-75.5\n33.6\t-75.4\n33.8\t-75.3\n34\t-75.2\n34.2\t-75.1\n34.4\t-75\n34.6\t-74.9\n34.8\t-74.8\n35\t-74.7\n35.2\t-74.6\n35.4\t-74.5\n35.6\t-74.4\n35.8\t-74.3\n36\t-74.2\n36.2\t-74.1\n36.4\t-74\n36.6\t-73.9\n36.8\t-73.8\n37\t-73.7\n37.2\t-73.6\n37.4\t-73.5\n37.6\t-73.4\n37.8\t-73.3\n38\t-73.2\n38.2\t-73.1\n38.4\t-73\n38.6\t-72.9\n38.8\t-72.8\n39\t-72.7\n39.2\t-72.6\n39.4\t-72.5\n39.6\t-72.4\n39.8\t-72.3\n40\t-72.2\n40.2\t-72.1\n40.4\t-72\n40.6\t-71.9\n40.8\t-71.8\n41\t-71.7\n41.2\t-71.6\n41.4\t-71.5\n41.6\t-71.4\n41.8\t-71.3\n42\t-71.2\n42.2\t-71.1\n42.4\t-71\n42.6\t-70.9\n42.8\t-70.8\n43\t-70.7\n43.2\t-70.6\n43.4\t-70.5\n43.6\t-70.4\n43.8\t-70.3\n44\t-70.2\n44.2\t-70.1\n44.4\t-70\n44.6\t-69.9\n44.8\t-69.8\n45\t-69.7\n45.2\t-69.6\n45.4\t-69.5\n45.6\t-69.4\n45.8\t-69.3\n46\t-69.2\n46.2\t-69.1\n46.4\t-69\n46.6\t-68.9\n46.8\t-68.8\n47\t-68.7\n47.2\t-68.6\n47.4\t-68.5\n47.6\t-68.4\n47.8\t-68.3\n48\t-68.2\n48.2\t-68.1\n48.4\t-68\n48.6\t-67.9\n48.8\t-67.8\n49\t-67.7\n49.2\t-67.6\n49.4\t-67.5\n49.6\t-67.4\n49.8\t-67.3\n50\t-67.2\n50.2\t-67.1\n50.4\t-67\n50.6\t-66.9\n50.8\t-66.8\n51\t-66.7\n51.2\t-66.6\n51.4\t-66.5\n51.6\t-66.4\n51.8\t-66.3\n52\t-66.2\n52.2\t-66.1\n52.4\t-66\n52.6\t-65.9\n52.8\t-65.8\n53\t-65.7\n53.2\t-65.6\n53.4\t-65.5\n53.6\t-65.4\n53.8\t-65.1\n54\t-64.8\n54.2\t-64.5\n54.4\t-64.2\n54.6\t-63.9\n54.8\t-63.6\n55\t-63.3\n55.2\t-63\n55.4\t-62.7\n55.6\t-62.4\n55.8\t-62.1\n56\t-61.8\n56.2\t-61.5\n56.4\t-61.2\n56.6\t-60.9\n56.8\t-60.6\n57\t-60.3\n57.2\t-60\n57.4\t-59.7\n57.6\t-59.4\n57.8\t-59.1\n58\t-58.8\n58.2\t-58.5\n58.4\t-58.2\n58.6\t-57.9\n58.8\t-57.6\n59\t-57.3\n59.2\t-57\n59.4\t-56.7\n59.6\t-56.4\n59.8\t-56.1\n60\t-55.8\n60.2\t-55.5\n60.4\t-55.2\n60.6\t-54.9\n60.8\t-54.6\n61\t-54.3\n61.2\t-54\n61.4\t-53.7\n61.6\t-53.4\n61.8\t-53.1\n62\t-52.8\n62.2\t-52.5\n62.4\t-52.2\n62.6\t-51.9\n62.8\t-51.6\n63\t-51.3\n63.2\t-51\n63.4\t-50.7\n63.6\t-50.4\n63.8\t-50.1\n64\t-49.8\n64.2\t-49.5\n64.4\t-49.2\n64.6\t-48.9\n64.8\t-48.6\n65\t-48.3\n65.2\t-48\n65.4\t-47.7\n65\t-47.4\n64.6\t-47.1\n64.2\t-46.8\n63.8\t-46.5\n63.4\t-46.2\n63\t-45.9\n62.6\t-45.6\n62.2\t-45.3\n61.8\t-45\n61.4\t-44.7\n61\t-44.4\n60.6\t-44.1\n60.2\t-43.8\n59.8\t-43.5\n59.4\t-43.2\n59\t-42.9\n58.6\t-42.6\n58.2\t-42.3\n57.8\t-42\n57.4\t-41.7\n57\t-41.4\n56.6\t-41.1\n56.2\t-40.8\n55.8\t-40.5\n55.4\t-40.2\n55\t-39.9\n54.6\t-39.6\n54.2\t-39.3\n53.8\t-39\n53.4\t-38.7\n53\t-38.4\n52.6\t-38.1\n52.2\t-37.8\n51.8\t-37.5\n51.4\t-37.2\n51\t-36.9\n50.6\t-36.6\n50.2\t-36.3\n49.8\t-36\n49.4\t-35.7\n49\t-35.4\n48.6\t-35.1\n48.2\t-34.8\n47.8\t-34.5\n47.4\t-34.2\n47\t-33.9\n46.6\t-33.6\n46.2\t-33.3\n45.8\t-33\n45.4\t-32.7\n45\t-32.4\n44.6\t-32.1\n44.2\t-31.8\n43.8\t-31.5\n43.4\t-31.2\n43\t-30.9\n42.6\t-30.6\n42.2\t-30.3\n41.8\t-30\n41.4\t-29.7\n41\t-29.4\n40.6\t-29.1\n40.2\t-28.8\n39.8\t-28.5\n39.4\t-28.2\n39\t-27.9\n38.6\t-27.6\n38.2\t-27.3\n37.8\t-27\n37.4\t-26.7\n37\t-26.4\n36.6\t-26.1\n36.2\t-25.8\n35.8\t-25.5\n35.4\t-25.2\n35\t-24.9\n34.6\t-24.6\n34.2\t-24.3\n33.8\t-24\n33.4\t-23.7\n33\t-23.4\n32.6\t-23.1\n32.2\t-22.8\n31.8\t-22.5\n31.4\t-22.2\n31\t-21.9\n30.6\t-21.6\n30.2\t-21.3\n29.8\t-21\n29.4\t-20.7\n29\t-20.4\n28.6\t-20.1\n28.2\t-19.8\n27.8\t-19.5\n27.4\t-19.2\n27\t-18.9\n26.6\t-18.6\n26.2\t-18.3\n25.8\t-18\n25.4\t-17.7\n25\t-17.4\n24.6\t-17.1\n24.2\t-16.8\n23.8\t-16.5\n23.4\t-16.2\n23\t-15.9\n22.6\t-15.6\n22.2\t-15.3\n21.8\t-15\n21.4\t-14.7\n21\t-14.4\n20.6\t-14.1\n20.2\t-13.8\n19.8\t-13.5\n19.4\t-13.2\n19\t-12.9\n18.6\t-12.6\n18.2\t-12.3\n17.8\t-12\n17.4\t-11.7\n17\t-11.4\n16.6\t-11.1\n16.2\t-10.8\n15.8\t-10.5\n15.4\t-10.2\n15\t-9.9\n14.6\t-9.6\n14.2\t-9.3\n13.8\t-9\n13.4\t-8.7\n13\t-8.4\n12.6\t-8.1\n12.2\t-7.8\n11.8\t-7.5\n11.4\t-7.2\n11\t-6.9\n10.6\t-6.6\n10.2\t-6.3\n9.8\t-6\n9.4\t-5.7\n9\t-5.4\n8.6\t-5.1\n8.2\t-4.8\n7.8\t-4.5\n7.4\t-4.2\n7\t-3.9\n6.6\t-3.6\n6.2\t-3.3\n5.8\t-3\n5.4\t-2.7\n5\t-2.4\n4.6\t-2.1\n4.2\t-1.8\n3.8\t-1.5\n3.4\t-1.2\n3\t-0.9\n2.6\t-0.6\n2.2\t-0.3\n1.8\t-1.83087E-12\n1.4\t0.3\n1\t0.6\n0.6\t0.9\n0.2\t1.2\n-0.2\t1.5\n-0.6\t1.8\n-1\t2.1\n-1.4\t2.4\n-1.8\t2.7\n-2.2\t3\n-2.6\t3.3\n-3\t3.6\n-3.4\t3.9\n-3.8\t4.2\n-4.2\t4.5\n-4.6\t4.8\n-5\t5.1\n-5.4\t5.4\n-5.8\t5.7\n-6.2\t6\n-6.6\t6.3\n-7\t6.6\n-7.4\t6.9\n-7.8\t7.2\n-8.2\t7.5\n-8.6\t7.8\n-9\t8.1\n-9.4\t8.4\n-9.8\t8.7\n-10.2\t9\n-10.6\t9.3\n-11\t9.6\n-11.4\t9.9\n-11.8\t10.2\n-12.2\t10.5\n-12.6\t10.8\n-13\t11.1\n-13.4\t11.4\n-13.8\t11.7\n-14.2\t12\n-14.6\t12.3\n-15\t12.6\n-15.4\t12.9\n-15.8\t13.2\n-16.2\t13.5\n-16.6\t13.8\n-17\t14.1\n-17.4\t14.4\n-17.8\t14.7\n-18.2\t15\n-18.6\t15.3\n-19\t15.6\n-19.4\t15.9\n-19.8\t16.2\n-20.2\t16.5\n-20.6\t16.8\n-21\t17.1\n-21.4\t17.4\n-21.8\t17.7\n-22.2\t18\n-22.6\t18.3\n-23\t18.6\n-23.4\t18.9\n-23.8\t19.2\n-24.2\t19.5\n-24.6\t19.8\n-25\t20.1\n-25.4\t20.4\n-25.8\t20.7\n-26.2\t21\n-26.6\t21.3\n-27\t21.6\n-27.4\t21.9\n-27.8\t22.2\n-28.2\t22.5\n-28.6\t22.8\n-29\t23.1\n-29.4\t23.4\n-29.8\t23.7\n-30.2\t24\n-30.6\t24.3\n-31\t24.6\n-31.4\t24.9\n-31.8\t25.2\n-32.2\t25.5\n-32.6\t25.8\n-33\t26.1\n-33.4\t26.4\n-33.8\t26.7\n-34.2\t27\n-34.6\t27.3\n-35\t27.6\n-35.4\t27.9\n-35.8\t28.2\n-36.2\t28.5\n-36.6\t28.8\n-37\t29.1\n-37.4\t29.4\n-37.8\t29.7\n-38.2\t30\n-38.6\t30.3\n-39\t30.6\n-39.4\t30.9\n-39.8\t31.2\n-40.2\t31.5\n-40.6\t31.8\n-41\t32.1\n-41.4\t32.4\n-41.8\t32.7\n-42.2\t33\n-42.6\t33.3\n-43\t33.6\n-43.4\t33.9\n-43.8\t34.2\n-44.2\t34.5\n-44.6\t34.8\n-45\t35.1\n-45.4\t35.4\n-45.8\t35.7\n-46.2\t36\n-46.6\t36.3\n-47\t36.6\n-47.4\t36.9\n-47.8\t37.2\n-48.2\t37.5\n-48.6\t37.8\n-49\t38.1\n-49.4\t38.4\n-49.8\t38.7\n-50.2\t39\n-50.6\t39.3\n-51\t39.6\n-51.4\t39.9\n-51.8\t40.2\n-52.2\t40.5\n-52.6\t40.8\n-53\t41.1\n-53.4\t41.4\n-53.8\t41.7\n-54.2\t42\n-54.6\t42.3\n-55\t42.6\n-55.4\t42.9\n-55.8\t43.2\n-56.2\t43.5\n-55.6\t43.8\n-55\t44.1\n-54.4\t44.4\n-53.8\t44.7\n-53.2\t45\n-52.6\t45.3\n-52\t45.6\n-51.4\t45.9\n-50.8\t46.2\n-50.2\t46.5\n-49.6\t46.8\n-49\t47.1\n-48.4\t47.4\n-47.8\t47.7\n-47.2\t48\n-46.6\t48.3\n-46\t48.6\n-45.4\t48.9\n-44.8\t49.2\n-44.2\t49.5\n-43.6\t49.8\n-43\t50.1\n-42.4\t50.4\n-41.8\t50.7\n-41.2\t51\n-40.6\t51.3\n-40\t51.6\n-39.4\t51.9\n-38.8\t52.2\n-38.2\t52.5\n-37.6\t52.8\n-37\t53.1\n-36.4\t53.4\n-35.8\t53.7\n-35.2\t54\n-34.6\t54.3\n-34\t54.6\n-33.4\t54.9\n-32.8\t55.2\n-32.2\t55.5\n-31.6\t55.8\n-31\t56.1\n-30.4\t56.4\n-29.8\t56.7\n-29.2\t57\n-28.6\t57.3\n-28\t57.6\n-27.4\t57.9\n-26.8\t58.2\n-26.2\t58.5\n-25.6\t58.8\n-25\t59.1\n-24.4\t59.4\n-23.8\t59.7\n-23.2\t60\n-22.6\t60.3\n-22\t60.6\n-21.4\t60.9\n-20.8\t61.2\n-20.2\t61.5\n-19.6\t61.8\n-19\t62.1\n-18.4\t62.4\n-17.8\t62.7\n-17.2\t63\n-16.6\t63.3\n-16\t63.6\n-15.4\t63.9\n-14.8\t64.2\n-14.2\t64.5\n-13.6\t64.8\n-13\t65.1\n-12.4\t65.4\n-11.8\t65.7\n-11.2\t66\n-10.6\t66.3\n-10\t66.6\n-9.4\t66.9\n-8.8\t67.2\n-8.2\t67.5\n-7.6\t67.8\n-7\t68.1\n-6.4\t68.4\n-5.8\t68.7\n-5.2\t69\n-4.6\t69.3\n-4\t69.6\n-3.4\t69.9\n-2.8\t70.2\n-2.2\t70.5\n-1.6\t70.8\n-1\t71.1\n-0.4\t71.4\n0.2\t71.7\n0.8\t72\n1.4\t72.3\n2\t72.6\n2.6\t72.9\n3.2\t73.2\n3.8\t73.5\n4.4\t73.8\n5\t74.1\n5.6\t74.4\n6.2\t74.7\n6.8\t75\n7.4\t75.3\n8\t75.6\n8.6\t75.9\n9.2\t76.2\n9.8\t76.5\n10.4\t76.8\n11\t77.1\n11.6\t77.4\n12.2\t77.7\n12.8\t78\n13.4\t78.3\n14\t78.6\n14.6\t78.9\n15.2\t79.2\n15.8\t79.5\n16.4\t79.8\n17\t80.1\n17.6\t80.4\n18.2\t80.7\n18.8\t81\n19.4\t81.3\n20\t81.6\n20.6\t81.9\n21.2\t82.2\n21.8\t82.5\n22.4\t82.8\n23\t83.1\n23.6\t83.4\n24.2\t83.7\n24.8\t84\n25.4\t84.3\n26\t84.6\n26.6\t84.9\n27.2\t85.2\n27.8\t85.5\n28.4\t85.8\n29\t86.1\n29.6\t86.4\n30.2\t86.7\n30.8\t87\n31.4\t87.3\n32\t87.6\n32.6\t87.9\n33.2\t88.2\n33.8\t88.5\n34.4\t88.8\n35\t89.1\n35.6\t89.4\n36.2\t89.7\n36.8\t90\n37.4\t90.3\n38\t90.6\n38.6\t90.9\n39.2\t91.2\n39.8\t91.5\n40.4\t91.8\n41\t92.1\n41.6\t92.4\n42.2\t92.7\n42.8\t93\n43.4\t93.3\n44\t93.6\n44.6\t93.9\n45.2\t93.2\n45.8\t92.5\n46.4\t91.8\n47\t91.1\n47.6\t90.4\n48.2\t89.7\n48.8\t89\n49.4\t88.3\n50\t87.6\n50.6\t86.9\n51.2\t86.2\n51.8\t85.5\n52.4\t84.8\n53\t84.1\n53.6\t83.4\n54.2\t82.7\n54.8\t82\n55.4\t81.3\n56\t80.6\n56.6\t79.9\n57.2\t79.2\n57.8\t78.5\n58.4\t77.8\n59\t77.1\n59.6\t76.4\n60.2\t75.7\n60.8\t75\n61.4\t74.3\n62\t73.6\n62.6\t72.9\n63.2\t72.2\n63.8\t71.5\n64.4\t70.8\n65\t70.1\n65.6\t69.4\n66.2\t68.7\n66.8\t68\n67.4\t67.3\n68\t66.6\n68.6\t65.9\n69.2\t65.2\n69.8\t64.5\n70.4\t63.8\n71\t63.1\n71.6\t62.4\n72.2\t61.7\n72.8\t61\n73.4\t60.3\n74\t59.6\n74.6\t58.9\n75.2\t58.2\n75.8\t57.5\n76.4\t56.8\n77\t56.1\n77.6\t55.4\n78.2\t54.7\n78.8\t54\n79.4\t53.3\n80\t52.6\n80.6\t51.9\n81.2\t51.2\n81.8\t50.5\n82.4\t49.8\n83\t49.1\n83.6\t48.4\n84.2\t47.7\n84.8\t47\n85.4\t46.3\n86\t45.6\n86.6\t44.9\n87.2\t44.2\n87.8\t43.5\n88.4\t42.8\n89\t42.1\n89.6\t41.4\n90.2\t40.7\n90.8\t40\n91.4\t39.3\n92\t38.6\n92.6\t37.9\n93.2\t37.2\n93\t36.5\n92.8\t35.8\n92.6\t35.1\n92.4\t34.4\n92.2\t33.7\n92\t33\n91.8\t32.3\n91.6\t31.6\n91.4\t30.9\n91.2\t30.2\n91\t29.5\n90.8\t28.8\n90.6\t28.1\n90.4\t27.4\n90.2\t26.7\n90\t26\n89.8\t25.3\n89.6\t24.6\n89.4\t23.9\n89.2\t23.2\n89\t22.5\n88.8\t21.8\n88.6\t21.1\n88.4\t20.4\n88.2\t19.7\n88\t19\n87.8\t18.3\n87.6\t17.6\n87.4\t16.9\n87.2\t16.2\n87\t15.5\n86.8\t14.8\n86.6\t14.1\n86.4\t13.4\n86.2\t12.7\n86\t12\n85.8\t11.3\n85.6\t10.6\n85.4\t9.9\n85.2\t9.2\n85\t8.5\n84.8\t7.8\n84.6\t7.1\n84.4\t6.4\n84.2\t5.7\n84\t5\n83.8\t4.3\n83.6\t3.6\n83.4\t2.9\n83.2\t2.2\n83\t1.5\n82.8\t0.8\n82.6\t0.1\n82.4\t-0.6\n82.2\t-1.3\n82\t-2\n81.8\t-2.7\n81.6\t-3.4\n81.4\t-4.1\n81.2\t-4.8\n81\t-5.5\n80.8\t-6.2\n80.6\t-6.9\n80.4\t-7.6\n80.2\t-8.3\n80\t-9\n79.8\t-9.7\n79.6\t-10.4\n79.4\t-11.1\n79.2\t-11.8\n79\t-12.5\n78.8\t-13.2\n78.6\t-13.9\n78.4\t-14.6\n78.2\t-15.3\n78\t-16\n77.8\t-16.7\n77.6\t-17.4\n77.4\t-18.1\n77.2\t-18.8\n77\t-19.5\n76.8\t-20.2\n76.6\t-20.9\n76.4\t-21.6\n76.2\t-22.3\n76\t-23\n75.8\t-23.7\n75.6\t-24.4\n75.4\t-25.1\n75.2\t-25.8\n75\t-26.5\n74.8\t-27.2\n74.6\t-27.9\n74.4\t-28.6\n74.2\t-29.3\n74\t-30\n73.8\t-30.7\n73.6\t-31.4\n73.4\t-32.1\n73.2\t-32.8\n73\t-33.5\n72.8\t-34.2\n72.6\t-34.9\n72.4\t-35.6\n72.2\t-36.3\n72\t-37\n71.8\t-37.7\n71.6\t-38.4\n71.4\t-39.1\n71.2\t-39.8\n71\t-40.5\n70.8\t-41.2\n70.6\t-41.9\n70.4\t-42.6\n70.2\t-43.3\n70\t-44\n69.8\t-44.7\n69.6\t-45.4\n69.4\t-46.1\n69.2\t-46.8\n69\t-47.5\n68.8\t-48.2\n68.6\t-48.9\n68.4\t-49.6\n68.2\t-50.3\n68\t-51\n67.8\t-51.7\n67.6\t-52.4\n67.4\t-53.1\n67.2\t-53.8\n67\t-54.5\n66.8\t-55.2\n66.6\t-55.9\n66.4\t-56.6\n66.2\t-57.3\n66\t-58\n65.8\t-58.7\n65.6\t-59.4\n65.4\t-60.1\n65.2\t-60.8\n65\t-61.5\n64.8\t-62.2\n64.6\t-62.9\n64.4\t-63.6\n64.2\t-64.3\n64\t-65\n63.8\t-65.7\n63.6\t-66.4\n63.4\t-67.1\n63.2\t-67.8\n63\t-68.5\n62.8\t-69.2\n62.6\t-69.9\n62.4\t-70.6\n62.2\t-71.3\n62\t-72\n61.8\t-72.7\n61.6\t-73.4\n61.4\t-74.1\n61.2\t-74.8\n61\t-75.5\n60.8\t-75\n60.6\t-74.5\n60.4\t-74\n60.2\t-73.5\n60\t-73\n59.8\t-72.5\n59.6\t-72\n59.4\t-71.5\n59.2\t-71\n59\t-70.5\n58.8\t-70\n58.6\t-69.5\n58.4\t-69\n58.2\t-68.5\n58\t-68\n57.8\t-67.5\n57.6\t-67\n57.4\t-66.5\n57.2\t-66\n57\t-65.5\n56.8\t-65\n56.6\t-64.5\n56.4\t-64\n56.2\t-63.5\n56\t-63\n55.8\t-62.5\n55.6\t-62\n55.4\t-61.5\n55.2\t-61\n55\t-60.5\n54.8\t-60\n54.6\t-59.5\n54.4\t-59\n54.2\t-58.5\n54\t-58\n53.8\t-57.5\n53.6\t-57\n53.4\t-56.5\n53.2\t-56\n53\t-55.5\n52.8\t-55\n52.6\t-54.5\n52.4\t-54\n52.2\t-53.5\n52\t-53\n51.8\t-52.5\n51.6\t-52\n51.4\t-51.5\n51.2\t-51\n51\t-50.5\n50.8\t-50\n50.6\t-49.5\n50.4\t-49\n50.2\t-48.5\n50\t-48\n49.8\t-47.5\n49.6\t-47\n49.4\t-46.5\n49.2\t-46\n49\t-45.5\n48.8\t-45\n48.6\t-44.5\n48.4\t-44\n48.2\t-43.5\n48\t-43\n47.8\t-42.5\n47.6\t-42\n47.4\t-41.5\n47.2\t-41\n47\t-40.5\n46.8\t-40\n46.6\t-39.5\n46.4\t-39\n46.2\t-38.5\n46\t-38\n45.8\t-37.5\n45.6\t-37\n45.4\t-36.5\n45.2\t-36\n45\t-35.5\n44.8\t-35\n44.6\t-34.5\n44.4\t-34\n44.2\t-33.5\n44\t-33\n43.8\t-32.5\n43.6\t-32\n43.4\t-31.5\n43.2\t-31\n43\t-30.5\n42.8\t-30\n42.6\t-29.5\n42.4\t-29\n42.2\t-28.5\n42\t-28\n41.8\t-27.5\n41.6\t-27\n41.4\t-26.5\n41.2\t-26\n41\t-25.5\n40.8\t-25\n40.6\t-24.5\n40.4\t-24\n40.2\t-23.5\n40\t-23\n39.8\t-22.5\n39.6\t-22\n39.4\t-21.5\n39.2\t-21\n39\t-20.5\n38.8\t-20\n38.6\t-19.5\n38.4\t-19\n38.2\t-18.5\n38\t-18\n37.8\t-17.5\n37.6\t-17\n37.4\t-16.5\n37.2\t-16\n37\t-15.5\n36.8\t-15\n36.6\t-14.5\n36.4\t-14\n36.2\t-13.5\n36\t-13\n35.8\t-12.5\n35.6\t-12\n35.4\t-11.5\n35.2\t-11\n35\t-10.5\n34.8\t-10\n34.6\t-9.5\n34.4\t-9\n34.2\t-8.5\n34\t-8\n33.8\t-7.5\n33.6\t-7\n33.4\t-6.5\n33.2\t-6\n33\t-5.5\n32.8\t-5\n32.6\t-4.5\n32.4\t-4\n32.2\t-3.5\n32\t-3\n31.8\t-2.5\n31.6\t-2\n31.4\t-1.5\n31.2\t-1\n31\t-0.5\n30.8\t-2.74269E-12\n30.6\t0.5\n30.4\t1\n30.2\t1.5\n30\t2\n29.8\t2.5\n29.6\t3\n29.4\t3.5\n29.2\t4\n29\t4.5\n28.8\t5\n28.6\t5.5\n28.4\t6\n28.2\t6.5\n28\t7\n27.8\t7.5\n27.6\t8\n27.4\t8.5\n27.2\t9\n27\t9.5\n26.8\t10\n26.6\t10.5\n26.4\t11\n26.2\t11.5\n26\t12\n25.8\t12.5\n25.6\t13\n25.4\t13.5\n25.2\t14\n25\t14.5\n24.8\t15\n24.6\t15.5\n24.4\t16\n24.2\t16.5\n24\t17\n23.8\t17.5\n23.6\t18\n23.4\t18.5\n23.2\t19\n23\t19.5\n22.8\t20\n22.6\t20.5\n22.4\t21\n22.2\t21.5\n22\t22\n21.8\t22.5\n21.6\t23\n21.4\t23.5\n21.2\t24\n21\t24.5\n20.8\t25\n20.6\t25.5\n20.4\t26\n20.2\t26.5\n20\t27\n19.8\t27.5\n19.6\t28\n19.4\t28.5\n19.2\t29\n19\t29.5\n18.8\t30\n18.6\t30.5\n18.4\t31\n18.2\t31.5\n18\t32\n17.8\t32.5\n17.6\t33\n17.4\t33.5\n17.2\t34\n17\t34.5\n16.8\t35\n16.6\t35.5\n16.4\t36\n16.2\t35.8\n16\t35.6\n15.8\t35.4\n15.6\t35.2\n15.4\t35\n15.2\t34.8\n15\t34.6\n14.8\t34.4\n14.6\t34.2\n14.4\t34\n14.2\t33.8\n14\t33.6\n13.8\t33.4\n13.6\t33.2\n13.4\t33\n13.2\t32.8\n13\t32.6\n12.8\t32.4\n12.6\t32.2\n12.4\t32\n12.2\t31.8\n12\t31.6\n11.8\t31.4\n11.6\t31.2\n11.4\t31\n11.2\t30.8\n11\t30.6\n10.8\t30.4\n10.6\t30.2\n10.4\t30\n10.2\t29.8\n10\t29.6\n9.8\t29.4\n9.6\t29.2\n9.4\t29\n9.2\t28.8\n9\t28.6\n8.8\t28.4\n8.6\t28.2\n8.4\t28\n8.2\t27.8\n8\t27.6\n7.8\t27.4\n7.6\t27.2\n7.4\t27\n7.2\t26.8\n7\t26.6\n6.8\t26.4\n6.6\t26.2\n6.4\t26\n6.2\t25.8\n6\t25.6\n5.8\t25.4\n5.6\t25.2\n5.4\t25\n5.2\t24.8\n5\t24.6\n4.8\t24.4\n4.6\t24.2\n4.4\t24\n4.2\t23.8\n4\t23.6\n3.8\t23.4\n3.6\t23.2\n3.4\t23\n3.2\t22.8\n3\t22.6\n2.8\t22.4\n2.6\t22.2\n2.4\t22\n2.2\t21.8\n2\t21.6\n1.8\t21.4\n1.6\t21.2\n1.4\t21\n1.2\t20.8\n1\t20.6\n0.8\t20.4\n0.6\t20.2\n0.4\t20\n0.2\t19.8\n8.04967E-13\t19.6\n-0.2\t19.4\n-0.4\t19.2\n-0.6\t19\n-0.8\t18.8\n-1\t18.6\n-1.2\t18.4\n-1.4\t18.2\n-1.6\t18\n-1.8\t17.8\n-2\t17.6\n-2.2\t17.4\n-2.4\t17.2\n-3\t17\n-3.6\t16.8\n-4.2\t16.6\n-4.8\t16.4\n-5.4\t16.2\n-6\t16\n-6.6\t15.8\n-7.2\t15.6\n-7.8\t15.4\n-8.4\t15.2\n-9\t15\n-9.6\t14.8\n-10.2\t14.6\n-10.8\t14.4\n-11.4\t14.2\n-12\t14\n-12.6\t13.8\n-13.2\t13.6\n-13.8\t13.4\n-14.4\t13.2\n-15\t13\n-15.6\t12.8\n-16.2\t12.6\n-16.8\t12.4\n-17.4\t12.2\n-18\t12\n-18.6\t11.8\n-19.2\t11.6\n-19.8\t11.4\n-20.4\t11.2\n-21\t11\n-21.6\t10.8\n-22.2\t10.6\n-22.8\t10.4\n-23.4\t10.2\n-24\t10\n-24.6\t9.8\n-25.2\t9.6\n-25.8\t9.4\n-26.4\t9.2\n-27\t9\n-27.6\t8.8\n-28.2\t8.6\n-28.8\t8.4\n-29.4\t8.2\n-30\t8\n-30.6\t7.8\n-31.2\t7.6\n-31.8\t7.4\n-32.4\t7.2\n-33\t7\n-33.6\t6.8\n-34.2\t6.6\n-34.8\t6.4\n-35.4\t6.2\n-36\t6\n-36.6\t5.8\n-37.2\t5.6\n-37.8\t5.4\n-38.4\t5.2\n-39\t5\n-39.6\t4.8\n-40.2\t4.6\n-40.8\t4.4\n-41.4\t4.2\n-42\t4\n-42.6\t3.8\n-43.2\t3.6\n-43.8\t3.4\n-44.4\t3.2\n-45\t3\n-45.6\t2.8\n-46.2\t2.6\n-46.8\t2.4\n-47.4\t2.2\n-48\t2\n-48.6\t1.8\n-49.2\t1.6\n-49.8\t1.4\n-50.4\t1.2\n-51\t1\n-51.6\t0.8\n-52.2\t0.6\n-52.8\t0.4\n-53.4\t0.2\n-54\t-2.71644E-12\n-54.6\t-0.2\n-55.2\t-0.4\n-55.8\t-0.6\n-56.4\t-0.8\n-57\t-1\n-57.6\t-1.2\n-58.2\t-1.4\n-58.8\t-1.6\n-59.4\t-1.8\n-60\t-2\n-60.6\t-2.2\n-61.2\t-2.4\n-61.8\t-2.6\n-62.4\t-2.8\n-63\t-3\n-63.6\t-3.2\n-64.2\t-3.4\n-64.8\t-3.6\n-65.4\t-3.8\n-66\t-4\n-66.6\t-4.2\n-67.2\t-4.4\n-67.8\t-4.6\n-68.4\t-4.8\n-69\t-5\n-69.6\t-5.2\n-70.2\t-5.4\n-70.8\t-5.6\n-71.4\t-5.8\n-72\t-6\n-72.6\t-6.2\n-73.2\t-6.4\n-73.8\t-6.6\n-74.4\t-6.8\n-75\t-7\n-75.6\t-7.2\n-76.2\t-7.4\n-76.8\t-7.6\n-77.4\t-7.8\n-78\t-8\n-78.6\t-8.2\n-79.2\t-8.4\n-79.8\t-8.6\n-80.4\t-8.8\n-81\t-9\n-81.6\t-9.2\n-82.2\t-9.4\n-82.8\t-9.6\n-83.4\t-9.8\n-84\t-10\n-84.6\t-10.2\n-85.2\t-10.4\n-85.8\t-10.6\n-86.4\t-10.8\n-87\t-11\n-87.6\t-11.2\n-88.2\t-11.4\n-88.8\t-11.6\n-89.4\t-11.8\n-90\t-12\n-90.6\t-12.2\n-91.2\t-12.4\n-91.8\t-12.6\n-92.4\t-12.8\n-92.2\t-13\n-92\t-13.2\n-91.8\t-13.4\n-91.6\t-13.6\n-91.4\t-13.8\n-91.2\t-14\n-91\t-14.2\n-90.8\t-14.4\n-90.6\t-14.6\n-90.4\t-14.8\n-90.2\t-15\n-90\t-15.2\n-89.8\t-15.4\n-89.6\t-15.6\n-89.4\t-15.8\n-89.2\t-16\n-89\t-16.2\n-88.8\t-16.4\n-88.6\t-16.6\n-88.4\t-16.8\n-88.2\t-17\n-88\t-17.2\n-87.8\t-17.4\n-87.6\t-17.6\n-87.4\t-17.8\n-87.2\t-18\n-87\t-18.2\n-86.8\t-18.4\n-86.6\t-18.6\n-86.4\t-18.8\n-86.2\t-19\n-86\t-19.2\n-85.8\t-19.4\n-85.6\t-19.6\n-85.4\t-19.8\n-85.2\t-20\n-85\t-20.2\n-84.8\t-20.4\n-84.6\t-20.6\n-84.4\t-20.8\n-84.2\t-21\n-84\t-21.2\n-83.8\t-21.4\n-83.6\t-21.6\n-83.4\t-21.8\n-83.2\t-22\n-83\t-22.2\n-82.8\t-22.4\n-82.6\t-22.6\n-82.4\t-22.8\n-82.2\t-23\n-82\t-23.2\n-81.8\t-23.4\n-81.6\t-23.6\n-81.4\t-23.8\n-81.2\t-24\n-81\t-24.2\n-80.8\t-24.4\n-80.6\t-24.6\n-80.4\t-24.8\n-80.2\t-25\n-80\t-25.2\n-79.8\t-25.4\n-79.6\t-25.6\n-79.4\t-25.8\n-79.2\t-26\n-79\t-26.2\n-78.8\t-26.4\n-78.6\t-26.6\n-78.4\t-26.8\n-78.2\t-27\n-78\t-27.2\n-77.8\t-27.4\n-77.6\t-27.6\n-77.4\t-27.8\n-77.2\t-28\n-77\t-28.2\n-76.8\t-28.4\n-76.6\t-28.6\n-76.4\t-28.8\n-76.2\t-29\n-76\t-29.2\n-75.8\t-29.4\n-75.6\t-29.6\n-75.4\t-29.8\n-75.2\t-30\n-75\t-30.2\n-74.8\t-30.4\n-74.6\t-30.6\n-74.4\t-30.8\n-74.2\t-31\n-74\t-31.2\n-73.8\t-31.4\n-73.6\t-31.6\n-73.4\t-31.8\n-73.2\t-32\n-73\t-32.2\n-72.8\t-32.4\n-72.6\t-32.6\n-72.4\t-32.8\n-72.2\t-33\n-72\t-33.2\n-71.8\t-33.4\n-71.6\t-33.6\n-71.4\t-33.8\n-71.2\t-34\n-71\t-34.2\n-70.8\t-34.4\n-70.6\t-34.6\n-70.4\t-34.8\n-70.2\t-35\n-70\t-35.2\n-69.8\t-35.4\n-69.6\t-35.6\n-69.4\t-35.8\n-69.2\t-36\n-69\t-36.2\n-68.8\t-36.4\n-68.6\t-36.6\n-68.4\t-36.8\n-68.2\t-37\n-68\t-37.2\n-67.8\t-37.4\n-67.6\t-37.6\n-67.4\t-37.8\n-67.2\t-38\n-67\t-38.2\n-66.8\t-38.4\n-66.6\t-38.6\n-66.4\t-38.8\n-66.2\t-39\n-66\t-39.2\n-65.8\t-39.4\n-65.6\t-39.6\n-65.4\t-39.8\n-65.2\t-40\n-65\t-40.2\n-64.8\t-40.4\n-64.6\t-40.6\n-64.4\t-40.8\n-64.2\t-41\n-64\t-41.2\n-63.8\t-41.4\n-63.6\t-41.6\n-63.4\t-41.8\n-63.2\t-42\n-63\t-42.2\n-62.8\t-42.4\n-62.6\t-42.6\n-62.4\t-42.8\n-62.2\t-43\n-62\t-43.2\n-61.8\t-43.4\n-61.6\t-43.6\n-61.4\t-43.8\n-61.2\t-44\n-61\t-44.2\n-60.8\t-44.4\n-60.6\t-44.6\n-60.4\t-44.8\n-60.2\t-45\n-60\t-45.2\n-59.8\t-45.4\n-59.6\t-45.6\n-59.4\t-45.8\n-59.2\t-46\n-59\t-46.2\n-58.8\t-46.4\n-58.6\t-46.6\n-58.4\t-46.8\n-58.2\t-47\n-58\t-47.2\n-57.8\t-47.4\n-57.6\t-47.6\n-57.4\t-47.8\n-57.2\t-48\n-57\t-48.2\n-56.8\t-48.4\n-56.6\t-48.6\n-56.4\t-48.8\n-56.2\t-49\n-56\t-49.2\n-55.8\t-49.4\n-55.6\t-49.6\n-55.4\t-49.8\n-55.2\t-50\n-55\t-50.2\n-54.8\t-50.4\n-54.6\t-50.6\n-54.4\t-50.8\n-54.2\t-51\n-54\t-51.2\n-53.8\t-51.4\n-53.6\t-51.6\n-53.4\t-51.8\n-53.2\t-52\n-53\t-52.2\n-52.8\t-52.4\n-52.6\t-52.6\n-52.4\t-52.8\n-52.2\t-53\n-52\t-53.2\n-51.8\t-53.4\n-51.6\t-53.6\n-51.4\t-53.8\n-51.2\t-54\n-51\t-54.2\n-50.8\t-54.4\n-50.6\t-54.6\n-50.4\t-54.8\n-50.2\t-55\n-50\t-55.2\n-49.8\t-55.4\n-49.6\t-55.6\n-49.4\t-55.8\n-49.2\t-56\n-49\t-56.2\n-48.8\t-56.4\n-48.6\t-56.6\n-48.4\t-56.8\n-48.2\t-57\n-48\t-57.2\n-47.8\t-57.4\n-47.6\t-57.6\n-47.4\t-57.8\n-47.2\t-58\n-47\t-58.2\n-46.8\t-58.4\n-46.6\t-58.6\n-46.4\t-58.8\n-46.2\t-59\n-46\t-59.2\n-45.8\t-59.4\n-45.6\t-59.6\n-45.4\t-59.8\n-45.2\t-60\n-45\t-60.2\n-44.8\t-60.4\n-44.6\t-60.6\n-44.4\t-60.8\n-44.2\t-61\n-44\t-61.2\n-43.8\t-61.4\n-43.6\t-61.6\n-43.4\t-61.8\n-43.2\t-62\n-43\t-62.2\n-42.8\t-62.4\n-42.6\t-62.6\n-42.4\t-62.8\n-42.2\t-63\n-42\t-63.2\n-41.8\t-63.4\n-41.6\t-63.6\n-41.4\t-63.8\n-41.2\t-64\n-41\t-64.2\n-40.8\t-64.4\n-40.6\t-64.6\n-40.4\t-64.8\n-40.2\t-65\n-40\t-65.2\n-39.8\t-65.4\n-39.6\t-65.6\n-39.4\t-65.8\n-39.2\t-66\n-39\t-66.2\n-38.8\t-66.4\n-38.6\t-66.6\n-38.4\t-66.8\n-38.2\t-67\n-38\t-67.2\n-37.8\t-67.4\n-37.6\t-67.6\n-37.4\t-67.8\n-37.2\t-68\n-37\t-68.2\n-36.8\t-68.4\n-36.6\t-68.6\n-36.4\t-68.8\n-36.2\t-69\n-36\t-69.2\n-35.8\t-69.4\n-35.6\t-69.6\n-35.4\t-69.8\n-35.2\t-70\n-35\t-70.2\n-34.8\t-70.4\n-34.6\t-70.6\n-34.4\t-70.8\n-34.2\t-71\n-34\t-71.2\n-33.8\t-71.4\n-33.6\t-71.6\n-33.4\t-71.8\n-33.2\t-72\n-33\t-72.2\n-32.8\t-72.4\n-32.6\t-72.6\n-32.4\t-72.8\n-32.2\t-73\n-32\t-73.2\n-31.8\t-73.4\n-31.6\t-73.6\n-31.4\t-73.8\n-31.2\t-74\n-31\t-74.2\n-30.8\t-74.4\n-30.6\t-74.6\n-30.4\t-74.8\n-30.2\t-75\n-30\t-75.2\n-29.8\t-75.4\n-29.6\t-75.6\n-29.4\t-75.8\n-29.2\t-76\n-29\t-76.2\n-28.8\t-76.4\n-28.6\t-76.6\n-28.4\t-76.8\n-28.2\t-77\n-28\t-77.2\n-27.8\t-77.4\n-27.6\t-77.6\n-27.4\t-77.8\n-27.2\t-78\n-27\t-78.2\n-26.8\t-78.4\n-26.6\t-78.6\n-26.4\t-78.8\n-26.2\t-79\n-26\t-79.2\n-25.8\t-79.4\n-25.6\t-79.6\n-25.4\t-79.8\n-25.2\t-80\n-25\t-80.2\n-24.8\t-80.4\n-24.6\t-80.6\n-24.4\t-80.8\n-24.2\t-81\n-24\t-81.2\n-23.8\t-81.4\n-23.6\t-81.6\n-23.4\t-81.8\n-23.2\t-82\n-23\t-82.2\n-22.8\t-82.4\n-22.6\t-82.6\n-22.4\t-82.8\n-22.2\t-83\n-22\t-83.2\n-21.8\t-83.4\n-21.6\t-83.6\n-21.4\t-83.8\n-21.2\t-84\n-21\t-84.2\n-20.8\t-84.4\n-20.6\t-84.6\n-20.4\t-84.8\n-20.2\t-85\n-20\t-85.2\n-19.8\t-85.4\n-19.6\t-85.6\n-19.4\t-85.8\n-19.2\t-86\n-19\t-86.2\n-18.8\t-86.4\n-18.6\t-86.6\n-18.4\t-86.8\n-18.2\t-87\n-18\t-87.2\n-17.8\t-87.4\n-17.6\t-87.6\n-17.4\t-87.8\n-17.2\t-88\n-17\t-88.2\n-16.8\t-88.4\n-16.6\t-88.6\n-16.4\t-88.8\n-16.2\t-89\n-16\t-89.2\n-15.8\t-89.4\n-15.6\t-89.6\n-15.4\t-89.8\n-15.2\t-90\n-15\t-90.2\n-14.8\t-90.4\n-14.6\t-90.6\n-14.4\t-90.8\n-14.2\t-91\n-14\t-91.2\n-13.8\t-91.4\n-13.6\t-91.6\n-13.4\t-91.8\n-13.2\t-92\n-13\t-92.2\n-12.8\t-92.4\n-12.6\t-92.6\n-12.4\t-92.8\n-12.2\t-93\n-12\t-93.2\n-11.8\t-93.4\n-11.6\t-93.6\n-11.4\t-93.8\n-11.2\t-94\n-11\t-93.6\n-10.8\t-93.2\n-10.6\t-92.8\n-10.4\t-92.4\n-10.2\t-92\n-10\t-91.6\n-9.8\t-91.2\n-9.6\t-90.8\n-9.4\t-90.4\n-9.2\t-90\n-9\t-89.6\n-8.8\t-89.2\n-8.6\t-88.8\n-8.4\t-88.4\n-8.2\t-88\n-8\t-87.6\n-7.8\t-87.2\n-7.6\t-86.8\n-7.4\t-86.4\n-7.2\t-86\n-7\t-85.6\n-6.8\t-85.2\n-6.6\t-84.8\n-6.4\t-84.4\n-6.2\t-84\n-6\t-83.6\n-5.8\t-83.2\n-5.6\t-82.8\n-5.4\t-82.4\n-5.2\t-82\n-5\t-81.6\n-4.8\t-81.2\n-4.6\t-80.8\n-4.4\t-80.4\n-4.2\t-80\n-4\t-79.6\n-3.8\t-79.2\n-3.6\t-78.8\n-3.4\t-78.4\n-3.2\t-78\n-3\t-77.6\n-2.8\t-77.2\n-2.6\t-76.8\n-2.4\t-76.4\n-2.2\t-76\n-2\t-75.6\n-1.8\t-75.2\n-1.6\t-74.8\n-1.4\t-74.4\n-1.2\t-74\n-1\t-73.6\n-0.8\t-73.2\n-0.6\t-72.8\n-0.4\t-72.4\n-0.2\t-72\n1.7501E-12\t-71.6\n0.2\t-71.2\n0.4\t-70.8\n0.6\t-70.4\n0.8\t-70\n1\t-69.6\n1.2\t-69.2\n1.4\t-68.8\n1.6\t-68.4\n1.8\t-68\n2\t-67.6\n2.2\t-67.2\n2.4\t-66.8\n2.6\t-66.4\n2.8\t-66\n3\t-65.6\n3.2\t-65.2\n3.4\t-64.8\n3.6\t-64.4\n3.8\t-64\n4\t-63.6\n4.2\t-63.2\n4.4\t-62.8\n4.6\t-62.4\n4.8\t-62\n5\t-61.6\n5.2\t-61.2\n5.4\t-60.8\n5.6\t-60.4\n5.8\t-60\n6\t-59.6\n6.2\t-59.2\n6.4\t-58.8\n6.6\t-58.4\n6.8\t-58\n7\t-57.6\n7.2\t-57.2\n7.4\t-56.8\n7.6\t-56.4\n7.8\t-56\n8\t-55.6\n8.2\t-55.2\n8.4\t-54.8\n8.6\t-54.4\n8.8\t-54\n9\t-53.6\n9.2\t-53.2\n9.4\t-52.8\n9.6\t-52.4\n9.8\t-52\n10\t-51.6\n10.2\t-51.2\n10.4\t-50.8\n10.6\t-50.4\n10.8\t-50\n11\t-49.6\n11.2\t-49.2\n11.4\t-48.8\n11.6\t-48.4\n11.8\t-48\n12\t-47.6\n12.2\t-47.2\n12.4\t-46.8\n12.6\t-46.4\n12.8\t-46\n13\t-45.6\n13.2\t-45.2\n13.4\t-44.8\n13.6\t-44.4\n13.8\t-44\n14\t-43.6\n14.2\t-43.2\n14.4\t-42.8\n14.6\t-42.4\n14.8\t-42\n15\t-41.6\n15.2\t-41.2\n15.4\t-40.8\n15.6\t-40.4\n15.8\t-40\n16\t-39.6\n16.2\t-39.2\n16.4\t-38.8\n16.6\t-38.4\n16.8\t-38\n17\t-37.6\n17.2\t-37.2\n17.4\t-36.8\n17.6\t-36.4\n17.8\t-36\n18\t-35.6\n18.2\t-35.2\n18.4\t-34.8\n18.6\t-34.4\n18.8\t-34\n19\t-33.6\n19.2\t-33.2\n19.4\t-32.8\n19.6\t-32.4\n19.8\t-32\n20\t-31.6\n20.2\t-31.2\n20.4\t-30.8\n20.6\t-30.4\n20.8\t-30\n21\t-29.6\n21.2\t-29.2\n21.4\t-28.8\n21.6\t-28.4\n21.8\t-28\n22\t-27.6\n22.2\t-27.2\n22.4\t-26.8\n22.6\t-26.4\n22.8\t-26\n23\t-25.6\n23.2\t-25.2\n23.4\t-24.8\n23.6\t-24.4\n23.8\t-24\n24\t-23.6\n24.2\t-23.2\n24.4\t-22.8\n24.6\t-22.4\n24.8\t-22\n25\t-21.6\n25.2\t-21.2\n25.4\t-20.8\n25.6\t-20.4\n25.8\t-20\n26\t-19.6\n26.2\t-19.2\n26.4\t-18.8\n26.6\t-18.4\n26.8\t-18\n27\t-17.6\n27.2\t-17.2\n27.4\t-16.8\n27.6\t-16.4\n27.8\t-16\n28\t-15.6\n28.2\t-15.2\n28.4\t-14.8\n28.6\t-14.4\n28.8\t-14\n29\t-13.6\n29.2\t-13.2\n29.4\t-12.8\n29.6\t-12.4\n29.8\t-12\n30\t-11.6\n30.2\t-11.2\n30.4\t-10.8\n30.6\t-10.4\n30.8\t-10\n31\t-9.6\n31.2\t-9.2\n31.4\t-8.8\n31.6\t-8.4\n31.8\t-8\n32\t-7.6\n32.2\t-7.2\n32.4\t-6.8\n32.6\t-6.4\n32.8\t-6\n33\t-5.6\n33.2\t-5.2\n33.4\t-4.8\n33.6\t-4.4\n33.8\t-4\n34\t-3.6\n34.2\t-3.2\n34.4\t-2.8\n34.6\t-2.4\n34.8\t-2\n35\t-1.6\n35.2\t-1.2\n35.4\t-0.8\n35.6\t-0.4\n35.8\t0\n36\t0.5\n36.2\t1\n36.4\t1.5\n36.6\t2\n36.8\t2.5\n37\t3\n37.2\t3.5\n37.4\t4\n37.6\t4.5\n37.8\t5\n38\t5.5\n38.2\t6\n38.4\t6.5\n38.6\t7\n38.8\t7.5\n39\t8\n39.2\t8.5\n39.4\t9\n39.6\t9.5\n39.8\t10\n40\t10.5\n40.2\t11\n40.4\t11.5\n40.6\t12\n40.8\t12.5\n41\t13\n41.2\t13.5\n41.4\t14\n41.6\t14.5\n41.8\t15\n42\t15.5\n42.2\t16\n42.4\t16.5\n42.6\t17\n42.8\t17.5\n43\t18\n43.2\t18.5\n43.4\t19\n43.6\t19.5\n43.8\t20\n44\t20.5\n44.2\t21\n44.4\t21.5\n44.6\t22\n44.8\t22.5\n45\t23\n45.2\t23.5\n45.4\t24\n45.6\t24.5\n45.8\t25\n46\t25.5\n46.2\t26\n46.4\t26.5\n46.6\t27\n46.8\t27.5\n47\t28\n47.2\t28.5\n47.4\t29\n47.6\t29.5\n47.8\t30\n48\t30.5\n48.2\t31\n48.4\t31.5\n48.6\t32\n48.8\t32.5\n49\t33\n49.2\t33.5\n49.4\t34\n49.6\t34.5\n49.8\t35\n50\t35.5\n50.2\t36\n50.4\t36.5\n50.6\t37\n50.8\t37.5\n51\t38\n51.2\t38.5\n51.4\t39\n51.6\t39.5\n51.8\t40\n52\t40.5\n52.2\t41\n52.4\t41.5\n52.6\t42\n52.8\t42.5\n53\t43\n53.2\t43.5\n53.4\t44\n53.6\t44.5\n53.8\t45\n54\t45.5\n54.2\t46\n54.4\t46.5\n54.6\t47\n54.8\t47.5\n55\t48\n55.2\t48.5\n55.4\t49\n55.6\t49.5\n55.8\t50\n56\t50.5\n56.2\t51\n56.4\t51.5\n56.6\t52\n56.8\t52.5\n57\t53\n57.2\t53.5\n57.4\t54\n57.6\t54.5\n57.8\t55\n58\t55.5\n58.2\t56\n58.4\t56.5\n58.6\t57\n58.8\t57.5\n59\t58\n59.2\t58.5\n59.4\t59\n59.6\t59.5\n") -> (array=w13:dbl[][])  [unwired: 2 in]
      n34 = Get Date/Time In Seconds() -> (seconds since 1Jan1904=w25:timestamp)
      "Nombre total de vaisseaux" <- 5
    }
    frame #1 {
      n35 = while {
        tunnel: w56 -> [w100]
        shift-right: [w99] -> _
        shift-left: _ -> [w97]
        shift-right: [w97] -> _
        shift-left: _ -> [w96]
        tunnel: w55 -> [w58]
        i -> [w57]
        stop <- "Cancel Button" stop-if-true
        n36 = Subtract(x=w97, y=w96) -> (x-y=w95:u32)
        n37 = case shown="True" "Boolean" {
          frame False {
          }
          frame True {
          }
        }
        n38 = dll-call lib="PTH2Šabs CUsersCharles\tDocumentsÃ‰coleImplicationJeux PhotoniquesDÃ©fi Gentec-EOPC-Beamage Labview Distribution\nBeamageNP.dll" fn="WriteNP"("command"="*MEAMAJAX") -> (error out=w62:errorcluster)  [unwired: 5 in, 1 out]
        n39 = local read "Nombre total de vaisseaux"() -> (w88:dbl)
        n40 = dll-call lib="PTH2Šabs CUsersCharles\tDocumentsÃ‰coleImplicationJeux PhotoniquesDÃ©fi Gentec-EOPC-Beamage Labview Distribution\nBeamageNP.dll" fn="WriteNP"("command"="*MEACENTY") -> (error out=w66:errorcluster)  [unwired: 5 in, 1 out]
        n41 = dll-call lib="PTH2Šabs CUsersCharles\tDocumentsÃ‰coleImplicationJeux PhotoniquesDÃ©fi Gentec-EOPC-Beamage Labview Distribution\nBeamageNP.dll" fn="WriteNP"("command"="*MEACENTX") -> (error out=w80:errorcluster)  [unwired: 5 in, 1 out]
        n42 = Divide(x=w95, y=12000.0) -> (x/y=w90:dbl)
        n43 = local read "Pointage 1"() -> (w89:dbl)
        n44 = dll-call lib="PTH2Šabs CUsersCharles\tDocumentsÃ‰coleImplicationJeux PhotoniquesDÃ©fi Gentec-EOPC-Beamage Labview Distribution\nBeamageNP.dll" fn="ReadNP"(error in=w62, "command"="") -> ("command"=w63:string)  [unwired: 3 in, 2 out]
        n45 = dll-call lib="PTH2Šabs CUsersCharles\tDocumentsÃ‰coleImplicationJeux PhotoniquesDÃ©fi Gentec-EOPC-Beamage Labview Distribution\nBeamageNP.dll" fn="ReadNP"(error in=w66, "command"="") -> ("command"=w65:string)  [unwired: 3 in, 2 out]
        n46 = dll-call lib="PTH2Šabs CUsersCharles\tDocumentsÃ‰coleImplicationJeux PhotoniquesDÃ©fi Gentec-EOPC-Beamage Labview Distribution\nBeamageNP.dll" fn="ReadNP"(error in=w80, "command"="") -> ("command"=w81:string)  [unwired: 3 in, 2 out]
        n47 = Get Date/Time In Seconds() -> (seconds since 1Jan1904=w87:timestamp)
        n48 = Greater?(x=w90, y=0.05) -> (0:w92:bool)
        n49 = Decimal String To Number(string=w63) -> (number=w59:i32)  [unwired: 2 in, 1 out]
        n50 = Decimal String To Number(string=w65) -> (number=w69:i32)  [unwired: 2 in, 1 out]
        n51 = Decimal String To Number(string=w81) -> (number=w77:i32)  [unwired: 2 in, 1 out]
        n52 = Subtract(x=w87, y=w100) -> (x-y=w83:dbl)
        n53 = Less?(x=w89, y=w88) -> (x < y?=w84:bool)
        n54 = Multiply(x=w69, y=100) -> (x*y=w71:i32)
        n55 = Select(t=0.0, s=w92, f=w90) -> (s? t:f=w86:dbl)
        n56 = Multiply(x=w77, y=100) -> (x*y=w75:i32)
        n57 = Divide(x=w71, y=2992.0) -> (x/y=w64:dbl)
        n58 = Divide(x=w75, y=5632.0) -> (x/y=w73:dbl)
        n59 = Not(x=w84) -> (.not. x?=w85:bool)
        n60 = case shown="True" w84 {
          tunnel: w86 -> [_ w113]
          tunnel: w83 -> [_ _]
          tunnel: w87 -> [_ w112]
          tunnel: w83 -> [_ w109]
          tunnel: w73 -> [_ w108]
          tunnel: w64 -> [_ w107]
          tunnel: w59 -> [_ w106]
          tunnel: w58 -> [_ w105]
          tunnel: w57 -> [_ w104]
          frame False {
          }
          frame True {
            n61 = local read "Pause En Cours 1"() -> (w110:bool)
            n62 = Not(x=w110) -> (.not. x?=w111:bool)
            n63 = case shown="True" w110 {
              tunnel: w112 -> [_ w190]
              tunnel: w109 -> [w185 _]
              frame False {
                "Chrono 1" <- w185
              }
              frame True {
                w189 = 9
                n64 = local read "Temps Pause 1"() -> (w191:timestamp)
                n65 = Subtract(x=w190, y=w191) -> (x-y=w188:dbl)
                n66 = Greater?(x=w188, y=w189) -> (0:w187:bool)
                n67 = Subtract(x=w189, y=w188) -> (x-y=w186:dbl)
                n68 = case shown="True" w187 {
                  frame False {
                  }
                  frame True {
                    w198 = u32 0
                    n69 = local write "Pause En Cours 1"(FALSE) -> ()
                    n70 = property on="Chrono 1" class="DigNum (strict)"("NumText.BGColor"=w198) -> ()  [unwired: 2 in, 2 out]
                    n71 = property on="XY Graph 1" class="XYGraph (strict)"("BG Color"=w198) -> ()  [unwired: 2 in, 2 out]
                    n72 = local read "File Type"() -> (w195:enum16{"JPG", "PNG", "BMP"})
                    n73 = Current VI's Path() -> (path=w193:path)
                    n74 = Build Path(base path=w193, name or relative path=path "../Espace.bmp") -> (appended path=w192:path)
                    n75 = case shown="\"BMP\"" w195 {
                      tunnel: [w201 w203 w205] -> w196
                      tunnel: w192 -> [w200 w202 w204]
                      frame "JPG", Default {
                        n76 = call <vilib>:"Read JPEG File.vi"("path to JPEG file"=w200) -> ("image data"=w201:T1)  [unwired: 8 in, 2 out]
                      }
                      frame "PNG" {
                        n77 = call <vilib>:"Read PNG File.vi"("path to PNG file"=w202) -> ("image data"=w203:T1)  [unwired: 8 in, 2 out]
                      }
                      frame "BMP" {
                        n78 = call <vilib>:"Read BMP File.vi"("path to BMP file"=w204) -> ("image data"=w205:T1)  [unwired: 8 in, 2 out]
                      }
                    }
                    n79 = call <vilib>:"Draw Flattened Pixmap.vi"("image data"=w196) -> ("new picture"=w197:picture)  [unwired: 8 in]
                    n80 = property on="XY Graph 1" class="XYGraph (strict)"("PlotImages.Back"=w197) -> ()  [unwired: 2 in, 2 out]
                  }
                }
                n81 = local write "Chrono 1"(w186) -> ()
              }
            }
            n82 = case shown="True" w111 {
              tunnel: w113 -> [_ w156]
              tunnel: w108 -> [_ w128]
              tunnel: w107 -> [_ w140]
              tunnel: w106 -> [_ w136]
              tunnel: w105 -> [_ w124]
              tunnel: w104 -> [_ w125]
              tunnel: w105 -> [_ w120]
              tunnel: w104 -> [_ w119]
              frame False {
              }
              frame True {
                w141 = 0.0
                w155 = 100
                n83 = Index Array(array=w124, index (row)=w125, index (col)=0) -> (element=w126:dbl)
                n84 = Index Array(array=w120, index (row)=w119, index (col)=1) -> (element=w121:dbl)
                n85 = Less?(x=w136, y=11000) -> (x < y?=w138:bool)
                n86 = Select(t=w140, s=w138, f=2000.0) -> (s? t:f=w127:dbl)
                "Yposition" <- w127
                n87 = Subtract(x=w127, y=w121) -> (x-y=w129:dbl)
                n88 = Subtract(x=w128, y=w126) -> (x-y=w130:dbl)
                n89 = Square(x=w130) -> (x^2=w161:dbl)
                n90 = Square(x=w129) -> (x^2=w160:dbl)
                n91 = Build Array(w128) -> (w162:dbl[])
                n92 = Build Array(w127) -> (w163:dbl[])
                n93 = Build Array(w126) -> (w134:dbl[])
                n94 = Build Array(w121) -> (w135:dbl[])
                n95 = Add(x=w161, y=w160) -> (x+y=w159:dbl)
                n96 = Bundle(w162, w163) -> (w133:cluster{dbl[], dbl[]})  [unwired: 1 in]
                n97 = Bundle(w134, w135) -> (w132:cluster{dbl[], dbl[]})  [unwired: 1 in]
                n98 = Square Root(x=w159) -> (sqrt(x)=w158:dbl)
                n99 = Build Array(w133, w132) -> (→"XY Graph 1":cluster{dbl[], dbl[]}[])
                n100 = Subtract(x=w155, y=w158) -> (x-y=w118:dbl)
                n101 = Greater Or Equal?(x=w118, y=w141) -> (x >= y?=w142:bool)
                n102 = Select(t=w118, s=w142, f=w141) -> (s? t:f=w117:dbl)
                n103 = Square(x=w117) -> (x^2=w116:dbl)
                n104 = local read "Pointage 1"() -> (w151:dbl)
                n105 = local read "Barre Rouge 1"() -> (w150:dbl)
                n106 = Divide(x=w116, y=w155) -> (x/y=w115:dbl)
                "Barre Verte 1" <- w115
                n107 = local read "Nombre total de vaisseaux"() -> (w143:dbl)
                n108 = Multiply(x=w115, y=w156) -> (x*y=w157:dbl)
                n109 = Multiply(x=100.0, y=w151) -> (x*y=w114:dbl)
                n110 = Add(x=w157, y=w150) -> (x+y=w146:dbl)
                n111 = Divide(x=w114, y=w143) -> (x/y=→"Barre Bleue 1":dbl)
                n112 = Less?(x=w146, y=0.0) -> (x < y?=w147:bool)
                n113 = Greater Or Equal?(x=w146, y=100) -> (x >= y?=w153:bool)
                n114 = Select(t=0.0, s=w147, f=w146) -> (s? t:f=w144:dbl)
                n115 = case shown="True" w153 {
                  tunnel: w144 -> [w164 _]
                  frame False {
                    "Barre Rouge 1" <- w164
                  }
                  frame True {
                    n116 = local read "Nombre total de vaisseaux"() -> (w166:dbl)
                    n117 = Get Date/Time In Seconds() -> (seconds since 1Jan1904=→"Temps Pause 1":timestamp)
                    n118 = local read "Pointage 1"() -> (w169:dbl)
                    n119 = local write "Barre Rouge 1"(0) -> ()
                    n120 = Increment(x=w169) -> (x+1=w167:dbl)
                    n121 = Not Equal?(x=w167, y=w166) -> (x != y?=w165:bool)
                    n122 = local write "Pointage 1"(w167) -> ()
                    n123 = case shown="True" w165 {
                      frame False {
                      }
                      frame True {
                        w177 = u32 8650752
                        n124 = property on="Chrono 1" class="DigNum (strict)"("NumText.BGColor"=w177) -> ()  [unwired: 2 in, 2 out]
                        n125 = property on="XY Graph 1" class="XYGraph (strict)"("BG Color"=w177) -> ()  [unwired: 2 in, 2 out]
                        n126 = Current VI's Path() -> (path=w173:path)
                        n127 = Build Path(base path=w173, name or relative path=path "../Explosion.bmp") -> (appended path=w171:path)
                        n128 = case shown="\"BMP\"" "File Type 2" {
                          tunnel: [w180 w182 w184] -> w176
                          tunnel: w171 -> [w179 w181 w183]
                          frame "JPG", Default {
                            n129 = call <vilib>:"Read JPEG File.vi"("path to JPEG file"=w179) -> ("image data"=w180:T1)  [unwired: 8 in, 2 out]
                          }
                          frame "PNG" {
                            n130 = call <vilib>:"Read PNG File.vi"("path to PNG file"=w181) -> ("image data"=w182:T1)  [unwired: 8 in, 2 out]
                          }
                          frame "BMP" {
                            n131 = call <vilib>:"Read BMP File.vi"("path to BMP file"=w183) -> ("image data"=w184:T1)  [unwired: 8 in, 2 out]
                          }
                        }
                        n132 = call <vilib>:"Draw Flattened Pixmap.vi"("image data"=w176) -> ("new picture"=w174:picture)  [unwired: 8 in]
                        n133 = property on="XY Graph 1" class="XYGraph (strict)"("PlotImages.Back"=w174) -> ()  [unwired: 2 in, 2 out]
                        "Pause En Cours 1" <- TRUE
                      }
                    }
                  }
                }
                "Xposition" <- w128
                "Saturation Power" <- w136
              }
            }
          }
        }
        n134 = case shown="True" w85 {
          frame False {
          }
          frame True {
            n135 = local write "Pause En Cours 1"(FALSE) -> ()
            n136 = property on="Panneau de Fin" class="Str"("Visible"=TRUE) -> ()  [unwired: 2 in, 2 out]
          }
        }
        n137 = Wait (ms)(milliseconds to wait=20) -> ()  [unwired: 1 out]
        n138 = Tick Count (ms)() -> (millisecond timer value=w99:u32)
        "Loop" <- w57
      }
    }
  }
